vi "UNITEST MAIN v2.0.vi"() -> ()   [LabVIEW 2025]
uses:
  Traction Loop/Traction Receipe Enum.ctl
  v06/controls/LAB-IQ UI Data.ctl
  controls/REF Enum Unitest.ctl
  Acquostics Loops/Write Main Enum.ctl
  Acquostics Loops/Read Main Enum.ctl
  Temperature/Temperature enum.ctl
  Traction Loop/Traction Write enum.ctl
  Traction Loop/Traction Read enum.ctl
  HEAVE vi's/Heave Write enum.ctl
  HEAVE vi's/Heave Right enum.ctl
  SWAY vi's/Sway Write enum.ctl
  SWAY vi's/Sway Right enum.ctl
  v05/LOAD CELL CODE/New Logic/Load cell Enum.ctl
  48f5795f-33f4-4366-aaa7-704d1097ecc1.vi
  0f9b3d6c-7caf-4790-9f98-5fac89a3677b.vi
  d081153b-36ca-4bc4-8478-749476f82ba4.vi
  1202965f-721d-4349-8d61-5de826f379ef.vi
  02c5850b-52e8-4ed5-91f8-6f0ad62f4994.vi
  1223eb78-e4c4-4b69-bf80-185c82055158.vi
  e5651a45-6a49-4a3f-b503-ff1eaf449b4a.vi
  <vilib>/Utility/error.llb/Trim Whitespace One-Sided.vi
  support/Message Queue/Enqueue Message (Single).vi
  <vilib>/Utility/error.llb/Error Cluster From Error Code.vi
  <vilib>/Utility/file.llb/Read Delimited Spreadsheet (string).vi
  <vilib>/Utility/file.llb/Write Delimited Spreadsheet (string).vi
  <vilib>/ErrorRing/Error Ring.xnode
  support/Message Queue/LAB-IQ Message Queue.lvlib
  support/User Event - Stop/LAB-IQ User Event - Stop.lvlib
panel:
  in  "Disable Axis Jog Soft Limits":bool
  out "error out 6":errorcluster
  out "error out 5":errorcluster
  in  "Temperature 2":dbl caption="°C"
  out "error out 4":errorcluster
  out "Traction Recipe Start Recording":bool
  out "error out 3":errorcluster
  out "Depth (µm)":dbl min=-200.0 max=200.0 step=0.1 format="%.1f"
  out "tdms file out":refnum<k34>
  in  "Depthz":bool
  out "Acoustic Graphs":cluster{"number: 0 to 1":dbl, dbl, dbl}(graph)
  out "SET entrainment Velocity":dbl
  out "Test Array Size":i32
  in  "SRR INDEX [ STRIBECK]":i32
  out "Stribeck Size":i32
  out "SET SRR":dbl
  out "Enum - READ":T1
  out "ELAPSED TIMER":dbl
  out "BALL SET RPM":dbl
  out "DISC SET RPM":dbl
  out "SET LOAD":dbl
  in  "TEMPERATURE READ":dbl=40.0
  out "SET TEMPERATURE":dbl
  out "Traction Size":i32
  out "DISC SPEED (rpm)":dbl=100.0 min=0.1 max=3000.0 step=0.1 format="%.1f"
  out "BALL SPEED (rpm)":dbl=100.0 min=0.1 max=3000.0 step=0.1 format="%.1f"
  in  "BALL WEAR TRACK":dbl=7.9
  in  "DISC WEARTRACK":dbl=24.0
  in  "SRR INDEX [ TRACTION]":i32
  in  "Start Index Type":i32
  in  "Enum - Menu":T1
  out "Ball (mm/sec)":dbl
  out "Disc (mm/sec)":dbl
  in  "Traction Receipe Update Details":bool
  in  "HomeTraction":bool
  in  "Demo Mode Display":enum32{"Page 1", "Page 2"}(tab)
  in  "Traction Message":string="Recommended motion directions \nfor traction module.\n\nBall:  Counterclockwise\nDisc: Clockwise"
  in  "Traction Step Update Details":bool
  in  "Main Tab sequence for selection":T2(tab)
  out "ExceedDiscSpeed  Cinstant Speed":string
  out "ExceedBallSpeed Constant":string
  in  "TEST SELECTION (MTM) 2":enum32{"Ball Speed", "Disc Speed"}(radio)
  in  "SPEED SELECTION : MTM 2":enum32{"Speed in Rpm", "Speed in m/sec"}(radio)=enum."Speed in m/sec"
  in  "MTM Test Selection 2":enum32{"Time", "Cycle"}(radio)
  in  "Enter the Speed (m/sec):":dbl=0.5 min=3e-06 max=2500.0 step=0.001 format="%.6f"
  in  "Enter the Speed (m/sec):":dbl=0.5 min=3e-06 max=3000.0 step=0.001 format="%.6f"
  in  "Enter the Speed (RPM):":dbl=100.0 min=0.1 max=3000.0 step=0.1 format="%.1f"
  out "Lower Spped":string
  out "Upper":string
  in  "Enter the Speed (RPM):":dbl=1.0 min=0.1 max=2500.0 step=0.1 format="%.1f"
  out "ExceedBallSpeed step":string
  out "ExceedDiscSpeed":string
  out "Disc Speed Indicator":bool
  out "ExceedBallSpeed":string
  out "BallSpeed Exceed Indication":bool
  in  "Apply":bool
  in  "SPEED SELECTION : MTM":enum32{"Speed in Rpm", "Speed in m/sec"}(radio)=enum."Speed in m/sec"
  in  "TEST SELECTION (MTM)":enum32{"Ball Speed", "Disc Speed"}(radio)
  in  "MTM Test Selection":enum32{"Time", "Cycle"}(radio)
  in  "File Path Tab":enum32{"Page 1", "Page 2"}(tab)
  in  "File Path String":string="File Path Location : C:-->LAB-IQ 150 --> User Defined\n                                       Protocol-->File.txt"
  in  "Save":bool
  in  "Import":bool
  in  "File Path :":path
  in  "Step Sequence Indication Tab":enum32{"Page 1", "Page 2"}(tab)
  in  "Step Sequence Indication":string="Minimum 2 Steps required to perform the Speed Sequence"
  in  "Calculate Step":bool
  in  "StepTable":string[][](table)
  in  "Ramp Tab":enum32{"Page 1"}(tab)
  out "e.v/ssr":enum32{"E.V", "SSR"}(tab)
  in  "Enter Fixed SRR":dbl=1.0 min=-1.0 max=1.0 step=0.001 format="%.3f"
  in  "Enter the Final E.Velocity (m/s)":dbl=1.0 min=0.001 max=10.0 step=0.001 format="%.3f"
  in  "Enter initial E.Velocity (m/s)":dbl=2.0 min=0.001 max=10.0 step=0.001 format="%.3f"
  in  "Enter Fixed E.Velocity":dbl=1.0 min=0.001 max=2.0 step=0.001 format="%.3f"
  in  "Enter Final SRR":dbl=1.0 min=-1.0 max=1.0 step=0.001 format="%.2f"
  in  "Enter initial SRR":dbl=1.0 min=-1.0 max=1.0 step=0.001 format="%.2f"
  in  "Ball WTD":dbl=17.32 min=17.32 max=17.32 step=0.001 format="%.2f"
  in  "E.Velocity":bool caption="SRR"
  in  "Enter the Final Velocity (m/s)":dbl=1.0 min=0.001 max=2.0 step=0.001 format="%.3f"
  in  "Enter initial Velocity (m/s)":dbl=2.0 min=0.001 max=2.0 step=0.001 format="%.3f"
  out "Ramp Up   Disc":bool caption="Ramp Down"
  out "Initial DiscSpeed (RPM)":dbl=100.0 min=0.1 max=3000.0 step=0.1 format="%.1f"
  out "Final Speed (RPM)":dbl=1.0 min=0.1 max=3000.0 step=0.1 format="%.1f"
  out "Final Speed (RPM)":dbl=1.0 min=0.1 max=3000.0 step=0.1 format="%.1f"
  out "Initial Speed (RPM)":dbl=100.0 min=0.1 max=3000.0 step=0.1 format="%.1f"
  in  "Enter the Final Velocity (m/s)":dbl=1.0 min=0.001 max=2.0 step=0.001 format="%.3f"
  in  "Enter initial Velocity (m/s)":dbl=2.0 min=0.001 max=2.0 step=0.001 format="%.3f"
  out "Ramp Up":bool caption="Ramp Down"
  in  "Disc Motion Direction:":u16(ring) items=["Clockwise", "Counter Clockwise"]
  in  "Ball Motion Direction :":u16(ring) items=["Clockwise", "Counter Clockwise"]
  in  "Motion Mode:":u16(ring) items=["Uniform Rotation", "Speed Step", "Speed Ramp", "Speed Recipe"]
  in  "Wear Track Diameter (mm) 3":dbl=16.0 caption="Wear Track Diameter (mm):" min=1.0 max=20.0 step=0.01 format="%.2f"
  in  "Set WTD 2":bool
  in  "SRR Sweep Range (%)":string caption="Speed (mm/s)"
  out "Traction Receipe":i32(listbox)=-1
  in  "Total Execution Time":dbl
  in  "Total Steps":dbl
  in  "Duration / Step (s)":dbl=6.0
  in  "STRIBECK Fixed SRR List (%)":string="5,10,20,40,60,80,100"
  in  "Duration / Step (s)":dbl=6.0
  in  "SRR Sweep Range (%)":string
  in  "Speed (mm/s)":dbl=1000.0
  in  "Temperature Stages (°C)":string="40,100,140"
  in  "Load (N)":string="25"
  in  "Lubricant Name":string
  in  "Profile File Name":string
  out "error out":errorcluster
  in  "Checkbox 2":bool
  in  "Checkbox":bool=TRUE
  out "Scratch Start Recording":bool
  in  "SwaySpeed Set":bool
  in  "Analysis Home":bool
  out "Test Trip":bool
  out "Hymidity":bool
  in  "Humidity Disable trip":bool=TRUE
  in  "CoF Trip  2":dbl=540.0 min=100.0 max=540.0 step=1.0
  in  "File Path :  2":path
  out "Wear Track Diameter":dbl
  in  "Stribeck table":bool
  in  "seq":bool=TRUE
  out "Drive Error":string
  out "Scratch Start Test":bool
  in  "HomeScratch":bool
  in  "TEST SELECTION":enum32{"Time", "Cycle"}(radio)
  out "Spare 15":u8
  out "Spare 14":u8
  out "Spare 13":u8
  out "Spare 12":u8
  out "Spare 11":u8
  out "Spare 10":u8
  out "Spare 9":u8
  out "Spare 8":u8
  out "Start Test Temp":bool
  in  "PID Delay (sec)":dbl=1.0 format="%#_6p"
  out "Spare 15":u8
  out "Spare 14":u8
  out "Spare 13":u8
  out "Spare 12":u8
  out "Spare 11":u8
  out "Spare 10":u8
  out "Spare 9":u8
  out "Spare 8":u8
  out "Load Cell Temp":bool
  in  "Enter Fixed SRR 2":dbl min=0.0 max=0.0 format="%.3f"
  in  "E.Velocity 2":bool=TRUE caption="SRR"
  in  "Tab Control 3":T3(tab)
  in  "PID":T4={"min_deadband_floor"=50000000.0, "min_finetune_floor"=10.0, "dynamic_spindle_noise_scalar"=100.0, "filter_alpha"=0.05, "Vertical load (N)"=0.0, "Pulse delta"=0.0, "Fine Tune Zone"=10.0, "Max_pos_limit"=50000000.0, "Min_pos_limit"=0.0, "i_limit"=10.0, "Max Step Linit"=10.0, "Init Step"=10.0, "pct_scale"=100.0, "Deadband"=0.1, "Kd"=0.0, "Ki"=0.0, "Kp"=1.0, "Current Position"=0.0, "Set Load"=0.0, "Current Load"=0.0, "gFF Rot 7"={0.0, 0.0, 0.0}, "Bypass Load"=FALSE, "Enter ByPass Load"=0.0, "apply load"=FALSE} {"Vertical load (N)" format="%#.3f"}
  in  "Ramp":bool
  in  "Load Cell Link":T5={"model"="", "SN"=0, "Sensor IP"="192.168.1.100", "Port"=8080, "Acq Delay (ms)"=10.0, "Burst Delay (ms)"=10.0, "Save Dwell"=0.015, "FORCE (N)"=[], "TORQUE (N-m)"=[], "ft_data"=[1.0, 1.0, 1.0, 1.0, 1.0, 1.0], "running_flag"=FALSE, "ClearAll"=FALSE, "ZeroAll"=FALSE} {"Save Dwell" min=0.0 max=5.0 step=0.001 format="%.3f"}
  out "error out Temperature":errorcluster
  in  "READ TEMPERATURE":dbl
  out "Downlink traction":T6 {"TRACTION POSE 1" format="%#.6f"; "TRACTION POSE 2" format="%#.6f"; "Missed Packets" format="%#.6f"}
  in  "Uplink Traction":T7={"Sequence ID"=0, "Mode Command"=2, "Distance"=10000.0, "SPEED"=10000.0, "Reserved "=0.0, "SPARE 1"=0, "SPARE 2"=0, "SPARE  3"=0, "SPARE  4"=0, "SPARE  5"=0, "SPARE 6"=0, "SPARE 7"=0, "SPARE 8"=0, "SPARE 9"=0, "SPARE 10"=0, "SPARE 11"=0, "SPARE 12"=0, "SPARE 13"=0, "SPARE 14"=0, "SPARE 15"=0, "SPARE 16"=0, "SPARE 17"=0}
  out "DOWNLINK SWAY":T8 {"SWAY POSE" format="%#.6f"; "Rotary POSE" format="%#.6f"; "Missed Packets" format="%#.6f"}
  in  "UPLINK SWAY":T9={"Sequence ID"=0, "Mode Command"=2, "Distance"=10000.0, "SPEED"=10000.0, "Reserved"=0.0, "SPARE1"=0, "SPARE 2"=0, "SPARE  3"=0, "SPARE  4"=0, "SPARE  5"=0, "SPARE 6"=0, "SPARE 7"=0, "SPARE 8"=0, "SPARE 9"=0, "SPARE 10"=0, "SPARE 11"=0, "SPARE 12"=0, "SPARE 13"=0, "SPARE 14"=0, "SPARE 15"=0, "SPARE 16"=0, "SPARE 17"=0}
  out "DOWNLINK HEAVE":T10 {"HEAVE POSE" format="%#.6f"; "SURGE POSE" format="%#.6f"; "Missed Packets" format="%#.6f"}
  in  "UPLINK HEAVE":T11={"Sequence ID"=0, "Mode Command"=2, "Distance"=10000.0, "SPEED"=10000.0, "Reserved"=0.0, "SPARE 1"=0, "SPARE 2"=0, "SPARE 3"=0, "SPARE 4"=0, "SPARE 5"=0, "SPARE 6"=0, "SPARE 7"=0, "SPARE 8"=0, "SPARE 9"=0, "SPARE 10"=0, "SPARE 11"=0, "SPARE 12"=0, "SPARE 13"=0, "SPARE 14"=0, "SPARE 15"=0, "SPARE 16"=0, "SPARE 17"=0}
  out "error out 2":errorcluster
  in  "error in (no error)":errorcluster
  out "Downlink Packet":T12
  in  "Uplink Packet":T13
  in  "Manual Write TRACTION":bool
  out "TRACTION WRITE":string
  out "Read TRACTION Temp":bool
  out "error out Read TRACTION":errorcluster
  out "error out Write  TRACTION":errorcluster
  out "TRACTION READ":string
  in  "Manual Write SWAY":bool
  out "SWAY WRITE":string
  out "Read SWAY Temp":bool
  out "error out Read SWAY":errorcluster
  out "error out Write  SWAY":errorcluster
  out "SWAY READ":string
  out "HEAVE ENABLE":bool
  in  "Manual Write Heave & Surge":bool
  out "Heave and Surge Write":string
  out "Read Heave Temp":bool
  out "error out Read":errorcluster
  out "error out Write":errorcluster
  out "Heave and Surge Read":string
  out "DAQ Status":u32
  out "Isolated Gain":u32
  out "Current Filter Id":u32
  out "rx command count":u32
  out "Last Config Rejected":u32
  out "data out":string
  in  "Manual Write Acquostic":bool
  in  "Sway Loop Delay":dbl
  in  "Sway PID Speed":dbl=1.0 format="%.4f"
  in  "Sway Jog Speed":dbl=1.0 format="%.4f"
  in  "Heave Loop Delay":dbl
  in  "Heave PID Speed":dbl=15.0
  in  "Surge Jog Speed":dbl=1.0 format="%.4f"
  in  "Heave Jog Speed":dbl=15.0
  in  "Sway PPR":dbl=6400.0
  in  "Surge PPR":dbl=6400.0
  in  "Heave PPR":dbl=6400.0
  in  "Sway Pitch":dbl=2.0
  in  "Surge Pitch":dbl=3.0
  in  "Heave Pitch":dbl=4.0
  out "Sway Pulses/mm":dbl=320.0
  out "Surge Pulses/mm":dbl=1600.0
  out "Heave Pulses/mm":dbl=1600.0
  out "Zmm":dbl=1600.0
  in  "Heave distance":dbl=340.0
  in  "RotHomeSurgeOffsetCounts":dbl=311465.0
  in  "RotHomeSwayOffsetCounts":dbl=14656.0
  in  "TracHomeSwayOffsetCounts 20MM":dbl=1432.0
  in  "TracHomeSurgeOffsetCounts 20MM":dbl=505100.0
  in  "LRMHomeSwayOffsetCounts":dbl=26880.0
  in  "LRMHomeSurgeOffsetCounts":dbl=307197.0
  in  "Heave Counts:":dbl=100.0 min=0.0 max=100000000.0 step=1.0
  in  "Distance (mm):":dbl=100.0 min=0.0 max=1500.0 step=0.001 format="%.5f"
  in  "Distance (mm): 2":dbl=100.0 caption="Distance (mm):" min=0.0 max=1500.0 step=0.0001 format="%.3f"
  in  "Surge Counts:":dbl=100.0 min=0.0 max=100000000.0 step=1.0 format="%.1f"
  in  "Distance (mm): 3":dbl=100.0 caption="Distance (mm):" min=0.0 max=1500.0 step=0.001 format="%.5f"
  in  "Sway Counts:":dbl=100.0 min=0.0 max=100000000.0 step=1.0 format="%.2f"
  in  "Enter Distance":bool caption="Enter Counts"
  in  "SAVE  2":bool
  in  "DataSavingLoopDelay(ms)":dbl=15.0
  in  "Surge distance (mm)":dbl=370.0
  in  "Sway distance (mm)":dbl=245.0
  in  "Filter%":dbl=80.0 min=50.0 max=100.0 step=0.1 format="%.1f"
  in  "Apply Filter (Load)":bool=TRUE
  in  "Filter% 2":dbl=50.0 min=50.0 max=100.0 step=0.1 format="%.1f"
  in  "Apply Filter (FF)":bool
  in  "Acoustic Emission:":dbl=1.0 min=0.0001 max=200.0 step=0.0001 format="%.4f"
  in  "TracHomeSwayOffsetCounts 10MM":dbl=1432.0
  in  "TracHomeSurgeOffsetCounts 10MM":dbl=505100.0
  in  "Filter ON/OFF":bool=TRUE
  in  "Re-initilaize":bool
  in  "SAMPLES":dbl=100.0
  in  "JOG TRIP LOAD VALUE (N)":dbl
  in  "Start Button":bool
  in  "SURGE FORWARD COUNT":dbl
  in  "SURGE BACKWARD COUNT":dbl
  in  "SURGE SPEED":dbl
  in  "Firmware Version":string="BCLV 3.6"
  in  "Instrument Serial":string="770073"
  in  "Runtime":string="LabVIEW 2025 (64-bit)"
  in  "Workorder":string="2479"
  in  "Version":string="1.AU.26"
  in  "Operating System":string="Windows 11 Pro"
  in  "version":string="v1.AU.26"
  in  "COF TRIP VALUE":dbl
  in  "FF TRIP VALUE":dbl
  in  "CYCLIC FF TRIP VALUE":dbl
  in  "CYCLIC CoF TRIP VALUE":dbl
  in  "COF TRIP  ENABLE":bool
  in  "FF TRIP  ENABLE":bool
  in  "CYCLIC FF TRIP  ENABLE":bool
  in  "CYCLIC COF TRIP  ENABLE":bool
  in  "LOAD TRIP VALUE":dbl
  in  "LOAD TRIP  ENABLE":bool
  in  "DEPTH TRIP VALUE":dbl
  in  "DEPTH TRIP   ENABLE":bool
  in  "Rotary Vertical":bool
  in  "Rotary Horizontal":bool
  in  "Sway LRM":bool
  in  "LRM CAM":bool
  in  "Scratch 2":bool
  in  "Traction 2":bool
  in  "GUI":T14(tab)
  in  "Platform Settings":bool caption="Password"
  in  "Configure":bool caption="Password"
  in  "Home":bool caption="Password"
  in  "EXIT":bool
  in  "Analysis":bool caption="Password"
  in  "service 2":bool caption="Password"
  in  "MainPage":T15(tab)=enum."HOME"
  in  "Select Load Head":bool
  in  "Notes :":string
  in  "FILE":string
  in  "Sample ID :":string
  in  "Operator ID :":string
  in  "Operator Name :":string
  in  "Auto":bool caption="Power Status"
  in  "Disable Axis Jog Soft Limits m":bool
  out "Sway and Surge COM Status":bool=TRUE caption="Load COM Status"
  out "Heave COM Status":bool=TRUE caption="Load COM Status"
  in  "Enable Platform":bool
  in  "Surge Forward Main":bool
  in  "Surge Backward Main":bool
  in  "Sway Right Main":bool
  in  "Sway Left Main":bool
  in  "Heave Down Main":bool
  in  "Heave Up main":bool
  in  "mm":dbl=0.001 caption="Jog" min=0.001 max=100.0 step=0.01 format="%#.3f"
  in  "Surface Analysis":bool
  in  "Imaging":bool
  in  "Image Analysis":bool
  in  "Post Analysis":bool
  in  "SSP 0.75":bool
  in  "SSP 0.5":bool
  in  "SSP 0.3":bool
  in  "Warning":enum32{"Page 2"}(tab)
  in  "gui GIF":enum32{"Check", "Deca", "kilo", "Micro"}(tab)
  out "Communication is established":bool=TRUE caption="Load COM Status"
  in  "Reference Sample":u16(ring) items=["None", "Brass", "Aluminium", "Mild Steel"]
  in  "com 3":bool
  out "com":bool
  out "DecaForce COM Status":bool caption="Load COM Status"
  in  "Loading Mode":u16(ring) items=["Constant", "Ramp", "Steps", "Indentation"]
  in  "Enter the CoF Trip":dbl=1.0
  in  "Enter the Friction Force Trip":dbl=520.0 min=500.0 max=500.0 step=1.0 format="%#.1f"
  in  "Enter the Normal load Trip":dbl=520.0 min=500.0 max=500.0 step=0.001 format="%.3f"
  in  "KiloForce":bool
  in  "DecaForce":bool
  in  "MicroForce":bool
  in  "LHBack":bool
  in  "LHNext":bool
  in  "Load Selection":T16(tab)
  in  "Enter the Load  (N)":dbl=2.0 caption="Enter the Load (N)" min=2.0 max=50.0 step=0.1 format="%#.4f"
  in  "Enter the Final Load (N)":dbl=1.0 min=2.0 max=200.0 step=1.0 format="%#.0f"
  in  "Enter the Loading Rate (N/min)":dbl=60.0 min=1.0 max=200.0 step=0.1 format="%.2f"
  out "Warning 2":bool
  in  "Stribeck Table  For loading":string[][](table)
  in  "Clear 3":bool
  out "Message":string="Load Entered is out of range!!!"
  in  "Save 3":bool
  in  "Import 3":bool
  in  "Indentation":string[][](table)=[["Detection", "5", "2"], ["Unload", "0", "5"], ["Load", "10", "2"], ["Unload", "0", "5"], ["Detection", "5", "2"], ["Unload", "0", "5"]]
  in  "Multipoint":bool caption="Singlepoint"
  in  "AppLoad 4":bool
  in  "zNL":bool
  out "NL disp":dbl caption="Normal Load ( N )" min=-2000.0 max=2000.0 step=0.0001 format="%.1f"
  in  "Traction":bool
  in  "Surge Forward MM":bool
  in  "Surge Backward MM":bool
  in  "M3 Image":enum32{"Page 1", "Page 2"}(tab)
  in  "String 39":string="Jog heave to bring the upper sample closer to the lower sample within 1mm."
  in  "Sway Left MM":bool
  in  "Sway Right MM":bool
  in  "mm":dbl=0.001 caption="Jog" min=0.001 max=5.0 step=0.0001 format="%#.3f"
  in  "Heave Down MM":bool
  in  "Heave Up MM":bool
  in  "Wear Track Diameter (mm)":dbl=30.0 caption="Wear Track Diameter (mm):" min=1.0 max=30.0 step=1.0 format="%.2f"
  in  "Set WTD":bool
  in  "HomeScratch":bool
  in  "HomeRot":bool
  in  "PlaceModule":bool
  in  "Motion Mode:":u16(ring) items=["Uniform Rotation", "Angular Oscillation", "Stribeck ", "Steps"]
  in  "LR Sway":bool
  in  "Rot Hor":bool
  in  "Rot Ver":bool
  in  "Scratch":bool
  in  "LR Cam":bool
  in  "MMBack":bool
  in  "MMNext":bool
  in  "Rotary Module Selection":T17(tab)
  in  "SPEED SELECTION :":enum32{"Speed in RPM", "Speed in m/sec"}(radio)=enum."Speed in m/sec"
  in  "Enter the Speed(mm/sec)":dbl=0.1 min=0.0001 max=1000.0 step=0.1 format="%#.4f"
  in  "Enter the Speed (RPM)":dbl=45.0 min=1.0 max=3000.0 step=1.0
  in  "Enter the Frequency (Hz)":dbl=1.0 min=0.1 max=10.0 step=0.1 format="%.1f"
  in  "Enter the Angle (Deg)":dbl=45.0 min=5.0 max=300.0 step=1.0
  in  "Angular Oscillation Set":bool
  in  "Rotary Tab":enum32{"Page 1", "Page 2"}(tab)
  out "e.v/ssr 2":enum32{"E.V", "SSR"}(tab)
  in  "Enter the Final E.Velocity (m/s) 2":dbl=1.0 min=0.001 max=4.0 step=0.001 format="%.3f"
  in  "Enter initial E.Velocity (m/s) 2":dbl=2.0 min=0.001 max=4.0 step=0.001 format="%.3f"
  in  "Enter Fixed E.Velocity 2":dbl=1.0 min=0.001 max=2.0 step=0.001 format="%.3f"
  in  "Enter Final SRR 2":dbl=1.0 min=0.001 max=1.0 step=0.001 format="%.2f"
  in  "Enter initial SRR 2":dbl=1.0 min=0.001 max=1.0 step=0.001 format="%.2f"
  out "Final Speed (RPM) 3":dbl=1.0 min=0.1 max=3000.0 step=0.1 format="%.1f"
  out "Initial Speed (RPM) 2":dbl=100.0 min=0.1 max=3000.0 step=0.1 format="%.1f"
  in  "Enter the Final Velocity (m/s) 3":dbl=1.0 min=0.001 max=2.0 step=0.001 format="%.3f"
  in  "Enter initial Velocity (m/s)  3":dbl=2.0 min=0.001 max=2.0 step=0.001 format="%.3f"
  out "Ramp Up 2":bool caption="Ramp Down"
  in  "Import 2":bool
  in  "Save 2":bool
  in  "SPEED SELECTION : rotary":enum32{"Speed in Rpm", "Speed in m/sec"}(radio)=enum."Speed in m/sec"
  in  "calculate rotary":bool
  in  "String 45":string="File Path Location : C:-->LAB-IQ 150 --> User Defined\n                                       Protocol-->File.txt"
  in  "Step Speed":enum32{"Step Speed", "Step (load-Speed)"}(tab)
  in  "StepTable For Speed":string[][](table)
  in  "StepTable For Load-Speed":string[][](table)=[["", "", ""], ["", "", ""], ["", "", ""], ["", "", ""]]
  in  "StepTable For Speed 3":string[][](table)=[["", "", ""], ["", "", ""], ["", "", ""], ["", "", ""]]
  in  "Clear rot":bool
  in  "Motion Direction:  3":u16(ring)=1 items=["Clockwise", "Counter Clockwise"]
  in  "Enter Scratch length (mm):":dbl=1.0 min=1.0 max=50.0 step=0.0001 format="%.4f"
  in  "Enter Scratch Speed (mm/s):":dbl=1.0 min=0.003 max=10.0 step=0.0031 format="%.5f"
  in  "Scartch Offset":dbl=1.0 caption="Scratch Offset: (mm)" min=0.1 max=5.0 step=0.1 format="%.1f"
  in  "Motion type:":u16(ring) items=["Unidirection", "Bidirection"]
  in  "Scratch Mode":u16(ring) items=["Scratch", "Pre-Post Scan", "Multi Scratch"]
  in  "Rotary Speed Exced":string="Motor Speed Out of Range"
  in  "No of Scratch":dbl=1.0 min=1.0 max=50.0 step=0.0001
  out "Humidity  Status  3":bool caption="Communication Status"
  out "Low Temp  Status  2":bool=TRUE caption="Communication Status"
  out "TK4 status 2":bool=TRUE caption="Communication Status"
  in  "Acuostic M":string="Before selecting Acoustic make sure the sensor output pin is connected to A4."
  in  "Stage Temperature":dbl[](array[numeric])=[150.0, 230.0, 300.0, 350.0, 400.0, 450.0, 500.0]
  in  "Sample Temperature":dbl[](array[numeric])=[100.0, 150.0, 200.0, 250.0, 300.0, 350.0, 400.0]
  in  "Humidity (Amb)":bool
  in  "Clear List":bool
  out "Sensors Picked":string
  in  "Add to list":bool
  in  "Wear":bool
  in  "Vibration":bool
  in  "Humidity (Chamber)":bool
  in  "Temperature (Chamber)":bool
  in  "ECR":bool
  in  "Temperature (Amb)":bool
  in  "Microphone":bool
  in  "Acoustic Emission 3":bool
  in  "SNext":bool
  in  "APBack":bool
  in  "Enter the Temperature (°C):":dbl
  in  "Enter the Stage \nTemperature (°C):":dbl=20.0 min=20.0 max=150.0 step=1.0 format="%#.0f"
  in  "Enter the Humidity (%Rh):":dbl=30.0 min=30.0 max=85.0 step=1.0
  in  "Low Temp":bool
  in  "High Temp":bool
  in  "Humidity":bool
  in  "Gains":enum32{"20dB", "40dB", "60dB"}(radio)=enum."60dB"
  in  "Main Screen Tab":T18(tab)
  out "NL Trip 2":dbl=600.0
  in  "Load Disable Trip":bool=TRUE
  in  "Depth Trip 2":bool=TRUE
  out "Depth Trip":dbl=600.0
  in  "ClrLog":bool
  out "Trip Log":string
  in  "Start Test":bool
  out "Test status":bool caption="Test Status"
  out "AR Led":bool caption="AR"
  out "Data":bool=TRUE
  out "Health":bool=TRUE
  out "Sway COM Status":bool=TRUE caption="Load COM Status"
  out "Heave COM Status":bool=TRUE caption="Load COM Status"
  in  "BACK":bool
  out "Ambient \nTemperature":dbl min=0.0 max=5000.0 step=0.1 format="%.1f"
  out "Ambient\n Humidity":dbl min=0.0 max=5000.0 step=0.1 format="%.2f"
  out "NL disp 2":dbl caption="Normal Load ( N )" min=-2000.0 max=2000.0 step=0.0001 format="%.1f"
  out "Set Humidity":dbl caption="Set Humidity  (% Rh)" min=-2000.0 max=2000.0 step=1.0 format="%.1f"
  out "humidity disp":dbl caption="Humidity (% Rh)" min=-2000.0 max=2000.0 step=1.0 format="%.1f"
  in  "Humidity On":bool
  in  "zNL 2":bool
  in  "Load En":bool
  out "Freq (Hz)":dbl min=0.0 max=5000.0 step=0.1 format="%.4f"
  out "HumCOMStatus":bool caption="Communication Status"
  out "Load Communication":bool
  in  "Temp Tabs":enum32{"Low Temp", "High Temp"}(tab)=enum."High Temp"
  out "Controller  Status":bool
  out "ChamberTemp":dbl format="%#.1f"
  in  "SetTmp":dbl=-190.0 caption="Set Temperature (Deg C)" min=-190.0 max=100.0 step=1.0 format="%.1f"
  in  "Cooling":bool
  in  "Heater":bool
  out "TK4 status":bool caption="Controller  Status"
  out "ChamberTemp":dbl format="%#.1f"
  in  "SetTmp":dbl caption="Set Temperature (Deg C)" min=0.0 max=1000.0 step=1.0 format="%.1f"
  in  "Set Load (N)":dbl=100.0 min=0.01 max=1500.0 step=0.01 format="%.1f"
  in  "Time Tab":enum32{"cycles", "duration"}(tab)=enum."duration"
  out "Test Duration 4":dbl=600.0 caption="Test Duration\n(HH:MM:SS)" min=0.0083 max=180000.0 step=0.0001 format="%<%H:%M:%S>t"
  out "TEST CYCLE":dbl min=0.0 max=5000.0 step=0.01 format="%.2f"
  in  "TOTAL CYCLES":dbl min=0.0 max=5000.0 step=0.1 format="%.4f"
  out "Time ( HH:MM:SS ) 2":dbl min=0.0 max=144000.0 step=1.0 format="%<%H:%M:%S>t"
  in  "Test Duration":dbl=600.0 caption="Test Duration\n(HH:MM:SS)" min=0.0083 max=180000.0 step=0.0001 format="%<%H:%M:%S>t"
  in  "Main Speed Tab":enum32{"ROTARY", "TRACTION"}(tab)
  in  "SPEED TAB":enum32{"RPM", "m/sec"}(tab)
  out "Speed (RPM)":dbl min=0.0 max=5000.0 step=0.1 format="%.1f"
  out "Set Speed":dbl caption="Set Speed (RPM)" min=0.0 max=1500.0 step=0.1 format="%.1f"
  out "Speed (m/sec)":dbl min=0.0 max=5000.0 step=0.001 format="%.4f"
  out "Set Speed (m/sec)":dbl min=0.0 max=1500.0 step=0.001 format="%.4f"
  in  "MTM MOTOR DISPLAY":enum32{"MTM RPM", "MTM m/sec"}(tab)
  out "Disc Speed (RPM)":dbl min=0.0 max=1500.0 step=0.1 format="%.1f"
  out "Ball Speed (RPM)":dbl min=0.0 max=1500.0 step=0.1 format="%.1f"
  out "Disc Speed (m/sec)":dbl min=0.0 max=1500.0 step=0.1 format="%.1f"
  out "Ball Speed (m/sec)":dbl min=0.0 max=1500.0 step=0.1 format="%.1f"
  in  "Angle and Frequency":enum32{"angular", "lrm"}(tab)
  out "Angle (Deg)":dbl min=0.0 max=5000.0 step=0.01 format="%.2f"
  out "Stroke (mm)":dbl min=0.0 max=5000.0 step=0.01 format="%.2f"
  in  "STOP":bool
  out "Multi Scratch Pass":dbl min=0.0 max=5000.0 step=0.1
  in  "FF Tab":T19(tab)
  in  "COF Disable Trip":bool=TRUE
  out "COF TRIP":dbl=600.0
  out "Coefficient of Friction":dbl[](graph) caption="Waveform Chart - Dark"
  in  "zFF":bool
  in  "FF Disable Trip":bool=TRUE
  out "FF TRIP":dbl=600.0
  out "Friction Force (N)":dbl min=-2000.0 max=2000.0 step=0.0001 format="%.3f"
  out "Friction Force (N)":dbl[](graph) caption="Waveform Chart - Dark"
  in  "CZ FF":bool
  out "Cyclic Friction Force (N)":dbl min=-2000.0 max=2000.0 step=0.0001 format="%.3f"
  out "Cyclic FF TRIP":dbl=600.0
  in  "Cyclic FF Disable Trip":bool=TRUE
  out "cyclic COF TRIP":dbl=600.0
  in  "cyclic COF Disable Trip":bool=TRUE
  out "Acoustic Emission (mV)":dbl min=0.0 max=5000.0 step=0.1
  out "Normal Load ( N )":dbl[](graph) caption="Waveform Chart - Dark"
  out "Acoustic Emission":dbl[](graph) caption="Waveform Chart - Dark"
  out "Depth (Microns)":dbl[](graph) caption="Waveform Chart - Dark"
  in  "X-AXIS":u16(ring) items=["None", "Time ( Sec )", "Normal Load ( N )", "Frictional Force ( N )", "Coefficient of Friction", "Depth ( Microns )", "Speed ( RPM )", "Frequency ( Hz )", "Angle ( Degree )", "Cyclic Friction Force ( N )", "Cyclic Co efficient Friction ", "Stage temperature ( Degree celcius )", "Sample temperature ( Degree celcius )", "Stroke Length ( mm )", "Scratch Speed ( mm/sec )", "Amb Humidity ( % Rh ) ", "Amb Temperature (Deg C)", "Acoustic (mV)", "Mx (Nm)", "My (Nm)", "Mz (Nm)", "Humidity ( % Rh )", "Sliding Distance (mm)", "Wear Track Diameter (mm)", "Fx(N)", "Fy(N)", "MTM BallSpeed (RPM)", "MTM DiscSpeed (RPM)", "Entrainment Speed", "Slide Role", "Slip(%)", "Rotary Speed (m/sec)", "MTM Ball Speed (m/sec)", "MTM Disc Speed (m/sec)", "ECR (ohms)", "Cycles (N)"]
  in  "Y-AXIS":u16(ring) items=["None", "Time ( Sec )", "Normal Load ( N )", "Frictional Force ( N )", "Coefficient of Friction", "Depth ( Microns )", "Speed ( RPM )", "Frequency ( Hz )", "Angle ( Degree )", "Cyclic Friction Force ( N )", "Cyclic Co efficient Friction ", "Stage temperature ( Degree celcius )", "Sample temperature ( Degree celcius )", "Stroke Length ( mm )", "Scratch Speed ( mm/sec )", "Amb Humidity ( % Rh ) ", "Amb Temperature (Deg C)", "Acoustic (mV)", "Mx (Nm)", "My (Nm)", "Mz (Nm)", "Humidity ( % Rh )", "Sliding Distance (mm)", "Wear Track Diameter (mm)", "Fx(N)", "Fy(N)", "MTM BallSpeed (RPM)", "MTM DiscSpeed (RPM)", "Entrainment Speed", "Slide Role", "Slip(%)", "Rotary Speed (m/sec)", "MTM Ball Speed (m/sec)", "MTM Disc Speed (m/sec)", "ECR (ohms)", "Cycles (N)"]
  out "XY Graph":cluster{"Array 2":dbl[], "Array 2":dbl[]}[](graph) caption="XY Graph 20"
  out "VARIANCE":dbl=-0.0 format="%0.2f"
  out "SD":dbl=-0.0 format="%.3f"
  out "MEAN":dbl format="%.3f"
  out "VARIANCE":dbl=-0.0 format="%0.2f"
  out "SD":dbl=-0.0 format="%.3f"
  out "MEAN":dbl format="%.3f"
  out "VARIANCE":dbl=-0.0 format="%0.2f"
  out "SD":dbl=-0.0 format="%.3f"
  out "MEAN":dbl format="%.3f"
  out "VARIANCE":dbl=-0.0 format="%0.2f"
  out "SD":dbl=-0.0 format="%.3f"
  out "MEAN":dbl format="%.3f"
  in  "Analysis Home new":bool
  out "File 2 Discription":string="\r"
  out "File 1 Discription":string="\r"
  in  "OPEN 1":bool
  in  "OPEN 2":bool
  out "File Name 1":string
  out "File Name 2":string
  in  "Refresh 2":bool
  in  "OPEN 3":bool
  out "File Name 3":string
  out "File Name 4":string
  in  "OPEN 4":bool
  out "File 4 Discription":string="\r"
  out "File 3 Discription":string="\r"
  in  "File Format":u16(ring) items=["csv", "txt", "duf"]
  in  "Export":bool
  in  "Report":bool
  in  "Password":string
  in  "Home Service":bool
  in  "Advanced Setting":bool
  in  "Edit Gain Constants":bool
  in  "Save Gain Constants":bool
  in  "Humidity Port:":refnum<visa-resource-name>="COM10"
  in  "Temperature":refnum<visa-resource-name>="COM14"
  in  "ECR Port:":refnum<visa-resource-name>="COM10"
  in  "Info":bool
  in  "Service About":bool
  # "1. Test Identification & Global Setup"
  # "2. Step Configurations & Timing"
  # "Step 1 Configuration: TRACTION Step"
  # "%"
  # "NOTE: This operation needs to be done only when the machine is ON."
  # "Steps 2+ Configuration: STRIBECK Steps"
  # "Acoustic Emission (mV)"
  # "Upper Drive (Ball)"
  # "Lower Drive (Disc)"
  # "Variable"
  # "Configuration"
  # "ABOUT SCREEN PARAMETERS"
  # "Limits for Heave Surge and Sway"
  # "© 2023"
  # "Modules Offset Parameters"
  # "Counts-Distance Calculator"
  # "SURGE MOVEMENT"
  # "STAGE SELECTION"
  # "LOAD TRIP PARAMETERS"
  # "File Name :"
  # "Ensure the traction module is aligned\n horizontally with the stage before ENABLE."
  # "JOG MODE"
  # "Module Selection"
  # "Positioning Control"
  # "Connect the controller\ncable to M2"
  # "Environment"
  # "Sensors"
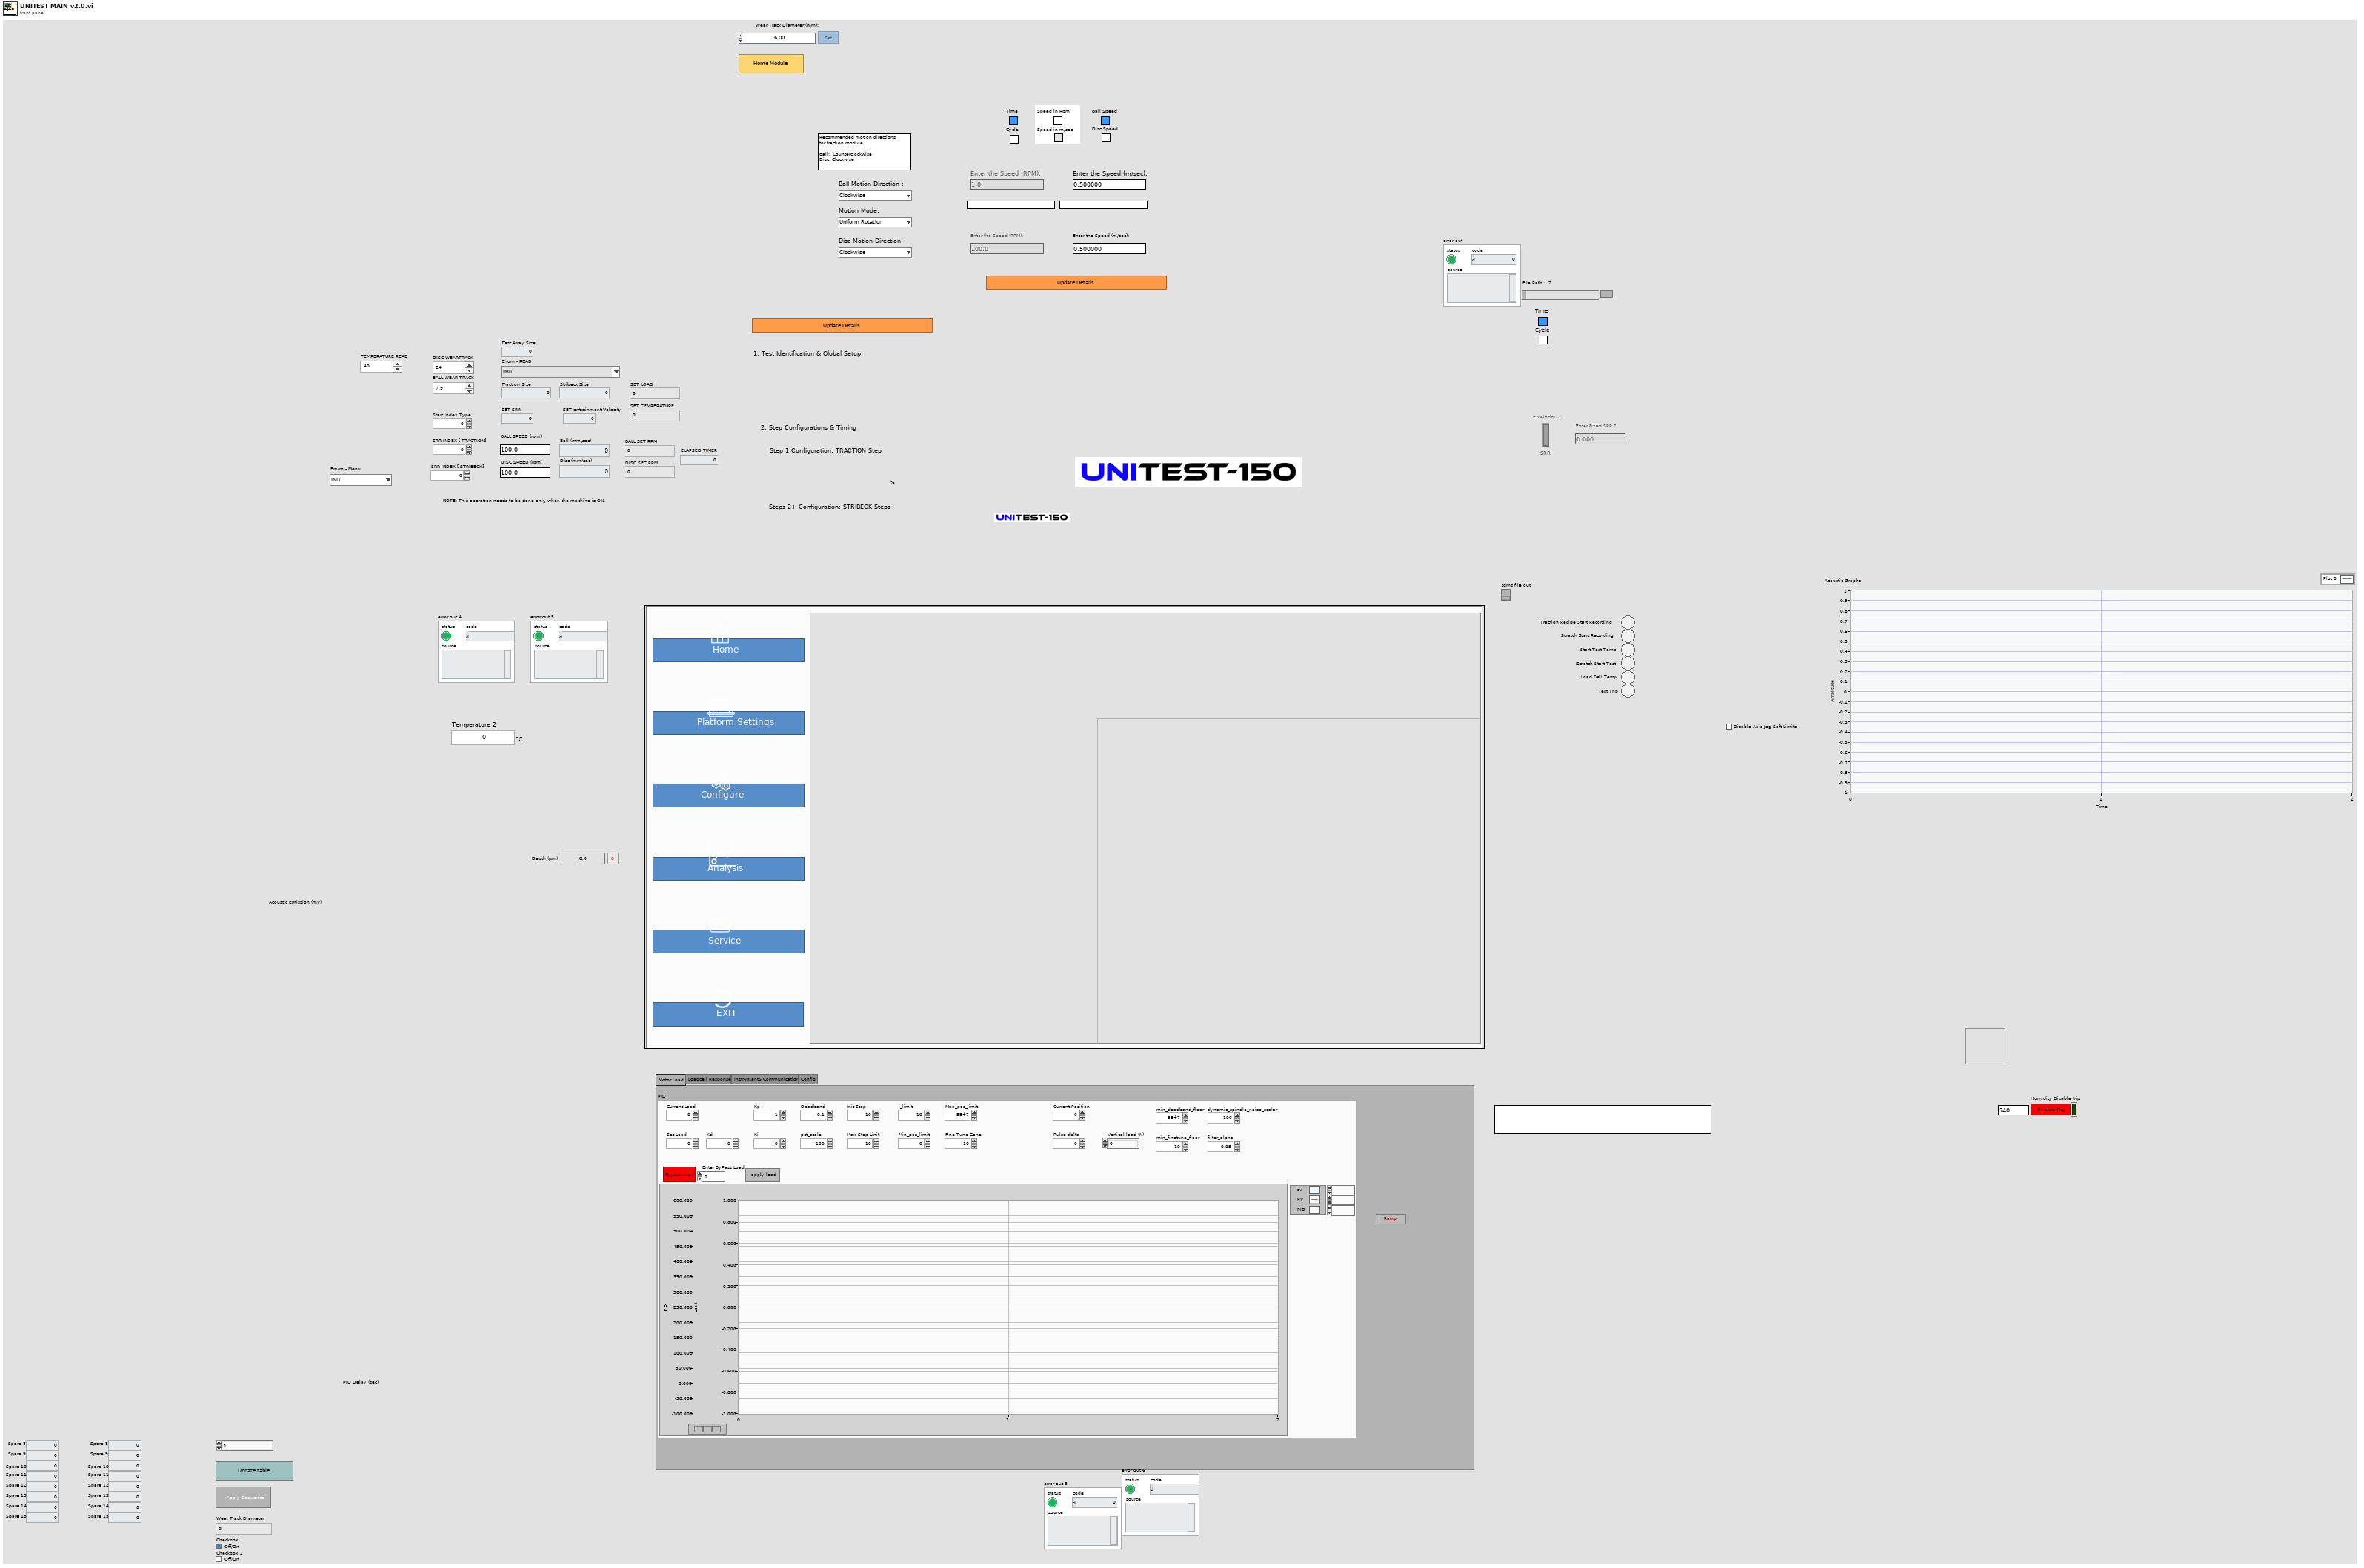
[diagram p1: front panel]
types:
  T1 = typedef "Traction Receipe Enum.ctl" = enum16{"INIT", "START", "TRACTION", "STRIBECK", "MAIN INDEX INCREMENT", "TEMPERATURE SET", "TEMPERATURE REACH", "CHURNING START", "CHURNING STOP", "LOAD", "LOAD REACHED", "SRR SET", "SRR WAIT", "SRR INCREMENT", "SPEED SET", "SPEED WAIT", "SPEED INCREMENT", "UNLOAD", "CLOSE"}
  T2 = enum32{"Uniform Rotary", "Speed Sequence", "SpeedRamp"}
  T3 = enum32{"Motor Load", "Loadcell Response", "Motor", "Depth_graph", "UIO Communicator", "Add to list parametrs", "InstrumentS Communication", "Config"}
  T4 = cluster{"min_deadband_floor":dbl, "min_finetune_floor":dbl, "dynamic_spindle_noise_scalar":dbl, "filter_alpha":dbl, "Vertical load (N)":dbl, "Pulse delta":dbl, "Fine Tune Zone":dbl, "Max_pos_limit":dbl, "Min_pos_limit":dbl, "i_limit":dbl, "Max Step Linit":dbl, "Init Step":dbl, "pct_scale":dbl, "Deadband":dbl, "Kd":dbl, "Ki":dbl, "Kp":dbl, "Current Position":dbl, "Set Load":dbl, "Current Load":dbl, "gFF Rot 7":cluster{dbl, dbl, dbl}, "Bypass Load":bool, "Enter ByPass Load":dbl, "apply load":bool}
  T5 = cluster{"model":string, "SN":i32, "Sensor IP":string, "Port":i32, "Acq Delay (ms)":dbl, "Burst Delay (ms)":dbl, "Save Dwell":dbl, "FORCE (N)":dbl[][], "TORQUE (N-m)":dbl[][], "ft_data":dbl[], "running_flag":bool, "ClearAll":bool, "ZeroAll":bool}
  T6 = cluster{"Ack ID":u16, "State":u8, "Homed":u8, "TRACTION POSE 1":sgl, "TRACTION POSE 2":sgl, "faultCode ":u16, "fwMajor ":u8, "fwMinor":u8, "Node Id":u8, "Spare 1":u8, "Spare 2":u8, "Spare 3":u8, "Spare 4":u8, "Spare 5":u8, "Spare 6":u8, "Spare 7":u8, "System UPTIME":sgl, "Missed Packets":sgl, "faultCode Traction 1":u16, "faultCode Traction 2":u16}
  T7 = cluster{"Sequence ID":u16, "Mode Command":u8, "Distance":sgl, "SPEED":sgl, "Reserved ":sgl, "SPARE 1":u8, "SPARE 2":u8, "SPARE  3":u8, "SPARE  4":u8, "SPARE  5":u8, "SPARE 6":u8, "SPARE 7":u8, "SPARE 8":u8, "SPARE 9":u8, "SPARE 10":u8, "SPARE 11":u8, "SPARE 12":u8, "SPARE 13":u8, "SPARE 14":u8, "SPARE 15":u8, "SPARE 16":u8, "SPARE 17":u8}
  T8 = cluster{"Ack ID ":u16, "State":u8, "Homed":u8, "SWAY POSE ":sgl, "Rotary POSE ":sgl, "faultCode":u16, "fwMajor":u8, "fwMinor":u8, "Node Id":u8, "Spare 1":u8, "Spare 2":u8, "Spare 3":u8, "Spare 4":u8, "Spare 5":u8, "Spare 6":u8, "Spare 7":u8, "System UPTIME ":sgl, "Missed Packets ":sgl, "faultCode Sway":u16, "faultCode Rotary":u16}
  T9 = cluster{"Sequence ID":u16, "Mode Command":u8, "Distance":sgl, "SPEED":sgl, "Reserved":sgl, "SPARE1":u8, "SPARE 2":u8, "SPARE  3":u8, "SPARE  4":u8, "SPARE  5":u8, "SPARE 6":u8, "SPARE 7":u8, "SPARE 8":u8, "SPARE 9":u8, "SPARE 10":u8, "SPARE 11":u8, "SPARE 12":u8, "SPARE 13":u8, "SPARE 14":u8, "SPARE 15":u8, "SPARE 16":u8, "SPARE 17":u8}
  T10 = cluster{"Ack ID":u16, "State":u8, "Homed":u8, "HEAVE POSE":sgl, "SURGE POSE":sgl, "faultCode":u16, "fwMajor":u8, "fwMinor":u8, "Node Id":u8, "Temp":u8, "Humidity":u8, "Spare 1":u8, "Spare 2":u8, "Spare 3":u8, "Spare 4":u8, "Spare 5":u8, "System UPTIME":sgl, "Missed Packets":sgl, "faultCode Heave":u16, "faultCode Surge Left":u16, "faultCode Surge Right":u16}
  T11 = cluster{"Sequence ID":u16, "Mode Command":u8, "Distance":sgl, "SPEED":sgl, "Reserved":sgl, "SPARE 1":u8, "SPARE 2":u8, "SPARE 3":u8, "SPARE 4":u8, "SPARE 5":u8, "SPARE 6":u8, "SPARE 7":u8, "SPARE 8":u8, "SPARE 9":u8, "SPARE 10":u8, "SPARE 11":u8, "SPARE 12":u8, "SPARE 13":u8, "SPARE 14":u8, "SPARE 15":u8, "SPARE 16":u8, "SPARE 17":u8}
  T12 = cluster{"Sequence ID":u32, "Timestamp":u32, "System Status":u32, "Peak Amplitude":sgl, "Amplitude dB_AE":sgl, "AE Ring-Down Counts":u32, "Signal Energy":sgl, "Spare 1":u32}
  T13 = cluster{"Sequence ID":u32, "Target Gain":u32, "Target Filter":u32, "Spare 1":u32, "Spare 2":u32, "Spare 3":u32, "Spare 4":u32, "Spare 5":u32}
  T14 = enum32{"Setup", "Load Head", "Motion Module", "Environment", "Begin"}
  T15 = enum32{"Details", "PlatformSetting", "Analysis", "HOME"}
  T16 = enum32{"Constant", "Ramp", "Step", "Indentation"}
  T17 = enum32{"Uniform Rotation", "Angular Oscillation", "Speed Ramp", "Speed Step"}
  T18 = enum32{"  Acquire  ", "Compare Files Rot", "About", "Service"}
  T19 = enum32{"Coefficient of Friction ", "Friction Force (N)", "Cyclic Friction Force (N)", "Cyclic Coefficient of Friction "}
  T20 = typedef "REF Enum Unitest.ctl" = enum16{"Init", "UI Loop", "LOAD COM LOOP", "HEAVE MOTOR COM LOOP", "SWAY MOTOR COM LOOP", "RAMP MOTOR COM LOOP", "TEMPERATURE COM LOOP", "HUMIDITY COM PORT", "ECR PORT", "MONITOR LOOP", "PROGRAM LOOP", "LOAD PID", "REPORT", "ACOUSTIC"}
  T21 = typedef "LAB-IQ UI Data.ctl" = cluster{"Main Home Screen":cluster{"GUI":refnum<vi>, "Platform Settings":refnum<vi>, "Configure":refnum<vi>, "Home":refnum<vi>, "EXIT":refnum<vi>, "service 2":refnum<vi>, "MainPage":refnum<vi>, "Analysis":refnum<vi>}, "Platform Settings":cluster{"mm/s  Surge":refnum<vi>, "Drive Error":refnum<vi>, "Disable Axis Jog Soft Limits":refnum<vi>, "mm/s  Sway":refnum<vi>, "Sway and Surge COM Status":refnum<vi>, "Heave COM Status":refnum<vi>, "Enable Platform":refnum<vi>, "Surge Forward Main":refnum<vi>, "Sway Right Main":refnum<vi>, "Sway Left Main":refnum<vi>, "Heave Down Main":refnum<vi>, "Heave Up main":refnum<vi>, "mm/s Heave":refnum<vi>, "mm/sec":refnum<vi>, "mm":refnum<vi>, "Surge Backward Main":refnum<vi>}, "Analysis Screen":cluster{"Analysis Home":refnum<vi>, "Surface Analysis":refnum<vi>, "Imaging":refnum<vi>, "Image Analysis":refnum<vi>, "Post Analysis":refnum<vi>}, "Config Screen":cluster{"Select Load Head":refnum<vi>, "Notes :":refnum<vi>, "FILE":refnum<vi>, "Sample ID :":refnum<vi>, "Operator ID :":refnum<vi>, "Operator Name :":refnum<vi>, "Auto":refnum<vi>}, "Motion Module":cluster{"zNL":refnum<vi>, "NL disp":refnum<vi>, "Rotary Tab":refnum<vi>, "Motion Direction:  3":refnum<vi>, "E.Velocity 2":refnum<vi>, "e.v/ssr 2":refnum<vi>, "Enter Fixed E.Velocity 2":refnum<vi>, "Enter Final SRR 2":refnum<vi>, "Enter initial SRR 2":refnum<vi>, "Enter Fixed SRR 2":refnum<vi>, "Enter the Final E.Velocity (m/s) 2":refnum<vi>, "Enter initial E.Velocity (m/s) 2":refnum<vi>, "Final Speed (RPM) 3":refnum<vi>, "Initial Speed (RPM) 2":refnum<vi>, "Enter the Final Velocity (m/s) 3":refnum<vi>, "Enter initial Velocity (m/s)  3":refnum<vi>, "Ramp Up 2":refnum<vi>, "TEST SELECTION":refnum<vi>, "SPEED SELECTION : ":refnum<vi>, "Angular Oscillation Set":refnum<vi>, "Traction":refnum<vi>, "Step Speed":refnum<vi>, "StepTable For Load-Speed":refnum<vi>, "StepTable For Speed":refnum<vi>, "Surge Forward MM":refnum<vi>, "Surge Backward MM":refnum<vi>, "M3 Image":refnum<vi>, "String 39":refnum<vi>, "Sway Left MM":refnum<vi>, "Sway Right MM":refnum<vi>, "Disable Axis Jog Soft Limits":refnum<vi>, "mm":refnum<vi>, "Heave Down MM":refnum<vi>, "Heave Up MM":refnum<vi>, "Wear Track Diameter (mm)":refnum<vi>, "Set WTD":refnum<vi>, "HomeScratch":refnum<vi>, "HomeRot":refnum<vi>, "PlaceModule":refnum<vi>, "Enter the Angle (Deg)":refnum<vi>, "Enter the Frequency (Hz)":refnum<vi>, "Motion Mode:":refnum<vi>, "LR Sway":refnum<vi>, "Rot Hor":refnum<vi>, "Scratch":refnum<vi>, "LR Cam":refnum<vi>, "MMBack":refnum<vi>, "MMNext":refnum<vi>, "Rot Ver":refnum<vi>, "Rotary Module Selection":refnum<vi>, "calculate rotary":refnum<vi>, "SPEED SELECTION : rotary":refnum<vi>, "Import 2":refnum<vi>, "Save 2":refnum<vi>, "File Path :  2":refnum<vi>, "String 45":refnum<vi>, "StepTable For Speed 3":refnum<vi>, "Enter the Speed(mm/sec)":refnum<vi>, "Enter the Speed(RPM)":refnum<vi>, "Enter Scratch Speed (mm/s):":refnum<vi>, "SwaySpeed Set":refnum<vi>, "Scartch Offset":refnum<vi>, "Motion type:":refnum<vi>, "HomeScratch 2":refnum<vi>, "Enter Scratch length (mm):":refnum<vi>, "Wear Track Diameter":refnum<vi>, "Rotary Speed Exced":refnum<vi>, "Scratch Mode":refnum<vi>, "No of Scratch":refnum<vi>}, "Environmental control":cluster{"Humidity  Status  3":refnum<vi>, "Low Temp  Status  2":refnum<vi>, "TK4 status 2":refnum<vi>, "Stage Temperature":refnum<vi>, "Sample Temperature":refnum<vi>, "Humidity (Amb)":refnum<vi>, "Clear List":refnum<vi>, "Add to list":refnum<vi>, "Wear":refnum<vi>, "Vibration":refnum<vi>, "Humidity (Chamber)":refnum<vi>, "Temperature (Chamber)":refnum<vi>, "ECR ":refnum<vi>, "Temperature (Amb)":refnum<vi>, "Microphone":refnum<vi>, "Acoustic Emission 3":refnum<vi>, "SNext":refnum<vi>, "APBack":refnum<vi>, "Enter the Temperature (°C):":refnum<vi>, "Enter the Stage \nTemperature (°C):":refnum<vi>, "Enter the Humidity (%Rh):":refnum<vi>, "Low Temp":refnum<vi>, "High Temp":refnum<vi>, "Humidity":refnum<vi>, "Sensors Picked":refnum<vi>}, "About Screen":cluster{"Password":refnum<vi>, "Home Service":refnum<vi>, "Advanced Setting":refnum<vi>, "About Tab":refnum<vi>, "ECR Port:":refnum<vi>, "Ramp Port:":refnum<vi>, "Installation/Replacement completed":refnum<vi>, "Loahead":refnum<vi>, "Heave and Surge COM Port:":refnum<vi>, "Sway COM Port:":refnum<vi>, "Temp Modbus:":refnum<vi>, "Humidity Port:":refnum<vi>, "Edit Gain Constants":refnum<vi>, "Save Gain Constants":refnum<vi>}, "Main Screen":cluster{"Main Screen Tab":refnum<vi>, "Angle and Frequency":refnum<vi>, "Stroke (mm)":refnum<vi>, "Angle (Deg)":refnum<vi>, "Main Speed Tab":refnum<vi>, "MTM MOTOR DISPLAY":refnum<vi>, "Disc Speed (m/sec)":refnum<vi>, "Ball Speed (m/sec)":refnum<vi>, "Disc Speed (RPM)":refnum<vi>, "Ball Speed (RPM)":refnum<vi>, "SPEED TAB":refnum<vi>, "Speed (m/sec)":refnum<vi>, "Set Speed (m/sec)":refnum<vi>, "Speed (RPM)":refnum<vi>, "Set Speed":refnum<vi>, "Time Tab":refnum<vi>, "Time ( HH:MM:SS ) 2":refnum<vi>, "Test Duration":refnum<vi>, "Test Duration 4":refnum<vi>, "TEST CYCLE":refnum<vi>, "TOTAL CYCLES":refnum<vi>, "Set Load (N)":refnum<vi>, "Temp Tabs":refnum<vi>, "Heater":refnum<vi>, "TK4 status":refnum<vi>, "ChamberTemp":refnum<vi>, "SetTmp":refnum<vi>, "Controller  Status":refnum<vi>, "ChamberTemp 2":refnum<vi>, "SetTmp 2":refnum<vi>, "Controller  Status 2":refnum<vi>, "ChamberTemp 3":refnum<vi>, "SetTmp 3":refnum<vi>, "Cooling":refnum<vi>, "Load Communication":refnum<vi>, "Ambient \nTemperature":refnum<vi>, "HumCOMStatus":refnum<vi>, "Ambient\n Humidity":refnum<vi>, "Freq (Hz)":refnum<vi>, "Load En":refnum<vi>, "NLt":refnum<vi>, "zNL 2":refnum<vi>, "Humidity On":refnum<vi>, "humidity disp":refnum<vi>, "Set Humidity":refnum<vi>, "NL disp 2":refnum<vi>, "Humidity On 2":refnum<vi>, "humidity disp 2":refnum<vi>, "Set Humidity 2":refnum<vi>, "NL disp 3":refnum<vi>, "AppLoadSeq scratch":refnum<vi>, "Stop Scratch":refnum<vi>, "ClrLog":refnum<vi>, "Trip Log":refnum<vi>, "STOP":refnum<vi>, "Start Test":refnum<vi>, "Test status":refnum<vi>, "AR Led":refnum<vi>, "Data":refnum<vi>, "Health":refnum<vi>, "Sway COM Status":refnum<vi>, "Heave COM Status":refnum<vi>, "Grp Tab":refnum<vi>, "Sub Graph":refnum<vi>, "SD (mm)":refnum<vi>, "Siliding distance Reset Graph":refnum<vi>, "SDGp":refnum<vi>, "Humidity Reset Graph":refnum<vi>, "HumrGp":refnum<vi>, "Acoustic Emission (mV)":refnum<vi>, "Aqucostic Reset Graph":refnum<vi>, "gACQUOS":refnum<vi>, "ECR RESET":refnum<vi>, "ECR":refnum<vi>, "Temperature Reset":refnum<vi>, "Acoustic Emission (mV) 2":refnum<vi>, "Aqucostic Reset Graph 2":refnum<vi>, "gACQUOS 2":refnum<vi>, "ECR RESET 2":refnum<vi>, "ECR 2":refnum<vi>, "Temperature Reset 2":refnum<vi>, "Temperature (deg c)":refnum<vi>, "Speed Reset Graph":refnum<vi>, "Speed Tab":refnum<vi>, "MTM DISC  SPEED":refnum<vi>, "MTM BALL SPEED":refnum<vi>, "speed mm/sec":refnum<vi>, "Hymidity":refnum<vi>, "Humidity Disable trip":refnum<vi>, "CoF Trip  2":refnum<vi>, "Depth Trip":refnum<vi>, "Weart Deapth":refnum<vi>, "Depth Reset Graph":refnum<vi>, "Weart":refnum<vi>, "Depthz":refnum<vi>, "Depth (µm)":refnum<vi>, "WearGp":refnum<vi>, "NL Trip 2":refnum<vi>, "Load pid":refnum<vi>, "Load Disable Trip":refnum<vi>, "Load Reset Graph":refnum<vi>, "NL Display 4":refnum<vi>, "Main Chart 3":refnum<vi>, "BACK":refnum<vi>, "Depth Trip 2":refnum<vi>, "COF TRIP ":refnum<vi>, "Friction Force (N)":refnum<vi>, "FF Reset Graph":refnum<vi>, "FF Disable Trip":refnum<vi>, "FF TRIP":refnum<vi>, "COF Disable Trip":refnum<vi>, "COF Reset Graph":refnum<vi>, "Start Test Temp":refnum<vi>, "zFF":refnum<vi>, "Friction Force (N) Graph":refnum<vi>, "Coefficient of Friction":refnum<vi>, "Scratch Start Test":refnum<vi>, "FF Tab":refnum<vi>, "Cyclic Friction Force (N)":refnum<vi>, "CZ FF":refnum<vi>, "Cyclic Friction Force (N) Graph":refnum<vi>, "Cyclic Coefficient of Friction":refnum<vi>, "Cyclic FF TRIP":refnum<vi>, "Cyclic FF Disable Trip":refnum<vi>, "cyclic COF Disable Trip":refnum<vi>, "cyclic COF TRIP":refnum<vi>, "cyclic COF Reset Graph":refnum<vi>, "Cyclic FF Reset Graph":refnum<vi>, "Test Trip":refnum<vi>, "Multi Scratch Pass":refnum<vi>, "Scratch Start Recording":refnum<vi>, "Coefficient of Friction 2":refnum<vi>, "Acoustic Emission":refnum<vi>, "Friction Force (N) 2":refnum<vi>, "Depth (Microns)":refnum<vi>, "Normal Load ( N )":refnum<vi>}, "Loading":cluster{"Indentation":refnum<vi>, "Reference Sample":refnum<vi>, "Load Cell Communication Slide":refnum<vi>, "com 3":refnum<vi>, "com":refnum<vi>, "DecaForce COM Status":refnum<vi>, "Update":refnum<vi>, "Clear 3":refnum<vi>, "seq":refnum<vi>, "Stribeck table":refnum<vi>, "Stribeck Table  For loading":refnum<vi>, "Loading Mode":refnum<vi>, "Enter the Final Load (N)":refnum<vi>, "Enter the CoF Trip":refnum<vi>, "Enter the Friction Force Trip":refnum<vi>, "Enter the Normal load Trip":refnum<vi>, "Enter the Load  (N)":refnum<vi>, "KiloForce":refnum<vi>, "DecaForce ":refnum<vi>, "MicroForce":refnum<vi>, "LHBack":refnum<vi>, "LHNext":refnum<vi>, "Enter the Loading Rate (N/min)":refnum<vi>, "Message":refnum<vi>, "Warning 2":refnum<vi>, "SSP 0.75":refnum<vi>, "SSP 0.5":refnum<vi>, "SSP 0.3":refnum<vi>, "Warning":refnum<vi>, "gui GIF":refnum<vi>, "Communication is established":refnum<vi>, "AppLoad 4":refnum<vi>, "Multipoint":refnum<vi>, "Load Selection":refnum<vi>}, "PID":cluster{"Ramp":refnum<vi>, "Vertical load (N)":refnum<vi>, "apply load":refnum<vi>, "apply load 2":refnum<vi>, "Enter ByPass Load":refnum<vi>, "Bypass Load":refnum<vi>, "gFF Rot":refnum<vi>}, "Config Parameters":cluster{"Tab Control 3":refnum<vi>, "Tab Control 19":refnum<vi>, "SAMPLES":refnum<vi>, "Re-initilaize":refnum<vi>, "Filter ON/OFF":refnum<vi>, "TracHomeSurgeOffsetCounts 10MM":refnum<vi>, "TracHomeSwayOffsetCounts 10MM":refnum<vi>, "Acoustic Emission:":refnum<vi>, "Apply Filter (FF)":refnum<vi>, "Filter% 2":refnum<vi>, "Apply Filter (Load)":refnum<vi>, "Filter% ":refnum<vi>, "Sway distance (mm)":refnum<vi>, "Surge distance (mm)":refnum<vi>, "DataSavingLoopDelay(ms)":refnum<vi>, "SAVE 2":refnum<vi>, "Enter Distance":refnum<vi>, "Sway Counts:":refnum<vi>, "Distance (mm): 3":refnum<vi>, "Surge Counts:":refnum<vi>, "Distance (mm): 2":refnum<vi>, "Distance (mm):":refnum<vi>, "Heave Counts:":refnum<vi>, "LRMHomeSurgeOffsetCounts":refnum<vi>, "LRMHomeSwayOffsetCounts":refnum<vi>, "TracHomeSurgeOffsetCounts 20MM":refnum<vi>, "TracHomeSwayOffsetCounts 20MM":refnum<vi>, "RotHomeSwayOffsetCounts":refnum<vi>, "RotHomeSurgeOffsetCounts":refnum<vi>, "Heave distance":refnum<vi>, "Zmm":refnum<vi>, "Heave Pulses/mm":refnum<vi>, "Surge Pulses/mm":refnum<vi>, "Sway Pulses/mm":refnum<vi>, "Heave Pitch":refnum<vi>, "Surge Pitch":refnum<vi>, "Sway Pitch":refnum<vi>, "Heave PPR":refnum<vi>, "Surge PPR":refnum<vi>, "Sway PPR":refnum<vi>, "Tab Control 5":refnum<vi>, "Tab Control 14":refnum<vi>, "Tab Control 26":refnum<vi>, "AE":refnum<vi>, "Heave Loop Delay":refnum<vi>, "Heave PID Speed":refnum<vi>, "Surge Jog Speed":refnum<vi>, "Heave Jog Speed":refnum<vi>, "Sway Loop Delay":refnum<vi>, "Sway PID Speed":refnum<vi>, "Sway Jog Speed":refnum<vi>, "DEPTH TRIP VALUE":refnum<vi>, "LOAD TRIP VALUE":refnum<vi>, "DEPTH TRIP   ENABLE":refnum<vi>, "LOAD TRIP  ENABLE":refnum<vi>, "CYCLIC FF TRIP VALUE":refnum<vi>, "FF TRIP VALUE":refnum<vi>, "CYCLIC CoF TRIP VALUE":refnum<vi>, "COF TRIP VALUE":refnum<vi>, "CYCLIC COF TRIP  ENABLE":refnum<vi>, "CYCLIC FF TRIP  ENABLE":refnum<vi>, "FF TRIP  ENABLE":refnum<vi>, "COF TRIP  ENABLE":refnum<vi>, "JOG TRIP LOAD VALUE (N)":refnum<vi>, "Rotary Vertical":refnum<vi>, "Traction":refnum<vi>, "Scratch":refnum<vi>, "LRM CAM":refnum<vi>, "Sway LRM":refnum<vi>, "Rotary Horizontal":refnum<vi>, "SURGE SPEED":refnum<vi>, "SURGE BACKWARD COUNT":refnum<vi>, "SURGE FORWARD COUNT":refnum<vi>, "Start Button":refnum<vi>}, "Loading Com Port":cluster{"ClearAll":refnum<vi>, "Mz(Nm)":refnum<vi>, "My(Nm)":refnum<vi>, "Mx(Nm)":refnum<vi>, "Save Dwell":refnum<vi>, "Acq Delay (ms)":refnum<vi>, "Burst Delay (ms)":refnum<vi>, "model":refnum<vi>, "SN":refnum<vi>, "FFx(N)":refnum<vi>, "Sensor IP":refnum<vi>, "Port":refnum<vi>, "FFy(N)":refnum<vi>, "Load(N)":refnum<vi>, "delete Handle":refnum<vi>, "Create Handle":refnum<vi>, "ft_data":refnum<vi>, "ft_range":refnum<vi>, "ft_data 2":refnum<vi>, "stop 6":refnum<vi>, "running_flag":refnum<vi>, "ft_udp_handle":refnum<vi>, "get-data-return":refnum<vi>, "get-range-return":refnum<vi>, "zero-return":refnum<vi>, "filter-return":refnum<vi>, "initial-return":refnum<vi>, "deleteHandle-result":refnum<vi>, "Load Cell Temp":refnum<vi>, "Load Cell":refnum<vi>, "ZeroAll":refnum<vi>, "FORCE (N)":refnum<vi>, "TORQUE (N-m)":refnum<vi>, "Load Cell Link":refnum<vi>}, "Heave AND Surge":cluster{"SURGE POSE":refnum<vi>, "error out Read":refnum<vi>, "HEAVE POSE":refnum<vi>, "State":refnum<vi>, "Homed":refnum<vi>, "Sequence ID":refnum<vi>, "error out Write":refnum<vi>, "faultCode":refnum<vi>, "Ack ID":refnum<vi>, "SPEED":refnum<vi>, "Distance":refnum<vi>, "Mode Command":refnum<vi>, "Heave and Surge Read":refnum<vi>, "Read Heave Temp":refnum<vi>, "Spare 15":refnum<vi>, "Spare 14":refnum<vi>, "Spare 13":refnum<vi>, "Spare 12":refnum<vi>, "Spare 11":refnum<vi>, "Spare 10":refnum<vi>, "Spare 9":refnum<vi>, "Spare 8":refnum<vi>, "Spare 7":refnum<vi>, "Spare 4":refnum<vi>, "Spare 3":refnum<vi>, "Spare 2":refnum<vi>, "Humidity":refnum<vi>, "Temp":refnum<vi>, "Node Id":refnum<vi>, "Spare 1":refnum<vi>, "SPARE 4":refnum<vi>, "SPARE 3":refnum<vi>, "SPARE 2":refnum<vi>, "SPARE 1":refnum<vi>, "fwMajor":refnum<vi>, "fwMinor":refnum<vi>, "Manual Write":refnum<vi>, "Heave and Surge Write":refnum<vi>, "SPARE 5":refnum<vi>, "Reserved ":refnum<vi>, "SPARE 8":refnum<vi>, "SPARE 6":refnum<vi>, "SPARE 7":refnum<vi>, "SPARE 17":refnum<vi>, "SPARE 16":refnum<vi>, "SPARE 15":refnum<vi>, "SPARE 14":refnum<vi>, "SPARE 13":refnum<vi>, "SPARE 12":refnum<vi>, "SPARE 11":refnum<vi>, "SPARE 10":refnum<vi>, "SPARE 9":refnum<vi>, "System UPTIME":refnum<vi>, "Missed Packets":refnum<vi>, "faultCode Surge Right":refnum<vi>, "faultCode Surge Left":refnum<vi>, "faultCode Heave":refnum<vi>, "UPLINK HEAVE":refnum<vi>, "DOWNLINK HEAVE":refnum<vi>}, "New PID LOGIC":cluster{"Fine Tune Zone":refnum<vi>, "PID SDelay":refnum<vi>, "Max_pos_limit":refnum<vi>, "Min_pos_limit":refnum<vi>, "i_limit":refnum<vi>, "pct_scale":refnum<vi>, "Deadband":refnum<vi>, "Kd":refnum<vi>, "Ki":refnum<vi>, "Kp":refnum<vi>, "Current Position":refnum<vi>, "Set Load":refnum<vi>, "Current Load":refnum<vi>, "Pulse delta":refnum<vi>, "Init Step":refnum<vi>, "Max Step Linit":refnum<vi>, "min_deadband_floor":refnum<vi>, "dynamic_spindle_noise_scalar":refnum<vi>, "min_finetune_floor":refnum<vi>, "filter_alpha":refnum<vi>, "PID":refnum<vi>}, "SWAY ":cluster{"fwMajor":refnum<vi>, "Homed":refnum<vi>, "Rotary POSE":refnum<vi>, "State":refnum<vi>, "SWAY POSE":refnum<vi>, "Ack ID":refnum<vi>, "faultCode":refnum<vi>, "Node Id":refnum<vi>, "fwMinor":refnum<vi>, "Spare 6":refnum<vi>, "Spare 5":refnum<vi>, "Spare 4":refnum<vi>, "Spare 3":refnum<vi>, "Spare 2":refnum<vi>, "Spare 1":refnum<vi>, "Spare 7":refnum<vi>, "SPARE  5":refnum<vi>, "error out Write  SWAY ":refnum<vi>, "error out Read SWAY ":refnum<vi>, "Manual Write SWAY ":refnum<vi>, "SWAY WRITE":refnum<vi>, "SPARE  4":refnum<vi>, "SPARE  3":refnum<vi>, "SPARE 2":refnum<vi>, "SPARE 1":refnum<vi>, "Spare 15":refnum<vi>, "Spare 14":refnum<vi>, "Spare 13":refnum<vi>, "Spare 12":refnum<vi>, "Spare 11":refnum<vi>, "Spare 9":refnum<vi>, "Spare 8":refnum<vi>, "SPEED":refnum<vi>, "Distance":refnum<vi>, "Mode Command":refnum<vi>, "Sequence ID":refnum<vi>, "SWAY READ":refnum<vi>, "Spare 10":refnum<vi>, "Read SWAY Temp":refnum<vi>, "faultCode Sway ":refnum<vi>, "Missed Packets":refnum<vi>, "System UPTIME sway":refnum<vi>, "SPARE 6":refnum<vi>, "SPARE 7":refnum<vi>, "SPARE 9":refnum<vi>, "SPARE 11":refnum<vi>, "SPARE 10":refnum<vi>, "SPARE 8":refnum<vi>, "SPARE 13":refnum<vi>, "SPARE 12":refnum<vi>, "SPARE 17":refnum<vi>, "SPARE 16":refnum<vi>, "SPARE 15":refnum<vi>, "SPARE 14":refnum<vi>, "Reserved":refnum<vi>, "faultCode Rotary":refnum<vi>, "UPLINK SWAY":refnum<vi>, "DOWNLINK SWAY":refnum<vi>}, "Analysis Screen":cluster{"Analysis Home":refnum<vi>, "Refresh 2":refnum<vi>, "MEAN 4":refnum<vi>, "SD 4":refnum<vi>, "VARIANCE 4":refnum<vi>, "MEAN  3":refnum<vi>, "SD  3":refnum<vi>, "VARIANCE  3":refnum<vi>, "MEAN 2":refnum<vi>, "SD  2":refnum<vi>, "VARIANCE 2":refnum<vi>, "MEAN":refnum<vi>, "SD":refnum<vi>, "VARIANCE":refnum<vi>, "File 4 Discription":refnum<vi>, "OPEN 4":refnum<vi>, "File Name 4":refnum<vi>, "OPEN 3":refnum<vi>, "File 3 Discription":refnum<vi>, "File Name 3":refnum<vi>, "Y-AXIS":refnum<vi>, "X-AXIS":refnum<vi>, "XY Graph":refnum<vi>, "File Name 2":refnum<vi>, "File Name 1":refnum<vi>, "OPEN 2":refnum<vi>, "OPEN 1":refnum<vi>, "File 1 Discription ":refnum<vi>, "File 2 Discription":refnum<vi>, "Export":refnum<vi>, "File Format":refnum<vi>}, "Traction":cluster{"faultCode Traction 2":refnum<vi>, "faultCode Traction 1":refnum<vi>, "Missed Packets":refnum<vi>, "System UPTIME Traction":refnum<vi>, "SPARE 17":refnum<vi>, "SPARE 16":refnum<vi>, "SPARE 15":refnum<vi>, "SPARE 14":refnum<vi>, "SPARE 13":refnum<vi>, "SPARE 12":refnum<vi>, "SPARE 11":refnum<vi>, "SPARE 10":refnum<vi>, "SPARE 9":refnum<vi>, "SPARE 8":refnum<vi>, "SPARE 7":refnum<vi>, "SPARE 6":refnum<vi>, "Reserved":refnum<vi>, "SPARE  5":refnum<vi>, "Manual Write TRACTION":refnum<vi>, "TRACTION WRITE":refnum<vi>, "SPARE  4":refnum<vi>, "SPARE  3":refnum<vi>, "SPARE 2":refnum<vi>, "SPARE 1":refnum<vi>, "Spare 7":refnum<vi>, "Spare 6":refnum<vi>, "Spare 5":refnum<vi>, "Spare 4":refnum<vi>, "Spare 2":refnum<vi>, "Spare 1":refnum<vi>, "Node Id":refnum<vi>, "Read TRACTION Temp":refnum<vi>, "fwMinor":refnum<vi>, "fwMajor":refnum<vi>, "faultCode":refnum<vi>, "TRACTION POSE":refnum<vi>, "TRACTION POSE 2":refnum<vi>, "Homed":refnum<vi>, "State":refnum<vi>, "Ack ID":refnum<vi>, "SPEED":refnum<vi>, "Distance":refnum<vi>, "Mode Command":refnum<vi>, "Sequence ID":refnum<vi>, "error out Read TRACTION":refnum<vi>, "error out Write  TRACTION":refnum<vi>, "TRACTION READ":refnum<vi>, "Spare 3":refnum<vi>, "Downlink traction":refnum<vi>, "Uplink Traction":refnum<vi>}, "Traction reciepe":cluster{"SRR Sweep Range (%) Stribeck":refnum<vi>, "Traction Receipe":refnum<vi>, "Total Execution Time":refnum<vi>, "Total Steps":refnum<vi>, "Duration / Step (s)  Stribeck":refnum<vi>, "STRIBECK Fixed SRR List (%)":refnum<vi>, "Duration / Step (s) Traction":refnum<vi>, "SRR Sweep Range (%) traction":refnum<vi>, "Rolling Speed (mm/s)":refnum<vi>, "Temperature Stages (°C)":refnum<vi>, "Ball Load (N)":refnum<vi>, "Lubricant Name":refnum<vi>, "Profile File Name":refnum<vi>, "SET entrainment Velocity":refnum<vi>, "Test Array Size":refnum<vi>, "SRR INDEX [ STRIBECK]":refnum<vi>, "Stribeck Size":refnum<vi>, "SET SRR":refnum<vi>, "ELAPSED TIMER ":refnum<vi>, "BALL SET RPM":refnum<vi>, "DISC SET RPM":refnum<vi>, "SET LOAD":refnum<vi>, "TEMPERATURE READ":refnum<vi>, "SET TEMPERATURE":refnum<vi>, "Traction Size":refnum<vi>, "DISC SPEED (rpm)":refnum<vi>, "BALL SPEED (rpm)":refnum<vi>, "BALL WEAR TRACK":refnum<vi>, "DISC WEARTRACK":refnum<vi>, "SRR INDEX [ TRACTION]":refnum<vi>, "Start Index Type":refnum<vi>, "Enum - Menu":refnum<vi>, "Ball (mm/sec)":refnum<vi>, "Disc (mm/sec)":refnum<vi>, "Traction Receipe Update Details":refnum<vi>}, "Traction Control":cluster{"HomeTraction":refnum<vi>, "Demo Mode Display":refnum<vi>, "Traction Message":refnum<vi>, "Traction Step Update Details":refnum<vi>, "Main Tab sequence for selection":refnum<vi>, "Ramp Tab":refnum<vi>, "e.v/ssr":refnum<vi>, "Enter Fixed E.Velocity":refnum<vi>, "Enter Final SRR":refnum<vi>, "Enter initial SRR":refnum<vi>, "Enter Fixed SRR":refnum<vi>, "Enter the Final E.Velocity (m/s)":refnum<vi>, "Enter initial E.Velocity (m/s)":refnum<vi>, "Ball WTD":refnum<vi>, "E.Velocity":refnum<vi>, "Enter the Final Velocity (m/s)":refnum<vi>, "Enter initial Velocity (m/s)":refnum<vi>, "Ramp Up   Disc":refnum<vi>, "Initial DiscSpeed (RPM)":refnum<vi>, "Final Speed (RPM) Ball":refnum<vi>, "Final Speed (RPM)":refnum<vi>, "Initial Speed (RPM) Ball":refnum<vi>, "Enter the Final Velocity (m/s) Ball":refnum<vi>, "Enter initial Velocity (m/s) Ball":refnum<vi>, "Ramp Up":refnum<vi>, "ExceedBallSpeed step":refnum<vi>, "ExceedDiscSpeed":refnum<vi>, "BallSpeed Exceed Indication":refnum<vi>, "Apply":refnum<vi>, "SPEED SELECTION : MTM":refnum<vi>, "SPEED SELECTION : MTM 2":refnum<vi>, "TEST SELECTION (MTM)":refnum<vi>, "MTM Test Selection":refnum<vi>, "File Path Tab":refnum<vi>, "File Path String":refnum<vi>, "Save":refnum<vi>, "Save  2":refnum<vi>, "Import ":refnum<vi>, "File Path :":refnum<vi>, "Step Sequence Indication Tab":refnum<vi>, "Step Sequence Indication":refnum<vi>, "Calculate Step":refnum<vi>, "StepTable":refnum<vi>, "ExceedDiscSpeed  Cinstant Speed":refnum<vi>, "ExceedBallSpeed Constant":refnum<vi>, "TEST SELECTION (MTM) 2":refnum<vi>, "SPEED SELECTION : MTM 3":refnum<vi>, "MTM Test Selection 2":refnum<vi>, "Enter the Speed (m/sec): ":refnum<vi>, "Enter the Speed (m/sec):  2":refnum<vi>, "Enter the Speed (RPM):":refnum<vi>, "Lower Spped ":refnum<vi>, "Upper":refnum<vi>, "Enter the Speed (RPM):Ball":refnum<vi>, "Disc Motion Direction: ":refnum<vi>, "Ball Motion Direction :":refnum<vi>, "Motion Mode: ":refnum<vi>, "Wear Track Diameter (mm) ":refnum<vi>, "Disc Speed Indicator":refnum<vi>, "ExceedBallSpeed":refnum<vi>}, "Acquostic":cluster{"Last Config Rejected ":refnum<vi>, "rx command count":refnum<vi>, "Current Filter Id":refnum<vi>, "Isolated Gain":refnum<vi>, "DAQ Status":refnum<vi>, "error out":refnum<vi>, "error in (no error)":refnum<vi>, "Uplink Packet":refnum<vi>, "data out":refnum<vi>, "Downlink Packet":refnum<vi>, "Gains":refnum<vi>, "Manual Write Acquostic":refnum<vi>, "Acoustic Graphs":refnum<vi>}, "ABOUT":cluster{"version":refnum<vi>, "Operating System":refnum<vi>, "Version":refnum<vi>, "Workorder":refnum<vi>, "Runtime":refnum<vi>, "Instrument Serial":refnum<vi>, "Firmware Version":refnum<vi>, "Info":refnum<vi>}, "Temperature Port":cluster{"Temperature":refnum<vi>, "error out Temperature":refnum<vi>, "READ TEMPERATURE":refnum<vi>}}
  T22 = typedef "Traction Read enum.ctl" = enum16{"INIT", "READ", "CLOSE", "REINIT", ""}
  T23 = typedef "Traction Write enum.ctl" = enum16{"INIT", "WRITE", "CLOSE", "REINIT"}
  T24 = typedef "Heave Right enum.ctl" = enum16{"INIT", "READ", "CLOSE", "REINIT", ""}
  T25 = typedef "Heave Write enum.ctl" = enum16{"INIT", "WRITE", "CLOSE", "REINIT"}
  T26 = enum8{"Enabled", "Disabled", "Disabled and Grayed Out"}
  T27 = enum16{"open", "open or create", "create or replace", "create", "open (read-only)"}
  T28 = typedef "Load cell Enum.ctl" = enum16{"Init", "set UDP", "Read Info", "set Low Pass Filter", "Set Zero", "get data", "close", "REInit"}
  T29 = typedef "Sway Write enum.ctl" = enum16{"INIT", "WRITE", "CLOSE", "REINIT"}
  T30 = typedef "Write Main Enum.ctl" = enum16{"INIT", "WRITE", "RE-INIT", "CLOSE"}
  T31 = typedef "Temperature enum.ctl" = enum16{"Init", "read", "write", "close", "error_init"}
  T32 = typedef "Sway Right enum.ctl" = enum16{"INIT", "READ", "CLOSE", "REINIT", ""}
  T33 = typedef "Read Main Enum.ctl" = enum16{"INIT", "READ", "RE-INIT", "CLOSE"}
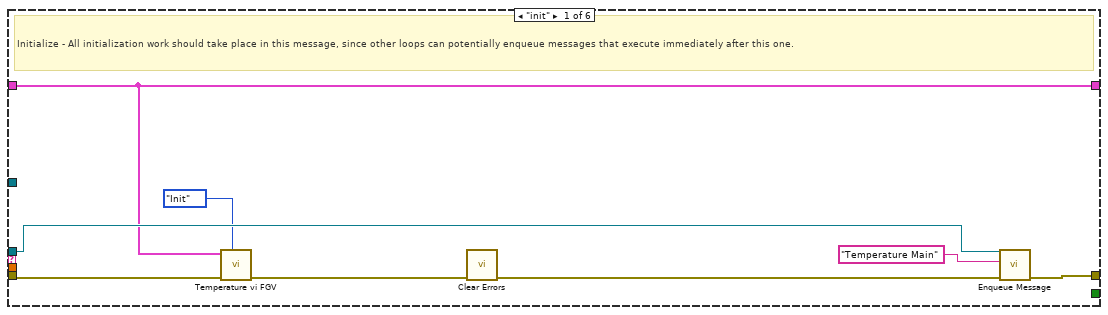
[diagram p2: hidden frame]
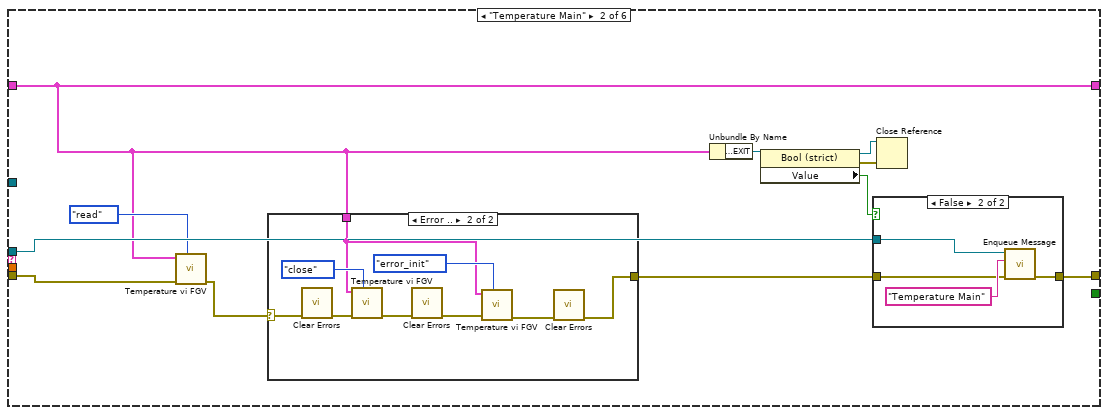
[diagram p3: hidden frame]
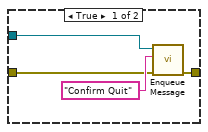
[diagram p5: hidden frame]
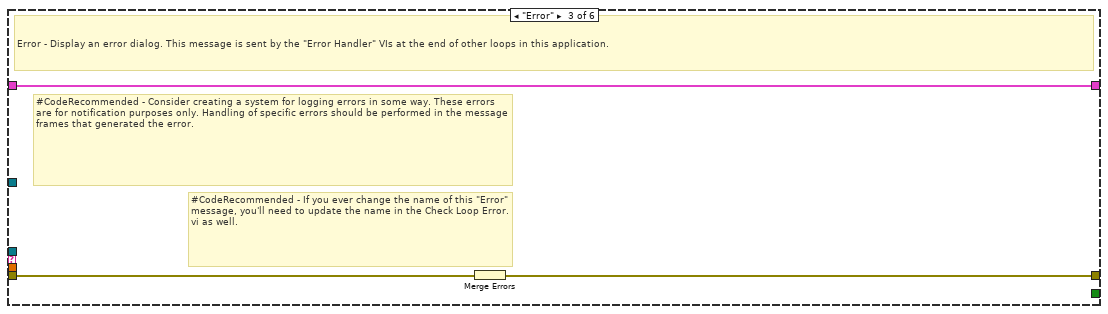
[diagram p6: hidden frame]
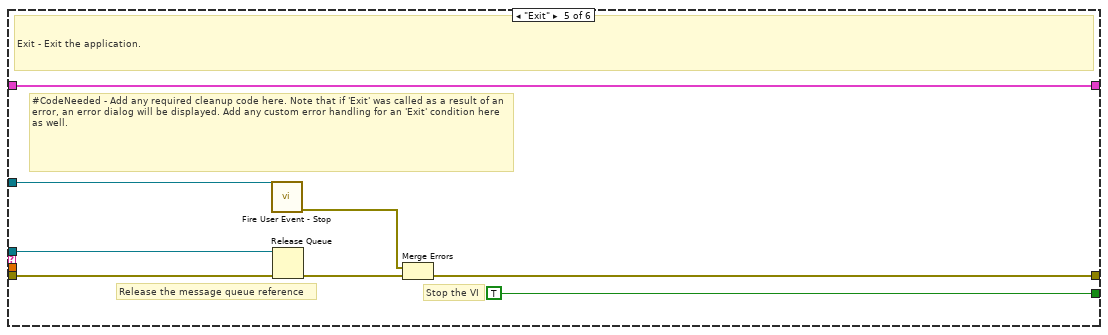
[diagram p7: hidden frame]
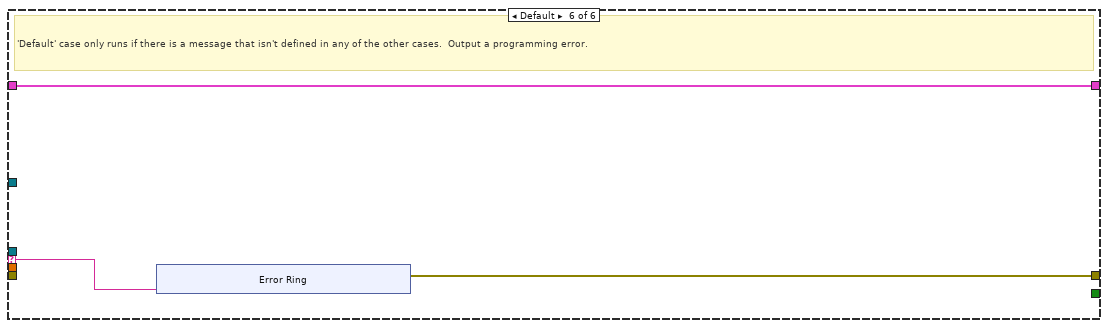
[diagram p8: hidden frame]
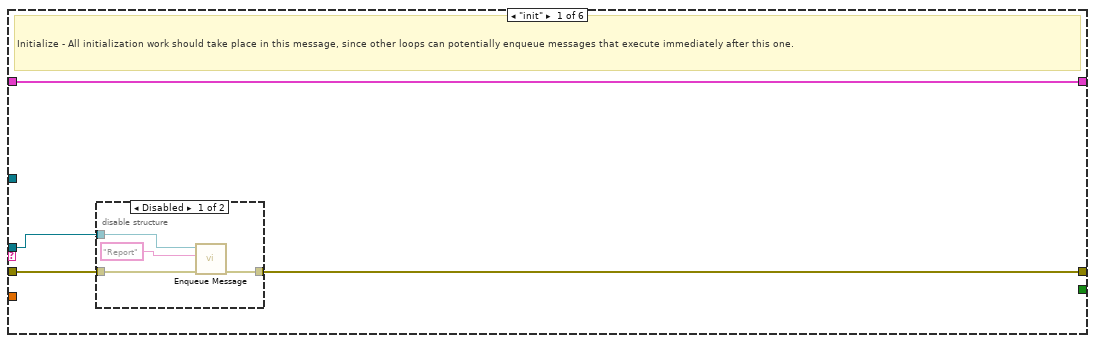
[diagram p9: hidden frame]
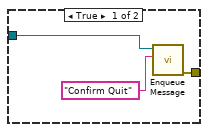
[diagram p11: hidden frame]
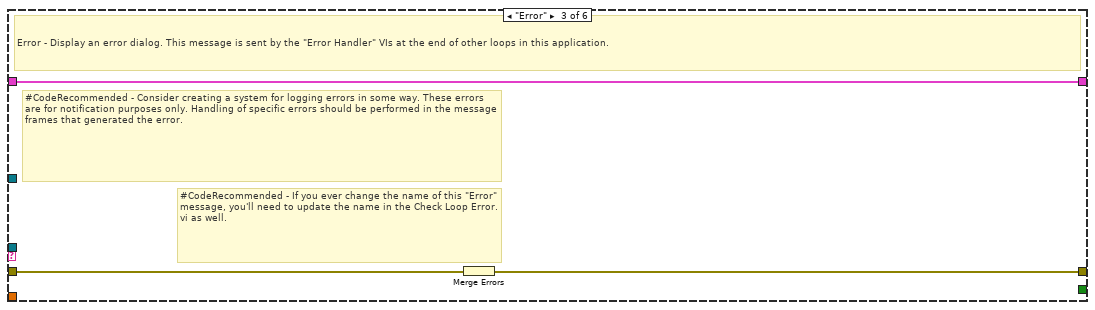
[diagram p12: hidden frame]
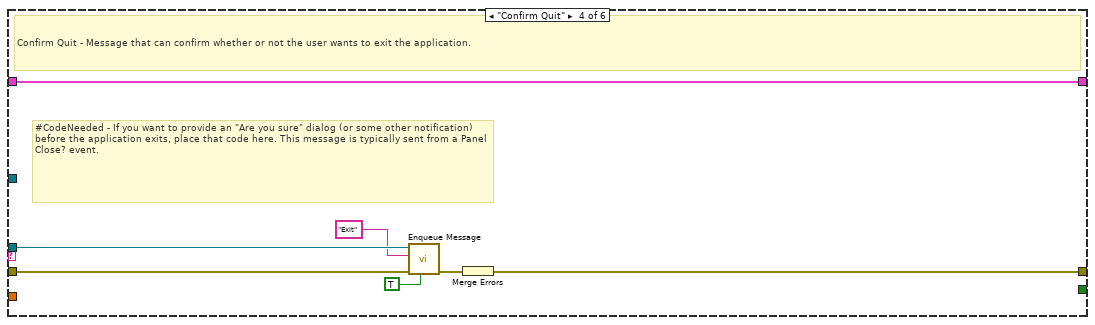
[diagram p13: hidden frame]
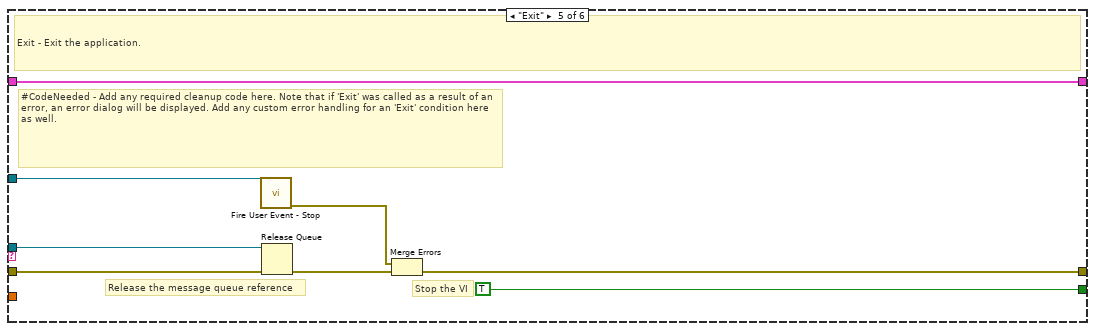
[diagram p14: hidden frame]
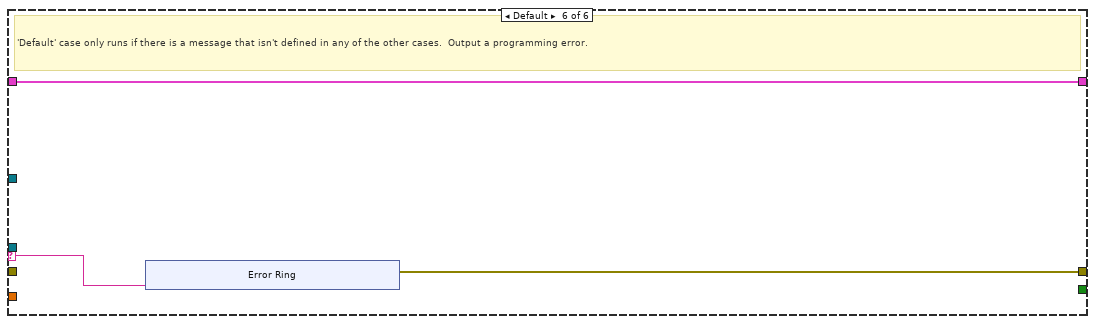
[diagram p15: hidden frame]
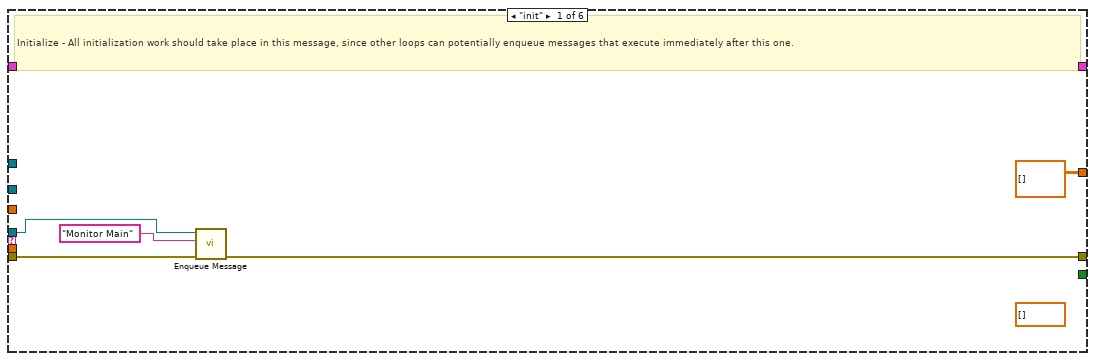
[diagram p16: hidden frame]
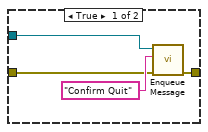
[diagram p17: hidden frame]
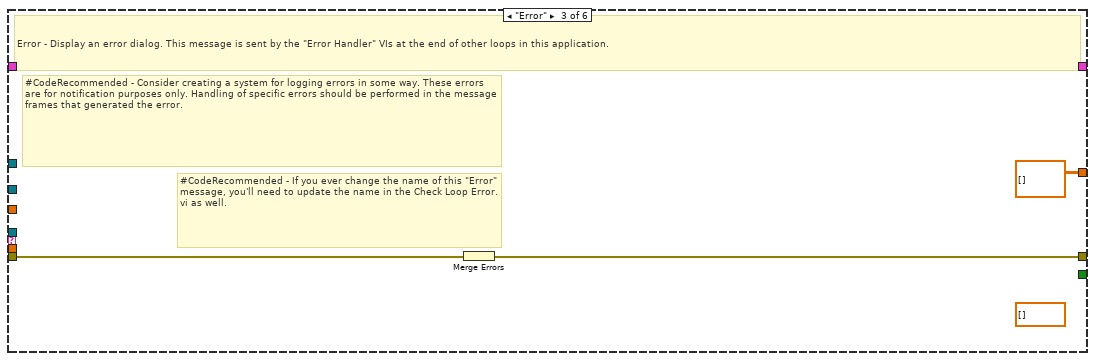
[diagram p18: hidden frame]
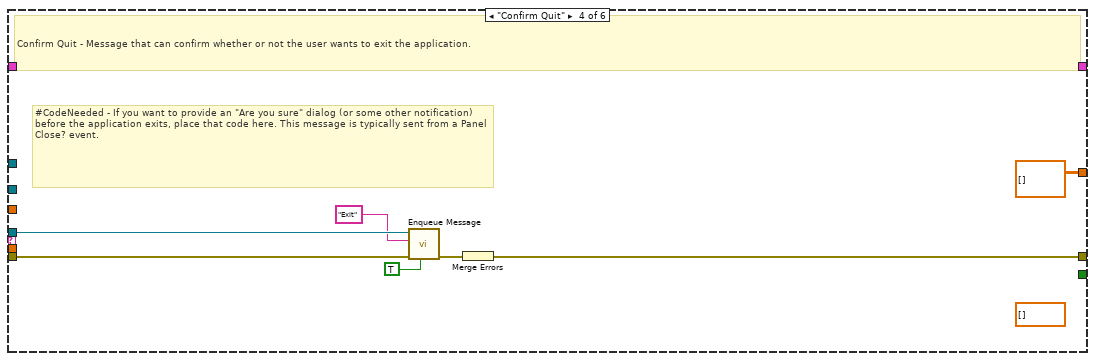
[diagram p19: hidden frame]
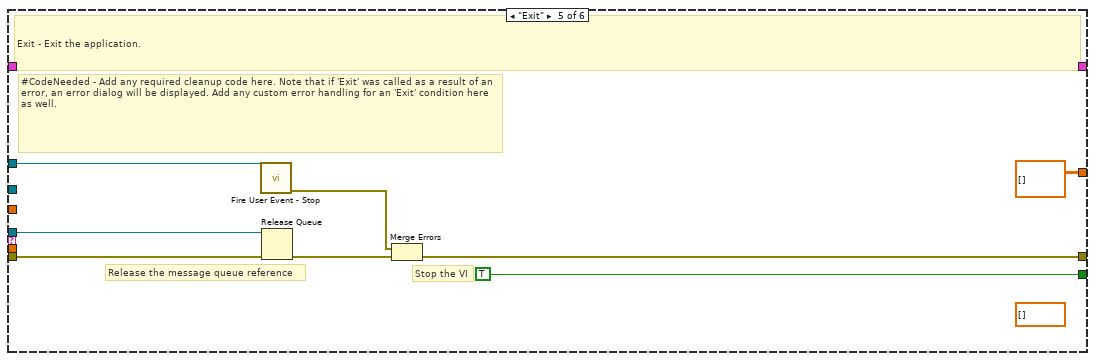
[diagram p20: hidden frame]
diagram:
  w59 = 0.0 ("prev_error_out")
  n1 = flat-sequence {
    tunnel: [w98] -> w87
    tunnel: T21 {"Main Home Screen"={"GUI"=refnum, "Platform Settings"=refnum, "Configure"=refnum, "Home"=refnum, "EXIT"=refnum, "service 2"=refnum, "MainPage"=refnum, "Analysis"=refnum}, "Platform Settings"={"mm/s  Surge"=refnum, "Drive Error"=refnum, "Disable Axis Jog Soft Limits"=refnum, "mm/s  Sway"=refnum, "Sway and Surge COM Status"=refnum, "Heave COM Status"=refnum, "Enable Platform"=refnum, "Surge Forward Main"=refnum, "Sway Right Main"=refnum, "Sway Left Main"=refnum, "Heave Down Main"=refnum, "Heave Up main"=refnum, "mm/s Heave"=refnum, "mm/sec"=refnum, "mm"=refnum, "Surge Backward Main"=refnum}, "Analysis Screen"={"Analysis Home"=refnum, "Surface Analysis"=refnum, "Imaging"=refnum, "Image Analysis"=refnum, "Post Analysis"=refnum}, "Config Screen"={"Select Load Head"=refnum, "Notes :"=refnum, "FILE"=refnum, "Sample ID :"=refnum, "Operator ID :"=refnum, "Operator Name :"=refnum, "Auto"=refnum}, "Motion Module"={"zNL"=refnum, "NL disp"=refnum, "Rotary Tab"=refnum, "Motion Direction:  3"=refnum, "E.Velocity 2"=refnum, "e.v/ssr 2"=refnum, "Enter Fixed E.Velocity 2"=refnum, "Enter Final SRR 2"=refnum, "Enter initial SRR 2"=refnum, "Enter Fixed SRR 2"=refnum, "Enter the Final E.Velocity (m/s) 2"=refnum, "Enter initial E.Velocity (m/s) 2"=refnum, "Final Speed (RPM) 3"=refnum, "Initial Speed (RPM) 2"=refnum, "Enter the Final Velocity (m/s) 3"=refnum, "Enter initial Velocity (m/s)  3"=refnum, "Ramp Up 2"=refnum, "TEST SELECTION"=refnum, "SPEED SELECTION : "=refnum, "Angular Oscillation Set"=refnum, "Traction"=refnum, "Step Speed"=refnum, "StepTable For Load-Speed"=refnum, "StepTable For Speed"=refnum, "Surge Forward MM"=refnum, "Surge Backward MM"=refnum, "M3 Image"=refnum, "String 39"=refnum, "Sway Left MM"=refnum, "Sway Right MM"=refnum, "Disable Axis Jog Soft Limits"=refnum, "mm"=refnum, "Heave Down MM"=refnum, "Heave Up MM"=refnum, "Wear Track Diameter (mm)"=refnum, "Set WTD"=refnum, "HomeScratch"=refnum, "HomeRot"=refnum, "PlaceModule"=refnum, "Enter the Angle (Deg)"=refnum, "Enter the Frequency (Hz)"=refnum, "Motion Mode:"=refnum, "LR Sway"=refnum, "Rot Hor"=refnum, "Scratch"=refnum, "LR Cam"=refnum, "MMBack"=refnum, "MMNext"=refnum, "Rot Ver"=refnum, "Rotary Module Selection"=refnum, "calculate rotary"=refnum, "SPEED SELECTION : rotary"=refnum, "Import 2"=refnum, "Save 2"=refnum, "File Path :  2"=refnum, "String 45"=refnum, "StepTable For Speed 3"=refnum, "Enter the Speed(mm/sec)"=refnum, "Enter the Speed(RPM)"=refnum, "Enter Scratch Speed (mm/s):"=refnum, "SwaySpeed Set"=refnum, "Scartch Offset"=refnum, "Motion type:"=refnum, "HomeScratch 2"=refnum, "Enter Scratch length (mm):"=refnum, "Wear Track Diameter"=refnum, "Rotary Speed Exced"=refnum, "Scratch Mode"=refnum, "No of Scratch"=refnum}, "Environmental control"={"Humidity  Status  3"=refnum, "Low Temp  Status  2"=refnum, "TK4 status 2"=refnum, "Stage Temperature"=refnum, "Sample Temperature"=refnum, "Humidity (Amb)"=refnum, "Clear List"=refnum, "Add to list"=refnum, "Wear"=refnum, "Vibration"=refnum, "Humidity (Chamber)"=refnum, "Temperature (Chamber)"=refnum, "ECR "=refnum, "Temperature (Amb)"=refnum, "Microphone"=refnum, "Acoustic Emission 3"=refnum, "SNext"=refnum, "APBack"=refnum, "Enter the Temperature (°C):"=refnum, "Enter the Stage \nTemperature (°C):"=refnum, "Enter the Humidity (%Rh):"=refnum, "Low Temp"=refnum, "High Temp"=refnum, "Humidity"=refnum, "Sensors Picked"=refnum}, "About Screen"={"Password"=refnum, "Home Service"=refnum, "Advanced Setting"=refnum, "About Tab"=refnum, "ECR Port:"=refnum, "Ramp Port:"=refnum, "Installation/Replacement completed"=refnum, "Loahead"=refnum, "Heave and Surge COM Port:"=refnum, "Sway COM Port:"=refnum, "Temp Modbus:"=refnum, "Humidity Port:"=refnum, "Edit Gain Constants"=refnum, "Save Gain Constants"=refnum}, "Main Screen"={"Main Screen Tab"=refnum, "Angle and Frequency"=refnum, "Stroke (mm)"=refnum, "Angle (Deg)"=refnum, "Main Speed Tab"=refnum, "MTM MOTOR DISPLAY"=refnum, "Disc Speed (m/sec)"=refnum, "Ball Speed (m/sec)"=refnum, "Disc Speed (RPM)"=refnum, "Ball Speed (RPM)"=refnum, "SPEED TAB"=refnum, "Speed (m/sec)"=refnum, "Set Speed (m/sec)"=refnum, "Speed (RPM)"=refnum, "Set Speed"=refnum, "Time Tab"=refnum, "Time ( HH:MM:SS ) 2"=refnum, "Test Duration"=refnum, "Test Duration 4"=refnum, "TEST CYCLE"=refnum, "TOTAL CYCLES"=refnum, "Set Load (N)"=refnum, "Temp Tabs"=refnum, "Heater"=refnum, "TK4 status"=refnum, "ChamberTemp"=refnum, "SetTmp"=refnum, "Controller  Status"=refnum, "ChamberTemp 2"=refnum, "SetTmp 2"=refnum, "Controller  Status 2"=refnum, "ChamberTemp 3"=refnum, "SetTmp 3"=refnum, "Cooling"=refnum, "Load Communication"=refnum, "Ambient \nTemperature"=refnum, "HumCOMStatus"=refnum, "Ambient\n Humidity"=refnum, "Freq (Hz)"=refnum, "Load En"=refnum, "NLt"=refnum, "zNL 2"=refnum, "Humidity On"=refnum, "humidity disp"=refnum, "Set Humidity"=refnum, "NL disp 2"=refnum, "Humidity On 2"=refnum, "humidity disp 2"=refnum, "Set Humidity 2"=refnum, "NL disp 3"=refnum, "AppLoadSeq scratch"=refnum, "Stop Scratch"=refnum, "ClrLog"=refnum, "Trip Log"=refnum, "STOP"=refnum, "Start Test"=refnum, "Test status"=refnum, "AR Led"=refnum, "Data"=refnum, "Health"=refnum, "Sway COM Status"=refnum, "Heave COM Status"=refnum, "Grp Tab"=refnum, "Sub Graph"=refnum, "SD (mm)"=refnum, "Siliding distance Reset Graph"=refnum, "SDGp"=refnum, "Humidity Reset Graph"=refnum, "HumrGp"=refnum, "Acoustic Emission (mV)"=refnum, "Aqucostic Reset Graph"=refnum, "gACQUOS"=refnum, "ECR RESET"=refnum, "ECR"=refnum, "Temperature Reset"=refnum, "Acoustic Emission (mV) 2"=refnum, "Aqucostic Reset Graph 2"=refnum, "gACQUOS 2"=refnum, "ECR RESET 2"=refnum, "ECR 2"=refnum, "Temperature Reset 2"=refnum, "Temperature (deg c)"=refnum, "Speed Reset Graph"=refnum, "Speed Tab"=refnum, "MTM DISC  SPEED"=refnum, "MTM BALL SPEED"=refnum, "speed mm/sec"=refnum, "Hymidity"=refnum, "Humidity Disable trip"=refnum, "CoF Trip  2"=refnum, "Depth Trip"=refnum, "Weart Deapth"=refnum, "Depth Reset Graph"=refnum, "Weart"=refnum, "Depthz"=refnum, "Depth (µm)"=refnum, "WearGp"=refnum, "NL Trip 2"=refnum, "Load pid"=refnum, "Load Disable Trip"=refnum, "Load Reset Graph"=refnum, "NL Display 4"=refnum, "Main Chart 3"=refnum, "BACK"=refnum, "Depth Trip 2"=refnum, "COF TRIP "=refnum, "Friction Force (N)"=refnum, "FF Reset Graph"=refnum, "FF Disable Trip"=refnum, "FF TRIP"=refnum, "COF Disable Trip"=refnum, "COF Reset Graph"=refnum, "Start Test Temp"=refnum, "zFF"=refnum, "Friction Force (N) Graph"=refnum, "Coefficient of Friction"=refnum, "Scratch Start Test"=refnum, "FF Tab"=refnum, "Cyclic Friction Force (N)"=refnum, "CZ FF"=refnum, "Cyclic Friction Force (N) Graph"=refnum, "Cyclic Coefficient of Friction"=refnum, "Cyclic FF TRIP"=refnum, "Cyclic FF Disable Trip"=refnum, "cyclic COF Disable Trip"=refnum, "cyclic COF TRIP"=refnum, "cyclic COF Reset Graph"=refnum, "Cyclic FF Reset Graph"=refnum, "Test Trip"=refnum, "Multi Scratch Pass"=refnum, "Scratch Start Recording"=refnum, "Coefficient of Friction 2"=refnum, "Acoustic Emission"=refnum, "Friction Force (N) 2"=refnum, "Depth (Microns)"=refnum, "Normal Load ( N )"=refnum}, "Loading"={"Indentation"=refnum, "Reference Sample"=refnum, "Load Cell Communication Slide"=refnum, "com 3"=refnum, "com"=refnum, "DecaForce COM Status"=refnum, "Update"=refnum, "Clear 3"=refnum, "seq"=refnum, "Stribeck table"=refnum, "Stribeck Table  For loading"=refnum, "Loading Mode"=refnum, "Enter the Final Load (N)"=refnum, "Enter the CoF Trip"=refnum, "Enter the Friction Force Trip"=refnum, "Enter the Normal load Trip"=refnum, "Enter the Load  (N)"=refnum, "KiloForce"=refnum, "DecaForce "=refnum, "MicroForce"=refnum, "LHBack"=refnum, "LHNext"=refnum, "Enter the Loading Rate (N/min)"=refnum, "Message"=refnum, "Warning 2"=refnum, "SSP 0.75"=refnum, "SSP 0.5"=refnum, "SSP 0.3"=refnum, "Warning"=refnum, "gui GIF"=refnum, "Communication is established"=refnum, "AppLoad 4"=refnum, "Multipoint"=refnum, "Load Selection"=refnum}, "PID"={"Ramp"=refnum, "Vertical load (N)"=refnum, "apply load"=refnum, "apply load 2"=refnum, "Enter ByPass Load"=refnum, "Bypass Load"=refnum, "gFF Rot"=refnum}, "Config Parameters"={"Tab Control 3"=refnum, "Tab Control 19"=refnum, "SAMPLES"=refnum, "Re-initilaize"=refnum, "Filter ON/OFF"=refnum, "TracHomeSurgeOffsetCounts 10MM"=refnum, "TracHomeSwayOffsetCounts 10MM"=refnum, "Acoustic Emission:"=refnum, "Apply Filter (FF)"=refnum, "Filter% 2"=refnum, "Apply Filter (Load)"=refnum, "Filter% "=refnum, "Sway distance (mm)"=refnum, "Surge distance (mm)"=refnum, "DataSavingLoopDelay(ms)"=refnum, "SAVE 2"=refnum, "Enter Distance"=refnum, "Sway Counts:"=refnum, "Distance (mm): 3"=refnum, "Surge Counts:"=refnum, "Distance (mm): 2"=refnum, "Distance (mm):"=refnum, "Heave Counts:"=refnum, "LRMHomeSurgeOffsetCounts"=refnum, "LRMHomeSwayOffsetCounts"=refnum, "TracHomeSurgeOffsetCounts 20MM"=refnum, "TracHomeSwayOffsetCounts 20MM"=refnum, "RotHomeSwayOffsetCounts"=refnum, "RotHomeSurgeOffsetCounts"=refnum, "Heave distance"=refnum, "Zmm"=refnum, "Heave Pulses/mm"=refnum, "Surge Pulses/mm"=refnum, "Sway Pulses/mm"=refnum, "Heave Pitch"=refnum, "Surge Pitch"=refnum, "Sway Pitch"=refnum, "Heave PPR"=refnum, "Surge PPR"=refnum, "Sway PPR"=refnum, "Tab Control 5"=refnum, "Tab Control 14"=refnum, "Tab Control 26"=refnum, "AE"=refnum, "Heave Loop Delay"=refnum, "Heave PID Speed"=refnum, "Surge Jog Speed"=refnum, "Heave Jog Speed"=refnum, "Sway Loop Delay"=refnum, "Sway PID Speed"=refnum, "Sway Jog Speed"=refnum, "DEPTH TRIP VALUE"=refnum, "LOAD TRIP VALUE"=refnum, "DEPTH TRIP   ENABLE"=refnum, "LOAD TRIP  ENABLE"=refnum, "CYCLIC FF TRIP VALUE"=refnum, "FF TRIP VALUE"=refnum, "CYCLIC CoF TRIP VALUE"=refnum, "COF TRIP VALUE"=refnum, "CYCLIC COF TRIP  ENABLE"=refnum, "CYCLIC FF TRIP  ENABLE"=refnum, "FF TRIP  ENABLE"=refnum, "COF TRIP  ENABLE"=refnum, "JOG TRIP LOAD VALUE (N)"=refnum, "Rotary Vertical"=refnum, "Traction"=refnum, "Scratch"=refnum, "LRM CAM"=refnum, "Sway LRM"=refnum, "Rotary Horizontal"=refnum, "SURGE SPEED"=refnum, "SURGE BACKWARD COUNT"=refnum, "SURGE FORWARD COUNT"=refnum, "Start Button"=refnum}, "Loading Com Port"={"ClearAll"=refnum, "Mz(Nm)"=refnum, "My(Nm)"=refnum, "Mx(Nm)"=refnum, "Save Dwell"=refnum, "Acq Delay (ms)"=refnum, "Burst Delay (ms)"=refnum, "model"=refnum, "SN"=refnum, "FFx(N)"=refnum, "Sensor IP"=refnum, "Port"=refnum, "FFy(N)"=refnum, "Load(N)"=refnum, "delete Handle"=refnum, "Create Handle"=refnum, "ft_data"=refnum, "ft_range"=refnum, "ft_data 2"=refnum, "stop 6"=refnum, "running_flag"=refnum, "ft_udp_handle"=refnum, "get-data-return"=refnum, "get-range-return"=refnum, "zero-return"=refnum, "filter-return"=refnum, "initial-return"=refnum, "deleteHandle-result"=refnum, "Load Cell Temp"=refnum, "Load Cell"=refnum, "ZeroAll"=refnum, "FORCE (N)"=refnum, "TORQUE (N-m)"=refnum, "Load Cell Link"=refnum}, "Heave AND Surge"={"SURGE POSE"=refnum, "error out Read"=refnum, "HEAVE POSE"=refnum, "State"=refnum, "Homed"=refnum, "Sequence ID"=refnum, "error out Write"=refnum, "faultCode"=refnum, "Ack ID"=refnum, "SPEED"=refnum, "Distance"=refnum, "Mode Command"=refnum, "Heave and Surge Read"=refnum, "Read Heave Temp"=refnum, "Spare 15"=refnum, "Spare 14"=refnum, "Spare 13"=refnum, "Spare 12"=refnum, "Spare 11"=refnum, "Spare 10"=refnum, "Spare 9"=refnum, "Spare 8"=refnum, "Spare 7"=refnum, "Spare 4"=refnum, "Spare 3"=refnum, "Spare 2"=refnum, "Humidity"=refnum, "Temp"=refnum, "Node Id"=refnum, "Spare 1"=refnum, "SPARE 4"=refnum, "SPARE 3"=refnum, "SPARE 2"=refnum, "SPARE 1"=refnum, "fwMajor"=refnum, "fwMinor"=refnum, "Manual Write"=refnum, "Heave and Surge Write"=refnum, "SPARE 5"=refnum, "Reserved "=refnum, "SPARE 8"=refnum, "SPARE 6"=refnum, "SPARE 7"=refnum, "SPARE 17"=refnum, "SPARE 16"=refnum, "SPARE 15"=refnum, "SPARE 14"=refnum, "SPARE 13"=refnum, "SPARE 12"=refnum, "SPARE 11"=refnum, "SPARE 10"=refnum, "SPARE 9"=refnum, "System UPTIME"=refnum, "Missed Packets"=refnum, "faultCode Surge Right"=refnum, "faultCode Surge Left"=refnum, "faultCode Heave"=refnum, "UPLINK HEAVE"=refnum, "DOWNLINK HEAVE"=refnum}, "New PID LOGIC"={"Fine Tune Zone"=refnum, "PID SDelay"=refnum, "Max_pos_limit"=refnum, "Min_pos_limit"=refnum, "i_limit"=refnum, "pct_scale"=refnum, "Deadband"=refnum, "Kd"=refnum, "Ki"=refnum, "Kp"=refnum, "Current Position"=refnum, "Set Load"=refnum, "Current Load"=refnum, "Pulse delta"=refnum, "Init Step"=refnum, "Max Step Linit"=refnum, "min_deadband_floor"=refnum, "dynamic_spindle_noise_scalar"=refnum, "min_finetune_floor"=refnum, "filter_alpha"=refnum, "PID"=refnum}, "SWAY "={"fwMajor"=refnum, "Homed"=refnum, "Rotary POSE"=refnum, "State"=refnum, "SWAY POSE"=refnum, "Ack ID"=refnum, "faultCode"=refnum, "Node Id"=refnum, "fwMinor"=refnum, "Spare 6"=refnum, "Spare 5"=refnum, "Spare 4"=refnum, "Spare 3"=refnum, "Spare 2"=refnum, "Spare 1"=refnum, "Spare 7"=refnum, "SPARE  5"=refnum, "error out Write  SWAY "=refnum, "error out Read SWAY "=refnum, "Manual Write SWAY "=refnum, "SWAY WRITE"=refnum, "SPARE  4"=refnum, "SPARE  3"=refnum, "SPARE 2"=refnum, "SPARE 1"=refnum, "Spare 15"=refnum, "Spare 14"=refnum, "Spare 13"=refnum, "Spare 12"=refnum, "Spare 11"=refnum, "Spare 9"=refnum, "Spare 8"=refnum, "SPEED"=refnum, "Distance"=refnum, "Mode Command"=refnum, "Sequence ID"=refnum, "SWAY READ"=refnum, "Spare 10"=refnum, "Read SWAY Temp"=refnum, "faultCode Sway "=refnum, "Missed Packets"=refnum, "System UPTIME sway"=refnum, "SPARE 6"=refnum, "SPARE 7"=refnum, "SPARE 9"=refnum, "SPARE 11"=refnum, "SPARE 10"=refnum, "SPARE 8"=refnum, "SPARE 13"=refnum, "SPARE 12"=refnum, "SPARE 17"=refnum, "SPARE 16"=refnum, "SPARE 15"=refnum, "SPARE 14"=refnum, "Reserved"=refnum, "faultCode Rotary"=refnum, "UPLINK SWAY"=refnum, "DOWNLINK SWAY"=refnum}, "Analysis Screen"={"Analysis Home"=refnum, "Refresh 2"=refnum, "MEAN 4"=refnum, "SD 4"=refnum, "VARIANCE 4"=refnum, "MEAN  3"=refnum, "SD  3"=refnum, "VARIANCE  3"=refnum, "MEAN 2"=refnum, "SD  2"=refnum, "VARIANCE 2"=refnum, "MEAN"=refnum, "SD"=refnum, "VARIANCE"=refnum, "File 4 Discription"=refnum, "OPEN 4"=refnum, "File Name 4"=refnum, "OPEN 3"=refnum, "File 3 Discription"=refnum, "File Name 3"=refnum, "Y-AXIS"=refnum, "X-AXIS"=refnum, "XY Graph"=refnum, "File Name 2"=refnum, "File Name 1"=refnum, "OPEN 2"=refnum, "OPEN 1"=refnum, "File 1 Discription "=refnum, "File 2 Discription"=refnum, "Export"=refnum, "File Format"=refnum}, "Traction"={"faultCode Traction 2"=refnum, "faultCode Traction 1"=refnum, "Missed Packets"=refnum, "System UPTIME Traction"=refnum, "SPARE 17"=refnum, "SPARE 16"=refnum, "SPARE 15"=refnum, "SPARE 14"=refnum, "SPARE 13"=refnum, "SPARE 12"=refnum, "SPARE 11"=refnum, "SPARE 10"=refnum, "SPARE 9"=refnum, "SPARE 8"=refnum, "SPARE 7"=refnum, "SPARE 6"=refnum, "Reserved"=refnum, "SPARE  5"=refnum, "Manual Write TRACTION"=refnum, "TRACTION WRITE"=refnum, "SPARE  4"=refnum, "SPARE  3"=refnum, "SPARE 2"=refnum, "SPARE 1"=refnum, "Spare 7"=refnum, "Spare 6"=refnum, "Spare 5"=refnum, "Spare 4"=refnum, "Spare 2"=refnum, "Spare 1"=refnum, "Node Id"=refnum, "Read TRACTION Temp"=refnum, "fwMinor"=refnum, "fwMajor"=refnum, "faultCode"=refnum, "TRACTION POSE"=refnum, "TRACTION POSE 2"=refnum, "Homed"=refnum, "State"=refnum, "Ack ID"=refnum, "SPEED"=refnum, "Distance"=refnum, "Mode Command"=refnum, "Sequence ID"=refnum, "error out Read TRACTION"=refnum, "error out Write  TRACTION"=refnum, "TRACTION READ"=refnum, "Spare 3"=refnum, "Downlink traction"=refnum, "Uplink Traction"=refnum}, "Traction reciepe"={"SRR Sweep Range (%) Stribeck"=refnum, "Traction Receipe"=refnum, "Total Execution Time"=refnum, "Total Steps"=refnum, "Duration / Step (s)  Stribeck"=refnum, "STRIBECK Fixed SRR List (%)"=refnum, "Duration / Step (s) Traction"=refnum, "SRR Sweep Range (%) traction"=refnum, "Rolling Speed (mm/s)"=refnum, "Temperature Stages (°C)"=refnum, "Ball Load (N)"=refnum, "Lubricant Name"=refnum, "Profile File Name"=refnum, "SET entrainment Velocity"=refnum, "Test Array Size"=refnum, "SRR INDEX [ STRIBECK]"=refnum, "Stribeck Size"=refnum, "SET SRR"=refnum, "ELAPSED TIMER "=refnum, "BALL SET RPM"=refnum, "DISC SET RPM"=refnum, "SET LOAD"=refnum, "TEMPERATURE READ"=refnum, "SET TEMPERATURE"=refnum, "Traction Size"=refnum, "DISC SPEED (rpm)"=refnum, "BALL SPEED (rpm)"=refnum, "BALL WEAR TRACK"=refnum, "DISC WEARTRACK"=refnum, "SRR INDEX [ TRACTION]"=refnum, "Start Index Type"=refnum, "Enum - Menu"=refnum, "Ball (mm/sec)"=refnum, "Disc (mm/sec)"=refnum, "Traction Receipe Update Details"=refnum}, "Traction Control"={"HomeTraction"=refnum, "Demo Mode Display"=refnum, "Traction Message"=refnum, "Traction Step Update Details"=refnum, "Main Tab sequence for selection"=refnum, "Ramp Tab"=refnum, "e.v/ssr"=refnum, "Enter Fixed E.Velocity"=refnum, "Enter Final SRR"=refnum, "Enter initial SRR"=refnum, "Enter Fixed SRR"=refnum, "Enter the Final E.Velocity (m/s)"=refnum, "Enter initial E.Velocity (m/s)"=refnum, "Ball WTD"=refnum, "E.Velocity"=refnum, "Enter the Final Velocity (m/s)"=refnum, "Enter initial Velocity (m/s)"=refnum, "Ramp Up   Disc"=refnum, "Initial DiscSpeed (RPM)"=refnum, "Final Speed (RPM) Ball"=refnum, "Final Speed (RPM)"=refnum, "Initial Speed (RPM) Ball"=refnum, "Enter the Final Velocity (m/s) Ball"=refnum, "Enter initial Velocity (m/s) Ball"=refnum, "Ramp Up"=refnum, "ExceedBallSpeed step"=refnum, "ExceedDiscSpeed"=refnum, "BallSpeed Exceed Indication"=refnum, "Apply"=refnum, "SPEED SELECTION : MTM"=refnum, "SPEED SELECTION : MTM 2"=refnum, "TEST SELECTION (MTM)"=refnum, "MTM Test Selection"=refnum, "File Path Tab"=refnum, "File Path String"=refnum, "Save"=refnum, "Save  2"=refnum, "Import "=refnum, "File Path :"=refnum, "Step Sequence Indication Tab"=refnum, "Step Sequence Indication"=refnum, "Calculate Step"=refnum, "StepTable"=refnum, "ExceedDiscSpeed  Cinstant Speed"=refnum, "ExceedBallSpeed Constant"=refnum, "TEST SELECTION (MTM) 2"=refnum, "SPEED SELECTION : MTM 3"=refnum, "MTM Test Selection 2"=refnum, "Enter the Speed (m/sec): "=refnum, "Enter the Speed (m/sec):  2"=refnum, "Enter the Speed (RPM):"=refnum, "Lower Spped "=refnum, "Upper"=refnum, "Enter the Speed (RPM):Ball"=refnum, "Disc Motion Direction: "=refnum, "Ball Motion Direction :"=refnum, "Motion Mode: "=refnum, "Wear Track Diameter (mm) "=refnum, "Disc Speed Indicator"=refnum, "ExceedBallSpeed"=refnum}, "Acquostic"={"Last Config Rejected "=refnum, "rx command count"=refnum, "Current Filter Id"=refnum, "Isolated Gain"=refnum, "DAQ Status"=refnum, "error out"=refnum, "error in (no error)"=refnum, "Uplink Packet"=refnum, "data out"=refnum, "Downlink Packet"=refnum, "Gains"=refnum, "Manual Write Acquostic"=refnum, "Acoustic Graphs"=refnum}, "ABOUT"={"version"=refnum, "Operating System"=refnum, "Version"=refnum, "Workorder"=refnum, "Runtime"=refnum, "Instrument Serial"=refnum, "Firmware Version"=refnum, "Info"=refnum}, "Temperature Port"={"Temperature"=refnum, "error out Temperature"=refnum, "READ TEMPERATURE"=refnum}} ("Data Cluster") -> [w97]
    tunnel: w87 -> [w120]
    tunnel: [w107] -> w86
    tunnel: w86 -> [w127]
    tunnel: [w121] -> w85
    tunnel: w85 -> [w136]
    tunnel: [w135] -> w84
    tunnel: w84 -> [w170]
    tunnel: [w169] -> w82
    tunnel: w82 -> [w241]
    tunnel: [w240] -> w81
    tunnel: w81 -> [w268]
    tunnel: [w267] -> w80
    tunnel: w80 -> [w278]
    tunnel: [w277] -> w79
    tunnel: w79 -> [w366]
    tunnel: [w365] -> w67
    tunnel: w67 -> [w374]
    tunnel: [w373] -> w66
    tunnel: w66 -> [w444]
    tunnel: [w443] -> w65
    tunnel: w65 -> [w461]
    tunnel: [w460] -> w64
    tunnel: w64 -> [w522]
    tunnel: [w521] -> w63
    tunnel: w63 -> [w545]
    tunnel: [w544] -> w62
    tunnel: w62 -> [w605]
    tunnel: [w604] -> w60
    tunnel: w60 -> [w638]
    tunnel: [w637] -> w57
    tunnel: w57 -> [w690]
    tunnel: [w689] -> w56
    tunnel: w56 -> [w727]
    tunnel: [w726] -> w55
    tunnel: w55 -> [w787]
    tunnel: [w786] -> w49
    tunnel: w49 -> [w802]
    tunnel: [w801] -> w2
    tunnel: w2 -> [w812]
    tunnel: [w811] -> w1
    tunnel: [w816] -> w47
    tunnel: w1 -> [w817]
    frame #0 {
      # "MAIN HOME SCREEN"
      n2 = control-ref of="GUI"() -> (w106:refnum<vi>)
      n3 = control-ref of="MainPage"() -> (w100:refnum<vi>)
      n4 = control-ref of="Platform Settings"() -> (w105:refnum<vi>)
      n5 = control-ref of="Configure"() -> (w104:refnum<vi>)
      n6 = control-ref of="Home"() -> (w103:refnum<vi>)
      n7 = control-ref of="EXIT"() -> (w102:refnum<vi>)
      n8 = control-ref of="service 2"() -> (w101:refnum<vi>)
      n9 = control-ref of="Analysis"() -> (w99:refnum<vi>)
      n10 = Bundle By Name(cluster=w97, "Main Home Screen.GUI"=w106, "Main Home Screen.Platform Settings"=w105, "Main Home Screen.Configure"=w104, "Main Home Screen.Home"=w103, "Main Home Screen.EXIT"=w102, "Main Home Screen.service 2"=w101, "Main Home Screen.MainPage"=w100, "Main Home Screen.Analysis"=w99) -> (w98:T21)
    }
    frame #1 {
      # "PLATFORM SETTINGS"
      n11 = control-ref of="Disable Axis Jog Soft Limits m"() -> (w118:refnum<vi>)
      n12 = control-ref of="Sway and Surge COM Status"() -> (w117:refnum<vi>)
      n13 = control-ref of="Heave COM Status"() -> (w116:refnum<vi>)
      n14 = control-ref of="Enable Platform"() -> (w115:refnum<vi>)
      n15 = control-ref of="Surge Forward Main"() -> (w114:refnum<vi>)
      n16 = control-ref of="Sway Right Main"() -> (w113:refnum<vi>)
      n17 = control-ref of="Sway Left Main"() -> (w112:refnum<vi>)
      n18 = control-ref of="Heave Down Main"() -> (w111:refnum<vi>)
      n19 = control-ref of="Heave Up main"() -> (w110:refnum<vi>)
      n20 = control-ref of="Surge Backward Main"() -> (w108:refnum<vi>)
      n21 = control-ref of="mm"() -> (w109:refnum<vi>)
      n22 = control-ref of="Drive Error"() -> (w119:refnum<vi>)
      n23 = Bundle By Name(cluster=w120, "Platform Settings.Drive Error"=w119, "Platform Settings.Disable Axis Jog Soft Limits"=w118, "Platform Settings.Sway and Surge COM Status"=w117, "Platform Settings.Heave COM Status"=w116, "Platform Settings.Enable Platform"=w115, "Platform Settings.Surge Forward Main"=w114, "Platform Settings.Sway Right Main"=w113, "Platform Settings.Sway Left Main"=w112, "Platform Settings.Heave Down Main"=w111, "Platform Settings.Heave Up main"=w110, "Platform Settings.mm"=w109, "Platform Settings.Surge Backward Main"=w108) -> (w107:T21)
    }
    frame #2 {
      # "ANALYSIS SCREEN"
      n24 = control-ref of="Analysis Home"() -> (w126:refnum<vi>)
      n25 = control-ref of="Surface Analysis"() -> (w125:refnum<vi>)
      n26 = control-ref of="Imaging"() -> (w124:refnum<vi>)
      n27 = control-ref of="Image Analysis"() -> (w123:refnum<vi>)
      n28 = control-ref of="Post Analysis"() -> (w122:refnum<vi>)
      n29 = Bundle By Name(cluster=w127, "Analysis Screen.Analysis Home"=w126, "Analysis Screen.Surface Analysis"=w125, "Analysis Screen.Imaging"=w124, "Analysis Screen.Image Analysis"=w123, "Analysis Screen.Post Analysis"=w122) -> (w121:T21)
    }
    frame #3 {
      # "CONFIG SCREEN"
      n30 = control-ref of="Select Load Head"() -> (w134:refnum<vi>)
      n31 = control-ref of="Auto"() -> (w128:refnum<vi>)
      n32 = control-ref of="Notes :"() -> (w133:refnum<vi>)
      n33 = control-ref of="FILE"() -> (w132:refnum<vi>)
      n34 = control-ref of="Sample ID :"() -> (w131:refnum<vi>)
      n35 = control-ref of="Operator ID :"() -> (w130:refnum<vi>)
      n36 = control-ref of="Operator Name :"() -> (w129:refnum<vi>)
      n37 = Bundle By Name(cluster=w136, "Config Screen.Select Load Head"=w134, "Config Screen.Notes :"=w133, "Config Screen.FILE"=w132, "Config Screen.Sample ID :"=w131, "Config Screen.Operator ID :"=w130, "Config Screen.Operator Name :"=w129, "Config Screen.Auto"=w128) -> (w135:T21)
    }
    frame #4 {
      # "°C"
      # "LOADING SCREEN"
      n38 = control-ref of="Warning"() -> (w162:refnum<vi>)
      n39 = control-ref of="gui GIF"() -> (w161:refnum<vi>)
      n40 = control-ref of="Load Selection"() -> (w137:refnum<vi>)
      n41 = control-ref of="Warning 2"() -> (w166:refnum<vi>)
      n42 = control-ref of="SSP 0.75"() -> (w165:refnum<vi>)
      n43 = control-ref of="SSP 0.5"() -> (w164:refnum<vi>)
      n44 = control-ref of="SSP 0.3"() -> (w163:refnum<vi>)
      n45 = control-ref of="Communication is established"() -> (w160:refnum<vi>)
      n46 = control-ref of="AppLoad 4"() -> (w159:refnum<vi>)
      n47 = control-ref of="Multipoint"() -> (w158:refnum<vi>)
      n48 = control-ref of="com 3"() -> (w155:refnum<vi>)
      n49 = control-ref of="com"() -> (w154:refnum<vi>)
      n50 = control-ref of="DecaForce COM Status"() -> (w153:refnum<vi>)
      n51 = control-ref of="Clear 3"() -> (w152:refnum<vi>)
      n52 = control-ref of="seq"() -> (w151:refnum<vi>)
      n53 = control-ref of="Stribeck table"() -> (w150:refnum<vi>)
      n54 = control-ref of="KiloForce"() -> (w142:refnum<vi>)
      n55 = control-ref of="DecaForce"() -> (w141:refnum<vi>)
      n56 = control-ref of="MicroForce"() -> (w140:refnum<vi>)
      n57 = control-ref of="LHBack"() -> (w139:refnum<vi>)
      n58 = control-ref of="LHNext"() -> (w138:refnum<vi>)
      n59 = control-ref of="Enter the Loading Rate (N/min)"() -> (w168:refnum<vi>)
      n60 = control-ref of="Enter the Final Load (N)"() -> (w147:refnum<vi>)
      n61 = control-ref of="Enter the CoF Trip"() -> (w146:refnum<vi>)
      n62 = control-ref of="Enter the Friction Force Trip"() -> (w145:refnum<vi>)
      n63 = control-ref of="Enter the Normal load Trip"() -> (w144:refnum<vi>)
      n64 = control-ref of="Enter the Load  (N)"() -> (w143:refnum<vi>)
      n65 = control-ref of="Message"() -> (w167:refnum<vi>)
      n66 = control-ref of="Indentation"() -> (w157:refnum<vi>)
      n67 = control-ref of="Stribeck Table  For loading"() -> (w149:refnum<vi>)
      n68 = control-ref of="Reference Sample"() -> (w156:refnum<vi>)
      n69 = control-ref of="Loading Mode"() -> (w148:refnum<vi>)
      n70 = Bundle By Name(cluster=w170, "Loading.Enter the Loading Rate (N/min)"=w168, "Loading.Message"=w167, "Loading.Warning 2"=w166, "Loading.SSP 0.75"=w165, "Loading.SSP 0.5"=w164, "Loading.SSP 0.3"=w163, "Loading.Warning"=w162, "Loading.gui GIF"=w161, "Loading.Communication is established"=w160, "Loading.AppLoad 4"=w159, "Loading.Multipoint"=w158, "Loading.Indentation"=w157, "Loading.Reference Sample"=w156, "Loading.com 3"=w155, "Loading.com"=w154, "Loading.DecaForce COM Status"=w153, "Loading.Clear 3"=w152, "Loading.seq"=w151, "Loading.Stribeck table"=w150, "Loading.Stribeck Table  For loading"=w149, "Loading.Loading Mode"=w148, "Loading.Enter the Final Load (N)"=w147, "Loading.Enter the CoF Trip"=w146, "Loading.Enter the Friction Force Trip"=w145, "Loading.Enter the Normal load Trip"=w144, "Loading.Enter the Load  (N)"=w143, "Loading.KiloForce"=w142, "Loading.DecaForce"=w141, "Loading.MicroForce"=w140, "Loading.LHBack"=w139, "Loading.LHNext"=w138, "Loading.Load Selection"=w137) -> (w169:T21)
    }
    frame #5 {
      # "MOTION MODULE SCREEN"
      n71 = control-ref of="TEST SELECTION"() -> (w222:refnum<vi>)
      n72 = control-ref of="SPEED SELECTION :"() -> (w221:refnum<vi>)
      n73 = control-ref of="SPEED SELECTION : rotary"() -> (w188:refnum<vi>)
      n74 = control-ref of="Rotary Tab"() -> (w237:refnum<vi>)
      n75 = control-ref of="e.v/ssr 2"() -> (w234:refnum<vi>)
      n76 = control-ref of="Step Speed"() -> (w218:refnum<vi>)
      n77 = control-ref of="M3 Image"() -> (w213:refnum<vi>)
      n78 = control-ref of="Rotary Module Selection"() -> (w190:refnum<vi>)
      n79 = control-ref of="zNL"() -> (w239:refnum<vi>)
      n80 = control-ref of="E.Velocity 2"() -> (w235:refnum<vi>)
      n81 = control-ref of="Ramp Up 2"() -> (w223:refnum<vi>)
      n82 = control-ref of="Angular Oscillation Set"() -> (w220:refnum<vi>)
      n83 = control-ref of="Traction"() -> (w219:refnum<vi>)
      n84 = control-ref of="Surge Forward MM"() -> (w215:refnum<vi>)
      n85 = control-ref of="Surge Backward MM"() -> (w214:refnum<vi>)
      n86 = control-ref of="Sway Left MM"() -> (w211:refnum<vi>)
      n87 = control-ref of="Sway Right MM"() -> (w210:refnum<vi>)
      n88 = control-ref of="Disable Axis Jog Soft Limits"() -> (w209:refnum<vi>)
      n89 = control-ref of="Heave Down MM"() -> (w207:refnum<vi>)
      n90 = control-ref of="Heave Up MM"() -> (w206:refnum<vi>)
      n91 = control-ref of="Set WTD"() -> (w204:refnum<vi>)
      n92 = control-ref of="HomeScratch"() -> (w203:refnum<vi>)
      n93 = control-ref of="HomeRot"() -> (w202:refnum<vi>)
      n94 = control-ref of="PlaceModule"() -> (w201:refnum<vi>)
      n95 = control-ref of="LR Sway"() -> (w197:refnum<vi>)
      n96 = control-ref of="Rot Hor"() -> (w196:refnum<vi>)
      n97 = control-ref of="Scratch"() -> (w195:refnum<vi>)
      n98 = control-ref of="LR Cam"() -> (w194:refnum<vi>)
      n99 = control-ref of="MMBack"() -> (w193:refnum<vi>)
      n100 = control-ref of="MMNext"() -> (w192:refnum<vi>)
      n101 = control-ref of="Rot Ver"() -> (w191:refnum<vi>)
      n102 = control-ref of="calculate rotary"() -> (w189:refnum<vi>)
      n103 = control-ref of="Import 2"() -> (w187:refnum<vi>)
      n104 = control-ref of="Save 2"() -> (w186:refnum<vi>)
      n105 = control-ref of="SwaySpeed Set"() -> (w179:refnum<vi>)
      n106 = control-ref of="HomeScratch"() -> (w175:refnum<vi>)
      n107 = control-ref of="NL disp"() -> (w238:refnum<vi>)
      n108 = control-ref of="Enter Fixed E.Velocity 2"() -> (w233:refnum<vi>)
      n109 = control-ref of="Enter Final SRR 2"() -> (w232:refnum<vi>)
      n110 = control-ref of="Enter initial SRR 2"() -> (w231:refnum<vi>)
      n111 = control-ref of="Enter Fixed SRR 2"() -> (w230:refnum<vi>)
      n112 = control-ref of="Enter the Final E.Velocity (m/s) 2"() -> (w229:refnum<vi>)
      n113 = control-ref of="Enter initial E.Velocity (m/s) 2"() -> (w228:refnum<vi>)
      n114 = control-ref of="Final Speed (RPM) 3"() -> (w227:refnum<vi>)
      n115 = control-ref of="Initial Speed (RPM) 2"() -> (w226:refnum<vi>)
      n116 = control-ref of="Enter the Final Velocity (m/s) 3"() -> (w225:refnum<vi>)
      n117 = control-ref of="Enter initial Velocity (m/s)  3"() -> (w224:refnum<vi>)
      n118 = control-ref of="mm"() -> (w208:refnum<vi>)
      n119 = control-ref of="Wear Track Diameter (mm)"() -> (w205:refnum<vi>)
      n120 = control-ref of="Enter the Angle (Deg)"() -> (w200:refnum<vi>)
      n121 = control-ref of="Enter the Frequency (Hz)"() -> (w199:refnum<vi>)
      n122 = control-ref of="Enter the Speed(mm/sec)"() -> (w182:refnum<vi>)
      n123 = control-ref of="Enter the Speed (RPM)"() -> (w181:refnum<vi>)
      n124 = control-ref of="Enter Scratch Speed (mm/s):"() -> (w180:refnum<vi>)
      n125 = control-ref of="Scartch Offset"() -> (w178:refnum<vi>)
      n126 = control-ref of="Enter Scratch length (mm):"() -> (w174:refnum<vi>)
      n127 = control-ref of="Wear Track Diameter"() -> (w173:refnum<vi>)
      n128 = control-ref of="No of Scratch"() -> (w171:refnum<vi>)
      n129 = control-ref of="String 39"() -> (w212:refnum<vi>)
      n130 = control-ref of="String 45"() -> (w184:refnum<vi>)
      n131 = control-ref of="Rotary Speed Exced"() -> (w172:refnum<vi>)
      n132 = control-ref of="StepTable For Load-Speed"() -> (w217:refnum<vi>)
      n133 = control-ref of="StepTable For Speed"() -> (w216:refnum<vi>)
      n134 = control-ref of="StepTable For Speed 3"() -> (w183:refnum<vi>)
      n135 = control-ref of="Motion Direction:  3"() -> (w236:refnum<vi>)
      n136 = control-ref of="Motion Mode:"() -> (w198:refnum<vi>)
      n137 = control-ref of="Scratch Mode"() -> (w177:refnum<vi>)
      n138 = control-ref of="Motion type:"() -> (w176:refnum<vi>)
      n139 = control-ref of="File Path :  2"() -> (w185:refnum<vi>)
      n140 = Bundle By Name(cluster=w241, "Motion Module.zNL"=w239, "Motion Module.NL disp"=w238, "Motion Module.Rotary Tab"=w237, "Motion Module.Motion Direction:  3"=w236, "Motion Module.E.Velocity 2"=w235, "Motion Module.e.v/ssr 2"=w234, "Motion Module.Enter Fixed E.Velocity 2"=w233, "Motion Module.Enter Final SRR 2"=w232, "Motion Module.Enter initial SRR 2"=w231, "Motion Module.Enter Fixed SRR 2"=w230, "Motion Module.Enter the Final E.Velocity (m/s) 2"=w229, "Motion Module.Enter initial E.Velocity (m/s) 2"=w228, "Motion Module.Final Speed (RPM) 3"=w227, "Motion Module.Initial Speed (RPM) 2"=w226, "Motion Module.Enter the Final Velocity (m/s) 3"=w225, "Motion Module.Enter initial Velocity (m/s)  3"=w224, "Motion Module.Ramp Up 2"=w223, "Motion Module.TEST SELECTION"=w222, "Motion Module.SPEED SELECTION :"=w221, "Motion Module.Angular Oscillation Set"=w220, "Motion Module.Traction"=w219, "Motion Module.Step Speed"=w218, "Motion Module.StepTable For Load-Speed"=w217, "Motion Module.StepTable For Speed"=w216, "Motion Module.Surge Forward MM"=w215, "Motion Module.Surge Backward MM"=w214, "Motion Module.M3 Image"=w213, "Motion Module.String 39"=w212, "Motion Module.Sway Left MM"=w211, "Motion Module.Sway Right MM"=w210, "Motion Module.Disable Axis Jog Soft Limits"=w209, "Motion Module.mm"=w208, "Motion Module.Heave Down MM"=w207, "Motion Module.Heave Up MM"=w206, "Motion Module.Wear Track Diameter (mm)"=w205, "Motion Module.Set WTD"=w204, "Motion Module.HomeScratch"=w203, "Motion Module.HomeRot"=w202, "Motion Module.PlaceModule"=w201, "Motion Module.Enter the Angle (Deg)"=w200, "Motion Module.Enter the Frequency (Hz)"=w199, "Motion Module.Motion Mode:"=w198, "Motion Module.LR Sway"=w197, "Motion Module.Rot Hor"=w196, "Motion Module.Scratch"=w195, "Motion Module.LR Cam"=w194, "Motion Module.MMBack"=w193, "Motion Module.MMNext"=w192, "Motion Module.Rot Ver"=w191, "Motion Module.Rotary Module Selection"=w190, "Motion Module.calculate rotary"=w189, "Motion Module.SPEED SELECTION : rotary"=w188, "Motion Module.Import 2"=w187, "Motion Module.Save 2"=w186, "Motion Module.File Path :  2"=w185, "Motion Module.String 45"=w184, "Motion Module.StepTable For Speed 3"=w183, "Motion Module.Enter the Speed(mm/sec)"=w182, "Motion Module.Enter the Speed(RPM)"=w181, "Motion Module.Enter Scratch Speed (mm/s):"=w180, "Motion Module.SwaySpeed Set"=w179, "Motion Module.Scartch Offset"=w178, "Motion Module.Scratch Mode"=w177, "Motion Module.Motion type:"=w176, "Motion Module.HomeScratch 2"=w175, "Motion Module.Enter Scratch length (mm):"=w174, "Motion Module.Wear Track Diameter"=w173, "Motion Module.Rotary Speed Exced"=w172, "Motion Module.No of Scratch"=w171) -> (w240:T21)
    }
    frame #6 {
      # "ENVIRONMENTAL CONTROL"
      n141 = control-ref of="Add to list"() -> (w259:refnum<vi>)
      n142 = control-ref of="Wear"() -> (w258:refnum<vi>)
      n143 = control-ref of="Vibration"() -> (w257:refnum<vi>)
      n144 = control-ref of="Humidity (Chamber)"() -> (w256:refnum<vi>)
      n145 = control-ref of="Temperature (Chamber)"() -> (w255:refnum<vi>)
      n146 = control-ref of="ECR"() -> (w254:refnum<vi>)
      n147 = control-ref of="Temperature (Amb)"() -> (w253:refnum<vi>)
      n148 = control-ref of="Microphone"() -> (w252:refnum<vi>)
      n149 = control-ref of="Acoustic Emission 3"() -> (w251:refnum<vi>)
      n150 = control-ref of="SNext"() -> (w250:refnum<vi>)
      n151 = control-ref of="APBack"() -> (w249:refnum<vi>)
      n152 = control-ref of="Low Temp"() -> (w245:refnum<vi>)
      n153 = control-ref of="High Temp"() -> (w244:refnum<vi>)
      n154 = control-ref of="Humidity"() -> (w243:refnum<vi>)
      n155 = control-ref of="Humidity  Status  3"() -> (w266:refnum<vi>)
      n156 = control-ref of="Low Temp  Status  2"() -> (w265:refnum<vi>)
      n157 = control-ref of="TK4 status 2"() -> (w264:refnum<vi>)
      n158 = control-ref of="Humidity (Amb)"() -> (w261:refnum<vi>)
      n159 = control-ref of="Clear List"() -> (w260:refnum<vi>)
      n160 = control-ref of="Enter the Temperature (°C):"() -> (w248:refnum<vi>)
      n161 = control-ref of="Enter the Stage \nTemperature (°C):"() -> (w247:refnum<vi>)
      n162 = control-ref of="Enter the Humidity (%Rh):"() -> (w246:refnum<vi>)
      n163 = control-ref of="Sensors Picked"() -> (w242:refnum<vi>)
      n164 = control-ref of="Stage Temperature"() -> (w263:refnum<vi>)
      n165 = control-ref of="Sample Temperature"() -> (w262:refnum<vi>)
      n166 = Bundle By Name(cluster=w268, "Environmental control.Humidity  Status  3"=w266, "Environmental control.Low Temp  Status  2"=w265, "Environmental control.TK4 status 2"=w264, "Environmental control.Stage Temperature"=w263, "Environmental control.Sample Temperature"=w262, "Environmental control.Humidity (Amb)"=w261, "Environmental control.Clear List"=w260, "Environmental control.Add to list"=w259, "Environmental control.Wear"=w258, "Environmental control.Vibration"=w257, "Environmental control.Humidity (Chamber)"=w256, "Environmental control.Temperature (Chamber)"=w255, "Environmental control.ECR"=w254, "Environmental control.Temperature (Amb)"=w253, "Environmental control.Microphone"=w252, "Environmental control.Acoustic Emission 3"=w251, "Environmental control.SNext"=w250, "Environmental control.APBack"=w249, "Environmental control.Enter the Temperature (°C):"=w248, "Environmental control.Enter the Stage \nTemperature (°C):"=w247, "Environmental control.Enter the Humidity (%Rh):"=w246, "Environmental control.Low Temp"=w245, "Environmental control.High Temp"=w244, "Environmental control.Humidity"=w243, "Environmental control.Sensors Picked"=w242) -> (w267:T21)
    }
    frame #7 {
      # "ABOUT SCREEN"
      n167 = control-ref of="ECR Port:"() -> (w273:refnum<vi>)
      n168 = control-ref of="Temperature"() -> (w272:refnum<vi>)
      n169 = control-ref of="Humidity Port:"() -> (w271:refnum<vi>)
      n170 = control-ref of="Home Service"() -> (w275:refnum<vi>)
      n171 = control-ref of="Advanced Setting"() -> (w274:refnum<vi>)
      n172 = control-ref of="Edit Gain Constants"() -> (w270:refnum<vi>)
      n173 = control-ref of="Save Gain Constants"() -> (w269:refnum<vi>)
      n174 = control-ref of="Password"() -> (w276:refnum<vi>)
      n175 = Bundle By Name(cluster=w278, "About Screen.Password"=w276, "About Screen.Home Service"=w275, "About Screen.Advanced Setting"=w274, "About Screen.ECR Port:"=w273, "About Screen.Temp Modbus:"=w272, "About Screen.Humidity Port:"=w271, "About Screen.Edit Gain Constants"=w270, "About Screen.Save Gain Constants"=w269) -> (w277:T21)
    }
    frame #8 {
      # "TEST SCREEN"
      n176 = control-ref of="Coefficient of Friction"() -> (w283:refnum<vi>)
      n177 = control-ref of="Acoustic Emission"() -> (w282:refnum<vi>)
      n178 = control-ref of="Friction Force (N)"() -> (w281:refnum<vi>)
      n179 = control-ref of="Depth (Microns)"() -> (w280:refnum<vi>)
      n180 = control-ref of="Normal Load ( N )"() -> (w279:refnum<vi>)
      n181 = control-ref of="Main Screen Tab"() -> (w364:refnum<vi>)
      n182 = control-ref of="Angle and Frequency"() -> (w363:refnum<vi>)
      n183 = control-ref of="Main Speed Tab"() -> (w360:refnum<vi>)
      n184 = control-ref of="MTM MOTOR DISPLAY"() -> (w359:refnum<vi>)
      n185 = control-ref of="SPEED TAB"() -> (w354:refnum<vi>)
      n186 = control-ref of="Time Tab"() -> (w349:refnum<vi>)
      n187 = control-ref of="Temp Tabs"() -> (w342:refnum<vi>)
      n188 = control-ref of="FF Tab"() -> (w293:refnum<vi>)
      n189 = control-ref of="Test Trip"() -> (w286:refnum<vi>)
      n190 = control-ref of="Heater"() -> (w341:refnum<vi>)
      n191 = control-ref of="TK4 status"() -> (w340:refnum<vi>)
      n192 = control-ref of="Controller  Status"() -> (w337:refnum<vi>)
      n193 = control-ref of="Cooling"() -> (w334:refnum<vi>)
      n194 = control-ref of="Load Communication"() -> (w333:refnum<vi>)
      n195 = control-ref of="HumCOMStatus"() -> (w331:refnum<vi>)
      n196 = control-ref of="Load En"() -> (w328:refnum<vi>)
      n197 = control-ref of="zNL 2"() -> (w327:refnum<vi>)
      n198 = control-ref of="Humidity On"() -> (w326:refnum<vi>)
      n199 = control-ref of="ClrLog"() -> (w322:refnum<vi>)
      n200 = control-ref of="STOP"() -> (w320:refnum<vi>)
      n201 = control-ref of="Start Test"() -> (w319:refnum<vi>)
      n202 = control-ref of="Test status"() -> (w318:refnum<vi>)
      n203 = control-ref of="AR Led"() -> (w317:refnum<vi>)
      n204 = control-ref of="Data"() -> (w316:refnum<vi>)
      n205 = control-ref of="Health"() -> (w315:refnum<vi>)
      n206 = control-ref of="Sway COM Status"() -> (w314:refnum<vi>)
      n207 = control-ref of="Heave COM Status"() -> (w313:refnum<vi>)
      n208 = control-ref of="Hymidity"() -> (w311:refnum<vi>)
      n209 = control-ref of="Humidity Disable trip"() -> (w310:refnum<vi>)
      n210 = control-ref of="Depthz"() -> (w307:refnum<vi>)
      n211 = control-ref of="Load Disable Trip"() -> (w304:refnum<vi>)
      n212 = control-ref of="BACK"() -> (w303:refnum<vi>)
      n213 = control-ref of="Depth Trip 2"() -> (w302:refnum<vi>)
      n214 = control-ref of="FF Disable Trip"() -> (w299:refnum<vi>)
      n215 = control-ref of="COF Disable Trip"() -> (w297:refnum<vi>)
      n216 = control-ref of="Start Test Temp"() -> (w296:refnum<vi>)
      n217 = control-ref of="zFF"() -> (w295:refnum<vi>)
      n218 = control-ref of="Scratch Start Test"() -> (w294:refnum<vi>)
      n219 = control-ref of="CZ FF"() -> (w291:refnum<vi>)
      n220 = control-ref of="Cyclic FF Disable Trip"() -> (w289:refnum<vi>)
      n221 = control-ref of="cyclic COF Disable Trip"() -> (w288:refnum<vi>)
      n222 = control-ref of="Scratch Start Recording"() -> (w284:refnum<vi>)
      n223 = control-ref of="Stroke (mm)"() -> (w362:refnum<vi>)
      n224 = control-ref of="Angle (Deg)"() -> (w361:refnum<vi>)
      n225 = control-ref of="Disc Speed (m/sec)"() -> (w358:refnum<vi>)
      n226 = control-ref of="Ball Speed (m/sec)"() -> (w357:refnum<vi>)
      n227 = control-ref of="Disc Speed (RPM)"() -> (w356:refnum<vi>)
      n228 = control-ref of="Ball Speed (RPM)"() -> (w355:refnum<vi>)
      n229 = control-ref of="Speed (m/sec)"() -> (w353:refnum<vi>)
      n230 = control-ref of="Set Speed (m/sec)"() -> (w352:refnum<vi>)
      n231 = control-ref of="Speed (RPM)"() -> (w351:refnum<vi>)
      n232 = control-ref of="Set Speed"() -> (w350:refnum<vi>)
      n233 = control-ref of="Time ( HH:MM:SS ) 2"() -> (w348:refnum<vi>)
      n234 = control-ref of="Test Duration"() -> (w347:refnum<vi>)
      n235 = control-ref of="Test Duration 4"() -> (w346:refnum<vi>)
      n236 = control-ref of="TEST CYCLE"() -> (w345:refnum<vi>)
      n237 = control-ref of="TOTAL CYCLES"() -> (w344:refnum<vi>)
      n238 = control-ref of="Set Load (N)"() -> (w343:refnum<vi>)
      n239 = control-ref of="ChamberTemp"() -> (w339:refnum<vi>)
      n240 = control-ref of="SetTmp"() -> (w338:refnum<vi>)
      n241 = control-ref of="ChamberTemp"() -> (w336:refnum<vi>)
      n242 = control-ref of="SetTmp"() -> (w335:refnum<vi>)
      n243 = control-ref of="Ambient \nTemperature"() -> (w332:refnum<vi>)
      n244 = control-ref of="Ambient\n Humidity"() -> (w330:refnum<vi>)
      n245 = control-ref of="Freq (Hz)"() -> (w329:refnum<vi>)
      n246 = control-ref of="humidity disp"() -> (w325:refnum<vi>)
      n247 = control-ref of="Set Humidity"() -> (w324:refnum<vi>)
      n248 = control-ref of="NL disp 2"() -> (w323:refnum<vi>)
      n249 = control-ref of="Acoustic Emission (mV)"() -> (w312:refnum<vi>)
      n250 = control-ref of="CoF Trip  2"() -> (w309:refnum<vi>)
      n251 = control-ref of="Depth Trip"() -> (w308:refnum<vi>)
      n252 = control-ref of="Depth (µm)"() -> (w306:refnum<vi>)
      n253 = control-ref of="NL Trip 2"() -> (w305:refnum<vi>)
      n254 = control-ref of="COF TRIP"() -> (w301:refnum<vi>)
      n255 = control-ref of="Friction Force (N)"() -> (w300:refnum<vi>)
      n256 = control-ref of="FF TRIP"() -> (w298:refnum<vi>)
      n257 = control-ref of="Cyclic Friction Force (N)"() -> (w292:refnum<vi>)
      n258 = control-ref of="Cyclic FF TRIP"() -> (w290:refnum<vi>)
      n259 = control-ref of="cyclic COF TRIP"() -> (w287:refnum<vi>)
      n260 = control-ref of="Multi Scratch Pass"() -> (w285:refnum<vi>)
      n261 = control-ref of="Trip Log"() -> (w321:refnum<vi>)
      n262 = Bundle By Name(cluster=w366, "Main Screen.Test Trip"=w286, "Main Screen.Main Screen Tab"=w364, "Main Screen.Angle and Frequency"=w363, "Main Screen.Stroke (mm)"=w362, "Main Screen.Angle (Deg)"=w361, "Main Screen.Main Speed Tab"=w360, "Main Screen.MTM MOTOR DISPLAY"=w359, "Main Screen.Disc Speed (m/sec)"=w358, "Main Screen.Ball Speed (m/sec)"=w357, "Main Screen.Disc Speed (RPM)"=w356, "Main Screen.Ball Speed (RPM)"=w355, "Main Screen.SPEED TAB"=w354, "Main Screen.Speed (m/sec)"=w353, "Main Screen.Set Speed (m/sec)"=w352, "Main Screen.Speed (RPM)"=w351, "Main Screen.Set Speed"=w350, "Main Screen.Time Tab"=w349, "Main Screen.Time ( HH:MM:SS ) 2"=w348, "Main Screen.Test Duration"=w347, "Main Screen.Test Duration 4"=w346, "Main Screen.TEST CYCLE"=w345, "Main Screen.TOTAL CYCLES"=w344, "Main Screen.Set Load (N)"=w343, "Main Screen.Temp Tabs"=w342, "Main Screen.Heater"=w341, "Main Screen.TK4 status"=w340, "Main Screen.ChamberTemp"=w339, "Main Screen.SetTmp"=w338, "Main Screen.Controller  Status"=w337, "Main Screen.ChamberTemp 2"=w336, "Main Screen.SetTmp 2"=w335, "Main Screen.Cooling"=w334, "Main Screen.Load Communication"=w333, "Main Screen.Ambient \nTemperature"=w332, "Main Screen.HumCOMStatus"=w331, "Main Screen.Ambient\n Humidity"=w330, "Main Screen.Freq (Hz)"=w329, "Main Screen.Load En"=w328, "Main Screen.zNL 2"=w327, "Main Screen.Humidity On"=w326, "Main Screen.humidity disp"=w325, "Main Screen.Set Humidity"=w324, "Main Screen.NL disp 2"=w323, "Main Screen.ClrLog"=w322, "Main Screen.Trip Log"=w321, "Main Screen.STOP"=w320, "Main Screen.Start Test"=w319, "Main Screen.Test status"=w318, "Main Screen.AR Led"=w317, "Main Screen.Data"=w316, "Main Screen.Health"=w315, "Main Screen.Sway COM Status"=w314, "Main Screen.Heave COM Status"=w313, "Main Screen.Acoustic Emission (mV)"=w312, "Main Screen.Hymidity"=w311, "Main Screen.Humidity Disable trip"=w310, "Main Screen.CoF Trip  2"=w309, "Main Screen.Depth Trip"=w308, "Main Screen.Depthz"=w307, "Main Screen.Depth (µm)"=w306, "Main Screen.NL Trip 2"=w305, "Main Screen.Load Disable Trip"=w304, "Main Screen.BACK"=w303, "Main Screen.Depth Trip 2"=w302, "Main Screen.COF TRIP"=w301, "Main Screen.Friction Force (N)"=w300, "Main Screen.FF Disable Trip"=w299, "Main Screen.FF TRIP"=w298, "Main Screen.COF Disable Trip"=w297, "Main Screen.FF Tab"=w293, "Main Screen.Start Test Temp"=w296, "Main Screen.zFF"=w295, "Main Screen.Scratch Start Test"=w294, "Main Screen.Cyclic Friction Force (N)"=w292, "Main Screen.CZ FF"=w291, "Main Screen.Cyclic FF TRIP"=w290, "Main Screen.Cyclic FF Disable Trip"=w289, "Main Screen.cyclic COF Disable Trip"=w288, "Main Screen.cyclic COF TRIP"=w287, "Main Screen.Multi Scratch Pass"=w285, "Main Screen.Scratch Start Recording"=w284, "Main Screen.Coefficient of Friction 2"=w283, "Main Screen.Acoustic Emission"=w282, "Main Screen.Friction Force (N) 2"=w281, "Main Screen.Depth (Microns)"=w280, "Main Screen.Normal Load ( N )"=w279) -> (w365:T21)
    }
    frame #9 {
      # "PID"
      n263 = control-ref of="gFF Rot 7"() -> (w367:refnum<vi>)
      n264 = control-ref of="Ramp"() -> (w372:refnum<vi>)
      n265 = control-ref of="apply load"() -> (w370:refnum<vi>)
      n266 = control-ref of="Bypass Load"() -> (w368:refnum<vi>)
      n267 = control-ref of="Vertical load (N)"() -> (w371:refnum<vi>)
      n268 = control-ref of="Enter ByPass Load"() -> (w369:refnum<vi>)
      n269 = Bundle By Name(cluster=w374, "PID.Ramp"=w372, "PID.Vertical load (N)"=w371, "PID.apply load"=w370, "PID.Enter ByPass Load"=w369, "PID.Bypass Load"=w368, "PID.gFF Rot"=w367) -> (w373:T21)
    }
    frame #10 {
      # "CONFIG PARAMETERS"
      n270 = control-ref of="DEPTH TRIP   ENABLE"() -> (w395:refnum<vi>)
      n271 = control-ref of="LOAD TRIP  ENABLE"() -> (w394:refnum<vi>)
      n272 = control-ref of="CYCLIC COF TRIP  ENABLE"() -> (w389:refnum<vi>)
      n273 = control-ref of="CYCLIC FF TRIP  ENABLE"() -> (w388:refnum<vi>)
      n274 = control-ref of="FF TRIP  ENABLE"() -> (w387:refnum<vi>)
      n275 = control-ref of="COF TRIP  ENABLE"() -> (w386:refnum<vi>)
      n276 = control-ref of="Rotary Vertical"() -> (w384:refnum<vi>)
      n277 = control-ref of="Traction 2"() -> (w383:refnum<vi>)
      n278 = control-ref of="Scratch 2"() -> (w382:refnum<vi>)
      n279 = control-ref of="LRM CAM"() -> (w381:refnum<vi>)
      n280 = control-ref of="Sway LRM"() -> (w380:refnum<vi>)
      n281 = control-ref of="Rotary Horizontal"() -> (w379:refnum<vi>)
      n282 = control-ref of="Start Button"() -> (w375:refnum<vi>)
      n283 = control-ref of="Re-initilaize"() -> (w441:refnum<vi>)
      n284 = control-ref of="Filter ON/OFF"() -> (w440:refnum<vi>)
      n285 = control-ref of="Apply Filter (FF)"() -> (w436:refnum<vi>)
      n286 = control-ref of="Apply Filter (Load)"() -> (w434:refnum<vi>)
      n287 = control-ref of="SAVE  2"() -> (w429:refnum<vi>)
      n288 = control-ref of="Enter Distance"() -> (w428:refnum<vi>)
      n289 = control-ref of="Heave Loop Delay"() -> (w404:refnum<vi>)
      n290 = control-ref of="Heave PID Speed"() -> (w403:refnum<vi>)
      n291 = control-ref of="Surge Jog Speed"() -> (w402:refnum<vi>)
      n292 = control-ref of="Heave Jog Speed"() -> (w401:refnum<vi>)
      n293 = control-ref of="Sway Loop Delay"() -> (w400:refnum<vi>)
      n294 = control-ref of="Sway PID Speed"() -> (w399:refnum<vi>)
      n295 = control-ref of="Sway Jog Speed"() -> (w398:refnum<vi>)
      n296 = control-ref of="DEPTH TRIP VALUE"() -> (w397:refnum<vi>)
      n297 = control-ref of="LOAD TRIP VALUE"() -> (w396:refnum<vi>)
      n298 = control-ref of="CYCLIC FF TRIP VALUE"() -> (w393:refnum<vi>)
      n299 = control-ref of="FF TRIP VALUE"() -> (w392:refnum<vi>)
      n300 = control-ref of="CYCLIC CoF TRIP VALUE"() -> (w391:refnum<vi>)
      n301 = control-ref of="COF TRIP VALUE"() -> (w390:refnum<vi>)
      n302 = control-ref of="JOG TRIP LOAD VALUE (N)"() -> (w385:refnum<vi>)
      n303 = control-ref of="SURGE SPEED"() -> (w378:refnum<vi>)
      n304 = control-ref of="SURGE BACKWARD COUNT"() -> (w377:refnum<vi>)
      n305 = control-ref of="SURGE FORWARD COUNT"() -> (w376:refnum<vi>)
      n306 = control-ref of="SAMPLES"() -> (w442:refnum<vi>)
      n307 = control-ref of="TracHomeSurgeOffsetCounts 10MM"() -> (w439:refnum<vi>)
      n308 = control-ref of="TracHomeSwayOffsetCounts 10MM"() -> (w438:refnum<vi>)
      n309 = control-ref of="Acoustic Emission:"() -> (w437:refnum<vi>)
      n310 = control-ref of="Filter% 2"() -> (w435:refnum<vi>)
      n311 = control-ref of="Filter%"() -> (w433:refnum<vi>)
      n312 = control-ref of="Sway distance (mm)"() -> (w432:refnum<vi>)
      n313 = control-ref of="Surge distance (mm)"() -> (w431:refnum<vi>)
      n314 = control-ref of="DataSavingLoopDelay(ms)"() -> (w430:refnum<vi>)
      n315 = control-ref of="Sway Counts:"() -> (w427:refnum<vi>)
      n316 = control-ref of="Distance (mm): 3"() -> (w426:refnum<vi>)
      n317 = control-ref of="Surge Counts:"() -> (w425:refnum<vi>)
      n318 = control-ref of="Distance (mm): 2"() -> (w424:refnum<vi>)
      n319 = control-ref of="Distance (mm):"() -> (w423:refnum<vi>)
      n320 = control-ref of="Heave Counts:"() -> (w422:refnum<vi>)
      n321 = control-ref of="LRMHomeSurgeOffsetCounts"() -> (w421:refnum<vi>)
      n322 = control-ref of="LRMHomeSwayOffsetCounts"() -> (w420:refnum<vi>)
      n323 = control-ref of="TracHomeSurgeOffsetCounts 20MM"() -> (w419:refnum<vi>)
      n324 = control-ref of="TracHomeSwayOffsetCounts 20MM"() -> (w418:refnum<vi>)
      n325 = control-ref of="RotHomeSwayOffsetCounts"() -> (w417:refnum<vi>)
      n326 = control-ref of="RotHomeSurgeOffsetCounts"() -> (w416:refnum<vi>)
      n327 = control-ref of="Heave distance"() -> (w415:refnum<vi>)
      n328 = control-ref of="Zmm"() -> (w414:refnum<vi>)
      n329 = control-ref of="Heave Pulses/mm"() -> (w413:refnum<vi>)
      n330 = control-ref of="Surge Pulses/mm"() -> (w412:refnum<vi>)
      n331 = control-ref of="Sway Pulses/mm"() -> (w411:refnum<vi>)
      n332 = control-ref of="Heave Pitch"() -> (w410:refnum<vi>)
      n333 = control-ref of="Surge Pitch"() -> (w409:refnum<vi>)
      n334 = control-ref of="Sway Pitch"() -> (w408:refnum<vi>)
      n335 = control-ref of="Heave PPR"() -> (w407:refnum<vi>)
      n336 = control-ref of="Surge PPR"() -> (w406:refnum<vi>)
      n337 = control-ref of="Sway PPR"() -> (w405:refnum<vi>)
      n338 = Bundle By Name(cluster=w444, "Config Parameters.SAMPLES"=w442, "Config Parameters.Re-initilaize"=w441, "Config Parameters.Filter ON/OFF"=w440, "Config Parameters.TracHomeSurgeOffsetCounts 10MM"=w439, "Config Parameters.TracHomeSwayOffsetCounts 10MM"=w438, "Config Parameters.Acoustic Emission:"=w437, "Config Parameters.Apply Filter (FF)"=w436, "Config Parameters.Filter% 2"=w435, "Config Parameters.Apply Filter (Load)"=w434, "Config Parameters.Filter%"=w433, "Config Parameters.Sway distance (mm)"=w432, "Config Parameters.Surge distance (mm)"=w431, "Config Parameters.DataSavingLoopDelay(ms)"=w430, "Config Parameters.SAVE 2"=w429, "Config Parameters.Enter Distance"=w428, "Config Parameters.Sway Counts:"=w427, "Config Parameters.Distance (mm): 3"=w426, "Config Parameters.Surge Counts:"=w425, "Config Parameters.Distance (mm): 2"=w424, "Config Parameters.Distance (mm):"=w423, "Config Parameters.Heave Counts:"=w422, "Config Parameters.LRMHomeSurgeOffsetCounts"=w421, "Config Parameters.LRMHomeSwayOffsetCounts"=w420, "Config Parameters.TracHomeSurgeOffsetCounts 20MM"=w419, "Config Parameters.TracHomeSwayOffsetCounts 20MM"=w418, "Config Parameters.RotHomeSwayOffsetCounts"=w417, "Config Parameters.RotHomeSurgeOffsetCounts"=w416, "Config Parameters.Heave distance"=w415, "Config Parameters.Zmm"=w414, "Config Parameters.Heave Pulses/mm"=w413, "Config Parameters.Surge Pulses/mm"=w412, "Config Parameters.Sway Pulses/mm"=w411, "Config Parameters.Heave Pitch"=w410, "Config Parameters.Surge Pitch"=w409, "Config Parameters.Sway Pitch"=w408, "Config Parameters.Heave PPR"=w407, "Config Parameters.Surge PPR"=w406, "Config Parameters.Sway PPR"=w405, "Config Parameters.Heave Loop Delay"=w404, "Config Parameters.Heave PID Speed"=w403, "Config Parameters.Surge Jog Speed"=w402, "Config Parameters.Heave Jog Speed"=w401, "Config Parameters.Sway Loop Delay"=w400, "Config Parameters.Sway PID Speed"=w399, "Config Parameters.Sway Jog Speed"=w398, "Config Parameters.DEPTH TRIP VALUE"=w397, "Config Parameters.LOAD TRIP VALUE"=w396, "Config Parameters.DEPTH TRIP   ENABLE"=w395, "Config Parameters.LOAD TRIP  ENABLE"=w394, "Config Parameters.CYCLIC FF TRIP VALUE"=w393, "Config Parameters.FF TRIP VALUE"=w392, "Config Parameters.CYCLIC CoF TRIP VALUE"=w391, "Config Parameters.COF TRIP VALUE"=w390, "Config Parameters.CYCLIC COF TRIP  ENABLE"=w389, "Config Parameters.CYCLIC FF TRIP  ENABLE"=w388, "Config Parameters.FF TRIP  ENABLE"=w387, "Config Parameters.COF TRIP  ENABLE"=w386, "Config Parameters.JOG TRIP LOAD VALUE (N)"=w385, "Config Parameters.Rotary Vertical"=w384, "Config Parameters.Traction"=w383, "Config Parameters.Scratch"=w382, "Config Parameters.LRM CAM"=w381, "Config Parameters.Sway LRM"=w380, "Config Parameters.Rotary Horizontal"=w379, "Config Parameters.SURGE SPEED"=w378, "Config Parameters.SURGE BACKWARD COUNT"=w377, "Config Parameters.SURGE FORWARD COUNT"=w376, "Config Parameters.Start Button"=w375) -> (w443:T21)
    }
    frame #11 {
      # "LOADING COM PORT"
      n339 = control-ref of="FORCE (N)"() -> (w447:refnum<vi>)
      n340 = control-ref of="TORQUE (N-m)"() -> (w446:refnum<vi>)
      n341 = control-ref of="ClearAll"() -> (w459:refnum<vi>)
      n342 = control-ref of="ZeroAll"() -> (w457:refnum<vi>)
      n343 = control-ref of="running_flag"() -> (w449:refnum<vi>)
      n344 = control-ref of="Load Cell Temp"() -> (w448:refnum<vi>)
      n345 = control-ref of="Save Dwell"() -> (w458:refnum<vi>)
      n346 = control-ref of="Acq Delay (ms)"() -> (w456:refnum<vi>)
      n347 = control-ref of="Burst Delay (ms)"() -> (w455:refnum<vi>)
      n348 = control-ref of="SN"() -> (w453:refnum<vi>)
      n349 = control-ref of="Port"() -> (w451:refnum<vi>)
      n350 = control-ref of="Load Cell Link"() -> (w445:refnum<vi>)
      n351 = control-ref of="model"() -> (w454:refnum<vi>)
      n352 = control-ref of="Sensor IP"() -> (w452:refnum<vi>)
      n353 = control-ref of="ft_data"() -> (w450:refnum<vi>)
      n354 = Bundle By Name(cluster=w461, "Loading Com Port.ClearAll"=w459, "Loading Com Port.Save Dwell"=w458, "Loading Com Port.ZeroAll"=w457, "Loading Com Port.Acq Delay (ms)"=w456, "Loading Com Port.Burst Delay (ms)"=w455, "Loading Com Port.model"=w454, "Loading Com Port.SN"=w453, "Loading Com Port.Sensor IP"=w452, "Loading Com Port.Port"=w451, "Loading Com Port.ft_data"=w450, "Loading Com Port.running_flag"=w449, "Loading Com Port.Load Cell Temp"=w448, "Loading Com Port.FORCE (N)"=w447, "Loading Com Port.TORQUE (N-m)"=w446, "Loading Com Port.Load Cell Link"=w445) -> (w460:T21)
    }
    frame #12 {
      # "HEAVE AND SURGE"
      n355 = control-ref of="Read Heave Temp"() -> (w507:refnum<vi>)
      n356 = control-ref of="Manual Write Heave & Surge"() -> (w484:refnum<vi>)
      n357 = control-ref of="error out Read"() -> (w519:refnum<vi>)
      n358 = control-ref of="error out Write"() -> (w514:refnum<vi>)
      n359 = control-ref of="UPLINK HEAVE"() -> (w463:refnum<vi>)
      n360 = control-ref of="DOWNLINK HEAVE"() -> (w462:refnum<vi>)
      n361 = control-ref of="SURGE POSE"() -> (w520:refnum<vi>)
      n362 = control-ref of="HEAVE POSE"() -> (w518:refnum<vi>)
      n363 = control-ref of="State"() -> (w517:refnum<vi>)
      n364 = control-ref of="Homed"() -> (w516:refnum<vi>)
      n365 = control-ref of="Sequence ID"() -> (w515:refnum<vi>)
      n366 = control-ref of="faultCode"() -> (w513:refnum<vi>)
      n367 = control-ref of="Ack ID"() -> (w512:refnum<vi>)
      n368 = control-ref of="SPEED"() -> (w511:refnum<vi>)
      n369 = control-ref of="Distance"() -> (w510:refnum<vi>)
      n370 = control-ref of="Mode Command"() -> (w509:refnum<vi>)
      n371 = control-ref of="SPARE 2"() -> (w506:refnum<vi>)
      n372 = control-ref of="SPARE 1"() -> (w505:refnum<vi>)
      n373 = control-ref of="Spare 15"() -> (w504:refnum<vi>)
      n374 = control-ref of="Spare 14"() -> (w503:refnum<vi>)
      n375 = control-ref of="Spare 13"() -> (w502:refnum<vi>)
      n376 = control-ref of="Spare 12"() -> (w501:refnum<vi>)
      n377 = control-ref of="Spare 11"() -> (w500:refnum<vi>)
      n378 = control-ref of="Spare 10"() -> (w499:refnum<vi>)
      n379 = control-ref of="Spare 9"() -> (w498:refnum<vi>)
      n380 = control-ref of="Spare 8"() -> (w497:refnum<vi>)
      n381 = control-ref of="Spare 5"() -> (w496:refnum<vi>)
      n382 = control-ref of="Spare 4"() -> (w495:refnum<vi>)
      n383 = control-ref of="Spare 3"() -> (w494:refnum<vi>)
      n384 = control-ref of="Spare 2"() -> (w493:refnum<vi>)
      n385 = control-ref of="Spare 1"() -> (w492:refnum<vi>)
      n386 = control-ref of="Humidity"() -> (w491:refnum<vi>)
      n387 = control-ref of="Temp"() -> (w490:refnum<vi>)
      n388 = control-ref of="Node Id"() -> (w489:refnum<vi>)
      n389 = control-ref of="SPARE 3"() -> (w488:refnum<vi>)
      n390 = control-ref of="SPARE 4"() -> (w487:refnum<vi>)
      n391 = control-ref of="fwMajor"() -> (w486:refnum<vi>)
      n392 = control-ref of="fwMinor"() -> (w485:refnum<vi>)
      n393 = control-ref of="SPARE 5"() -> (w482:refnum<vi>)
      n394 = control-ref of="Reserved"() -> (w481:refnum<vi>)
      n395 = control-ref of="SPARE 8"() -> (w480:refnum<vi>)
      n396 = control-ref of="SPARE 6"() -> (w479:refnum<vi>)
      n397 = control-ref of="SPARE 7"() -> (w478:refnum<vi>)
      n398 = control-ref of="SPARE 17"() -> (w477:refnum<vi>)
      n399 = control-ref of="SPARE 16"() -> (w476:refnum<vi>)
      n400 = control-ref of="SPARE 15"() -> (w475:refnum<vi>)
      n401 = control-ref of="SPARE 14"() -> (w474:refnum<vi>)
      n402 = control-ref of="SPARE 13"() -> (w473:refnum<vi>)
      n403 = control-ref of="SPARE 12"() -> (w472:refnum<vi>)
      n404 = control-ref of="SPARE 11"() -> (w471:refnum<vi>)
      n405 = control-ref of="SPARE 10"() -> (w470:refnum<vi>)
      n406 = control-ref of="SPARE 9"() -> (w469:refnum<vi>)
      n407 = control-ref of="System UPTIME"() -> (w468:refnum<vi>)
      n408 = control-ref of="Missed Packets"() -> (w467:refnum<vi>)
      n409 = control-ref of="faultCode Surge Right"() -> (w466:refnum<vi>)
      n410 = control-ref of="faultCode Surge Left"() -> (w465:refnum<vi>)
      n411 = control-ref of="faultCode Heave"() -> (w464:refnum<vi>)
      n412 = control-ref of="Heave and Surge Read"() -> (w508:refnum<vi>)
      n413 = control-ref of="Heave and Surge Write"() -> (w483:refnum<vi>)
      n414 = Bundle By Name(cluster=w522, "Heave AND Surge.SURGE POSE"=w520, "Heave AND Surge.error out Read"=w519, "Heave AND Surge.HEAVE POSE"=w518, "Heave AND Surge.State"=w517, "Heave AND Surge.Homed"=w516, "Heave AND Surge.Sequence ID"=w515, "Heave AND Surge.error out Write"=w514, "Heave AND Surge.faultCode"=w513, "Heave AND Surge.Ack ID"=w512, "Heave AND Surge.SPEED"=w511, "Heave AND Surge.Distance"=w510, "Heave AND Surge.Mode Command"=w509, "Heave AND Surge.Heave and Surge Read"=w508, "Heave AND Surge.Read Heave Temp"=w507, "Heave AND Surge.SPARE 2"=w506, "Heave AND Surge.SPARE 1"=w505, "Heave AND Surge.Spare 15"=w504, "Heave AND Surge.Spare 14"=w503, "Heave AND Surge.Spare 13"=w502, "Heave AND Surge.Spare 12"=w501, "Heave AND Surge.Spare 11"=w500, "Heave AND Surge.Spare 10"=w499, "Heave AND Surge.Spare 9"=w498, "Heave AND Surge.Spare 8"=w497, "Heave AND Surge.Spare 7"=w496, "Heave AND Surge.Spare 4"=w495, "Heave AND Surge.Spare 3"=w494, "Heave AND Surge.Spare 4"=w493, "Heave AND Surge.Spare 3"=w492, "Heave AND Surge.Spare 2"=w491, "Heave AND Surge.Spare 1"=w490, "Heave AND Surge.Node Id"=w489, "Heave AND Surge.SPARE 3"=w488, "Heave AND Surge.SPARE 4"=w487, "Heave AND Surge.fwMajor"=w486, "Heave AND Surge.fwMinor"=w485, "Heave AND Surge.Manual Write"=w484, "Heave AND Surge.Heave and Surge Write"=w483, "Heave AND Surge.SPARE 5"=w482, "Heave AND Surge.Reserved"=w481, "Heave AND Surge.SPARE 8"=w480, "Heave AND Surge.SPARE 6"=w479, "Heave AND Surge.SPARE 7"=w478, "Heave AND Surge.SPARE 17"=w477, "Heave AND Surge.SPARE 16"=w476, "Heave AND Surge.SPARE 15"=w475, "Heave AND Surge.SPARE 14"=w474, "Heave AND Surge.SPARE 13"=w473, "Heave AND Surge.SPARE 12"=w472, "Heave AND Surge.SPARE 11"=w471, "Heave AND Surge.SPARE 10"=w470, "Heave AND Surge.SPARE 9"=w469, "Heave AND Surge.System UPTIME"=w468, "Heave AND Surge.Missed Packets"=w467, "Heave AND Surge.faultCode Surge Right"=w466, "Heave AND Surge.faultCode Surge Left"=w465, "Heave AND Surge.faultCode Heave"=w464, "Heave AND Surge.UPLINK HEAVE"=w463, "Heave AND Surge.DOWNLINK HEAVE"=w462) -> (w521:T21)
    }
    frame #13 {
      # "NEW PID LOGIC"
      n415 = control-ref of="PID"() -> (w523:refnum<vi>)
      n416 = control-ref of="Fine Tune Zone"() -> (w543:refnum<vi>)
      n417 = control-ref of="PID Delay (sec)"() -> (w542:refnum<vi>)
      n418 = control-ref of="Max_pos_limit"() -> (w541:refnum<vi>)
      n419 = control-ref of="Min_pos_limit"() -> (w540:refnum<vi>)
      n420 = control-ref of="i_limit"() -> (w539:refnum<vi>)
      n421 = control-ref of="pct_scale"() -> (w530:refnum<vi>)
      n422 = control-ref of="Deadband"() -> (w538:refnum<vi>)
      n423 = control-ref of="Kd"() -> (w537:refnum<vi>)
      n424 = control-ref of="Ki"() -> (w536:refnum<vi>)
      n425 = control-ref of="Kp"() -> (w535:refnum<vi>)
      n426 = control-ref of="Current Position"() -> (w534:refnum<vi>)
      n427 = control-ref of="Set Load"() -> (w533:refnum<vi>)
      n428 = control-ref of="Current Load"() -> (w532:refnum<vi>)
      n429 = control-ref of="Pulse delta"() -> (w531:refnum<vi>)
      n430 = control-ref of="Init Step"() -> (w529:refnum<vi>)
      n431 = control-ref of="Max Step Linit"() -> (w528:refnum<vi>)
      n432 = control-ref of="min_deadband_floor"() -> (w527:refnum<vi>)
      n433 = control-ref of="dynamic_spindle_noise_scalar"() -> (w526:refnum<vi>)
      n434 = control-ref of="min_finetune_floor"() -> (w525:refnum<vi>)
      n435 = control-ref of="filter_alpha"() -> (w524:refnum<vi>)
      n436 = Bundle By Name(cluster=w545, "New PID LOGIC.Fine Tune Zone"=w543, "New PID LOGIC.PID SDelay"=w542, "New PID LOGIC.Max_pos_limit"=w541, "New PID LOGIC.Min_pos_limit"=w540, "New PID LOGIC.i_limit"=w539, "New PID LOGIC.pct_scale"=w530, "New PID LOGIC.Deadband"=w538, "New PID LOGIC.Kd"=w537, "New PID LOGIC.Ki"=w536, "New PID LOGIC.Kp"=w535, "New PID LOGIC.Current Position"=w534, "New PID LOGIC.Set Load"=w533, "New PID LOGIC.Current Load"=w532, "New PID LOGIC.Pulse delta"=w531, "New PID LOGIC.Init Step"=w529, "New PID LOGIC.Max Step Linit"=w528, "New PID LOGIC.min_deadband_floor"=w527, "New PID LOGIC.dynamic_spindle_noise_scalar"=w526, "New PID LOGIC.min_finetune_floor"=w525, "New PID LOGIC.filter_alpha"=w524, "New PID LOGIC.PID"=w523) -> (w544:T21)
    }
    frame #14 {
      # "SWAY"
      n437 = control-ref of="Manual Write SWAY"() -> (w584:refnum<vi>)
      n438 = control-ref of="Read SWAY Temp"() -> (w565:refnum<vi>)
      n439 = control-ref of="error out Write  SWAY"() -> (w586:refnum<vi>)
      n440 = control-ref of="error out Read SWAY"() -> (w585:refnum<vi>)
      n441 = control-ref of="faultCode Rotary"() -> (w548:refnum<vi>)
      n442 = control-ref of="UPLINK SWAY"() -> (w547:refnum<vi>)
      n443 = control-ref of="DOWNLINK SWAY"() -> (w546:refnum<vi>)
      n444 = control-ref of="fwMajor"() -> (w603:refnum<vi>)
      n445 = control-ref of="Homed"() -> (w602:refnum<vi>)
      n446 = control-ref of="Rotary POSE"() -> (w601:refnum<vi>)
      n447 = control-ref of="State"() -> (w600:refnum<vi>)
      n448 = control-ref of="SWAY POSE"() -> (w599:refnum<vi>)
      n449 = control-ref of="Ack ID"() -> (w598:refnum<vi>)
      n450 = control-ref of="faultCode"() -> (w597:refnum<vi>)
      n451 = control-ref of="Node Id"() -> (w596:refnum<vi>)
      n452 = control-ref of="fwMinor"() -> (w595:refnum<vi>)
      n453 = control-ref of="Spare 6"() -> (w594:refnum<vi>)
      n454 = control-ref of="Spare 5"() -> (w593:refnum<vi>)
      n455 = control-ref of="Spare 4"() -> (w592:refnum<vi>)
      n456 = control-ref of="Spare 3"() -> (w591:refnum<vi>)
      n457 = control-ref of="Spare 2"() -> (w590:refnum<vi>)
      n458 = control-ref of="Spare 1"() -> (w589:refnum<vi>)
      n459 = control-ref of="Spare 7"() -> (w588:refnum<vi>)
      n460 = control-ref of="SPARE  5"() -> (w587:refnum<vi>)
      n461 = control-ref of="SPARE  4"() -> (w582:refnum<vi>)
      n462 = control-ref of="SPARE  3"() -> (w581:refnum<vi>)
      n463 = control-ref of="SPARE 2"() -> (w580:refnum<vi>)
      n464 = control-ref of="SPARE1"() -> (w579:refnum<vi>)
      n465 = control-ref of="Spare 15"() -> (w578:refnum<vi>)
      n466 = control-ref of="Spare 14"() -> (w577:refnum<vi>)
      n467 = control-ref of="Spare 13"() -> (w576:refnum<vi>)
      n468 = control-ref of="Spare 12"() -> (w575:refnum<vi>)
      n469 = control-ref of="Spare 11"() -> (w574:refnum<vi>)
      n470 = control-ref of="Spare 9"() -> (w573:refnum<vi>)
      n471 = control-ref of="Spare 8"() -> (w572:refnum<vi>)
      n472 = control-ref of="SPEED"() -> (w571:refnum<vi>)
      n473 = control-ref of="Distance"() -> (w570:refnum<vi>)
      n474 = control-ref of="Mode Command"() -> (w569:refnum<vi>)
      n475 = control-ref of="Sequence ID"() -> (w568:refnum<vi>)
      n476 = control-ref of="Spare 10"() -> (w566:refnum<vi>)
      n477 = control-ref of="faultCode Sway"() -> (w564:refnum<vi>)
      n478 = control-ref of="Missed Packets"() -> (w563:refnum<vi>)
      n479 = control-ref of="System UPTIME"() -> (w562:refnum<vi>)
      n480 = control-ref of="SPARE 6"() -> (w561:refnum<vi>)
      n481 = control-ref of="SPARE 7"() -> (w560:refnum<vi>)
      n482 = control-ref of="SPARE 9"() -> (w559:refnum<vi>)
      n483 = control-ref of="SPARE 11"() -> (w558:refnum<vi>)
      n484 = control-ref of="SPARE 10"() -> (w557:refnum<vi>)
      n485 = control-ref of="SPARE 8"() -> (w556:refnum<vi>)
      n486 = control-ref of="SPARE 13"() -> (w555:refnum<vi>)
      n487 = control-ref of="SPARE 12"() -> (w554:refnum<vi>)
      n488 = control-ref of="SPARE 17"() -> (w553:refnum<vi>)
      n489 = control-ref of="SPARE 16"() -> (w552:refnum<vi>)
      n490 = control-ref of="SPARE 15"() -> (w551:refnum<vi>)
      n491 = control-ref of="SPARE 14"() -> (w550:refnum<vi>)
      n492 = control-ref of="Reserved"() -> (w549:refnum<vi>)
      n493 = control-ref of="SWAY WRITE"() -> (w583:refnum<vi>)
      n494 = control-ref of="SWAY READ"() -> (w567:refnum<vi>)
      n495 = Bundle By Name(cluster=w605, "SWAY.fwMajor"=w603, "SWAY.Homed"=w602, "SWAY.Rotary POSE"=w601, "SWAY.State"=w600, "SWAY.SWAY POSE"=w599, "SWAY.Ack ID"=w598, "SWAY.faultCode"=w597, "SWAY.Node Id"=w596, "SWAY.fwMinor"=w595, "SWAY.Spare 6"=w594, "SWAY.Spare 5"=w593, "SWAY.Spare 4"=w592, "SWAY.Spare 3"=w591, "SWAY.Spare 2"=w590, "SWAY.Spare 1"=w589, "SWAY.Spare 7"=w588, "SWAY.SPARE  5"=w587, "SWAY.error out Write  SWAY"=w586, "SWAY.error out Read SWAY"=w585, "SWAY.Manual Write SWAY"=w584, "SWAY.SWAY WRITE"=w583, "SWAY.SPARE  4"=w582, "SWAY.SPARE  3"=w581, "SWAY.SPARE 2"=w580, "SWAY.SPARE 1"=w579, "SWAY.Spare 15"=w578, "SWAY.Spare 14"=w577, "SWAY.Spare 13"=w576, "SWAY.Spare 12"=w575, "SWAY.Spare 11"=w574, "SWAY.Spare 9"=w573, "SWAY.Spare 8"=w572, "SWAY.SPEED"=w571, "SWAY.Distance"=w570, "SWAY.Mode Command"=w569, "SWAY.Sequence ID"=w568, "SWAY.SWAY READ"=w567, "SWAY.Spare 10"=w566, "SWAY.Read SWAY Temp"=w565, "SWAY.faultCode Sway"=w564, "SWAY.Missed Packets"=w563, "SWAY.System UPTIME sway"=w562, "SWAY.SPARE 6"=w561, "SWAY.SPARE 7"=w560, "SWAY.SPARE 9"=w559, "SWAY.SPARE 11"=w558, "SWAY.SPARE 10"=w557, "SWAY.SPARE 8"=w556, "SWAY.SPARE 13"=w555, "SWAY.SPARE 12"=w554, "SWAY.SPARE 17"=w553, "SWAY.SPARE 16"=w552, "SWAY.SPARE 15"=w551, "SWAY.SPARE 14"=w550, "SWAY.Reserved"=w549, "SWAY.faultCode Rotary"=w548, "SWAY.UPLINK SWAY"=w547, "SWAY.DOWNLINK SWAY"=w546) -> (w604:T21)
    }
    frame #15 {
      # "ANALYSIS SCREEN GRAPH PLOT"
      n496 = control-ref of="Analysis Home new"() -> (w636:refnum<vi>)
      n497 = control-ref of="Refresh 2"() -> (w635:refnum<vi>)
      n498 = control-ref of="OPEN 4"() -> (w621:refnum<vi>)
      n499 = control-ref of="OPEN 3"() -> (w619:refnum<vi>)
      n500 = control-ref of="XY Graph"() -> (w614:refnum<vi>)
      n501 = control-ref of="OPEN 2"() -> (w611:refnum<vi>)
      n502 = control-ref of="OPEN 1"() -> (w610:refnum<vi>)
      n503 = control-ref of="Export"() -> (w607:refnum<vi>)
      n504 = control-ref of="MEAN"() -> (w634:refnum<vi>)
      n505 = control-ref of="SD"() -> (w633:refnum<vi>)
      n506 = control-ref of="VARIANCE"() -> (w632:refnum<vi>)
      n507 = control-ref of="MEAN"() -> (w631:refnum<vi>)
      n508 = control-ref of="SD"() -> (w630:refnum<vi>)
      n509 = control-ref of="VARIANCE"() -> (w629:refnum<vi>)
      n510 = control-ref of="MEAN"() -> (w628:refnum<vi>)
      n511 = control-ref of="SD"() -> (w627:refnum<vi>)
      n512 = control-ref of="VARIANCE"() -> (w626:refnum<vi>)
      n513 = control-ref of="MEAN"() -> (w625:refnum<vi>)
      n514 = control-ref of="SD"() -> (w624:refnum<vi>)
      n515 = control-ref of="VARIANCE"() -> (w623:refnum<vi>)
      n516 = control-ref of="File 4 Discription"() -> (w622:refnum<vi>)
      n517 = control-ref of="File Name 4"() -> (w620:refnum<vi>)
      n518 = control-ref of="File 3 Discription"() -> (w618:refnum<vi>)
      n519 = control-ref of="File Name 3"() -> (w617:refnum<vi>)
      n520 = control-ref of="File Name 2"() -> (w613:refnum<vi>)
      n521 = control-ref of="File Name 1"() -> (w612:refnum<vi>)
      n522 = control-ref of="File 1 Discription"() -> (w609:refnum<vi>)
      n523 = control-ref of="File 2 Discription"() -> (w608:refnum<vi>)
      n524 = control-ref of="Y-AXIS"() -> (w616:refnum<vi>)
      n525 = control-ref of="X-AXIS"() -> (w615:refnum<vi>)
      n526 = control-ref of="File Format"() -> (w606:refnum<vi>)
      n527 = Bundle By Name(cluster=w638, "Analysis Screen.Analysis Home"=w636, "Analysis Screen.Refresh 2"=w635, "Analysis Screen.MEAN 4"=w634, "Analysis Screen.SD 4"=w633, "Analysis Screen.VARIANCE 4"=w632, "Analysis Screen.MEAN  3"=w631, "Analysis Screen.SD  3"=w630, "Analysis Screen.VARIANCE  3"=w629, "Analysis Screen.MEAN 2"=w628, "Analysis Screen.SD  2"=w627, "Analysis Screen.VARIANCE 2"=w626, "Analysis Screen.MEAN"=w625, "Analysis Screen.SD"=w624, "Analysis Screen.VARIANCE"=w623, "Analysis Screen.File 4 Discription"=w622, "Analysis Screen.OPEN 4"=w621, "Analysis Screen.File Name 4"=w620, "Analysis Screen.OPEN 3"=w619, "Analysis Screen.File 3 Discription"=w618, "Analysis Screen.File Name 3"=w617, "Analysis Screen.Y-AXIS"=w616, "Analysis Screen.X-AXIS"=w615, "Analysis Screen.XY Graph"=w614, "Analysis Screen.File Name 2"=w613, "Analysis Screen.File Name 1"=w612, "Analysis Screen.OPEN 2"=w611, "Analysis Screen.OPEN 1"=w610, "Analysis Screen.File 1 Discription"=w609, "Analysis Screen.File 2 Discription"=w608, "Analysis Screen.Export"=w607, "Analysis Screen.File Format"=w606) -> (w637:T21)
    }
    frame #16 {
      # "TRACTION"
      n528 = control-ref of="Manual Write TRACTION"() -> (w670:refnum<vi>)
      n529 = control-ref of="Read TRACTION Temp"() -> (w657:refnum<vi>)
      n530 = control-ref of="error out Read TRACTION"() -> (w644:refnum<vi>)
      n531 = control-ref of="error out Write  TRACTION"() -> (w643:refnum<vi>)
      n532 = control-ref of="Downlink traction"() -> (w640:refnum<vi>)
      n533 = control-ref of="Uplink Traction"() -> (w639:refnum<vi>)
      n534 = control-ref of="Spare 3"() -> (w641:refnum<vi>)
      n535 = control-ref of="faultCode Traction 2"() -> (w688:refnum<vi>)
      n536 = control-ref of="faultCode Traction 1"() -> (w687:refnum<vi>)
      n537 = control-ref of="Missed Packets"() -> (w686:refnum<vi>)
      n538 = control-ref of="System UPTIME"() -> (w685:refnum<vi>)
      n539 = control-ref of="SPARE 17"() -> (w684:refnum<vi>)
      n540 = control-ref of="SPARE 16"() -> (w683:refnum<vi>)
      n541 = control-ref of="SPARE 15"() -> (w682:refnum<vi>)
      n542 = control-ref of="SPARE 14"() -> (w681:refnum<vi>)
      n543 = control-ref of="SPARE 13"() -> (w680:refnum<vi>)
      n544 = control-ref of="SPARE 12"() -> (w679:refnum<vi>)
      n545 = control-ref of="SPARE 11"() -> (w678:refnum<vi>)
      n546 = control-ref of="SPARE 10"() -> (w677:refnum<vi>)
      n547 = control-ref of="SPARE 9"() -> (w676:refnum<vi>)
      n548 = control-ref of="SPARE 8"() -> (w675:refnum<vi>)
      n549 = control-ref of="SPARE 7"() -> (w674:refnum<vi>)
      n550 = control-ref of="SPARE 6"() -> (w673:refnum<vi>)
      n551 = control-ref of="Reserved"() -> (w672:refnum<vi>)
      n552 = control-ref of="SPARE  5"() -> (w671:refnum<vi>)
      n553 = control-ref of="SPARE  4"() -> (w668:refnum<vi>)
      n554 = control-ref of="SPARE  3"() -> (w667:refnum<vi>)
      n555 = control-ref of="SPARE 2"() -> (w666:refnum<vi>)
      n556 = control-ref of="SPARE 1"() -> (w665:refnum<vi>)
      n557 = control-ref of="Spare 7"() -> (w664:refnum<vi>)
      n558 = control-ref of="Spare 6"() -> (w663:refnum<vi>)
      n559 = control-ref of="Spare 5"() -> (w662:refnum<vi>)
      n560 = control-ref of="Spare 4"() -> (w661:refnum<vi>)
      n561 = control-ref of="Spare 2"() -> (w660:refnum<vi>)
      n562 = control-ref of="Spare 1"() -> (w659:refnum<vi>)
      n563 = control-ref of="Node Id"() -> (w658:refnum<vi>)
      n564 = control-ref of="fwMinor"() -> (w656:refnum<vi>)
      n565 = control-ref of="fwMajor"() -> (w655:refnum<vi>)
      n566 = control-ref of="faultCode"() -> (w654:refnum<vi>)
      n567 = control-ref of="TRACTION POSE 2"() -> (w653:refnum<vi>)
      n568 = control-ref of="TRACTION POSE 1"() -> (w652:refnum<vi>)
      n569 = control-ref of="Homed"() -> (w651:refnum<vi>)
      n570 = control-ref of="State"() -> (w650:refnum<vi>)
      n571 = control-ref of="Ack ID"() -> (w649:refnum<vi>)
      n572 = control-ref of="SPEED"() -> (w648:refnum<vi>)
      n573 = control-ref of="Distance"() -> (w647:refnum<vi>)
      n574 = control-ref of="Mode Command"() -> (w646:refnum<vi>)
      n575 = control-ref of="Sequence ID"() -> (w645:refnum<vi>)
      n576 = control-ref of="TRACTION WRITE"() -> (w669:refnum<vi>)
      n577 = control-ref of="TRACTION READ"() -> (w642:refnum<vi>)
      n578 = Bundle By Name(cluster=w690, "Traction.faultCode Traction 2"=w688, "Traction.faultCode Traction 1"=w687, "Traction.Missed Packets"=w686, "Traction.System UPTIME Traction"=w685, "Traction.SPARE 17"=w684, "Traction.SPARE 16"=w683, "Traction.SPARE 15"=w682, "Traction.SPARE 14"=w681, "Traction.SPARE 13"=w680, "Traction.SPARE 12"=w679, "Traction.SPARE 11"=w678, "Traction.SPARE 10"=w677, "Traction.SPARE 9"=w676, "Traction.SPARE 8"=w675, "Traction.SPARE 7"=w674, "Traction.SPARE 6"=w673, "Traction.Reserved"=w672, "Traction.SPARE  5"=w671, "Traction.Manual Write TRACTION"=w670, "Traction.TRACTION WRITE"=w669, "Traction.SPARE  4"=w668, "Traction.SPARE  3"=w667, "Traction.SPARE 2"=w666, "Traction.SPARE 1"=w665, "Traction.Spare 7"=w664, "Traction.Spare 6"=w663, "Traction.Spare 5"=w662, "Traction.Spare 4"=w661, "Traction.Spare 2"=w660, "Traction.Spare 1"=w659, "Traction.Node Id"=w658, "Traction.Read TRACTION Temp"=w657, "Traction.fwMinor"=w656, "Traction.fwMajor"=w655, "Traction.faultCode"=w654, "Traction.TRACTION POSE"=w653, "Traction.TRACTION POSE 2"=w652, "Traction.Homed"=w651, "Traction.State"=w650, "Traction.Ack ID"=w649, "Traction.SPEED"=w648, "Traction.Distance"=w647, "Traction.Mode Command"=w646, "Traction.Sequence ID"=w645, "Traction.error out Read TRACTION"=w644, "Traction.error out Write  TRACTION"=w643, "Traction.TRACTION READ"=w642, "Traction.Spare 3"=w641, "Traction.Downlink traction"=w640, "Traction.Uplink Traction"=w639) -> (w689:T21)
    }
    frame #17 {
      # "TRACTIOJN RECEIPE"
      n579 = control-ref of="Traction Receipe"() -> (w713:refnum<vi>)
      n580 = control-ref of="Traction Receipe Update Details"() -> (w691:refnum<vi>)
      n581 = control-ref of="Total Execution Time"() -> (w724:refnum<vi>)
      n582 = control-ref of="Total Steps"() -> (w723:refnum<vi>)
      n583 = control-ref of="Duration / Step (s)"() -> (w722:refnum<vi>)
      n584 = control-ref of="Duration / Step (s)"() -> (w720:refnum<vi>)
      n585 = control-ref of="Speed (mm/s)"() -> (w718:refnum<vi>)
      n586 = control-ref of="SET entrainment Velocity"() -> (w712:refnum<vi>)
      n587 = control-ref of="Test Array Size"() -> (w711:refnum<vi>)
      n588 = control-ref of="SRR INDEX [ STRIBECK]"() -> (w710:refnum<vi>)
      n589 = control-ref of="Stribeck Size"() -> (w709:refnum<vi>)
      n590 = control-ref of="SET SRR"() -> (w708:refnum<vi>)
      n591 = control-ref of="ELAPSED TIMER"() -> (w707:refnum<vi>)
      n592 = control-ref of="BALL SET RPM"() -> (w706:refnum<vi>)
      n593 = control-ref of="DISC SET RPM"() -> (w705:refnum<vi>)
      n594 = control-ref of="SET LOAD"() -> (w704:refnum<vi>)
      n595 = control-ref of="TEMPERATURE READ"() -> (w703:refnum<vi>)
      n596 = control-ref of="SET TEMPERATURE"() -> (w702:refnum<vi>)
      n597 = control-ref of="Traction Size"() -> (w701:refnum<vi>)
      n598 = control-ref of="DISC SPEED (rpm)"() -> (w700:refnum<vi>)
      n599 = control-ref of="BALL SPEED (rpm)"() -> (w699:refnum<vi>)
      n600 = control-ref of="BALL WEAR TRACK"() -> (w698:refnum<vi>)
      n601 = control-ref of="DISC WEARTRACK"() -> (w697:refnum<vi>)
      n602 = control-ref of="SRR INDEX [ TRACTION]"() -> (w696:refnum<vi>)
      n603 = control-ref of="Start Index Type"() -> (w695:refnum<vi>)
      n604 = control-ref of="Ball (mm/sec)"() -> (w693:refnum<vi>)
      n605 = control-ref of="Disc (mm/sec)"() -> (w692:refnum<vi>)
      n606 = control-ref of="SRR Sweep Range (%)"() -> (w725:refnum<vi>)
      n607 = control-ref of="STRIBECK Fixed SRR List (%)"() -> (w721:refnum<vi>)
      n608 = control-ref of="SRR Sweep Range (%)"() -> (w719:refnum<vi>)
      n609 = control-ref of="Temperature Stages (°C)"() -> (w717:refnum<vi>)
      n610 = control-ref of="Load (N)"() -> (w716:refnum<vi>)
      n611 = control-ref of="Lubricant Name"() -> (w715:refnum<vi>)
      n612 = control-ref of="Profile File Name"() -> (w714:refnum<vi>)
      n613 = control-ref of="Enum - Menu"() -> (w694:refnum<vi>)
      n614 = Bundle By Name(cluster=w727, "Traction reciepe.SRR Sweep Range (%) Stribeck"=w725, "Traction reciepe.Traction Receipe"=w713, "Traction reciepe.Total Execution Time"=w724, "Traction reciepe.Total Steps"=w723, "Traction reciepe.Duration / Step (s)  Stribeck"=w722, "Traction reciepe.STRIBECK Fixed SRR List (%)"=w721, "Traction reciepe.Duration / Step (s) Traction"=w720, "Traction reciepe.SRR Sweep Range (%) traction"=w719, "Traction reciepe.Rolling Speed (mm/s)"=w718, "Traction reciepe.Temperature Stages (°C)"=w717, "Traction reciepe.Ball Load (N)"=w716, "Traction reciepe.Lubricant Name"=w715, "Traction reciepe.Profile File Name"=w714, "Traction reciepe.SET entrainment Velocity"=w712, "Traction reciepe.Test Array Size"=w711, "Traction reciepe.SRR INDEX [ STRIBECK]"=w710, "Traction reciepe.Stribeck Size"=w709, "Traction reciepe.SET SRR"=w708, "Traction reciepe.ELAPSED TIMER"=w707, "Traction reciepe.BALL SET RPM"=w706, "Traction reciepe.DISC SET RPM"=w705, "Traction reciepe.SET LOAD"=w704, "Traction reciepe.TEMPERATURE READ"=w703, "Traction reciepe.SET TEMPERATURE"=w702, "Traction reciepe.Traction Size"=w701, "Traction reciepe.DISC SPEED (rpm)"=w700, "Traction reciepe.BALL SPEED (rpm)"=w699, "Traction reciepe.BALL WEAR TRACK"=w698, "Traction reciepe.DISC WEARTRACK"=w697, "Traction reciepe.SRR INDEX [ TRACTION]"=w696, "Traction reciepe.Start Index Type"=w695, "Traction reciepe.Enum - Menu"=w694, "Traction reciepe.Ball (mm/sec)"=w693, "Traction reciepe.Disc (mm/sec)"=w692, "Traction reciepe.Traction Receipe Update Details"=w691) -> (w726:T21)
    }
    frame #18 {
      # "TRACTION CONTROL"
      n615 = control-ref of="SPEED SELECTION : MTM"() -> (w756:refnum<vi>)
      n616 = control-ref of="TEST SELECTION (MTM)"() -> (w755:refnum<vi>)
      n617 = control-ref of="MTM Test Selection"() -> (w754:refnum<vi>)
      n618 = control-ref of="TEST SELECTION (MTM) 2"() -> (w742:refnum<vi>)
      n619 = control-ref of="SPEED SELECTION : MTM 2"() -> (w741:refnum<vi>)
      n620 = control-ref of="MTM Test Selection 2"() -> (w740:refnum<vi>)
      n621 = control-ref of="Demo Mode Display"() -> (w784:refnum<vi>)
      n622 = control-ref of="Main Tab sequence for selection"() -> (w781:refnum<vi>)
      n623 = control-ref of="Ramp Tab"() -> (w780:refnum<vi>)
      n624 = control-ref of="e.v/ssr"() -> (w779:refnum<vi>)
      n625 = control-ref of="File Path Tab"() -> (w753:refnum<vi>)
      n626 = control-ref of="Step Sequence Indication Tab"() -> (w748:refnum<vi>)
      n627 = control-ref of="HomeTraction"() -> (w785:refnum<vi>)
      n628 = control-ref of="Traction Step Update Details"() -> (w782:refnum<vi>)
      n629 = control-ref of="E.Velocity"() -> (w771:refnum<vi>)
      n630 = control-ref of="Ramp Up   Disc"() -> (w768:refnum<vi>)
      n631 = control-ref of="Ramp Up"() -> (w761:refnum<vi>)
      n632 = control-ref of="BallSpeed Exceed Indication"() -> (w758:refnum<vi>)
      n633 = control-ref of="Apply"() -> (w757:refnum<vi>)
      n634 = control-ref of="Save"() -> (w751:refnum<vi>)
      n635 = control-ref of="Import"() -> (w750:refnum<vi>)
      n636 = control-ref of="Calculate Step"() -> (w746:refnum<vi>)
      n637 = control-ref of="Disc Speed Indicator"() -> (w729:refnum<vi>)
      n638 = control-ref of="Enter Fixed E.Velocity"() -> (w778:refnum<vi>)
      n639 = control-ref of="Enter Final SRR"() -> (w777:refnum<vi>)
      n640 = control-ref of="Enter initial SRR"() -> (w776:refnum<vi>)
      n641 = control-ref of="Enter Fixed SRR"() -> (w775:refnum<vi>)
      n642 = control-ref of="Enter the Final E.Velocity (m/s)"() -> (w774:refnum<vi>)
      n643 = control-ref of="Enter initial E.Velocity (m/s)"() -> (w773:refnum<vi>)
      n644 = control-ref of="Ball WTD"() -> (w772:refnum<vi>)
      n645 = control-ref of="Enter the Final Velocity (m/s)"() -> (w770:refnum<vi>)
      n646 = control-ref of="Enter initial Velocity (m/s)"() -> (w769:refnum<vi>)
      n647 = control-ref of="Initial DiscSpeed (RPM)"() -> (w767:refnum<vi>)
      n648 = control-ref of="Final Speed (RPM)"() -> (w766:refnum<vi>)
      n649 = control-ref of="Final Speed (RPM) Ball"() -> (w765:refnum<vi>)
      n650 = control-ref of="Initial Speed (RPM) Ball"() -> (w764:refnum<vi>)
      n651 = control-ref of="Enter the Final Velocity (m/s) Ball"() -> (w763:refnum<vi>)
      n652 = control-ref of="Enter initial Velocity (m/s) Ball"() -> (w762:refnum<vi>)
      n653 = control-ref of="Enter the Speed (m/sec):"() -> (w739:refnum<vi>)
      n654 = control-ref of="Enter the Speed (m/sec):"() -> (w738:refnum<vi>)
      n655 = control-ref of="Enter the Speed (RPM):"() -> (w737:refnum<vi>)
      n656 = control-ref of="Enter the Speed (RPM):Ball"() -> (w734:refnum<vi>)
      n657 = control-ref of="Wear Track Diameter (mm)"() -> (w730:refnum<vi>)
      n658 = control-ref of="Traction Message"() -> (w783:refnum<vi>)
      n659 = control-ref of="ExceedBallSpeed step"() -> (w760:refnum<vi>)
      n660 = control-ref of="ExceedDiscSpeed"() -> (w759:refnum<vi>)
      n661 = control-ref of="File Path String"() -> (w752:refnum<vi>)
      n662 = control-ref of="Step Sequence Indication"() -> (w747:refnum<vi>)
      n663 = control-ref of="ExceedDiscSpeed  Cinstant Speed"() -> (w744:refnum<vi>)
      n664 = control-ref of="ExceedBallSpeed Constant"() -> (w743:refnum<vi>)
      n665 = control-ref of="Lower Spped"() -> (w736:refnum<vi>)
      n666 = control-ref of="Upper"() -> (w735:refnum<vi>)
      n667 = control-ref of="ExceedBallSpeed"() -> (w728:refnum<vi>)
      n668 = control-ref of="StepTable"() -> (w745:refnum<vi>)
      n669 = control-ref of="Disc Motion Direction:"() -> (w733:refnum<vi>)
      n670 = control-ref of="Ball Motion Direction :"() -> (w732:refnum<vi>)
      n671 = control-ref of="Motion Mode:"() -> (w731:refnum<vi>)
      n672 = control-ref of="File Path :"() -> (w749:refnum<vi>)
      n673 = Bundle By Name(cluster=w787, "Traction Control.HomeTraction"=w785, "Traction Control.Demo Mode Display"=w784, "Traction Control.Traction Message"=w783, "Traction Control.Traction Step Update Details"=w782, "Traction Control.Main Tab sequence for selection"=w781, "Traction Control.Ramp Tab"=w780, "Traction Control.e.v/ssr"=w779, "Traction Control.Enter Fixed E.Velocity"=w778, "Traction Control.Enter Final SRR"=w777, "Traction Control.Enter initial SRR"=w776, "Traction Control.Enter Fixed SRR"=w775, "Traction Control.Enter the Final E.Velocity (m/s)"=w774, "Traction Control.Enter initial E.Velocity (m/s)"=w773, "Traction Control.Ball WTD"=w772, "Traction Control.E.Velocity"=w771, "Traction Control.Enter the Final Velocity (m/s)"=w770, "Traction Control.Enter initial Velocity (m/s)"=w769, "Traction Control.Ramp Up   Disc"=w768, "Traction Control.Initial DiscSpeed (RPM)"=w767, "Traction Control.Final Speed (RPM) Ball"=w766, "Traction Control.Final Speed (RPM)"=w765, "Traction Control.Initial Speed (RPM) Ball"=w764, "Traction Control.Enter the Final Velocity (m/s) Ball"=w763, "Traction Control.Enter initial Velocity (m/s) Ball"=w762, "Traction Control.Ramp Up"=w761, "Traction Control.ExceedBallSpeed step"=w760, "Traction Control.ExceedDiscSpeed"=w759, "Traction Control.BallSpeed Exceed Indication"=w758, "Traction Control.Apply"=w757, "Traction Control.SPEED SELECTION : MTM"=w756, "Traction Control.TEST SELECTION (MTM)"=w755, "Traction Control.MTM Test Selection"=w754, "Traction Control.File Path Tab"=w753, "Traction Control.File Path String"=w752, "Traction Control.Save"=w751, "Traction Control.Import"=w750, "Traction Control.File Path :"=w749, "Traction Control.Step Sequence Indication Tab"=w748, "Traction Control.Step Sequence Indication"=w747, "Traction Control.Calculate Step"=w746, "Traction Control.StepTable"=w745, "Traction Control.ExceedDiscSpeed  Cinstant Speed"=w744, "Traction Control.ExceedBallSpeed Constant"=w743, "Traction Control.TEST SELECTION (MTM) 2"=w742, "Traction Control.SPEED SELECTION : MTM 3"=w741, "Traction Control.MTM Test Selection 2"=w740, "Traction Control.Enter the Speed (m/sec):"=w739, "Traction Control.Enter the Speed (m/sec):  2"=w738, "Traction Control.Enter the Speed (RPM):"=w737, "Traction Control.Lower Spped"=w736, "Traction Control.Upper"=w735, "Traction Control.Enter the Speed (RPM):Ball"=w734, "Traction Control.Disc Motion Direction:"=w733, "Traction Control.Ball Motion Direction :"=w732, "Traction Control.Motion Mode:"=w731, "Traction Control.Wear Track Diameter (mm)"=w730, "Traction Control.Disc Speed Indicator"=w729, "Traction Control.ExceedBallSpeed"=w728) -> (w786:T21)
    }
    frame #19 {
      # "ACOUSTICS"
      n674 = control-ref of="Gains"() -> (w790:refnum<vi>)
      n675 = control-ref of="Acoustic Graphs"() -> (w788:refnum<vi>)
      n676 = control-ref of="Manual Write Acquostic"() -> (w789:refnum<vi>)
      n677 = control-ref of="error out 2"() -> (w795:refnum<vi>)
      n678 = control-ref of="error in (no error)"() -> (w794:refnum<vi>)
      n679 = control-ref of="Downlink Packet"() -> (w793:refnum<vi>)
      n680 = control-ref of="Uplink Packet"() -> (w792:refnum<vi>)
      n681 = control-ref of="Last Config Rejected"() -> (w800:refnum<vi>)
      n682 = control-ref of="rx command count"() -> (w799:refnum<vi>)
      n683 = control-ref of="Current Filter Id"() -> (w798:refnum<vi>)
      n684 = control-ref of="Isolated Gain"() -> (w797:refnum<vi>)
      n685 = control-ref of="DAQ Status"() -> (w796:refnum<vi>)
      n686 = control-ref of="data out"() -> (w791:refnum<vi>)
      n687 = Bundle By Name(cluster=w802, "Acquostic.Last Config Rejected"=w800, "Acquostic.rx command count"=w799, "Acquostic.Current Filter Id"=w798, "Acquostic.Isolated Gain"=w797, "Acquostic.DAQ Status"=w796, "Acquostic.error out"=w795, "Acquostic.error in (no error)"=w794, "Acquostic.Downlink Packet"=w793, "Acquostic.Uplink Packet"=w792, "Acquostic.data out"=w791, "Acquostic.Acoustic Graphs"=w788, "Acquostic.Gains"=w790, "Acquostic.Manual Write Acquostic"=w789) -> (w801:T21)
    }
    frame #20 {
      # "ABOUT SCREEN"
      n688 = control-ref of="Info"() -> (w803:refnum<vi>)
      n689 = control-ref of="version"() -> (w810:refnum<vi>)
      n690 = control-ref of="Operating System"() -> (w809:refnum<vi>)
      n691 = control-ref of="Version"() -> (w808:refnum<vi>)
      n692 = control-ref of="Workorder"() -> (w807:refnum<vi>)
      n693 = control-ref of="Runtime"() -> (w806:refnum<vi>)
      n694 = control-ref of="Instrument Serial"() -> (w805:refnum<vi>)
      n695 = control-ref of="Firmware Version"() -> (w804:refnum<vi>)
      n696 = Bundle By Name(cluster=w812, "ABOUT.version"=w810, "ABOUT.Operating System"=w809, "ABOUT.Version"=w808, "ABOUT.Workorder"=w807, "ABOUT.Runtime"=w806, "ABOUT.Instrument Serial"=w805, "ABOUT.Firmware Version"=w804, "ABOUT.Info"=w803) -> (w811:T21)
    }
    frame #21 {
      # "TEMPERATURE PORT"
      n697 = control-ref of="error out Temperature"() -> (w814:refnum<vi>)
      n698 = control-ref of="Temperature 2"() -> (w815:refnum<vi>)
      n699 = control-ref of="READ TEMPERATURE"() -> (w813:refnum<vi>)
      n700 = Bundle By Name(cluster=w817, "Temperature Port.Temperature"=w815, "Temperature Port.error out Temperature"=w814, "Temperature Port.READ TEMPERATURE"=w813) -> (w816:T21)
    }
  }
  n701 = call <userlib>:"Fit VI window to Largest Dec.vi"() -> ("error out"=w75:errorcluster, "dup VI Ref"=w72:refnum<vi>)  [unwired: 6 in]
  n702 = invoke on="Invoke Node" class="VI" method="FP.Run-Time Position.Maximized"(reference=w72, error in=w75) -> (error out=w74:errorcluster)  [unwired: 2 in, 3 out]
  n703 = call <vilib>:"Clear Errors.vi"("error in (no error)"=w74) -> ("error out"=w73:errorcluster)  [unwired: 5 in, 1 out]
  n704 = control-ref of="This VI"() -> (w78:refnum<vi>)
  n705 = invoke on="Invoke Node" class="VI" method="Default Vals.Reinit All"(reference=w78, error in=w73) -> (reference out=w76:refnum<vi>, error out=w77:errorcluster)  [unwired: 1 in, 1 out]
  n706 = Close Reference(reference=w76, error in (no error)=w77) -> (error out=w71:errorcluster)
  n707 = call "Create User Event - Stop.vi"("error in (no error)"=w71) -> ("error out"=w18:errorcluster, "User Event - Stop"=w48:refnum<user-event>)  [unwired: 9 in]
  n708 = call "Queue Out Unitest.vi"("error in"=w18, 11:REF_Enum_Unitest."Init") -> ("error out"=w43:errorcluster)  [unwired: 8 in, 1 out]
  n709 = call "Queue Out Unitest.vi"("error in"=w43, 11:REF_Enum_Unitest."UI Loop") -> ("error out"=w42:errorcluster, "Quee Out"=w16:refnum<queue>)  [unwired: 8 in]
  n710 = call "Queue Out Unitest.vi"("error in"=w42, 11:REF_Enum_Unitest."LOAD COM LOOP") -> ("error out"=w41:errorcluster, "Quee Out"=w15:refnum<queue>)  [unwired: 8 in]
  n711 = call "Queue Out Unitest.vi"("error in"=w41, 11:REF_Enum_Unitest."HEAVE MOTOR COM LOOP") -> ("error out"=w40:errorcluster, "Quee Out"=w14:refnum<queue>)  [unwired: 8 in]
  n712 = call "Queue Out Unitest.vi"("error in"=w40, 11:REF_Enum_Unitest."SWAY MOTOR COM LOOP") -> ("error out"=w39:errorcluster, "Quee Out"=w13:refnum<queue>)  [unwired: 8 in]
  n713 = call "Queue Out Unitest.vi"("error in"=w39, 11:REF_Enum_Unitest."RAMP MOTOR COM LOOP") -> ("error out"=w38:errorcluster, "Quee Out"=w12:refnum<queue>)  [unwired: 8 in]
  n714 = call "Queue Out Unitest.vi"("error in"=w38, 11:REF_Enum_Unitest."TEMPERATURE COM LOOP") -> ("error out"=w37:errorcluster, "Quee Out"=w11:refnum<queue>)  [unwired: 8 in]
  n715 = call "Queue Out Unitest.vi"("error in"=w37, 11:REF_Enum_Unitest."HUMIDITY COM PORT") -> ("error out"=w36:errorcluster, "Quee Out"=w10:refnum<queue>)  [unwired: 8 in]
  n716 = call "Queue Out Unitest.vi"("error in"=w36, 11:REF_Enum_Unitest."ECR PORT") -> ("error out"=w35:errorcluster, "Quee Out"=w9:refnum<queue>)  [unwired: 8 in]
  n717 = call "Queue Out Unitest.vi"("error in"=w35, 11:REF_Enum_Unitest."MONITOR LOOP") -> ("error out"=w34:errorcluster, "Quee Out"=w8:refnum<queue>)  [unwired: 8 in]
  n718 = call "Queue Out Unitest.vi"("error in"=w34, 11:REF_Enum_Unitest."PROGRAM LOOP") -> ("error out"=w33:errorcluster, "Quee Out"=w7:refnum<queue>)  [unwired: 8 in]
  n719 = call "Queue Out Unitest.vi"("error in"=w33, 11:REF_Enum_Unitest."LOAD PID") -> ("error out"=w32:errorcluster, "Quee Out"=w6:refnum<queue>)  [unwired: 8 in]
  n720 = call "Queue Out Unitest.vi"("error in"=w32, 11:REF_Enum_Unitest."REPORT") -> ("error out"=w20:errorcluster, "Quee Out"=w5:refnum<queue>)  [unwired: 8 in]
  n721 = call "Queue Out Unitest.vi"("error in"=w20, 11:REF_Enum_Unitest."ACOUSTIC") -> ("error out"=w17:errorcluster, "Quee Out"=w4:refnum<queue>)  [unwired: 8 in]
  n722 = register-events(w48) -> (reference out=w90:refnum<event-registration>, error out=w88:errorcluster)  [unwired: 2 in]
  n723 = Merge Errors(w88, w17) -> (w89:errorcluster)
  n724 = disable-structure shown="Enabled" {
    disable-tunnel: w12 -> [w822 _]
    disable-tunnel: [w821 w917] -> w58
    disable-tunnel: w48 -> [w820 _]
    disable-tunnel: w47 -> [w819 _]
    disable-tunnel: w18 -> [w818 w917]
    frame Enabled {
      n725 = while {
        shift-right: [w824] -> _
        shift-left: w819 -> [w843]
        tunnel: [w837] -> w821
        tunnel: w822 -> [w835]
        tunnel: w818 -> [w834]
        tunnel: w820 -> [w833]
        stop <- w842 stop-if-true
        # "Ramp Motor  Handling Loop"
        n726 = call "Dequeue Message.vi"("error in (no error)"=w834, "Message Queue"=w835) -> ("error out"=w841:errorcluster, "output data"=w839:dbl[][], "Message"=w840:string, "dup Message Queue"=w838:refnum<queue>)  [unwired: 6 in]
        n727 = case "Message Cases" shown="\"Ramp Main\"" w840 {
          selector: w840 -> [_ _ _ _ _ w907]
          tunnel: w838 -> [w855 w871 _ w894 w906 _]
          tunnel: w841 -> [w857 w869 w889 w898 w900 _]
          tunnel: [w858 w872 w890 w896 w902 w908] -> w836
          tunnel: w843 -> [w846 w860 w891 w897 w905 w909]
          tunnel: [w846 w860 w891 w897 w905 w909] -> w824
          tunnel: [_ _ _ _ TRUE _] -> w842
          tunnel: w839 -> [_ _ _ _ _ _]
          tunnel: w833 -> [_ _ _ _ w899 _]
          frame "init" {
            # "Initialize - All initialization work should take place in this message, since other loops can potentially enqueue messages that execute immediately after this one."
            n728 = call "TRACTION WRITE FGV.vi"("Enum - Menu"=Traction_Write_enum."INIT", "error in (no error)"=w857, "main ref"=w846) -> ("error out"=w854:errorcluster)  [unwired: 8 in]
            n729 = call <vilib>:"Clear Errors.vi"("error in (no error)"=w854) -> ("error out"=w852:errorcluster)  [unwired: 5 in, 1 out]
            n730 = call "Stall Data Flow.vim"("value in"=w852, "milliseconds to wait"=u32 1000) -> ("value out"=w851:errorcluster)  [unwired: 1 out]
            n731 = call "Traction  Init.vi"("error in (no error)"=w851, "main ref"=w846) -> ("error out"=w849:errorcluster)  [unwired: 9 in]
            n732 = call <vilib>:"Clear Errors.vi"("error in (no error)"=w849) -> ("error out"=w848:errorcluster)  [unwired: 5 in, 1 out]
            n733 = call "TRACTION READ FGV.vi"("Enum - Menu"=Traction_Read_enum."INIT", "error in (no error)"=w848, "main ref"=w846) -> ("error out"=w847:errorcluster)  [unwired: 7 in, 1 out]
            n734 = call <vilib>:"Clear Errors.vi"("error in (no error)"=w847) -> ("error out"=w845:errorcluster)  [unwired: 5 in, 1 out]
            n735 = call-poly "Enqueue Message.vi"("error in (no error)"=w845, "Message"="Ramp Main", "Message Queue"=w855) -> ("error out"=w858:errorcluster)  [unwired: 7 in, 1 out]
          }
          frame "Ramp Main" {
            n736 = Unbundle By Name(w860) -> ("Traction.Read TRACTION Temp"=w865:refnum<vi>)
            n737 = property on="Property Node" class="Bool (strict)"(reference=w865) -> (reference out=w863:refnum<vi>, error out=w864:errorcluster, "Value"=w861:bool)  [unwired: 1 in]
            n738 = Close Reference(reference=w863, error in (no error)=w864) -> ()  [unwired: 1 out]
            n739 = case shown="True" w861 {
              tunnel: w869 -> [w873 w880]
              tunnel: [w873 w877] -> w862
              tunnel: w860 -> [_ w878]
              tunnel: w860 -> [_ w876]
              frame False {
              }
              frame True {
                n740 = call "TRACTION READ FGV.vi"("Enum - Menu"=Traction_Read_enum."READ", "error in (no error)"=w880, "main ref"=w878) -> ("error out"=w879:errorcluster, "ERROR TEMP"=w875:bool)  [unwired: 7 in]
                n741 = call "Traction Reinitize.vi"("error in (no error)"=w879, "Checkbox"=w875, "Data Cluster"=w876) -> ("error out"=w877:errorcluster)  [unwired: 8 in]
              }
            }
            n742 = Unbundle By Name(w860) -> ("Main Home Screen.EXIT"=w870:refnum<vi>)
            n743 = call <vilib>:"Clear Errors.vi"("error in (no error)"=w862) -> ("error out"=w859:errorcluster)  [unwired: 5 in, 1 out]
            n744 = property on="Property Node" class="Bool (strict)"(reference=w870) -> (reference out=w867:refnum<vi>, error out=w868:errorcluster, "Value"=w866:bool)  [unwired: 1 in]
            n745 = case shown="False" w866 {
              tunnel: [w883 w887] -> w872
              tunnel: w871 -> [w882 w886]
              tunnel: w859 -> [w881 w885]
              frame True {
                n746 = call-poly "Enqueue Message.vi"("error in (no error)"=w881, "Message"="Confirm Quit", "Message Queue"=w882) -> ("error out"=w883:errorcluster)  [unwired: 7 in, 1 out]
              }
              frame False {
                n747 = call-poly "Enqueue Message.vi"("error in (no error)"=w885, "Message"="Ramp Main", "Message Queue"=w886) -> ("error out"=w887:errorcluster)  [unwired: 7 in, 1 out]
              }
            }
            n748 = Close Reference(reference=w867, error in (no error)=w868) -> ()  [unwired: 1 out]
          }
          frame "Error" {
            # "#CodeRecommended - If you ever change the name of this \"Error\" message, you'll need to update the name in the Check Loop Error.vi as well."
            # "#CodeRecommended - Consider creating a system for logging errors in some way. These errors are for notification purposes only. Handling of specific errors should be performed in the message frames that generated the error."
            # "Error - Display an error dialog. This message is sent by the \"Error Handler\" VIs at the end of other loops in this application."
            n749 = Merge Errors(w889) -> (w890:errorcluster)
          }
          frame "Confirm Quit" {
            # "#CodeNeeded - If you want to provide an \"Are you sure\" dialog (or some other notification) before the application exits, place that code here. This message is typically sent from a Panel Close? event."
            # "Confirm Quit - Message that can confirm whether or not the user wants to exit the application."
            n750 = call-poly "Enqueue Message.vi"("Priority Message? (F)"=TRUE, "error in (no error)"=w898, "Message"="Exit", "Message Queue"=w894) -> ("error out"=w895:errorcluster)  [unwired: 6 in, 1 out]
            n751 = Merge Errors(w895) -> (w896:errorcluster)
          }
          frame "Exit" {
            # "Stop the VI"
            # "Release the message queue reference"
            # "#CodeNeeded - Add any required cleanup code here. Note that if 'Exit' was called as a result of an error, an error dialog will be displayed. Add any custom error handling for an 'Exit' condition here as well."
            # "Exit - Exit the application."
            n752 = call "Fire User Event - Stop.vi"("User Event - Stop"=w899) -> ("error out"=w901:errorcluster)  [unwired: 10 in]
            n753 = Release Queue(queue=w906, error in (no error)=w900) -> (error out=w903:errorcluster)  [unwired: 1 in, 2 out]
            n754 = Merge Errors(w901, w903) -> (w902:errorcluster)
          }
          frame Default {
            # "'Default' case only runs if there is a message that isn't defined in any of the other cases.  Output a programming error."
            n755 = xnode ("Error Ring")("parameter 0"=w907) -> ("error out"=w908:errorcluster)
          }
        }
        n756 = call "LAB-IQ Error Handler - Message Handling Loop.vi"("error in (no error)"=w836, "Message Queue"=w838) -> ("dup error in"=w837:errorcluster)  [unwired: 8 in, 1 out]
        n757 = Unbundle By Name(w824) -> ("Motion Module.Traction"=w832:refnum<vi>)
        n758 = property on="Property Node" class="Bool (strict)"(reference=w832) -> (reference out=w830:refnum<vi>, error out=w831:errorcluster, "Value"=w829:bool)  [unwired: 1 in]
        n759 = Close Reference(reference=w830, error in (no error)=w831) -> ()  [unwired: 1 out]
        n760 = Equal?(x=w829, y=TRUE) -> (x = y?=w827:bool)
        n761 = Select(t=i64 5 ("Period"), s=w827, f=i64 1000) -> (s? t:f=w823:i64)
        n762 = Wait (ms)(milliseconds to wait=w823) -> ()  [unwired: 1 out]
      }
    }
    frame Disabled {
      # "E"
      # "ENABLE WHEN RUNNING IN TRACTION TEST CONDITION"
    }
  }
  n763 = disable-structure "Diagram Disable Structure" shown="Enabled" {
    disable-tunnel: w10 -> [w922 _]
    disable-tunnel: w47 -> [w921 _]
    disable-tunnel: w48 -> [w920 _]
    disable-tunnel: w18 -> [w919 w988]
    disable-tunnel: [w918 w988] -> w53
    frame Disabled {
      n764 = while {
        shift-right: [w933] -> _
        shift-left: w921 -> [w934]
        tunnel: [w927] -> w918
        tunnel: w922 -> [w925]
        tunnel: w919 -> [w924]
        tunnel: w920 -> [w923]
        stop <- w932 stop-if-true
        # "Humidity  Handling Loop"
        n765 = call "Dequeue Message.vi"("error in (no error)"=w924, "Message Queue"=w925) -> ("error out"=w931:errorcluster, "output data"=w929:dbl[][], "Message"=w930:string, "dup Message Queue"=w928:refnum<queue>)  [unwired: 6 in]
        n766 = case "Message Cases" shown="\"Humidity Main\"" w930 {
          selector: w930 -> [_ _ _ _ _ w978]
          tunnel: w928 -> [w935 w946 _ w965 w977 _]
          tunnel: w931 -> [w938 w943 w962 w969 w971 _]
          tunnel: [w939 w947 w956 w967 w973 w979] -> w926
          tunnel: w934 -> [w937 w945 w961 w968 w976 w980]
          tunnel: [w937 w945 w961 w968 w976 w980] -> w933
          tunnel: [_ _ _ _ TRUE _] -> w932
          tunnel: w929 -> [_ _ w960 _ _ _]
          tunnel: w923 -> [_ _ _ _ w970 _]
          frame "init" {
            # "Initialize - All initialization work should take place in this message, since other loops can potentially enqueue messages that execute immediately after this one."
            n767 = call-poly "Enqueue Message.vi"("error in (no error)"=w938, "Message"="Humidity Main", "Message Queue"=w935) -> ("error out"=w939:errorcluster)  [unwired: 7 in, 1 out]
          }
          frame "Humidity Main" {
            n768 = Unbundle By Name(w945) -> ("Main Home Screen.EXIT"=w944:refnum<vi>)
            n769 = property on="Property Node" class="Bool (strict)"(reference=w944) -> (reference out=w941:refnum<vi>, error out=w942:errorcluster, "Value"=w940:bool)  [unwired: 1 in]
            n770 = case shown="False" w940 {
              tunnel: [w950 w954] -> w947
              tunnel: w946 -> [w949 w953]
              tunnel: w943 -> [w948 w952]
              frame True {
                n771 = call-poly "Enqueue Message.vi"("error in (no error)"=w948, "Message"="Confirm Quit", "Message Queue"=w949) -> ("error out"=w950:errorcluster)  [unwired: 7 in, 1 out]
              }
              frame False {
                n772 = call-poly "Enqueue Message.vi"("error in (no error)"=w952, "Message"="Humidity Main", "Message Queue"=w953) -> ("error out"=w954:errorcluster)  [unwired: 7 in, 1 out]
              }
            }
            n773 = Close Reference(reference=w941, error in (no error)=w942) -> ()  [unwired: 1 out]
          }
          frame "Error" {
            # "#CodeRecommended - If you ever change the name of this \"Error\" message, you'll need to update the name in the Check Loop Error.vi as well."
            # "#CodeRecommended - Consider creating a system for logging errors in some way. These errors are for notification purposes only. Handling of specific errors should be performed in the message frames that generated the error."
            # "Error - Display an error dialog. This message is sent by the \"Error Handler\" VIs at the end of other loops in this application."
            n774 = Variant To Data(error in=w962, type=errorcluster {"status"=FALSE, "code"=0, "source"=""} ("error constant"), Variant=w960) -> (data=w958:errorcluster, error out=w957:errorcluster)
            n775 = call <vilib>:"Simple Error Handler.vi"("error in (no error)"=w958) -> ()  [unwired: 4 in, 5 out]
            n776 = Merge Errors(w957) -> (w956:errorcluster)
          }
          frame "Confirm Quit" {
            # "#CodeNeeded - If you want to provide an \"Are you sure\" dialog (or some other notification) before the application exits, place that code here. This message is typically sent from a Panel Close? event."
            # "Confirm Quit - Message that can confirm whether or not the user wants to exit the application."
            n777 = call-poly "Enqueue Message.vi"("Priority Message? (F)"=TRUE, "error in (no error)"=w969, "Message"="Exit", "Message Queue"=w965) -> ("error out"=w966:errorcluster)  [unwired: 6 in, 1 out]
            n778 = Merge Errors(w966) -> (w967:errorcluster)
          }
          frame "Exit" {
            # "Stop the VI"
            # "Release the message queue reference"
            # "#CodeNeeded - Add any required cleanup code here. Note that if 'Exit' was called as a result of an error, an error dialog will be displayed. Add any custom error handling for an 'Exit' condition here as well."
            # "Exit - Exit the application."
            n779 = call "Fire User Event - Stop.vi"("User Event - Stop"=w970) -> ("error out"=w972:errorcluster)  [unwired: 10 in]
            n780 = Release Queue(queue=w977, error in (no error)=w971) -> (error out=w974:errorcluster)  [unwired: 1 in, 2 out]
            n781 = Merge Errors(w972, w974) -> (w973:errorcluster)
          }
          frame Default {
            # "'Default' case only runs if there is a message that isn't defined in any of the other cases.  Output a programming error."
            n782 = xnode ("Error Ring")("parameter 0"=w978) -> ("error out"=w979:errorcluster)
          }
        }
        n783 = call "LAB-IQ Error Handler - Message Handling Loop.vi"("error in (no error)"=w926, "Message Queue"=w928) -> ("dup error in"=w927:errorcluster)  [unwired: 8 in, 1 out]
      }
    }
    frame Enabled {
    }
  }
  n784 = disable-structure "Diagram Disable Structure" shown="Enabled" {
    disable-tunnel: w9 -> [w993 _]
    disable-tunnel: w47 -> [w992 _]
    disable-tunnel: w48 -> [w991 _]
    disable-tunnel: w18 -> [w990 w1059]
    disable-tunnel: [w989 w1059] -> w54
    frame Disabled {
      n785 = while {
        shift-right: [w1004] -> _
        shift-left: w992 -> [w1005]
        tunnel: [w998] -> w989
        tunnel: w993 -> [w996]
        tunnel: w990 -> [w995]
        tunnel: w991 -> [w994]
        stop <- w1003 stop-if-true
        # "ECR  Handling Loop"
        n786 = call "Dequeue Message.vi"("error in (no error)"=w995, "Message Queue"=w996) -> ("error out"=w1002:errorcluster, "output data"=w1000:dbl[][], "Message"=w1001:string, "dup Message Queue"=w999:refnum<queue>)  [unwired: 6 in]
        n787 = case "Message Cases" shown="\"ECR Main\"" w1001 {
          selector: w1001 -> [_ _ _ _ _ w1049]
          tunnel: w999 -> [w1006 w1017 _ w1036 w1048 _]
          tunnel: w1002 -> [w1009 w1014 w1033 w1040 w1042 _]
          tunnel: [w1010 w1018 w1027 w1038 w1044 w1050] -> w997
          tunnel: w1005 -> [w1008 w1016 w1032 w1039 w1047 w1051]
          tunnel: [w1008 w1016 w1032 w1039 w1047 w1051] -> w1004
          tunnel: [_ _ _ _ TRUE _] -> w1003
          tunnel: w1000 -> [_ _ w1031 _ _ _]
          tunnel: w994 -> [_ _ _ _ w1041 _]
          frame "init" {
            # "Initialize - All initialization work should take place in this message, since other loops can potentially enqueue messages that execute immediately after this one."
            n788 = call-poly "Enqueue Message.vi"("error in (no error)"=w1009, "Message"="ECR Main", "Message Queue"=w1006) -> ("error out"=w1010:errorcluster)  [unwired: 7 in, 1 out]
          }
          frame "ECR Main" {
            n789 = Unbundle By Name(w1016) -> ("Main Home Screen.EXIT"=w1015:refnum<vi>)
            n790 = property on="Property Node" class="Bool (strict)"(reference=w1015) -> (reference out=w1012:refnum<vi>, error out=w1013:errorcluster, "Value"=w1011:bool)  [unwired: 1 in]
            n791 = case shown="False" w1011 {
              tunnel: [w1021 w1025] -> w1018
              tunnel: w1017 -> [w1020 w1024]
              tunnel: w1014 -> [w1019 w1023]
              frame True {
                n792 = call-poly "Enqueue Message.vi"("error in (no error)"=w1019, "Message"="Confirm Quit", "Message Queue"=w1020) -> ("error out"=w1021:errorcluster)  [unwired: 7 in, 1 out]
              }
              frame False {
                n793 = call-poly "Enqueue Message.vi"("error in (no error)"=w1023, "Message"="ECR Main", "Message Queue"=w1024) -> ("error out"=w1025:errorcluster)  [unwired: 7 in, 1 out]
              }
            }
            n794 = Close Reference(reference=w1012, error in (no error)=w1013) -> ()  [unwired: 1 out]
          }
          frame "Error" {
            # "#CodeRecommended - If you ever change the name of this \"Error\" message, you'll need to update the name in the Check Loop Error.vi as well."
            # "#CodeRecommended - Consider creating a system for logging errors in some way. These errors are for notification purposes only. Handling of specific errors should be performed in the message frames that generated the error."
            # "Error - Display an error dialog. This message is sent by the \"Error Handler\" VIs at the end of other loops in this application."
            n795 = Variant To Data(error in=w1033, type=errorcluster {"status"=FALSE, "code"=0, "source"=""} ("error constant"), Variant=w1031) -> (data=w1029:errorcluster, error out=w1028:errorcluster)
            n796 = call <vilib>:"Simple Error Handler.vi"("error in (no error)"=w1029) -> ()  [unwired: 4 in, 5 out]
            n797 = Merge Errors(w1028) -> (w1027:errorcluster)
          }
          frame "Confirm Quit" {
            # "#CodeNeeded - If you want to provide an \"Are you sure\" dialog (or some other notification) before the application exits, place that code here. This message is typically sent from a Panel Close? event."
            # "Confirm Quit - Message that can confirm whether or not the user wants to exit the application."
            n798 = call-poly "Enqueue Message.vi"("Priority Message? (F)"=TRUE, "error in (no error)"=w1040, "Message"="Exit", "Message Queue"=w1036) -> ("error out"=w1037:errorcluster)  [unwired: 6 in, 1 out]
            n799 = Merge Errors(w1037) -> (w1038:errorcluster)
          }
          frame "Exit" {
            # "Stop the VI"
            # "Release the message queue reference"
            # "#CodeNeeded - Add any required cleanup code here. Note that if 'Exit' was called as a result of an error, an error dialog will be displayed. Add any custom error handling for an 'Exit' condition here as well."
            # "Exit - Exit the application."
            n800 = call "Fire User Event - Stop.vi"("User Event - Stop"=w1041) -> ("error out"=w1043:errorcluster)  [unwired: 10 in]
            n801 = Release Queue(queue=w1048, error in (no error)=w1042) -> (error out=w1045:errorcluster)  [unwired: 1 in, 2 out]
            n802 = Merge Errors(w1043, w1045) -> (w1044:errorcluster)
          }
          frame Default {
            # "'Default' case only runs if there is a message that isn't defined in any of the other cases.  Output a programming error."
            n803 = xnode ("Error Ring")("parameter 0"=w1049) -> ("error out"=w1050:errorcluster)
          }
        }
        n804 = call "LAB-IQ Error Handler - Message Handling Loop.vi"("error in (no error)"=w997, "Message Queue"=w999) -> ("dup error in"=w998:errorcluster)  [unwired: 8 in, 1 out]
      }
    }
    frame Enabled {
    }
  }
  n805 = while {
    tunnel: w16 -> [w1067]
    shift-right: [w1065] -> w93
    shift-left: w90 -> [w1066]
    tunnel: [w1061] -> w91
    stop <- w1063 stop-if-true
    # "Event Handling Loop"
    n806 = event shown="[85] \"Heater\": Value Change" {
      selector: w1066 -> [_ _ _ _ _ _ _ _ _ _ _ _ _ _ _ _ _ _ _ _ _ _ _ _ _ _ _ _ _ _ _ _ _ _ _ _ _ _ _ _ _ _ _ _ _ _ _ _ _ _ _ _ _ _ _ _ _ _ _ _ _ _ _ _ _ _ _ _ _ _ _ _ _ _ _ _ _ _ _ _ _ _ _ _ _ _ _ _ _]
      dyn-events: [_ _ _ _ _ _ _ _ _ _ _ _ _ _ _ _ _ _ _ _ _ _ _ _ _ _ _ _ _ _ _ _ _ _ _ _ _ _ _ _ _ _ _ _ _ _ _ _ _ _ _ _ _ _ _ _ _ _ _ _ _ _ _ _ _ _ _ _ _ _ _ _ _ _ _ _ _ _ _ _ _ _ _ _ _ _ _ _ _] -> w1065
      timeout: 100 -> [_ _ _ _ _ _ _ _ _ _ _ _ _ _ _ _ _ _ _ _ _ _ _ _ _ _ _ _ _ _ _ _ _ _ _ _ _ _ _ _ _ _ _ _ _ _ _ _ _ _ _ _ _ _ _ _ _ _ _ _ _ _ _ _ _ _ _ _ _ _ _ _ _ _ _ _ _ _ _ _ _ _ _ _ _ _ _ _ _]
      tunnel: [_ _ _ _ _ _ _ _ _ _ _ _ _ _ _ _ _ _ _ _ _ _ _ _ _ _ _ _ _ _ _ _ _ _ _ _ _ _ _ _ _ _ _ _ _ _ _ _ _ _ _ _ _ _ _ _ _ _ _ _ _ _ _ _ _ _ _ _ _ _ _ _ _ _ _ _ _ _ _ _ _ _ _ _ _ _ _ _ TRUE ("Discard?")] -> w1063
      tunnel: w1067 -> [w1068 w1074 w1079 w1084 w1089 w1094 w1099 w1104 w1109 w1114 w1119 w1124 w1129 w1134 w1139 w1144 w1149 w1154 w1159 w1164 w1169 w1174 w1179 w1184 w1189 w1194 w1199 w1204 w1209 w1214 w1219 w1224 w1229 w1234 w1239 w1244 w1249 w1254 w1259 w1264 w1269 w1274 w1279 w1284 w1289 w1294 w1299 w1304 w1309 w1314 w1319 w1324 w1329 w1334 w1339 w1344 w1349 w1354 w1359 w1364 w1369 w1374 w1379 w1384 w1389 w1394 w1399 w1404 w1409 w1414 w1419 w1424 w1429 w1434 w1439 w1444 w1449 w1454 w1459 w1464 w1469 w1474 w1479 w1484 w1489 w1494 w1499 w1500 w1505]
      tunnel: [w1072 w1078 w1080 w1085 w1090 w1095 w1100 w1105 w1110 w1115 w1120 w1125 w1130 w1135 w1140 w1145 w1150 w1155 w1160 w1165 w1170 w1175 w1180 w1185 w1190 w1195 w1200 w1205 w1210 w1215 w1220 w1225 w1230 w1235 w1240 w1245 w1250 w1255 w1260 w1265 w1270 w1275 w1280 w1285 w1290 w1295 w1300 w1305 w1310 w1315 w1320 w1325 w1330 w1335 w1340 w1345 w1350 w1355 w1360 w1365 w1370 w1375 w1380 w1385 w1390 w1395 w1400 w1405 w1410 w1415 w1420 w1425 w1430 w1435 w1440 w1445 w1450 w1455 w1460 w1465 w1470 w1475 w1480 w1485 w1490 w1495 _ w1504 _] -> w1064
      tunnel: [w1071 w1077 w1081 w1086 w1091 w1096 w1101 w1106 w1111 w1116 w1121 w1126 w1131 w1136 w1141 w1146 w1151 w1156 w1161 w1166 w1171 w1176 w1181 w1186 w1191 w1196 w1201 w1206 w1211 w1216 w1221 w1226 w1231 w1236 w1241 w1246 w1251 w1256 w1261 w1266 w1271 w1276 w1281 w1286 w1291 w1296 w1301 w1306 w1311 w1316 w1321 w1326 w1331 w1336 w1341 w1346 w1351 w1356 w1361 w1366 w1371 w1376 w1381 w1386 w1391 w1396 w1401 w1406 w1411 w1416 w1421 w1426 w1431 w1436 w1441 w1446 w1451 w1456 w1461 w1466 w1471 w1476 w1481 w1486 w1491 w1496 w1499 w1503 w1505] -> w1062
      event Panel Close? {
        n807 = event-data() -> ()  [unwired: 1 in, 1 out]
        n808 = call-poly "Enqueue Message.vi"("Priority Message? (F)"=TRUE, "Message"="Confirm Quit", "Message Queue"=w1068) -> ("error out"=w1072:errorcluster, "dup Message Queue"=w1071:refnum<queue>)  [unwired: 7 in]
        n809 = event-data ("Event Filter Node")("Discard?"=TRUE) -> ()  [unwired: 1 in, 1 out]
      }
      event Timeout {
        n810 = event-data() -> ()  [unwired: 1 in, 1 out]
        n811 = call-poly "Enqueue Message.vi"("Priority Message? (F)"=TRUE, "Message"="Timeout", "Message Queue"=w1074) -> ("error out"=w1078:errorcluster, "dup Message Queue"=w1077:refnum<queue>)  [unwired: 7 in]
      }
      event "SAVE  2": Value Change {
        n812 = event-data() -> ()  [unwired: 1 in, 1 out]
        n813 = call-poly "Enqueue Message.vi"("Priority Message? (F)"=TRUE, "Message"="Service Save", "Message Queue"=w1079) -> ("error out"=w1080:errorcluster, "dup Message Queue"=w1081:refnum<queue>)  [unwired: 7 in]
      }
      event "Home": Value Change {
        n814 = event-data() -> ()  [unwired: 1 in, 1 out]
        n815 = call-poly "Enqueue Message.vi"("Priority Message? (F)"=TRUE, "Message"="HOME", "Message Queue"=w1084) -> ("error out"=w1085:errorcluster, "dup Message Queue"=w1086:refnum<queue>)  [unwired: 7 in]
      }
      event "Platform Settings": Value Change {
        n816 = event-data() -> ()  [unwired: 1 in, 1 out]
        n817 = call-poly "Enqueue Message.vi"("Priority Message? (F)"=TRUE, "Message"="Platform Setting", "Message Queue"=w1089) -> ("error out"=w1090:errorcluster, "dup Message Queue"=w1091:refnum<queue>)  [unwired: 7 in]
      }
      event "Configure": Value Change {
        n818 = event-data() -> ()  [unwired: 1 in, 1 out]
        n819 = call-poly "Enqueue Message.vi"("Priority Message? (F)"=TRUE, "Message"="Configure", "Message Queue"=w1094) -> ("error out"=w1095:errorcluster, "dup Message Queue"=w1096:refnum<queue>)  [unwired: 7 in]
      }
      event "Analysis": Value Change {
        n820 = event-data() -> ()  [unwired: 1 in, 1 out]
        n821 = call-poly "Enqueue Message.vi"("Priority Message? (F)"=TRUE, "Message"="Analysis", "Message Queue"=w1099) -> ("error out"=w1100:errorcluster, "dup Message Queue"=w1101:refnum<queue>)  [unwired: 7 in]
      }
      event "service 2": Value Change {
        n822 = event-data() -> ()  [unwired: 1 in, 1 out]
        n823 = call-poly "Enqueue Message.vi"("Priority Message? (F)"=TRUE, "Message"="service 2", "Message Queue"=w1104) -> ("error out"=w1105:errorcluster, "dup Message Queue"=w1106:refnum<queue>)  [unwired: 7 in]
      }
      event "Auto": Value Change {
        n824 = event-data() -> ()  [unwired: 1 in, 1 out]
        n825 = call-poly "Enqueue Message.vi"("Priority Message? (F)"=TRUE, "Message"="Auto", "Message Queue"=w1109) -> ("error out"=w1110:errorcluster, "dup Message Queue"=w1111:refnum<queue>)  [unwired: 7 in]
      }
      event "Select Load Head": Value Change {
        n826 = event-data() -> ()  [unwired: 1 in, 1 out]
        n827 = call-poly "Enqueue Message.vi"("Priority Message? (F)"=TRUE, "Message"="Select Load Head", "Message Queue"=w1114) -> ("error out"=w1115:errorcluster, "dup Message Queue"=w1116:refnum<queue>)  [unwired: 7 in]
      }
      event "com 3": Value Change {
        n828 = event-data() -> ()  [unwired: 1 in, 1 out]
        n829 = call-poly "Enqueue Message.vi"("Priority Message? (F)"=TRUE, "Message"="com 3", "Message Queue"=w1119) -> ("error out"=w1120:errorcluster, "dup Message Queue"=w1121:refnum<queue>)  [unwired: 7 in]
      }
      event "Loading Mode": Value Change {
        n830 = event-data() -> ()  [unwired: 1 in, 1 out]
        n831 = call-poly "Enqueue Message.vi"("Priority Message? (F)"=TRUE, "Message"="Loading Mode", "Message Queue"=w1124) -> ("error out"=w1125:errorcluster, "dup Message Queue"=w1126:refnum<queue>)  [unwired: 7 in]
      }
      event "SSP 0.3": Value Change {
        n832 = event-data() -> ()  [unwired: 1 in, 1 out]
        n833 = call-poly "Enqueue Message.vi"("Priority Message? (F)"=TRUE, "Message"="SSP 0.3", "Message Queue"=w1129) -> ("error out"=w1130:errorcluster, "dup Message Queue"=w1131:refnum<queue>)  [unwired: 7 in]
      }
      event "SSP 0.5": Value Change {
        n834 = event-data() -> ()  [unwired: 1 in, 1 out]
        n835 = call-poly "Enqueue Message.vi"("Priority Message? (F)"=TRUE, "Message"="SSP 0.5", "Message Queue"=w1134) -> ("error out"=w1135:errorcluster, "dup Message Queue"=w1136:refnum<queue>)  [unwired: 7 in]
      }
      event "SSP 0.75": Value Change {
        n836 = event-data() -> ()  [unwired: 1 in, 1 out]
        n837 = call-poly "Enqueue Message.vi"("Priority Message? (F)"=TRUE, "Message"="SSP 0.75", "Message Queue"=w1139) -> ("error out"=w1140:errorcluster, "dup Message Queue"=w1141:refnum<queue>)  [unwired: 7 in]
      }
      event "LHBack": Value Change {
        n838 = event-data() -> ()  [unwired: 1 in, 1 out]
        n839 = call-poly "Enqueue Message.vi"("Priority Message? (F)"=TRUE, "Message"="LHBack", "Message Queue"=w1144) -> ("error out"=w1145:errorcluster, "dup Message Queue"=w1146:refnum<queue>)  [unwired: 7 in]
      }
      event "LHNext": Value Change {
        n840 = event-data() -> ()  [unwired: 1 in, 1 out]
        n841 = call-poly "Enqueue Message.vi"("Priority Message? (F)"=TRUE, "Message"="LHNext", "Message Queue"=w1149) -> ("error out"=w1150:errorcluster, "dup Message Queue"=w1151:refnum<queue>)  [unwired: 7 in]
      }
      event "Rot Ver": Value Change {
        n842 = event-data() -> ()  [unwired: 1 in, 1 out]
        n843 = call-poly "Enqueue Message.vi"("Priority Message? (F)"=TRUE, "Message"="Rot Ver", "Message Queue"=w1154) -> ("error out"=w1155:errorcluster, "dup Message Queue"=w1156:refnum<queue>)  [unwired: 7 in]
      }
      event "Traction": Value Change {
        n844 = event-data() -> ()  [unwired: 1 in, 1 out]
        n845 = call-poly "Enqueue Message.vi"("Priority Message? (F)"=TRUE, "Message"="Traction", "Message Queue"=w1159) -> ("error out"=w1160:errorcluster, "dup Message Queue"=w1161:refnum<queue>)  [unwired: 7 in]
      }
      event "Scratch": Value Change {
        n846 = event-data() -> ()  [unwired: 1 in, 1 out]
        n847 = call-poly "Enqueue Message.vi"("Priority Message? (F)"=TRUE, "Message"="Scratch", "Message Queue"=w1164) -> ("error out"=w1165:errorcluster, "dup Message Queue"=w1166:refnum<queue>)  [unwired: 7 in]
      }
      event "Motion Mode:": Value Change {
        n848 = event-data() -> ()  [unwired: 1 in, 1 out]
        n849 = call-poly "Enqueue Message.vi"("Priority Message? (F)"=TRUE, "Message"="Motion Mode:", "Message Queue"=w1169) -> ("error out"=w1170:errorcluster, "dup Message Queue"=w1171:refnum<queue>)  [unwired: 7 in]
      }
      event "MMBack": Value Change {
        n850 = event-data() -> ()  [unwired: 1 in, 1 out]
        n851 = call-poly "Enqueue Message.vi"("Priority Message? (F)"=TRUE, "Message"="MMBack", "Message Queue"=w1174) -> ("error out"=w1175:errorcluster, "dup Message Queue"=w1176:refnum<queue>)  [unwired: 7 in]
      }
      event "MMNext": Value Change {
        n852 = event-data() -> ()  [unwired: 1 in, 1 out]
        n853 = call-poly "Enqueue Message.vi"("Priority Message? (F)"=TRUE, "Message"="MMNext", "Message Queue"=w1179) -> ("error out"=w1180:errorcluster, "dup Message Queue"=w1181:refnum<queue>)  [unwired: 7 in]
      }
      event "APBack": Value Change {
        n854 = event-data() -> ()  [unwired: 1 in, 1 out]
        n855 = call-poly "Enqueue Message.vi"("Priority Message? (F)"=TRUE, "Message"="APBack", "Message Queue"=w1184) -> ("error out"=w1185:errorcluster, "dup Message Queue"=w1186:refnum<queue>)  [unwired: 7 in]
      }
      event "SNext": Value Change {
        n856 = event-data() -> ()  [unwired: 1 in, 1 out]
        n857 = call-poly "Enqueue Message.vi"("Priority Message? (F)"=TRUE, "Message"="SNext", "Message Queue"=w1189) -> ("error out"=w1190:errorcluster, "dup Message Queue"=w1191:refnum<queue>)  [unwired: 7 in]
      }
      event "Load Cell Link.ZeroAll": Value Change {
        n858 = event-data() -> ()  [unwired: 1 in, 1 out]
        n859 = call-poly "Enqueue Message.vi"("Priority Message? (F)"=TRUE, "Message"="ZeroAll", "Message Queue"=w1194) -> ("error out"=w1195:errorcluster, "dup Message Queue"=w1196:refnum<queue>)  [unwired: 7 in]
      }
      event "Enable Platform": Value Change {
        n860 = event-data() -> ()  [unwired: 1 in, 1 out]
        n861 = call-poly "Enqueue Message.vi"("Priority Message? (F)"=TRUE, "Message"="Enable Platform", "Message Queue"=w1199) -> ("error out"=w1200:errorcluster, "dup Message Queue"=w1201:refnum<queue>)  [unwired: 7 in]
      }
      event "Heave Up main": Value Change {
        n862 = event-data() -> ()  [unwired: 1 in, 1 out]
        n863 = call-poly "Enqueue Message.vi"("Priority Message? (F)"=TRUE, "Message"="Heave Up main", "Message Queue"=w1204) -> ("error out"=w1205:errorcluster, "dup Message Queue"=w1206:refnum<queue>)  [unwired: 7 in]
      }
      event "Heave Up MM": Value Change {
        n864 = event-data() -> ()  [unwired: 1 in, 1 out]
        n865 = call-poly "Enqueue Message.vi"("Priority Message? (F)"=TRUE, "Message"="Heave Up MM", "Message Queue"=w1209) -> ("error out"=w1210:errorcluster, "dup Message Queue"=w1211:refnum<queue>)  [unwired: 7 in]
      }
      event "Heave Down Main": Value Change {
        n866 = event-data() -> ()  [unwired: 1 in, 1 out]
        n867 = call-poly "Enqueue Message.vi"("Priority Message? (F)"=TRUE, "Message"="Heave Down Main", "Message Queue"=w1214) -> ("error out"=w1215:errorcluster, "dup Message Queue"=w1216:refnum<queue>)  [unwired: 7 in]
      }
      event "Heave Down MM": Value Change {
        n868 = event-data() -> ()  [unwired: 1 in, 1 out]
        n869 = call-poly "Enqueue Message.vi"("Priority Message? (F)"=TRUE, "Message"="Heave Down MM", "Message Queue"=w1219) -> ("error out"=w1220:errorcluster, "dup Message Queue"=w1221:refnum<queue>)  [unwired: 7 in]
      }
      event "Manual Write Heave & Surge": Value Change {
        n870 = event-data() -> ()  [unwired: 1 in, 1 out]
        n871 = call-poly "Enqueue Message.vi"("Priority Message? (F)"=TRUE, "Message"="Manual Write Heave & Surge", "Message Queue"=w1224) -> ("error out"=w1225:errorcluster, "dup Message Queue"=w1226:refnum<queue>)  [unwired: 7 in]
      }
      event "Manual Write SWAY": Value Change {
        n872 = event-data() -> ()  [unwired: 1 in, 1 out]
        n873 = call-poly "Enqueue Message.vi"("Priority Message? (F)"=TRUE, "Message"="Manual Write SWAY", "Message Queue"=w1229) -> ("error out"=w1230:errorcluster, "dup Message Queue"=w1231:refnum<queue>)  [unwired: 7 in]
      }
      event "Surge Backward Main": Value Change {
        n874 = event-data() -> ()  [unwired: 1 in, 1 out]
        n875 = call-poly "Enqueue Message.vi"("Priority Message? (F)"=TRUE, "Message"="Surge Backward Main", "Message Queue"=w1234) -> ("error out"=w1235:errorcluster, "dup Message Queue"=w1236:refnum<queue>)  [unwired: 7 in]
      }
      event "Surge Backward MM": Value Change {
        n876 = event-data() -> ()  [unwired: 1 in, 1 out]
        n877 = call-poly "Enqueue Message.vi"("Priority Message? (F)"=TRUE, "Message"="Surge Backward MM", "Message Queue"=w1239) -> ("error out"=w1240:errorcluster, "dup Message Queue"=w1241:refnum<queue>)  [unwired: 7 in]
      }
      event "Surge Forward Main": Value Change {
        n878 = event-data() -> ()  [unwired: 1 in, 1 out]
        n879 = call-poly "Enqueue Message.vi"("Priority Message? (F)"=TRUE, "Message"="Surge Forward Main", "Message Queue"=w1244) -> ("error out"=w1245:errorcluster, "dup Message Queue"=w1246:refnum<queue>)  [unwired: 7 in]
      }
      event "Surge Forward MM": Value Change {
        n880 = event-data() -> ()  [unwired: 1 in, 1 out]
        n881 = call-poly "Enqueue Message.vi"("Priority Message? (F)"=TRUE, "Message"="Surge Forward MM", "Message Queue"=w1249) -> ("error out"=w1250:errorcluster, "dup Message Queue"=w1251:refnum<queue>)  [unwired: 7 in]
      }
      event "Sway Left Main": Value Change {
        n882 = event-data() -> ()  [unwired: 1 in, 1 out]
        n883 = call-poly "Enqueue Message.vi"("Priority Message? (F)"=TRUE, "Message"="Sway Left Main", "Message Queue"=w1254) -> ("error out"=w1255:errorcluster, "dup Message Queue"=w1256:refnum<queue>)  [unwired: 7 in]
      }
      event "Sway Left MM": Value Change {
        n884 = event-data() -> ()  [unwired: 1 in, 1 out]
        n885 = call-poly "Enqueue Message.vi"("Priority Message? (F)"=TRUE, "Message"="Sway Left MM", "Message Queue"=w1259) -> ("error out"=w1260:errorcluster, "dup Message Queue"=w1261:refnum<queue>)  [unwired: 7 in]
      }
      event "Sway Right MM": Value Change {
        n886 = event-data() -> ()  [unwired: 1 in, 1 out]
        n887 = call-poly "Enqueue Message.vi"("Priority Message? (F)"=TRUE, "Message"="Sway Right MM", "Message Queue"=w1264) -> ("error out"=w1265:errorcluster, "dup Message Queue"=w1266:refnum<queue>)  [unwired: 7 in]
      }
      event "Sway Right Main": Value Change {
        n888 = event-data() -> ()  [unwired: 1 in, 1 out]
        n889 = call-poly "Enqueue Message.vi"("Priority Message? (F)"=TRUE, "Message"="Sway Right Main", "Message Queue"=w1269) -> ("error out"=w1270:errorcluster, "dup Message Queue"=w1271:refnum<queue>)  [unwired: 7 in]
      }
      event "Load En": Value Change {
        n890 = event-data() -> ()  [unwired: 1 in, 1 out]
        n891 = call-poly "Enqueue Message.vi"("Priority Message? (F)"=TRUE, "Message"="Load En", "Message Queue"=w1274) -> ("error out"=w1275:errorcluster, "dup Message Queue"=w1276:refnum<queue>)  [unwired: 7 in]
      }
      event "PID.apply load": Value Change {
        n892 = event-data() -> ()  [unwired: 1 in, 1 out]
        n893 = call-poly "Enqueue Message.vi"("Priority Message? (F)"=TRUE, "Message"="apply load", "Message Queue"=w1279) -> ("error out"=w1280:errorcluster, "dup Message Queue"=w1281:refnum<queue>)  [unwired: 7 in]
      }
      event "BACK": Value Change {
        n894 = event-data() -> ()  [unwired: 1 in, 1 out]
        n895 = call-poly "Enqueue Message.vi"("Priority Message? (F)"=TRUE, "Message"="BACK", "Message Queue"=w1284) -> ("error out"=w1285:errorcluster, "dup Message Queue"=w1286:refnum<queue>)  [unwired: 7 in]
      }
      event "Start Test": Value Change {
        n896 = event-data() -> ()  [unwired: 1 in, 1 out]
        n897 = call-poly "Enqueue Message.vi"("Priority Message? (F)"=TRUE, "Message"="Start Test", "Message Queue"=w1289) -> ("error out"=w1290:errorcluster, "dup Message Queue"=w1291:refnum<queue>)  [unwired: 7 in]
      }
      event "STOP": Value Change {
        n898 = event-data() -> ()  [unwired: 1 in, 1 out]
        n899 = call-poly "Enqueue Message.vi"("Priority Message? (F)"=TRUE, "Message"="STOP", "Message Queue"=w1294) -> ("error out"=w1295:errorcluster, "dup Message Queue"=w1296:refnum<queue>)  [unwired: 7 in]
      }
      event "PlaceModule": Value Change {
        n900 = event-data() -> ()  [unwired: 1 in, 1 out]
        n901 = call-poly "Enqueue Message.vi"("Priority Message? (F)"=TRUE, "Message"="PlaceModule", "Message Queue"=w1299) -> ("error out"=w1300:errorcluster, "dup Message Queue"=w1301:refnum<queue>)  [unwired: 7 in]
      }
      event "HomeRot", "HomeScratch", "HomeScratch": Value Change {
        n902 = event-data() -> ()  [unwired: 1 in, 1 out]
        n903 = call-poly "Enqueue Message.vi"("Priority Message? (F)"=TRUE, "Message"="Stage Homing", "Message Queue"=w1304) -> ("error out"=w1305:errorcluster, "dup Message Queue"=w1306:refnum<queue>)  [unwired: 7 in]
      }
      event "Clear 3": Value Change {
        n904 = event-data() -> ()  [unwired: 1 in, 1 out]
        n905 = call-poly "Enqueue Message.vi"("Priority Message? (F)"=TRUE, "Message"="Clear 3", "Message Queue"=w1309) -> ("error out"=w1310:errorcluster, "dup Message Queue"=w1311:refnum<queue>)  [unwired: 7 in]
      }
      event "Set WTD": Value Change {
        n906 = event-data() -> ()  [unwired: 1 in, 1 out]
        n907 = call-poly "Enqueue Message.vi"("Priority Message? (F)"=TRUE, "Message"="Set WTD", "Message Queue"=w1314) -> ("error out"=w1315:errorcluster, "dup Message Queue"=w1316:refnum<queue>)  [unwired: 7 in]
      }
      event "Import 2": Value Change {
        n908 = event-data() -> ()  [unwired: 1 in, 1 out]
        n909 = call-poly "Enqueue Message.vi"("Priority Message? (F)"=TRUE, "Message"="Import 2", "Message Queue"=w1319) -> ("error out"=w1320:errorcluster, "dup Message Queue"=w1321:refnum<queue>)  [unwired: 7 in]
      }
      event "Import 3": Value Change {
        n910 = event-data() -> ()  [unwired: 1 in, 1 out]
        n911 = call-poly "Enqueue Message.vi"("Priority Message? (F)"=TRUE, "Message"="Import 3", "Message Queue"=w1324) -> ("error out"=w1325:errorcluster, "dup Message Queue"=w1326:refnum<queue>)  [unwired: 7 in]
      }
      event "Save 2": Value Change {
        n912 = event-data() -> ()  [unwired: 1 in, 1 out]
        n913 = call-poly "Enqueue Message.vi"("Priority Message? (F)"=TRUE, "Message"="Save 2", "Message Queue"=w1329) -> ("error out"=w1330:errorcluster, "dup Message Queue"=w1331:refnum<queue>)  [unwired: 7 in]
      }
      event "Save 3": Value Change {
        n914 = event-data() -> ()  [unwired: 1 in, 1 out]
        n915 = call-poly "Enqueue Message.vi"("Priority Message? (F)"=TRUE, "Message"="Save 3", "Message Queue"=w1334) -> ("error out"=w1335:errorcluster, "dup Message Queue"=w1336:refnum<queue>)  [unwired: 7 in]
      }
      event "calculate rotary": Value Change {
        n916 = event-data() -> ()  [unwired: 1 in, 1 out]
        n917 = call-poly "Enqueue Message.vi"("Priority Message? (F)"=TRUE, "Message"="Calculate Rotary", "Message Queue"=w1339) -> ("error out"=w1340:errorcluster, "dup Message Queue"=w1341:refnum<queue>)  [unwired: 7 in]
      }
      event "Clear List": Value Change {
        n918 = event-data() -> ()  [unwired: 1 in, 1 out]
        n919 = call-poly "Enqueue Message.vi"("Priority Message? (F)"=TRUE, "Message"="Clear List", "Message Queue"=w1344) -> ("error out"=w1345:errorcluster, "dup Message Queue"=w1346:refnum<queue>)  [unwired: 7 in]
      }
      event "Add to list": Value Change {
        n920 = event-data() -> ()  [unwired: 1 in, 1 out]
        n921 = call-poly "Enqueue Message.vi"("Priority Message? (F)"=TRUE, "Message"="Add to list", "Message Queue"=w1349) -> ("error out"=w1350:errorcluster, "dup Message Queue"=w1351:refnum<queue>)  [unwired: 7 in]
      }
      event "ClrLog": Value Change {
        n922 = event-data() -> ()  [unwired: 1 in, 1 out]
        n923 = call-poly "Enqueue Message.vi"("Priority Message? (F)"=TRUE, "Message"="ClrLog", "Message Queue"=w1354) -> ("error out"=w1355:errorcluster, "dup Message Queue"=w1356:refnum<queue>)  [unwired: 7 in]
      }
      event "Disable Axis Jog Soft Limits m": Value Change {
        n924 = event-data() -> ()  [unwired: 1 in, 1 out]
        n925 = call-poly "Enqueue Message.vi"("Priority Message? (F)"=TRUE, "Message"="Disable Axis Jog Soft Limits", "Message Queue"=w1359) -> ("error out"=w1360:errorcluster, "dup Message Queue"=w1361:refnum<queue>)  [unwired: 7 in]
      }
      event "Home Service": Value Change {
        n926 = event-data() -> ()  [unwired: 1 in, 1 out]
        n927 = call-poly "Enqueue Message.vi"("Priority Message? (F)"=TRUE, "Message"="Home Service", "Message Queue"=w1364) -> ("error out"=w1365:errorcluster, "dup Message Queue"=w1366:refnum<queue>)  [unwired: 7 in]
      }
      event "Edit Gain Constants": Value Change {
        n928 = event-data() -> ()  [unwired: 1 in, 1 out]
        n929 = call-poly "Enqueue Message.vi"("Priority Message? (F)"=TRUE, "Message"="Edit Gain Constants", "Message Queue"=w1369) -> ("error out"=w1370:errorcluster, "dup Message Queue"=w1371:refnum<queue>)  [unwired: 7 in]
      }
      event "Advanced Setting": Value Change {
        n930 = event-data() -> ()  [unwired: 1 in, 1 out]
        n931 = call-poly "Enqueue Message.vi"("Priority Message? (F)"=TRUE, "Message"="Advanced Setting", "Message Queue"=w1374) -> ("error out"=w1375:errorcluster, "dup Message Queue"=w1376:refnum<queue>)  [unwired: 7 in]
      }
      event "Password": Value Change {
        n932 = event-data() -> ()  [unwired: 1 in, 1 out]
        n933 = call-poly "Enqueue Message.vi"("Priority Message? (F)"=TRUE, "Message"="Password", "Message Queue"=w1379) -> ("error out"=w1380:errorcluster, "dup Message Queue"=w1381:refnum<queue>)  [unwired: 7 in]
      }
      event "Service About": Value Change {
        n934 = event-data() -> ()  [unwired: 1 in, 1 out]
        n935 = call-poly "Enqueue Message.vi"("Priority Message? (F)"=TRUE, "Message"="Service About", "Message Queue"=w1384) -> ("error out"=w1385:errorcluster, "dup Message Queue"=w1386:refnum<queue>)  [unwired: 7 in]
      }
      event "OPEN 1": Value Change {
        n936 = event-data() -> ()  [unwired: 1 in, 1 out]
        n937 = call-poly "Enqueue Message.vi"("Priority Message? (F)"=TRUE, "Message"="OPEN 1", "Message Queue"=w1389) -> ("error out"=w1390:errorcluster, "dup Message Queue"=w1391:refnum<queue>)  [unwired: 7 in]
      }
      event "OPEN 2": Value Change {
        n938 = event-data() -> ()  [unwired: 1 in, 1 out]
        n939 = call-poly "Enqueue Message.vi"("Priority Message? (F)"=TRUE, "Message"="OPEN 2", "Message Queue"=w1394) -> ("error out"=w1395:errorcluster, "dup Message Queue"=w1396:refnum<queue>)  [unwired: 7 in]
      }
      event "OPEN 3": Value Change {
        n940 = event-data() -> ()  [unwired: 1 in, 1 out]
        n941 = call-poly "Enqueue Message.vi"("Priority Message? (F)"=TRUE, "Message"="OPEN 3", "Message Queue"=w1399) -> ("error out"=w1400:errorcluster, "dup Message Queue"=w1401:refnum<queue>)  [unwired: 7 in]
      }
      event "OPEN 4": Value Change {
        n942 = event-data() -> ()  [unwired: 1 in, 1 out]
        n943 = call-poly "Enqueue Message.vi"("Priority Message? (F)"=TRUE, "Message"="OPEN 4", "Message Queue"=w1404) -> ("error out"=w1405:errorcluster, "dup Message Queue"=w1406:refnum<queue>)  [unwired: 7 in]
      }
      event "Refresh 2": Value Change {
        n944 = event-data() -> ()  [unwired: 1 in, 1 out]
        n945 = call-poly "Enqueue Message.vi"("Priority Message? (F)"=TRUE, "Message"="Refresh 2", "Message Queue"=w1409) -> ("error out"=w1410:errorcluster, "dup Message Queue"=w1411:refnum<queue>)  [unwired: 7 in]
      }
      event "Analysis Home new": Value Change {
        n946 = event-data() -> ()  [unwired: 1 in, 1 out]
        n947 = call-poly "Enqueue Message.vi"("Priority Message? (F)"=TRUE, "Message"="Analysis Home", "Message Queue"=w1414) -> ("error out"=w1415:errorcluster, "dup Message Queue"=w1416:refnum<queue>)  [unwired: 7 in]
      }
      event "Post Analysis": Value Change {
        n948 = event-data() -> ()  [unwired: 1 in, 1 out]
        n949 = call-poly "Enqueue Message.vi"("Priority Message? (F)"=TRUE, "Message"="Post Analysis", "Message Queue"=w1419) -> ("error out"=w1420:errorcluster, "dup Message Queue"=w1421:refnum<queue>)  [unwired: 7 in]
      }
      event "Scratch Mode": Value Change {
        n950 = event-data() -> ()  [unwired: 1 in, 1 out]
        n951 = call-poly "Enqueue Message.vi"("Priority Message? (F)"=TRUE, "Message"="Scratch Mode", "Message Queue"=w1424) -> ("error out"=w1425:errorcluster, "dup Message Queue"=w1426:refnum<queue>)  [unwired: 7 in]
      }
      event "Export": Value Change {
        n952 = event-data() -> ()  [unwired: 1 in, 1 out]
        n953 = call-poly "Enqueue Message.vi"("Priority Message? (F)"=TRUE, "Message"="Export", "Message Queue"=w1429) -> ("error out"=w1430:errorcluster, "dup Message Queue"=w1431:refnum<queue>)  [unwired: 7 in]
      }
      event "Traction Receipe Update Details": Value Change {
        n954 = event-data() -> ()  [unwired: 1 in, 1 out]
        n955 = call-poly "Enqueue Message.vi"("Priority Message? (F)"=TRUE, "Message"="Traction Receipe Update Details", "Message Queue"=w1434) -> ("error out"=w1435:errorcluster, "dup Message Queue"=w1436:refnum<queue>)  [unwired: 7 in]
      }
      event "Manual Write TRACTION": Value Change {
        n956 = event-data() -> ()  [unwired: 1 in, 1 out]
        n957 = call-poly "Enqueue Message.vi"("Priority Message? (F)"=TRUE, "Message"="Manual Write TRACTION", "Message Queue"=w1439) -> ("error out"=w1440:errorcluster, "dup Message Queue"=w1441:refnum<queue>)  [unwired: 7 in]
      }
      event "Manual Write Acquostic": Value Change {
        n958 = event-data() -> ()  [unwired: 1 in, 1 out]
        n959 = call-poly "Enqueue Message.vi"("Priority Message? (F)"=TRUE, "Message"="Manual Write ACQUOSTIC", "Message Queue"=w1444) -> ("error out"=w1445:errorcluster, "dup Message Queue"=w1446:refnum<queue>)  [unwired: 7 in]
      }
      event "Report": Value Change {
        n960 = event-data() -> ()  [unwired: 1 in, 1 out]
        n961 = call-poly "Enqueue Message.vi"("Priority Message? (F)"=TRUE, "Message"="Report", "Message Queue"=w1449) -> ("error out"=w1450:errorcluster, "dup Message Queue"=w1451:refnum<queue>)  [unwired: 7 in]
      }
      event "Acoustic Emission 3": Value Change {
        n962 = event-data() -> ()  [unwired: 1 in, 1 out]
        n963 = call-poly "Enqueue Message.vi"("Priority Message? (F)"=TRUE, "Message"="Acoustic Emission 3", "Message Queue"=w1454) -> ("error out"=w1455:errorcluster, "dup Message Queue"=w1456:refnum<queue>)  [unwired: 7 in]
      }
      event "Info": Value Change {
        n964 = event-data() -> ()  [unwired: 1 in, 1 out]
        n965 = call-poly "Enqueue Message.vi"("Priority Message? (F)"=TRUE, "Message"="Info", "Message Queue"=w1459) -> ("error out"=w1460:errorcluster, "dup Message Queue"=w1461:refnum<queue>)  [unwired: 7 in]
      }
      event "Clear rot": Value Change {
        n966 = event-data() -> ()  [unwired: 1 in, 1 out]
        n967 = call-poly "Enqueue Message.vi"("Priority Message? (F)"=TRUE, "Message"="Clear rot", "Message Queue"=w1464) -> ("error out"=w1465:errorcluster, "dup Message Queue"=w1466:refnum<queue>)  [unwired: 7 in]
      }
      event "Load Disable Trip": Value Change {
        n968 = event-data() -> ()  [unwired: 1 in, 1 out]
        n969 = call-poly "Enqueue Message.vi"("Priority Message? (F)"=TRUE, "Message"="Load Disable Trip", "Message Queue"=w1469) -> ("error out"=w1470:errorcluster, "dup Message Queue"=w1471:refnum<queue>)  [unwired: 7 in]
      }
      event "COF Disable Trip": Value Change {
        n970 = event-data() -> ()  [unwired: 1 in, 1 out]
        n971 = call-poly "Enqueue Message.vi"("Priority Message? (F)"=TRUE, "Message"="COF Disable Trip", "Message Queue"=w1474) -> ("error out"=w1475:errorcluster, "dup Message Queue"=w1476:refnum<queue>)  [unwired: 7 in]
      }
      event "Depth Trip 2": Value Change {
        n972 = event-data() -> ()  [unwired: 1 in, 1 out]
        n973 = call-poly "Enqueue Message.vi"("Priority Message? (F)"=TRUE, "Message"="Depth Trip 2", "Message Queue"=w1479) -> ("error out"=w1480:errorcluster, "dup Message Queue"=w1481:refnum<queue>)  [unwired: 7 in]
      }
      event "zNL 2": Value Change {
        n974 = event-data() -> ()  [unwired: 1 in, 1 out]
        n975 = call-poly "Enqueue Message.vi"("Priority Message? (F)"=TRUE, "Message"="zNL 2", "Message Queue"=w1484) -> ("error out"=w1485:errorcluster, "dup Message Queue"=w1486:refnum<queue>)  [unwired: 7 in]
      }
      event "High Temp": Value Change {
        n976 = event-data() -> ()  [unwired: 1 in, 1 out]
        n977 = call-poly "Enqueue Message.vi"("Priority Message? (F)"=TRUE, "Message"="High Temp", "Message Queue"=w1489) -> ("error out"=w1490:errorcluster, "dup Message Queue"=w1491:refnum<queue>)  [unwired: 7 in]
      }
      event "Heater": Value Change {
        n978 = event-data() -> ()  [unwired: 1 in, 1 out]
        n979 = call-poly "Enqueue Message.vi"("Priority Message? (F)"=TRUE, "Message"="Heater", "Message Queue"=w1494) -> ("error out"=w1495:errorcluster, "dup Message Queue"=w1496:refnum<queue>)  [unwired: 7 in]
      }
      event Application Instance Close {
        # "#CodeRecommended - When a project closes, all VIs within that project are aborted and leave memory. However, any code placed in this event frame is guaranteed to run to completion, so add any cleanup code that absolutely must happen here."
        n980 = event-data() -> ()  [unwired: 1 in, 1 out]
      }
      event "EXIT": Value Change {
        n981 = event-data() -> ()  [unwired: 1 in, 1 out]
        n982 = call-poly "Enqueue Message.vi"("Priority Message? (F)"=TRUE, "Message"="Exit", "Message Queue"=w1500) -> ("error out"=w1504:errorcluster, "dup Message Queue"=w1503:refnum<queue>)  [unwired: 7 in]
      }
      event User Event {
        # "The Message Handling Loop processed an \"Exit\" message, which fired this event to stop the Event Handling Loop."
        n983 = event-data() -> ()  [unwired: 1 in, 1 out]
      }
    }
    n984 = call "LAB-IQ Error Handler - Event Handling Loop.vi"("error in (no error)"=w1064, "Message Queue"=w1062) -> ("dup error in"=w1061:errorcluster)  [unwired: 8 in, 1 out]
  }
  n985 = while "Timed Loop" {
    shift-right: [w1517] -> _
    shift-left: w47 -> [w1518]
    tunnel: [w1511] -> w68
    tunnel: w14 -> [w1507]
    tunnel: w18 -> [w1509]
    tunnel: w48 -> [w1508]
    stop <- w1516 stop-if-true
    # "Heave Motor  Handling Loop"
    n986 = call "Dequeue Message.vi"("error in (no error)"=w1509, "Message Queue"=w1507) -> ("error out"=w1515:errorcluster, "output data"=w1513:dbl[][], "Message"=w1514:string, "dup Message Queue"=w1512:refnum<queue>)  [unwired: 6 in]
    n987 = case "Message Cases" shown="\"Heave Main\"" w1514 {
      selector: w1514 -> [_ _ _ _ _ w1607]
      tunnel: w1512 -> [w1531 w1547 _ w1595 w1606 _]
      tunnel: w1515 -> [w1528 w1545 w1585 w1598 w1600 _]
      tunnel: [w1529 w1548 w1586 w1588 w1602 w1608] -> w1510
      tunnel: w1518 -> [w1520 w1533 w1587 w1591 w1605 w1609]
      tunnel: [w1520 w1533 w1587 w1591 w1605 w1609] -> w1517
      tunnel: [_ _ _ _ TRUE _] -> w1516
      tunnel: w1513 -> [_ _ _ _ _ _]
      tunnel: w1508 -> [_ _ _ _ w1599 _]
      frame "init" {
        # "Initialize - All initialization work should take place in this message, since other loops can potentially enqueue messages that execute immediately after this one."
        n988 = call "HEAVE WRITE FGV.vi"("Enum - Menu"=Heave_Write_enum."INIT", "error in (no error)"=w1528, "main ref"=w1520) -> ("error out"=w1527:errorcluster)  [unwired: 8 in]
        n989 = call <vilib>:"Clear Errors.vi"("error in (no error)"=w1527) -> ("error out"=w1522:errorcluster)  [unwired: 5 in, 1 out]
        n990 = call "Stall Data Flow.vim"("value in"=w1522, "milliseconds to wait"=u32 1000) -> ("value out"=w1525:errorcluster)  [unwired: 1 out]
        n991 = call "Heave Init.vi"("error in (no error)"=w1525, "main ref"=w1520) -> ("error out"=w1523:errorcluster)  [unwired: 9 in]
        n992 = call "HEAVE READ FGV.vi"("Enum - Menu"=Heave_Right_enum."INIT", "error in (no error)"=w1523, "main ref"=w1520) -> ("error out"=w1521:errorcluster)  [unwired: 6 in, 2 out]
        n993 = call <vilib>:"Clear Errors.vi"("error in (no error)"=w1521) -> ("error out"=w1530:errorcluster)  [unwired: 5 in, 1 out]
        n994 = call-poly "Enqueue Message.vi"("error in (no error)"=w1530, "Message"="Heave Main", "Message Queue"=w1531) -> ("error out"=w1529:errorcluster)  [unwired: 7 in, 1 out]
      }
      frame "Heave Main" {
        n995 = Unbundle By Name(w1533) -> ("Heave AND Surge.Read Heave Temp"=w1541:refnum<vi>)
        n996 = property on="Property Node" class="Bool (strict)"(reference=w1541) -> (reference out=w1539:refnum<vi>, error out=w1540:errorcluster, "Value"=w1538:bool)  [unwired: 1 in]
        n997 = Close Reference(reference=w1539, error in (no error)=w1540) -> ()  [unwired: 1 out]
        n998 = case shown="True" w1538 {
          tunnel: w1545 -> [w1571 w1576]
          tunnel: [w1571 w1575] -> w1536
          tunnel: w1533 -> [_ w1574]
          tunnel: [FALSE ("x < y?") w1573] -> w1534
          frame False {
          }
          frame True {
            n999 = call "HEAVE READ FGV.vi"("Enum - Menu"=Heave_Right_enum."READ", "error in (no error)"=w1576, "main ref"=w1574) -> ("error out"=w1575:errorcluster, "x < y?"=w1573:bool)  [unwired: 6 in, 1 out]
          }
        }
        n1000 = case shown="True" w1534 {
          tunnel: w1533 -> [w1551 w1558]
          frame False {
            w1549 = TRUE ("PAUSE")
            w1550 = FALSE ("Value")
            n1001 = Unbundle By Name(w1551) -> ("Platform Settings.Heave COM Status"=w1557:refnum<vi>)
            n1002 = Unbundle By Name(w1551) -> ("Main Screen.Heave COM Status"=w1552:refnum<vi>)
            n1003 = property on="Property Node" class="Bool (strict)"(reference=w1557, "Value"=w1550) -> (reference out=w1555:refnum<vi>, error out=w1556:errorcluster)  [unwired: 1 in]
            n1004 = property on="Property Node" class="Bool (strict)"(reference=w1552, "Value"=w1550) -> (reference out=w1554:refnum<vi>, error out=w1553:errorcluster)  [unwired: 1 in]
            n1005 = Close Reference(reference=w1555, error in (no error)=w1556) -> ()  [unwired: 1 out]
            n1006 = Close Reference(reference=w1554, error in (no error)=w1553) -> ()  [unwired: 1 out]
            n1007 = call "ELAPSED TIMER VI FOR Sway Loop Connection.vi"("RESET"=w1549, "PAUSE"=w1549) -> ()  [unwired: 7 in, 3 out]
          }
          frame True {
            w1561 = FALSE ("PAUSE")
            n1008 = call "ELAPSED TIMER VI FOR Sway Loop Connection.vi"("TARGET"=2.0, "RESET"=w1561, "PAUSE"=w1561) -> ("ELAPSED INDICATION"=w1559:bool)  [unwired: 6 in, 2 out]
            n1009 = case shown="True" w1559 {
              tunnel: w1558 -> [_ w1562]
              frame False {
              }
              frame True {
                w1563 = TRUE ("Value")
                n1010 = Unbundle By Name(w1562) -> ("Main Screen.Heave COM Status"=w1564:refnum<vi>)
                n1011 = Unbundle By Name(w1562) -> ("Platform Settings.Heave COM Status"=w1569:refnum<vi>)
                n1012 = property on="Property Node" class="Bool (strict)"(reference=w1564, "Value"=w1563) -> (reference out=w1566:refnum<vi>, error out=w1565:errorcluster)  [unwired: 1 in]
                n1013 = property on="Property Node" class="Bool (strict)"(reference=w1569, "Value"=w1563) -> (reference out=w1567:refnum<vi>, error out=w1568:errorcluster)  [unwired: 1 in]
                n1014 = Close Reference(reference=w1566, error in (no error)=w1565) -> ()  [unwired: 1 out]
                n1015 = Close Reference(reference=w1567, error in (no error)=w1568) -> ()  [unwired: 1 out]
              }
            }
          }
        }
        n1016 = call "Heave Reinitial.vi"("error in (no error)"=w1536, "Data Cluster"=w1533) -> ("error out"=w1535:errorcluster)  [unwired: 9 in]
        n1017 = Unbundle By Name(w1533) -> ("Main Home Screen.EXIT"=w1546:refnum<vi>)
        n1018 = property on="Property Node" class="Bool (strict)"(reference=w1546) -> (reference out=w1543:refnum<vi>, error out=w1544:errorcluster, "Value"=w1542:bool)  [unwired: 1 in]
        n1019 = call <vilib>:"Clear Errors.vi"("error in (no error)"=w1535) -> ("error out"=w1537:errorcluster)  [unwired: 5 in, 1 out]
        n1020 = Close Reference(reference=w1543, error in (no error)=w1544) -> ()  [unwired: 1 out]
        n1021 = case shown="False" w1542 {
          tunnel: [w1579 w1583] -> w1548
          tunnel: w1547 -> [w1578 w1582]
          tunnel: w1537 -> [w1577 w1581]
          frame True {
            n1022 = call-poly "Enqueue Message.vi"("error in (no error)"=w1577, "Message"="Confirm Quit", "Message Queue"=w1578) -> ("error out"=w1579:errorcluster)  [unwired: 7 in, 1 out]
          }
          frame False {
            n1023 = call-poly "Enqueue Message.vi"("error in (no error)"=w1581, "Message"="Heave Main", "Message Queue"=w1582) -> ("error out"=w1583:errorcluster)  [unwired: 7 in, 1 out]
          }
        }
      }
      frame "Error" {
        # "#CodeRecommended - If you ever change the name of this \"Error\" message, you'll need to update the name in the Check Loop Error.vi as well."
        # "#CodeRecommended - Consider creating a system for logging errors in some way. These errors are for notification purposes only. Handling of specific errors should be performed in the message frames that generated the error."
        # "Error - Display an error dialog. This message is sent by the \"Error Handler\" VIs at the end of other loops in this application."
        n1024 = Merge Errors(w1585) -> (w1586:errorcluster)
      }
      frame "Confirm Quit" {
        # "#CodeNeeded - If you want to provide an \"Are you sure\" dialog (or some other notification) before the application exits, place that code here. This message is typically sent from a Panel Close? event."
        # "Confirm Quit - Message that can confirm whether or not the user wants to exit the application."
        n1025 = call-poly "Enqueue Message.vi"("Priority Message? (F)"=TRUE, "error in (no error)"=w1598, "Message"="Exit", "Message Queue"=w1595) -> ("error out"=w1596:errorcluster)  [unwired: 6 in, 1 out]
        n1026 = Merge Errors(w1596) -> (w1597:errorcluster)
        n1027 = call <vilib>:"Clear Errors.vi"("error in (no error)"=w1597) -> ("error out"=w1589:errorcluster)  [unwired: 5 in, 1 out]
        n1028 = call "HEAVE WRITE FGV.vi"("Enum - Menu"=Heave_Write_enum."CLOSE", "error in (no error)"=w1589, "main ref"=w1591) -> ("error out"=w1592:errorcluster)  [unwired: 8 in]
        n1029 = call <vilib>:"Clear Errors.vi"("error in (no error)"=w1592) -> ("error out"=w1588:errorcluster)  [unwired: 5 in, 1 out]
      }
      frame "Exit" {
        # "Stop the VI"
        # "Release the message queue reference"
        # "#CodeNeeded - Add any required cleanup code here. Note that if 'Exit' was called as a result of an error, an error dialog will be displayed. Add any custom error handling for an 'Exit' condition here as well."
        # "Exit - Exit the application."
        n1030 = call "Fire User Event - Stop.vi"("User Event - Stop"=w1599) -> ("error out"=w1601:errorcluster)  [unwired: 10 in]
        n1031 = Release Queue(queue=w1606, error in (no error)=w1600) -> (error out=w1603:errorcluster)  [unwired: 1 in, 2 out]
        n1032 = Merge Errors(w1601, w1603) -> (w1602:errorcluster)
      }
      frame Default {
        # "'Default' case only runs if there is a message that isn't defined in any of the other cases.  Output a programming error."
        n1033 = xnode ("Error Ring")("parameter 0"=w1607) -> ("error out"=w1608:errorcluster)
      }
    }
    n1034 = call "LAB-IQ Error Handler - Message Handling Loop.vi"("error in (no error)"=w1510, "Message Queue"=w1512) -> ("dup error in"=w1511:errorcluster)  [unwired: 8 in, 1 out]
  }
  n1035 = while {
    tunnel: w16 -> [w1617]
    shift-right: [w1627] -> _
    shift-left: w47 -> [w1628]
    tunnel: w48 -> [w1625]
    tunnel: w89 -> [w1624]
    tunnel: [w1619] -> w96
    stop <- w1626 stop-if-true
    # "Message Handling Loop"
    n1036 = call "Dequeue Message.vi"("error in (no error)"=w1624, "Message Queue"=w1617) -> ("error out"=w1623:errorcluster, "output data"=w1621:dbl[][], "Message"=w1622:string, "dup Message Queue"=w1620:refnum<queue>)  [unwired: 6 in]
    n1037 = case "Message Cases" shown="\"Timeout\"" w1622 {
      selector: w1622 -> [_ _ _ _ _ _ _ _ _ _ _ _ _ _ _ _ _ _ _ _ _ _ _ _ _ _ _ _ _ _ _ _ _ _ _ _ _ _ _ _ _ _ _ _ _ _ _ _ _ _ _ _ _ _ _ _ _ _ _ _ _ _ _ _ _ _ _ _ _ _ _ _ _ _ _ _ _ _ _ _ _ _ _ _ _ _ _ _ _ _ w3133]
      tunnel: w1620 -> [_ w1673 _ _ _ _ _ _ _ _ _ _ _ _ _ _ _ _ _ _ _ _ _ _ _ _ _ _ _ _ _ _ _ _ _ _ _ _ _ _ _ _ _ _ _ _ _ _ _ _ _ _ _ _ _ _ _ _ _ _ _ _ _ _ _ _ _ _ _ _ _ _ _ _ _ _ _ _ _ _ _ _ _ _ _ _ _ _ w3121 w3132 _]
      tunnel: w1623 -> [w1629 w1675 w1677 w1687 w1708 w1725 w1742 w1759 w1780 w1793 w1813 w1818 w1830 w1835 w1900 w1926 w1952 w1987 w2003 w2055 w2059 w2062 w2065 w2072 w2148 w2160 w2181 w2193 w2219 w2230 w2241 w2252 w2263 w2274 w2285 w2296 w2308 w2319 w2330 w2341 w2350 w2361 w2371 w2382 w2389 w2419 w2443 w2479 w2515 w2523 w2526 w2534 w2546 w2555 w2575 w2595 w2610 w2624 w2634 w2644 w2646 w2661 w2674 w2691 w2708 w2732 w2740 w2799 w2823 w2833 w2874 w2917 w2960 w2996 w3003 w3022 w3028 w3036 w3048 w3059 w3068 w3072 w3076 w3080 w3084 w3098 w3107 w3115 w3124 w3125 _]
      tunnel: [w1631 w1646 w1679 w1688 w1703 w1720 w1737 w1754 w1775 w1785 w1801 w1816 w1828 w1839 w1896 w1922 w1948 w1988 w2004 w2019 w2058 w2061 w2064 w2071 w2142 w2159 w2182 w2205 w2221 w2232 w2243 w2254 w2265 w2276 w2287 w2298 w2309 w2320 w2331 w2342 w2352 w2362 w2372 w2383 w2388 w2418 w2448 w2484 w2496 w2522 w2525 w2533 w2540 w2550 w2570 w2588 w2607 w2623 w2634 w2644 w2652 w2660 w2673 w2690 w2707 w2731 w2739 w2799 w2823 w2830 w2871 w2914 w2957 w2997 w3003 w3016 w3026 w3035 w3055 w3062 w3066 w3071 w3075 w3079 w3083 w3097 w3106 w3116 w3123 w3128 w3134] -> w1618
      tunnel: w1628 -> [w1630 w1633 w1678 w1686 w1694 w1711 w1728 w1745 w1763 w1783 w1803 w1815 w1823 w1834 w1898 w1924 w1950 w1975 w1990 w2006 w2057 w2060 w2063 w2066 w2141 w2158 w2171 w2189 w2217 w2228 w2239 w2250 w2261 w2272 w2283 w2294 w2306 w2317 w2328 w2339 w2349 w2360 w2370 w2381 w2387 w2417 w2439 w2477 w2491 w2521 w2524 w2528 w2539 w2548 w2568 w2590 w2608 w2622 w2626 w2636 w2645 w2659 w2663 w2676 w2694 w2710 w2734 w2791 w2814 w2826 w2867 w2910 w2953 w2995 w2998 w3015 w3025 w3030 w3053 w3060 w3065 w3070 w3074 w3078 w3082 w3089 w3101 w3117 w3118 w3131 w3135]
      tunnel: [w1630 w1633 w1678 w1686 w1694 w1711 w1728 w1745 w1763 w1783 w1803 w1815 w1823 w1834 w1898 w1924 w1950 w1975 w1990 w2006 w2057 w2060 w2063 w2066 w2141 w2158 w2171 w2189 w2217 w2228 w2239 w2250 w2261 w2272 w2283 w2294 w2306 w2317 w2328 w2339 w2349 w2360 w2370 w2381 w2387 w2417 w2439 w2477 w2491 w2521 w2524 w2528 w2539 w2548 w2568 w2590 w2608 w2622 w2626 w2636 w2645 w2659 w2663 w2676 w2694 w2710 w2734 w2791 w2814 w2826 w2867 w2910 w2953 w2995 w2998 w3015 w3025 w3030 w3053 w3060 w3065 w3070 w3074 w3078 w3082 w3089 w3101 w3117 w3118 w3131 w3135] -> w1627
      tunnel: [_ _ _ _ _ _ _ _ _ _ _ _ _ _ _ _ _ _ _ _ _ _ _ _ _ _ _ _ _ _ _ _ _ _ _ _ _ _ _ _ _ _ _ _ _ _ _ _ _ _ _ _ _ _ _ _ _ _ _ _ _ _ _ _ _ _ _ _ _ _ _ _ _ _ _ _ _ _ _ _ _ _ _ _ _ _ _ _ _ TRUE _] -> w1626
      tunnel: w1621 -> [_ _ _ _ _ _ _ _ _ _ _ _ _ _ _ _ _ _ _ _ _ _ _ _ _ _ _ _ _ _ _ _ _ _ _ _ _ _ _ _ _ _ _ _ _ _ _ _ _ _ _ _ _ _ _ _ _ _ _ _ _ _ _ _ _ _ _ _ _ _ _ _ _ _ _ _ _ _ _ _ _ _ _ _ _ _ _ _ _ _ _]
      tunnel: w1625 -> [_ _ _ _ _ _ _ _ _ _ _ _ _ _ _ _ _ _ _ _ _ _ _ _ _ _ _ _ _ _ _ _ _ _ _ _ _ _ _ _ _ _ _ _ _ _ _ _ _ _ _ _ _ _ _ _ _ _ _ _ _ _ _ _ _ _ _ _ _ _ _ _ _ _ _ _ _ _ _ _ _ _ _ _ _ _ _ _ _ w3127 _]
      frame "Timeout" {
        n1038 = call "Time Out Loop.vi"("error in (no error)"=w1629, "Data Cluster"=w1630) -> ("error out"=w1631:errorcluster)  [unwired: 9 in]
        n1039 = call "Trip Log and Trip Monitor.vi"("error in (no error)"=w1629, "main ref"=w1630) -> ()  [unwired: 9 in, 1 out]
      }
      frame "init" {
        (unwired) FALSE ("Value")
        # "Initialize - All initialization work should take place in this message, since other loops can potentially enqueue messages that execute immediately after this one."
        n1040 = Unbundle By Name(w1633) -> ("Loading.Warning"=w1636:refnum<vi>)
        n1041 = property class="TabCtl (strict)"(reference=w1636, "Visible"=FALSE) -> (reference out=w1634:refnum<vi>, error out=w1635:errorcluster)  [unwired: 1 in]
        n1042 = call-poly "Enqueue Message.vi"("error in (no error)"=w1675, "Message"="Init Other Loop", "Message Queue"=w1673) -> ("error out"=w1676:errorcluster)  [unwired: 7 in, 1 out]
        n1043 = Close Reference(reference=w1634, error in (no error)=w1635) -> ()  [unwired: 1 out]
        n1044 = Unbundle By Name(w1633) -> ("Loading.SSP 0.3"=w1665:refnum<vi>)
        n1045 = Unbundle By Name(w1633) -> ("Loading.SSP 0.5"=w1662:refnum<vi>)
        n1046 = Unbundle By Name(w1633) -> ("Loading.SSP 0.75"=w1657:refnum<vi>)
        n1047 = Unbundle By Name(w1633) -> ("Loading.Communication is established"=w1652:refnum<vi>)
        n1048 = Unbundle By Name(w1633) -> ("Motion Module.Set WTD"=w1645:refnum<vi>)
        n1049 = call "Read Config Unitest.vi"("error in (no error)"=w1676, "main ref"=w1633) -> ("error out"=w1671:errorcluster)  [unwired: 9 in]
        n1050 = Unbundle By Name(w1633) -> ("Motion Module.Wear Track Diameter"=w1639:refnum<vi>)
        n1051 = Unbundle By Name(w1633) -> ("PID.Ramp"=w1649:refnum<vi>)
        n1052 = call "Encrypt file path creation.vi"("error in (no error)"=w1671) -> ("error out"=w1670:errorcluster, "File Path"=w1669:path)  [unwired: 9 in]
        n1053 = property on="Property Node" class="Bool (strict)"(reference=w1662, "Visible"=FALSE) -> (reference out=w1660:refnum<vi>, error out=w1661:errorcluster)  [unwired: 1 in]
        n1054 = property on="Property Node" class="Bool (strict)"(reference=w1665, "Visible"=FALSE) -> (reference out=w1667:refnum<vi>, error out=w1666:errorcluster)  [unwired: 1 in]
        n1055 = property on="Property Node" class="Bool (strict)"(reference=w1657, "Visible"=FALSE) -> (reference out=w1659:refnum<vi>, error out=w1658:errorcluster)  [unwired: 1 in]
        n1056 = property on="Property Node" class="Bool (strict)"(reference=w1649, "Value"=FALSE) -> (reference out=w1651:refnum<vi>, error out=w1650:errorcluster)  [unwired: 1 in]
        n1057 = property on="Property Node" class="DigNum (strict)"(reference=w1639, "Value"=0.0) -> (reference out=w1638:refnum<vi>, error out=w1640:errorcluster)  [unwired: 1 in]
        n1058 = property on="Property Node" class="Bool (strict)"(reference=w1645, "Visible"=FALSE, "DisabledEnum"=T26."Disabled and Grayed Out" ("Disabled")) -> (reference out=w1642:refnum<vi>, error out=w1644:errorcluster)  [unwired: 1 in]
        n1059 = property on="Property Node" class="Bool (strict)"(reference=w1652, "Visible"=FALSE ("Value")) -> (reference out=w1654:refnum<vi>, error out=w1653:errorcluster)  [unwired: 1 in]
        n1060 = call "DATA ENCRYPT STRING FILE WRITE.vi"("file path (dialog if empty)"=w1669, "error in (no error)"=w1670, "User Action"="System Booted", "main ref"=w1633) -> ("error out"=w1672:errorcluster)  [unwired: 5 in, 1 out]
        n1061 = Close Reference(reference=w1660, error in (no error)=w1661) -> ()  [unwired: 1 out]
        n1062 = Close Reference(reference=w1667, error in (no error)=w1666) -> ()  [unwired: 1 out]
        n1063 = Close Reference(reference=w1659, error in (no error)=w1658) -> ()  [unwired: 1 out]
        n1064 = Close Reference(reference=w1651, error in (no error)=w1650) -> ()  [unwired: 1 out]
        n1065 = Close Reference(reference=w1638, error in (no error)=w1640) -> ()  [unwired: 1 out]
        n1066 = Close Reference(reference=w1642, error in (no error)=w1644) -> ()  [unwired: 1 out]
        n1067 = Close Reference(reference=w1654, error in (no error)=w1653) -> ()  [unwired: 1 out]
        n1068 = call "Reinitial Parameter After Test.vi"("error in (no error)"=w1672, "main ref"=w1633) -> ("error out"=w1646:errorcluster)  [unwired: 9 in]
        n1069 = local write "HEAVE ENABLE"(FALSE ("HEAVE ENABLE")) -> ()
      }
      frame "Init Other Loop" {
        n1070 = disable-structure shown="Disabled" {
          disable-tunnel: [w1682 w1683] -> w1679
          disable-tunnel: w1678 -> [w1681 _]
          disable-tunnel: w1677 -> [w1680 w1683]
          frame Disabled {
            n1071 = call "SET LOAD PARAMETERS.vi"("error in (no error)"=w1680, "main ref"=w1681) -> ("error out"=w1682:errorcluster)  [unwired: 9 in]
          }
          frame Enabled {
          }
        }
      }
      frame "Service Save" {
        n1072 = call "Write Config Unitest.vi"("error in (no error)"=w1687, "main ref"=w1686) -> ("error out"=w1692:errorcluster)  [unwired: 9 in]
        n1073 = call "Stall Data Flow.vim"("value in"=w1692, "milliseconds to wait"=u32 2000) -> ("value out"=w1691:errorcluster)  [unwired: 1 out]
        n1074 = call "Read Config Unitest.vi"("error in (no error)"=w1691, "main ref"=w1686) -> ("error out"=w1689:errorcluster)  [unwired: 9 in]
        n1075 = local write "SAVE  2"(FALSE ("SAVE  2")) -> ()
        n1076 = call "DATA ENCRYPT STRING FILE WRITE.vi"("error in (no error)"=w1689, "User Action"="Service Parameter Saved", "main ref"=w1686) -> ("error out"=w1688:errorcluster)  [unwired: 6 in, 1 out]
      }
      frame "HOME" {
        n1077 = call "DATA ENCRYPT STRING FILE WRITE.vi"("error in (no error)"=w1708, "User Action"="User Pressed Home", "main ref"=w1694) -> ("error out"=w1704:errorcluster)  [unwired: 6 in, 1 out]
        n1078 = Unbundle By Name(w1694) -> ("Main Home Screen.MainPage"=w1699:refnum<vi>)
        n1079 = Unbundle By Name(w1694) -> ("Main Home Screen.Home"=w1707:refnum<vi>)
        n1080 = Unbundle By Name(w1694) -> ("Main Home Screen.GUI"=w1697:refnum<vi>)
        n1081 = property on="Property Node" class="Bool (strict)"(reference=w1707, error in=w1704, "Value"=FALSE) -> (reference out=w1705:refnum<vi>, error out=w1706:errorcluster)
        n1082 = property on="Property Node" class="TabCtl (strict)"(reference=w1699, "Value"=T15."HOME") -> (reference out=w1701:refnum<vi>, error out=w1700:errorcluster)  [unwired: 1 in]
        n1083 = property on="Property Node" class="TabCtl (strict)"(reference=w1697, "Value"=T14."Setup") -> (reference out=w1695:refnum<vi>, error out=w1696:errorcluster)  [unwired: 1 in]
        n1084 = Close Reference(reference=w1705, error in (no error)=w1706) -> (error out=w1703:errorcluster)
        n1085 = Close Reference(reference=w1701, error in (no error)=w1700) -> ()  [unwired: 1 out]
        n1086 = Close Reference(reference=w1695, error in (no error)=w1696) -> ()  [unwired: 1 out]
      }
      frame "Platform Setting" {
        n1087 = call "DATA ENCRYPT STRING FILE WRITE.vi"("error in (no error)"=w1725, "User Action"="User Pressed Platform Setting", "main ref"=w1711) -> ("error out"=w1721:errorcluster)  [unwired: 6 in, 1 out]
        n1088 = Unbundle By Name(w1711) -> ("Main Home Screen.Platform Settings"=w1724:refnum<vi>)
        n1089 = Unbundle By Name(w1711) -> ("Main Home Screen.MainPage"=w1716:refnum<vi>)
        n1090 = Unbundle By Name(w1711) -> ("Main Home Screen.GUI"=w1714:refnum<vi>)
        n1091 = property on="Property Node" class="TabCtl (strict)"(reference=w1716, "Value"=T15."PlatformSetting") -> (reference out=w1718:refnum<vi>, error out=w1717:errorcluster)  [unwired: 1 in]
        n1092 = property on="Property Node" class="TabCtl (strict)"(reference=w1714, "Value"=T14."Setup") -> (reference out=w1712:refnum<vi>, error out=w1713:errorcluster)  [unwired: 1 in]
        n1093 = property on="Property Node" class="Bool (strict)"(reference=w1724, error in=w1721, "Value"=FALSE) -> (reference out=w1722:refnum<vi>, error out=w1723:errorcluster)
        n1094 = Close Reference(reference=w1718, error in (no error)=w1717) -> ()  [unwired: 1 out]
        n1095 = Close Reference(reference=w1712, error in (no error)=w1713) -> ()  [unwired: 1 out]
        n1096 = Close Reference(reference=w1722, error in (no error)=w1723) -> (error out=w1720:errorcluster)
      }
      frame "Configure" {
        n1097 = call "DATA ENCRYPT STRING FILE WRITE.vi"("error in (no error)"=w1742, "User Action"="User Pressed Configure", "main ref"=w1728) -> ("error out"=w1738:errorcluster)  [unwired: 6 in, 1 out]
        n1098 = Unbundle By Name(w1728) -> ("Main Home Screen.Configure"=w1741:refnum<vi>)
        n1099 = Unbundle By Name(w1728) -> ("Main Home Screen.MainPage"=w1733:refnum<vi>)
        n1100 = Unbundle By Name(w1728) -> ("Main Home Screen.GUI"=w1731:refnum<vi>)
        n1101 = property on="Property Node" class="Bool (strict)"(reference=w1741, error in=w1738, "Value"=FALSE) -> (reference out=w1739:refnum<vi>, error out=w1740:errorcluster)
        n1102 = property on="Property Node" class="TabCtl (strict)"(reference=w1733, "Value"=T15."Details") -> (reference out=w1735:refnum<vi>, error out=w1734:errorcluster)  [unwired: 1 in]
        n1103 = property on="Property Node" class="TabCtl (strict)"(reference=w1731, "Value"=T14."Setup") -> (reference out=w1729:refnum<vi>, error out=w1730:errorcluster)  [unwired: 1 in]
        n1104 = Close Reference(reference=w1739, error in (no error)=w1740) -> (error out=w1737:errorcluster)
        n1105 = Close Reference(reference=w1735, error in (no error)=w1734) -> ()  [unwired: 1 out]
        n1106 = Close Reference(reference=w1729, error in (no error)=w1730) -> ()  [unwired: 1 out]
      }
      frame "Analysis" {
        n1107 = call "DATA ENCRYPT STRING FILE WRITE.vi"("error in (no error)"=w1759, "User Action"="User Pressed Analysis", "main ref"=w1745) -> ("error out"=w1755:errorcluster)  [unwired: 6 in, 1 out]
        n1108 = Unbundle By Name(w1745) -> ("Main Home Screen.MainPage"=w1750:refnum<vi>)
        n1109 = Unbundle By Name(w1745) -> ("Main Home Screen.Analysis"=w1758:refnum<vi>)
        n1110 = Unbundle By Name(w1745) -> ("Main Home Screen.GUI"=w1748:refnum<vi>)
        n1111 = property on="Property Node" class="Bool (strict)"(reference=w1758, error in=w1755, "Value"=FALSE) -> (reference out=w1756:refnum<vi>, error out=w1757:errorcluster)
        n1112 = property on="Property Node" class="TabCtl (strict)"(reference=w1750, "Value"=T15."Analysis") -> (reference out=w1752:refnum<vi>, error out=w1751:errorcluster)  [unwired: 1 in]
        n1113 = property on="Property Node" class="TabCtl (strict)"(reference=w1748, "Value"=T14."Setup") -> (reference out=w1746:refnum<vi>, error out=w1747:errorcluster)  [unwired: 1 in]
        n1114 = Close Reference(reference=w1756, error in (no error)=w1757) -> (error out=w1754:errorcluster)
        n1115 = Close Reference(reference=w1752, error in (no error)=w1751) -> ()  [unwired: 1 out]
        n1116 = Close Reference(reference=w1746, error in (no error)=w1747) -> ()  [unwired: 1 out]
      }
      frame "service 2" {
        n1117 = call "DATA ENCRYPT STRING FILE WRITE.vi"("error in (no error)"=w1780, "User Action"="User Pressed service", "main ref"=w1763) -> ("error out"=w1776:errorcluster)  [unwired: 6 in, 1 out]
        n1118 = Unbundle By Name(w1763) -> ("Main Screen.Main Screen Tab"=w1764:refnum<vi>)
        n1119 = Unbundle By Name(w1763) -> ("Main Home Screen.MainPage"=w1771:refnum<vi>)
        n1120 = Unbundle By Name(w1763) -> ("Main Home Screen.service 2"=w1779:refnum<vi>)
        n1121 = Unbundle By Name(w1763) -> ("Main Home Screen.GUI"=w1769:refnum<vi>)
        n1122 = property on="Property Node" class="Bool (strict)"(reference=w1779, error in=w1776, "Value"=FALSE) -> (reference out=w1777:refnum<vi>, error out=w1778:errorcluster)
        n1123 = property on="Property Node" class="TabCtl (strict)"(reference=w1771, "Value"=T15."HOME") -> (reference out=w1773:refnum<vi>, error out=w1772:errorcluster)  [unwired: 1 in]
        n1124 = property on="Property Node" class="TabCtl (strict)"(reference=w1769, "Value"=T14."Begin") -> (reference out=w1767:refnum<vi>, error out=w1768:errorcluster)  [unwired: 1 in]
        n1125 = property on="Property Node" class="TabCtl (strict)"(reference=w1764, "Value"=T18."About") -> (reference out=w1761:refnum<vi>, error out=w1765:errorcluster)  [unwired: 1 in]
        n1126 = Close Reference(reference=w1777, error in (no error)=w1778) -> (error out=w1775:errorcluster)
        n1127 = Close Reference(reference=w1773, error in (no error)=w1772) -> ()  [unwired: 1 out]
        n1128 = Close Reference(reference=w1767, error in (no error)=w1768) -> ()  [unwired: 1 out]
        n1129 = Close Reference(reference=w1761, error in (no error)=w1765) -> ()  [unwired: 1 out]
      }
      frame "Auto" {
        # "%I_%M_%S_%p_%B_%d_%Y"
        n1130 = call "DATA ENCRYPT STRING FILE WRITE.vi"("error in (no error)"=w1793, "User Action"="User Pressed Auto File Name", "main ref"=w1783) -> ("error out"=w1790:errorcluster)  [unwired: 6 in, 1 out]
        n1131 = Get Date/Time In Seconds() -> (seconds since 1Jan1904=w1791:timestamp)
        n1132 = Format Into String(format string="%<%I_%M_%S_%p_%B_%d_%Y>T", error in=w1790, w1791) -> (resulting string=w1784:string, error out=w1786:errorcluster)  [unwired: 1 in]
        n1133 = local write "Auto"(FALSE ("Auto")) -> ()
        n1134 = Unbundle By Name(w1783) -> ("Config Screen.FILE"=w1789:refnum<vi>)
        n1135 = property on="Property Node" class="Str"(reference=w1789, error in=w1786, "Value"=w1784) -> (reference out=w1787:refnum<vi>, error out=w1788:errorcluster)
        n1136 = Close Reference(reference=w1787, error in (no error)=w1788) -> (error out=w1785:errorcluster)
      }
      frame "Select Load Head" {
        n1137 = call "Reinitial Parameter.vi"("error in (no error)"=w1813, "Data Cluster"=w1803) -> ("error out"=w1812:errorcluster)  [unwired: 9 in]
        n1138 = call "FILE NAME RECHECK.vi"("error in (no error)"=w1812, "main ref"=w1803) -> ("error out"=w1802:errorcluster, "FILE OUT"=w1795:path)  [unwired: 8 in]
        n1139 = Strip Path(path=w1795) -> (name=w1809:string)  [unwired: 1 out]
        n1140 = Build Path(base path=w1795, name or relative path=w1809) -> (appended path=w1810:path)
        n1141 = Path To String(path=w1810) -> (string=w1807:string)
        n1142 = Concatenate Strings(w1807, ".tdms" ("string")) -> (w1808:string)
        n1143 = String To Path(string=w1808) -> (path=w1800:path)
        n1144 = call <vilib>:"Create File with Incrementing Suffix.vi"("file path"=w1800) -> ("error out"=w1797:errorcluster, "refnum out"=w1799:refnum<file>)  [unwired: 8 in, 1 out]
        n1145 = Close File(refnum=w1799, error in=w1797) -> (path=w1798:path, error out=→"error out 3":errorcluster)
        n1146 = TDMS Open(6:FALSE ("disable buffering (T)"), 8:w1802, 10:T27."create or replace" ("operation"), 11:w1798) -> (0:w1801:errorcluster, 3:→"tdms file out":refnum<k34>)  [unwired: 3 in]
      }
      frame "com 3" {
        n1147 = call "DATA ENCRYPT STRING FILE WRITE.vi"("error in (no error)"=w1818, "User Action"="User Pressed Check Load Communication", "main ref"=w1815) -> ("error out"=w1817:errorcluster)  [unwired: 6 in, 1 out]
        n1148 = call "SET LOAD PARAMETERS.vi"("error in (no error)"=w1817, "main ref"=w1815) -> ("error out"=w1816:errorcluster)  [unwired: 9 in]
        n1149 = local write "com 3"(FALSE ("com 3")) -> ()
      }
      frame "ZeroAll" {
        n1150 = call "DATA ENCRYPT STRING FILE WRITE.vi"("error in (no error)"=w1830, "User Action"="User Pressed Zero All", "main ref"=w1823) -> ("error out"=w1829:errorcluster)  [unwired: 6 in, 1 out]
        n1151 = call "NEW Load Cell FGV.vi"("Enum - Menu"=Load_cell_Enum."Set Zero", "error in (no error)"=w1829, "main ref"=w1823) -> ("error out"=w1828:errorcluster)  [unwired: 6 in, 2 out]
        n1152 = Unbundle By Name(w1823) -> ("Loading Com Port.Load Cell Link"=w1826:refnum<vi>)
        n1153 = Bundle By Name(cluster=T5 {"model"="", "SN"=0, "Sensor IP"="", "Port"=0, "Acq Delay (ms)"=0.0, "Burst Delay (ms)"=0.0, "Save Dwell"=0.0, "FORCE (N)"=[], "TORQUE (N-m)"=[], "ft_data"=[], "running_flag"=FALSE, "ClearAll"=FALSE, "ZeroAll"=FALSE} ("Value"), "ZeroAll"=FALSE) -> (w1821:T5)
        n1154 = property on="Property Node" class="Clust (strict)"(reference=w1826, "Value"=w1821) -> (reference out=w1824:refnum<vi>, error out=w1825:errorcluster)  [unwired: 1 in]
        n1155 = Close Reference(reference=w1824, error in (no error)=w1825) -> ()  [unwired: 1 out]
      }
      frame "Loading Mode" {
        n1156 = Unbundle By Name(w1834) -> ("Loading.Loading Mode"=w1836:refnum<vi>)
        n1157 = property on="Property Node" class="Ring (strict)"(reference=w1836, error in=w1835) -> (reference out=w1838:refnum<vi>, error out=w1837:errorcluster, "Value"=w1832:u16)
        n1158 = Close Reference(reference=w1838, error in (no error)=w1837) -> (error out=w1833:errorcluster)
        n1159 = case shown="1" w1832 {
          tunnel: [w1853 w1870 w1882 w1894] -> w1839
          tunnel: w1834 -> [w1840 w1856 w1874 w1886]
          tunnel: w1833 -> [w1854 w1869 w1881 w1893]
          frame 0, Default {
            n1160 = Unbundle By Name(w1840) -> ("Loading.Enter the Loading Rate (N/min)"=w1847:refnum<vi>)
            n1161 = Unbundle By Name(w1840) -> ("Loading.Load Selection"=w1850:refnum<vi>)
            n1162 = Unbundle By Name(w1840) -> ("Loading.Enter the Final Load (N)"=w1842:refnum<vi>)
            n1163 = property on="Property Node" class="TabCtl (strict)"(reference=w1850, "Value"=T16."Constant") -> (reference out=w1852:refnum<vi>, error out=w1851:errorcluster)  [unwired: 1 in]
            n1164 = property on="Property Node" class="DigNum (strict)"(reference=w1847, "DisabledEnum"=T26."Disabled and Grayed Out" ("Disabled")) -> (reference out=w1846:refnum<vi>, error out=w1848:errorcluster)  [unwired: 1 in]
            n1165 = property on="Property Node" class="DigNum (strict)"(reference=w1842, "DisabledEnum"=T26."Disabled and Grayed Out" ("Disabled")) -> (reference out=w1843:refnum<vi>, error out=w1841:errorcluster)  [unwired: 1 in]
            n1166 = call "DATA ENCRYPT STRING FILE WRITE.vi"("error in (no error)"=w1854, "User Action"="User selected Constant Mode", "main ref"=w1840) -> ("error out"=w1853:errorcluster)  [unwired: 6 in, 1 out]
            n1167 = Close Reference(reference=w1852, error in (no error)=w1851) -> ()  [unwired: 1 out]
            n1168 = Close Reference(reference=w1846, error in (no error)=w1848) -> ()  [unwired: 1 out]
            n1169 = Close Reference(reference=w1843, error in (no error)=w1841) -> ()  [unwired: 1 out]
          }
          frame 1 {
            n1170 = Unbundle By Name(w1856) -> ("Loading.Enter the Loading Rate (N/min)"=w1867:refnum<vi>)
            n1171 = Unbundle By Name(w1856) -> ("Loading.Enter the Final Load (N)"=w1862:refnum<vi>)
            n1172 = Unbundle By Name(w1856) -> ("Loading.Load Selection"=w1858:refnum<vi>)
            n1173 = property on="Property Node" class="TabCtl (strict)"(reference=w1858, "Value"=T16."Constant") -> (reference out=w1860:refnum<vi>, error out=w1859:errorcluster)  [unwired: 1 in]
            n1174 = property on="Property Node" class="DigNum (strict)"(reference=w1867, "DisabledEnum"=T26."Enabled" ("Disabled")) -> (reference out=w1866:refnum<vi>, error out=w1868:errorcluster)  [unwired: 1 in]
            n1175 = property on="Property Node" class="DigNum (strict)"(reference=w1862, "DisabledEnum"=T26."Enabled" ("Disabled")) -> (reference out=w1863:refnum<vi>, error out=w1861:errorcluster)  [unwired: 1 in]
            n1176 = call "DATA ENCRYPT STRING FILE WRITE.vi"("error in (no error)"=w1869, "User Action"="User selected Ramp Mode", "main ref"=w1856) -> ("error out"=w1870:errorcluster)  [unwired: 6 in, 1 out]
            n1177 = Close Reference(reference=w1860, error in (no error)=w1859) -> ()  [unwired: 1 out]
            n1178 = Close Reference(reference=w1866, error in (no error)=w1868) -> ()  [unwired: 1 out]
            n1179 = Close Reference(reference=w1863, error in (no error)=w1861) -> ()  [unwired: 1 out]
          }
          frame 2 {
            n1180 = Unbundle By Name(w1874) -> ("Loading.Load Selection"=w1878:refnum<vi>)
            n1181 = Unbundle By Name(w1874) -> ("Loading.Warning 2"=w1876:refnum<vi>)
            n1182 = property on="Property Node" class="TabCtl (strict)"(reference=w1878, "Value"=T16."Step") -> (reference out=w1880:refnum<vi>, error out=w1879:errorcluster)  [unwired: 1 in]
            n1183 = property on="Property Node" class="Bool (strict)"(reference=w1876, "Visible"=FALSE) -> (reference out=w1872:refnum<vi>, error out=w1875:errorcluster)  [unwired: 1 in]
            n1184 = call "DATA ENCRYPT STRING FILE WRITE.vi"("error in (no error)"=w1881, "User Action"="User selected Step Mode", "main ref"=w1874) -> ("error out"=w1882:errorcluster)  [unwired: 6 in, 1 out]
            n1185 = Close Reference(reference=w1880, error in (no error)=w1879) -> ()  [unwired: 1 out]
            n1186 = Close Reference(reference=w1872, error in (no error)=w1875) -> ()  [unwired: 1 out]
          }
          frame 3 {
            n1187 = Unbundle By Name(w1886) -> ("Loading.Load Selection"=w1890:refnum<vi>)
            n1188 = Unbundle By Name(w1886) -> ("Loading.Warning 2"=w1888:refnum<vi>)
            n1189 = property on="Property Node" class="TabCtl (strict)"(reference=w1890, "Value"=T16."Indentation") -> (reference out=w1892:refnum<vi>, error out=w1891:errorcluster)  [unwired: 1 in]
            n1190 = property on="Property Node" class="Bool (strict)"(reference=w1888, "Visible"=FALSE) -> (reference out=w1884:refnum<vi>, error out=w1887:errorcluster)  [unwired: 1 in]
            n1191 = call "DATA ENCRYPT STRING FILE WRITE.vi"("error in (no error)"=w1893, "User Action"="User selected Indentation Mode", "main ref"=w1886) -> ("error out"=w1894:errorcluster)  [unwired: 6 in, 1 out]
            n1192 = Close Reference(reference=w1892, error in (no error)=w1891) -> ()  [unwired: 1 out]
            n1193 = Close Reference(reference=w1884, error in (no error)=w1887) -> ()  [unwired: 1 out]
          }
        }
      }
      frame "SSP 0.3" {
        n1194 = Unbundle By Name(w1898) -> ("Loading.SSP 0.3"=w1901:refnum<vi>)
        n1195 = property on="Property Node" class="Bool (strict)"(reference=w1901, error in=w1900) -> (reference out=w1903:refnum<vi>, error out=w1902:errorcluster, "Value"=w1899:bool)
        n1196 = Close Reference(reference=w1903, error in (no error)=w1902) -> (error out=w1897:errorcluster)
        n1197 = case shown="True" w1899 {
          tunnel: w1898 -> [_ w1905]
          tunnel: w1897 -> [w1904 w1913]
          tunnel: [w1904 w1912] -> w1896
          frame False {
          }
          frame True {
            w1915 = FALSE ("Value")
            n1198 = Unbundle By Name(w1905) -> ("Loading.Enter the Load  (N)"=w1911:refnum<vi>)
            n1199 = Unbundle By Name(w1905) -> ("Loading.SSP 0.75"=w1916:refnum<vi>)
            n1200 = Unbundle By Name(w1905) -> ("Loading.SSP 0.5"=w1921:refnum<vi>)
            n1201 = property on="Property Node" class="Bool (strict)"(reference=w1916, "Value"=w1915) -> (reference out=w1918:refnum<vi>, error out=w1917:errorcluster)  [unwired: 1 in]
            n1202 = property on="Property Node" class="Bool (strict)"(reference=w1921, "Value"=w1915) -> (reference out=w1919:refnum<vi>, error out=w1920:errorcluster)  [unwired: 1 in]
            n1203 = property on="Property Node" class="DigNum (strict)"(reference=w1911, "Minimum"=2.0 ("Data Entry Limits:Minimum"), "Maximum"=50.0 ("Data Entry Limits:Maximum"), "Increment"=0.1 ("Data Entry Limits:Increment")) -> (reference out=w1909:refnum<vi>, error out=w1910:errorcluster)  [unwired: 1 in]
            n1204 = call "DATA ENCRYPT STRING FILE WRITE.vi"("error in (no error)"=w1913, "User Action"="User selected 0.3 SSP", "main ref"=w1905) -> ("error out"=w1912:errorcluster)  [unwired: 6 in, 1 out]
            n1205 = Close Reference(reference=w1918, error in (no error)=w1917) -> ()  [unwired: 1 out]
            n1206 = Close Reference(reference=w1919, error in (no error)=w1920) -> ()  [unwired: 1 out]
            n1207 = Close Reference(reference=w1909, error in (no error)=w1910) -> ()  [unwired: 1 out]
          }
        }
      }
      frame "SSP 0.5" {
        n1208 = Unbundle By Name(w1924) -> ("Loading.SSP 0.5"=w1927:refnum<vi>)
        n1209 = property on="Property Node" class="Bool (strict)"(reference=w1927, error in=w1926) -> (reference out=w1929:refnum<vi>, error out=w1928:errorcluster, "Value"=w1925:bool)
        n1210 = Close Reference(reference=w1929, error in (no error)=w1928) -> (error out=w1923:errorcluster)
        n1211 = case shown="True" w1925 {
          tunnel: w1924 -> [_ w1931]
          tunnel: w1923 -> [w1930 w1939]
          tunnel: [w1930 w1938] -> w1922
          frame False {
          }
          frame True {
            w1941 = FALSE ("Value")
            n1212 = Unbundle By Name(w1931) -> ("Loading.Enter the Load  (N)"=w1937:refnum<vi>)
            n1213 = Unbundle By Name(w1931) -> ("Loading.SSP 0.75"=w1947:refnum<vi>)
            n1214 = Unbundle By Name(w1931) -> ("Loading.SSP 0.3"=w1942:refnum<vi>)
            n1215 = property on="Property Node" class="Bool (strict)"(reference=w1942, "Value"=w1941) -> (reference out=w1944:refnum<vi>, error out=w1943:errorcluster)  [unwired: 1 in]
            n1216 = property on="Property Node" class="Bool (strict)"(reference=w1947, "Value"=w1941) -> (reference out=w1945:refnum<vi>, error out=w1946:errorcluster)  [unwired: 1 in]
            n1217 = property on="Property Node" class="DigNum (strict)"(reference=w1937, "Minimum"=2.0 ("Data Entry Limits:Minimum"), "Maximum"=200.0 ("Data Entry Limits:Maximum"), "Increment"=0.1 ("Data Entry Limits:Increment")) -> (reference out=w1935:refnum<vi>, error out=w1936:errorcluster)  [unwired: 1 in]
            n1218 = call "DATA ENCRYPT STRING FILE WRITE.vi"("error in (no error)"=w1939, "User Action"="User selected 0.5 SSP", "main ref"=w1931) -> ("error out"=w1938:errorcluster)  [unwired: 6 in, 1 out]
            n1219 = Close Reference(reference=w1944, error in (no error)=w1943) -> ()  [unwired: 1 out]
            n1220 = Close Reference(reference=w1945, error in (no error)=w1946) -> ()  [unwired: 1 out]
            n1221 = Close Reference(reference=w1935, error in (no error)=w1936) -> ()  [unwired: 1 out]
          }
        }
      }
      frame "SSP 0.75" {
        n1222 = Unbundle By Name(w1950) -> ("Loading.SSP 0.75"=w1953:refnum<vi>)
        n1223 = property on="Property Node" class="Bool (strict)"(reference=w1953, error in=w1952) -> (reference out=w1955:refnum<vi>, error out=w1954:errorcluster, "Value"=w1951:bool)
        n1224 = Close Reference(reference=w1955, error in (no error)=w1954) -> (error out=w1949:errorcluster)
        n1225 = case shown="True" w1951 {
          tunnel: w1950 -> [_ w1957]
          tunnel: w1949 -> [w1956 w1965]
          tunnel: [w1956 w1964] -> w1948
          frame False {
          }
          frame True {
            w1967 = FALSE ("Value")
            n1226 = Unbundle By Name(w1957) -> ("Loading.SSP 0.3"=w1968:refnum<vi>)
            n1227 = Unbundle By Name(w1957) -> ("Loading.SSP 0.5"=w1973:refnum<vi>)
            n1228 = Unbundle By Name(w1957) -> ("Loading.Enter the Load  (N)"=w1963:refnum<vi>)
            n1229 = property on="Property Node" class="Bool (strict)"(reference=w1968, "Value"=w1967) -> (reference out=w1970:refnum<vi>, error out=w1969:errorcluster)  [unwired: 1 in]
            n1230 = property on="Property Node" class="Bool (strict)"(reference=w1973, "Value"=w1967) -> (reference out=w1971:refnum<vi>, error out=w1972:errorcluster)  [unwired: 1 in]
            n1231 = property on="Property Node" class="DigNum (strict)"(reference=w1963, "Minimum"=200.0 ("Data Entry Limits:Minimum"), "Maximum"=500.0 ("Data Entry Limits:Maximum"), "Increment"=0.1 ("Data Entry Limits:Increment")) -> (reference out=w1961:refnum<vi>, error out=w1962:errorcluster)  [unwired: 1 in]
            n1232 = call "DATA ENCRYPT STRING FILE WRITE.vi"("error in (no error)"=w1965, "User Action"="User selected 0.75 SSP", "main ref"=w1957) -> ("error out"=w1964:errorcluster)  [unwired: 6 in, 1 out]
            n1233 = Close Reference(reference=w1970, error in (no error)=w1969) -> ()  [unwired: 1 out]
            n1234 = Close Reference(reference=w1971, error in (no error)=w1972) -> ()  [unwired: 1 out]
            n1235 = Close Reference(reference=w1961, error in (no error)=w1962) -> ()  [unwired: 1 out]
          }
        }
      }
      frame "LHBack" {
        # "Back to Configure"
        n1236 = Unbundle By Name(w1975) -> ("Main Home Screen.GUI"=w1984:refnum<vi>)
        n1237 = Unbundle By Name(w1975) -> ("Main Home Screen.MainPage"=w1980:refnum<vi>)
        n1238 = Unbundle By Name(w1975) -> ("Loading.LHBack"=w1978:refnum<vi>)
        n1239 = property on="Property Node" class="TabCtl (strict)"(reference=w1980, "Value"=T15."HOME") -> (reference out=w1982:refnum<vi>, error out=w1981:errorcluster)  [unwired: 1 in]
        n1240 = property on="Property Node" class="Bool (strict)"(reference=w1978, "Value"=FALSE) -> (reference out=w1976:refnum<vi>, error out=w1977:errorcluster)  [unwired: 1 in]
        n1241 = property on="Property Node" class="TabCtl (strict)"(reference=w1984, "Value"=T14."Setup") -> (reference out=w1986:refnum<vi>, error out=w1985:errorcluster)  [unwired: 1 in]
        n1242 = Close Reference(reference=w1982, error in (no error)=w1981) -> ()  [unwired: 1 out]
        n1243 = Close Reference(reference=w1976, error in (no error)=w1977) -> ()  [unwired: 1 out]
        n1244 = Close Reference(reference=w1986, error in (no error)=w1985) -> ()  [unwired: 1 out]
        n1245 = call "DATA ENCRYPT STRING FILE WRITE.vi"("error in (no error)"=w1987, "User Action"="User selected Back to Configure", "main ref"=w1975) -> ("error out"=w1988:errorcluster)  [unwired: 6 in, 1 out]
      }
      frame "MMBack" {
        # "Back to Configure"
        n1246 = Unbundle By Name(w1990) -> ("Motion Module.MMBack"=w1994:refnum<vi>)
        n1247 = Unbundle By Name(w1990) -> ("Main Home Screen.GUI"=w2000:refnum<vi>)
        n1248 = Unbundle By Name(w1990) -> ("Main Home Screen.MainPage"=w1996:refnum<vi>)
        n1249 = property on="Property Node" class="Bool (strict)"(reference=w1994, "Value"=FALSE) -> (reference out=w1992:refnum<vi>, error out=w1993:errorcluster)  [unwired: 1 in]
        n1250 = property on="Property Node" class="TabCtl (strict)"(reference=w1996, "Value"=T15."HOME") -> (reference out=w1998:refnum<vi>, error out=w1997:errorcluster)  [unwired: 1 in]
        n1251 = property on="Property Node" class="TabCtl (strict)"(reference=w2000, "Value"=T14."Load Head") -> (reference out=w2002:refnum<vi>, error out=w2001:errorcluster)  [unwired: 1 in]
        n1252 = Close Reference(reference=w1992, error in (no error)=w1993) -> ()  [unwired: 1 out]
        n1253 = Close Reference(reference=w1998, error in (no error)=w1997) -> ()  [unwired: 1 out]
        n1254 = Close Reference(reference=w2002, error in (no error)=w2001) -> ()  [unwired: 1 out]
        n1255 = call "DATA ENCRYPT STRING FILE WRITE.vi"("error in (no error)"=w2003, "User Action"="User selected Back to Load Selection", "main ref"=w1990) -> ("error out"=w2004:errorcluster)  [unwired: 6 in, 1 out]
      }
      frame "LHNext" {
        w2040 = FALSE ("Visible")
        n1256 = Unbundle By Name(w2006) -> ("Motion Module.HomeRot"=w2046:refnum<vi>)
        n1257 = Unbundle By Name(w2006) -> ("Motion Module.HomeScratch"=w2041:refnum<vi>)
        n1258 = Unbundle By Name(w2006) -> ("Motion Module.PlaceModule"=w2039:refnum<vi>)
        n1259 = Unbundle By Name(w2006) -> ("Motion Module.Motion Mode:"=w2032:refnum<vi>)
        n1260 = Unbundle By Name(w2006) -> ("Motion Module.Motion Direction:  3"=w2031:refnum<vi>)
        n1261 = Unbundle By Name(w2006) -> ("Motion Module.Wear Track Diameter (mm)"=w2025:refnum<vi>)
        n1262 = Unbundle By Name(w2006) -> ("Motion Module.Set WTD"=w2022:refnum<vi>)
        n1263 = Unbundle By Name(w2006) -> ("Motion Module.Rotary Module Selection"=w2016:refnum<vi>)
        n1264 = call "DATA ENCRYPT STRING FILE WRITE.vi"("error in (no error)"=w2055, "User Action"="User selected Select Module", "main ref"=w2006) -> ("error out"=w2019:errorcluster)  [unwired: 6 in, 1 out]
        n1265 = property on="Property Node" class="TabCtl (strict)"(reference=w2016, "Visible"=FALSE) -> (reference out=w2015:refnum<vi>, error out=w2017:errorcluster)  [unwired: 1 in]
        n1266 = property on="Property Node" class="Bool (strict)"(reference=w2046, error in=w2019, "Visible"=w2040) -> (reference out=w2044:refnum<vi>, error out=w2045:errorcluster)
        n1267 = property on="Property Node" class="Bool (strict)"(reference=w2041, error in=w2019, "Visible"=w2040) -> (reference out=w2043:refnum<vi>, error out=w2042:errorcluster)
        n1268 = property on="Property Node" class="Bool (strict)"(reference=w2039, error in=w2019, "Visible"=TRUE) -> (reference out=w2037:refnum<vi>, error out=w2038:errorcluster)
        n1269 = property on="Property Node" class="Ring (strict)"(reference=w2032, error in=w2019, "Visible"=FALSE) -> (reference out=w2034:refnum<vi>, error out=w2033:errorcluster)
        n1270 = property on="Property Node" class="Ring (strict)"(reference=w2031, error in=w2019, "Visible"=FALSE) -> (reference out=w2028:refnum<vi>, error out=w2030:errorcluster)
        n1271 = property on="Property Node" class="DigNum (strict)"(reference=w2025, "Visible"=FALSE) -> (reference out=w2024:refnum<vi>, error out=w2026:errorcluster)  [unwired: 1 in]
        n1272 = property on="Property Node" class="Bool (strict)"(reference=w2022, "Visible"=FALSE) -> (reference out=w2023:refnum<vi>, error out=w2021:errorcluster)  [unwired: 1 in]
        n1273 = Close Reference(reference=w2044, error in (no error)=w2045) -> ()  [unwired: 1 out]
        n1274 = Close Reference(reference=w2043, error in (no error)=w2042) -> ()  [unwired: 1 out]
        n1275 = Close Reference(reference=w2037, error in (no error)=w2038) -> ()  [unwired: 1 out]
        n1276 = Close Reference(reference=w2034, error in (no error)=w2033) -> ()  [unwired: 1 out]
        n1277 = Close Reference(reference=w2028, error in (no error)=w2030) -> ()  [unwired: 1 out]
        n1278 = Close Reference(reference=w2024, error in (no error)=w2026) -> ()  [unwired: 1 out]
        n1279 = Close Reference(reference=w2015, error in (no error)=w2017) -> ()  [unwired: 1 out]
        n1280 = Close Reference(reference=w2023, error in (no error)=w2021) -> ()  [unwired: 1 out]
        n1281 = Unbundle By Name(w2006) -> ("Motion Module.M3 Image"=w2014:refnum<vi>)
        n1282 = Unbundle By Name(w2006) -> ("Main Home Screen.GUI"=w2052:refnum<vi>)
        n1283 = Unbundle By Name(w2006) -> ("Main Home Screen.MainPage"=w2048:refnum<vi>)
        n1284 = Unbundle By Name(w2006) -> ("Loading.LHNext"=w2010:refnum<vi>)
        n1285 = property on="Property Node" class="TabCtl (strict)"(reference=w2014, "Value"=enum32{"Page 1", "Page 2"}."Page 2") -> (reference out=w2012:refnum<vi>, error out=w2013:errorcluster)  [unwired: 1 in]
        n1286 = property on="Property Node" class="TabCtl (strict)"(reference=w2048, "Value"=T15."HOME") -> (reference out=w2050:refnum<vi>, error out=w2049:errorcluster)  [unwired: 1 in]
        n1287 = property on="Property Node" class="TabCtl (strict)"(reference=w2052, "Value"=T14."Motion Module") -> (reference out=w2054:refnum<vi>, error out=w2053:errorcluster)  [unwired: 1 in]
        n1288 = property on="Property Node" class="Bool (strict)"(reference=w2010, "Value"=FALSE ("Visible")) -> (reference out=w2007:refnum<vi>, error out=w2009:errorcluster)  [unwired: 1 in]
        n1289 = Close Reference(reference=w2012, error in (no error)=w2013) -> ()  [unwired: 1 out]
        n1290 = Close Reference(reference=w2007, error in (no error)=w2009) -> ()  [unwired: 1 out]
        n1291 = Close Reference(reference=w2050, error in (no error)=w2049) -> ()  [unwired: 1 out]
        n1292 = Close Reference(reference=w2054, error in (no error)=w2053) -> ()  [unwired: 1 out]
      }
      frame "Rot Ver" {
        n1293 = call "Rotory Module Selection.vi"("error in (no error)"=w2059, "Data Cluster"=w2057) -> ("error out"=w2058:errorcluster)  [unwired: 9 in]
      }
      frame "Scratch" {
        n1294 = call "Scratch Module Selection.vi"("error in (no error)"=w2062, "Data Cluster"=w2060) -> ("error out"=w2061:errorcluster)  [unwired: 9 in]
      }
      frame "Traction" {
        n1295 = call "TractionModule Selection.vi"("error in (no error)"=w2065, "Data Cluster"=w2063) -> ("error out"=w2064:errorcluster)  [unwired: 9 in]
      }
      frame "Motion Mode:" {
        n1296 = Unbundle By Name(w2066) -> ("Motion Module.Motion Mode:"=w2068:refnum<vi>)
        n1297 = property on="Property Node" class="Ring (strict)"(reference=w2068) -> (reference out=w2070:refnum<vi>, error out=w2069:errorcluster, "Value"=w2067:u16)  [unwired: 1 in]
        n1298 = Close Reference(reference=w2070, error in (no error)=w2069) -> ()  [unwired: 1 out]
        n1299 = case shown="3" w2067 {
          tunnel: w2072 -> [w2089 w2106 w2123 w2140]
          tunnel: [w2088 w2105 w2122 w2139] -> w2071
          tunnel: w2066 -> [w2087 w2104 w2121 w2138]
          tunnel: w2066 -> [w2073 w2091 w2107 w2124]
          frame 0, Default {
            n1300 = Unbundle By Name(w2073) -> ("Motion Module.Rotary Module Selection"=w2083:refnum<vi>)
            n1301 = Unbundle By Name(w2073) -> ("Motion Module.Motion Direction:  3"=w2081:refnum<vi>)
            n1302 = Unbundle By Name(w2073) -> ("Main Screen.Angle (Deg)"=w2075:refnum<vi>)
            n1303 = property on="Property Node" class="TabCtl (strict)"(reference=w2083, "Value"=T17."Uniform Rotation") -> (reference out=w2085:refnum<vi>, error out=w2084:errorcluster)  [unwired: 1 in]
            n1304 = property on="Property Node" class="DigNum (strict)"(reference=w2075, "DisabledEnum"=T26."Disabled and Grayed Out" ("Disabled")) -> (reference out=w2077:refnum<vi>, error out=w2076:errorcluster)  [unwired: 1 in]
            n1305 = property on="Property Node" class="Ring (strict)"(reference=w2081, "Visible"=TRUE) -> (reference out=w2079:refnum<vi>, error out=w2080:errorcluster)  [unwired: 1 in]
            n1306 = Close Reference(reference=w2085, error in (no error)=w2084) -> ()  [unwired: 1 out]
            n1307 = Close Reference(reference=w2077, error in (no error)=w2076) -> ()  [unwired: 1 out]
            n1308 = Close Reference(reference=w2079, error in (no error)=w2080) -> ()  [unwired: 1 out]
            n1309 = call "DATA ENCRYPT STRING FILE WRITE.vi"("error in (no error)"=w2089, "User Action"="User Selected Uniform Rotation", "main ref"=w2087) -> ("error out"=w2088:errorcluster)  [unwired: 6 in, 1 out]
          }
          frame 1 {
            n1310 = Unbundle By Name(w2091) -> ("Motion Module.Rotary Module Selection"=w2100:refnum<vi>)
            n1311 = Unbundle By Name(w2091) -> ("Motion Module.Motion Direction:  3"=w2098:refnum<vi>)
            n1312 = Unbundle By Name(w2091) -> ("Main Screen.Angle (Deg)"=w2092:refnum<vi>)
            n1313 = property on="Property Node" class="TabCtl (strict)"(reference=w2100, "Value"=T17."Angular Oscillation") -> (reference out=w2102:refnum<vi>, error out=w2101:errorcluster)  [unwired: 1 in]
            n1314 = property on="Property Node" class="DigNum (strict)"(reference=w2092, "DisabledEnum"=T26."Enabled" ("Disabled")) -> (reference out=w2094:refnum<vi>, error out=w2093:errorcluster)  [unwired: 1 in]
            n1315 = property on="Property Node" class="Ring (strict)"(reference=w2098, "Visible"=FALSE) -> (reference out=w2096:refnum<vi>, error out=w2097:errorcluster)  [unwired: 1 in]
            n1316 = Close Reference(reference=w2102, error in (no error)=w2101) -> ()  [unwired: 1 out]
            n1317 = Close Reference(reference=w2096, error in (no error)=w2097) -> ()  [unwired: 1 out]
            n1318 = Close Reference(reference=w2094, error in (no error)=w2093) -> ()  [unwired: 1 out]
            n1319 = call "DATA ENCRYPT STRING FILE WRITE.vi"("error in (no error)"=w2106, "User Action"="User Selected Angular Oscillation", "main ref"=w2104) -> ("error out"=w2105:errorcluster)  [unwired: 6 in, 1 out]
          }
          frame 2 {
            n1320 = Unbundle By Name(w2107) -> ("Motion Module.Rotary Module Selection"=w2117:refnum<vi>)
            n1321 = Unbundle By Name(w2107) -> ("Motion Module.Motion Direction:  3"=w2115:refnum<vi>)
            n1322 = Unbundle By Name(w2107) -> ("Main Screen.Angle (Deg)"=w2109:refnum<vi>)
            n1323 = property on="Property Node" class="DigNum (strict)"(reference=w2109, "DisabledEnum"=T26."Disabled and Grayed Out" ("Disabled")) -> (reference out=w2111:refnum<vi>, error out=w2110:errorcluster)  [unwired: 1 in]
            n1324 = property on="Property Node" class="TabCtl (strict)"(reference=w2117, "Value"=T17."Speed Ramp") -> (reference out=w2119:refnum<vi>, error out=w2118:errorcluster)  [unwired: 1 in]
            n1325 = property on="Property Node" class="Ring (strict)"(reference=w2115, "Visible"=TRUE) -> (reference out=w2113:refnum<vi>, error out=w2114:errorcluster)  [unwired: 1 in]
            n1326 = Close Reference(reference=w2111, error in (no error)=w2110) -> ()  [unwired: 1 out]
            n1327 = Close Reference(reference=w2119, error in (no error)=w2118) -> ()  [unwired: 1 out]
            n1328 = Close Reference(reference=w2113, error in (no error)=w2114) -> ()  [unwired: 1 out]
            n1329 = call "DATA ENCRYPT STRING FILE WRITE.vi"("error in (no error)"=w2123, "User Action"="User Selected Ramp Mode", "main ref"=w2121) -> ("error out"=w2122:errorcluster)  [unwired: 6 in, 1 out]
          }
          frame 3 {
            n1330 = Unbundle By Name(w2124) -> ("Motion Module.Rotary Module Selection"=w2134:refnum<vi>)
            n1331 = Unbundle By Name(w2124) -> ("Motion Module.Motion Direction:  3"=w2132:refnum<vi>)
            n1332 = Unbundle By Name(w2124) -> ("Main Screen.Angle (Deg)"=w2126:refnum<vi>)
            n1333 = property on="Property Node" class="TabCtl (strict)"(reference=w2134, "Value"=T17."Speed Step") -> (reference out=w2136:refnum<vi>, error out=w2135:errorcluster)  [unwired: 1 in]
            n1334 = property on="Property Node" class="DigNum (strict)"(reference=w2126, "DisabledEnum"=T26."Disabled and Grayed Out" ("Disabled")) -> (reference out=w2128:refnum<vi>, error out=w2127:errorcluster)  [unwired: 1 in]
            n1335 = property on="Property Node" class="Ring (strict)"(reference=w2132, "Visible"=TRUE) -> (reference out=w2130:refnum<vi>, error out=w2131:errorcluster)  [unwired: 1 in]
            n1336 = Close Reference(reference=w2136, error in (no error)=w2135) -> ()  [unwired: 1 out]
            n1337 = Close Reference(reference=w2128, error in (no error)=w2127) -> ()  [unwired: 1 out]
            n1338 = Close Reference(reference=w2130, error in (no error)=w2131) -> ()  [unwired: 1 out]
            n1339 = call "DATA ENCRYPT STRING FILE WRITE.vi"("error in (no error)"=w2140, "User Action"="User Selected Step Mode", "main ref"=w2138) -> ("error out"=w2139:errorcluster)  [unwired: 6 in, 1 out]
          }
        }
      }
      frame "MMNext" {
        n1340 = Unbundle By Name(w2141) -> ("Motion Module.MMNext"=w2146:refnum<vi>)
        n1341 = Unbundle By Name(w2141) -> ("Motion Module.MMNext"=w2153:refnum<vi>)
        n1342 = Unbundle By Name(w2141) -> ("Main Home Screen.GUI"=w2155:refnum<vi>)
        n1343 = property on="Property Node" class="Bool (strict)"(reference=w2146, "Value"=FALSE ("Visible")) -> (reference out=w2143:refnum<vi>, error out=w2145:errorcluster)  [unwired: 1 in]
        n1344 = property on="Property Node" class="TabCtl (strict)"(reference=w2155, "Value"=T14."Environment") -> (reference out=w2157:refnum<vi>, error out=w2156:errorcluster)  [unwired: 1 in]
        n1345 = property on="Property Node" class="Bool (strict)"(reference=w2153, "Value"=FALSE) -> (reference out=w2151:refnum<vi>, error out=w2152:errorcluster)  [unwired: 1 in]
        n1346 = Close Reference(reference=w2143, error in (no error)=w2145) -> ()  [unwired: 1 out]
        n1347 = Close Reference(reference=w2151, error in (no error)=w2152) -> ()  [unwired: 1 out]
        n1348 = Close Reference(reference=w2157, error in (no error)=w2156) -> ()  [unwired: 1 out]
        n1349 = call "DATA ENCRYPT STRING FILE WRITE.vi"("error in (no error)"=w2148, "User Action"="User Selected SetUp Module", "main ref"=w2141) -> ("error out"=w2147:errorcluster)  [unwired: 6 in, 1 out]
        n1350 = call "Main Screen Tab Visible.vi"("error in (no error)"=w2147, "main ref"=w2141) -> ("error out"=w2142:errorcluster)  [unwired: 9 in]
      }
      frame "APBack" {
        n1351 = Unbundle By Name(w2158) -> ("Environmental control.APBack"=w2165:refnum<vi>)
        n1352 = Unbundle By Name(w2158) -> ("Main Home Screen.GUI"=w2167:refnum<vi>)
        n1353 = property on="Property Node" class="TabCtl (strict)"(reference=w2167, "Value"=T14."Motion Module") -> (reference out=w2169:refnum<vi>, error out=w2168:errorcluster)  [unwired: 1 in]
        n1354 = property on="Property Node" class="Bool (strict)"(reference=w2165, "Value"=FALSE) -> (reference out=w2163:refnum<vi>, error out=w2164:errorcluster)  [unwired: 1 in]
        n1355 = Close Reference(reference=w2163, error in (no error)=w2164) -> ()  [unwired: 1 out]
        n1356 = Close Reference(reference=w2169, error in (no error)=w2168) -> ()  [unwired: 1 out]
        n1357 = call "DATA ENCRYPT STRING FILE WRITE.vi"("error in (no error)"=w2160, "User Action"="User Selected Back to Module", "main ref"=w2158) -> ("error out"=w2159:errorcluster)  [unwired: 6 in, 1 out]
      }
      frame "SNext" {
        n1358 = Unbundle By Name(w2171) -> ("Environmental control.Enter the Stage \nTemperature (°C):"=w2172:refnum<vi>)
        n1359 = Unbundle By Name(w2171) -> ("Environmental control.Acoustic Emission 3"=w2179:refnum<vi>)
        n1360 = property on="Property Node" class="Bool (strict)"(reference=w2179) -> (reference out=w2177:refnum<vi>, error out=w2178:errorcluster, "Value"=w2175:bool)  [unwired: 1 in]
        n1361 = property on="Property Node" class="DigNum (strict)"(reference=w2172) -> (reference out=w2174:refnum<vi>, error out=w2173:errorcluster, "Value"=w2170:dbl)  [unwired: 1 in]
        n1362 = Close Reference(reference=w2177, error in (no error)=w2178) -> ()  [unwired: 1 out]
        n1363 = Close Reference(reference=w2174, error in (no error)=w2173) -> ()  [unwired: 1 out]
        n1364 = case shown="True" w2175 {
          tunnel: w2181 -> [w2184 w2188]
          tunnel: [w2184 w2185] -> w2176
          tunnel: w2171 -> [_ w2186]
          frame False {
          }
          frame True {
            n1365 = call "Acq Gain Selection.vi"("error in (no error)"=w2188, "Data Cluster"=w2186) -> ("error out"=w2187:errorcluster)  [unwired: 9 in]
            n1366 = call <vilib>:"Clear Errors.vi"("error in (no error)"=w2187) -> ("error out"=w2185:errorcluster)  [unwired: 5 in, 1 out]
          }
        }
        n1367 = local write "SetTmp"(w2170) -> ()
        n1368 = call "Init Before Main Screen.vi"("error in (no error)"=w2176, "Data Cluster"=w2171) -> ("error out"=w2180:errorcluster)  [unwired: 9 in]
        n1369 = call "DATA ENCRYPT STRING FILE WRITE.vi"("error in (no error)"=w2180, "User Action"="User Pressed Setup", "main ref"=w2171) -> ("error out"=w2182:errorcluster)  [unwired: 6 in, 1 out]
      }
      frame "Enable Platform" {
        n1370 = call "Reinitialise Load cell after Error.vi"("error in (no error)"=w2193, "main ref"=w2189) -> ("error out"=w2191:errorcluster)  [unwired: 9 in]
        n1371 = Unbundle By Name(w2189) -> ("Platform Settings.Enable Platform"=w2216:refnum<vi>)
        n1372 = Bundle By Name(cluster=T11 {"Sequence ID"=0, "Mode Command"=0, "Distance"=0.0, "SPEED"=0.0, "Reserved"=0.0, "SPARE 1"=0, "SPARE 2"=0, "SPARE 3"=0, "SPARE 4"=0, "SPARE 5"=0, "SPARE 6"=0, "SPARE 7"=0, "SPARE 8"=0, "SPARE 9"=0, "SPARE 10"=0, "SPARE 11"=0, "SPARE 12"=0, "SPARE 13"=0, "SPARE 14"=0, "SPARE 15"=0, "SPARE 16"=0, "SPARE 17"=0} ("Value"), "Mode Command"=u8 1, "Distance"=sgl 0.0, "SPEED"=sgl 0.0, "Sequence ID"=u16 0) -> (w2202:T11)
        n1373 = Unbundle By Name(w2189) -> ("Heave AND Surge.UPLINK HEAVE"=w2195:refnum<vi>)
        n1374 = property on="Property Node" class="Bool (strict)"(reference=w2216, "Value"=FALSE) -> (reference out=w2214:refnum<vi>, error out=w2215:errorcluster)  [unwired: 1 in]
        n1375 = property on="Property Node" class="Clust (strict)"(reference=w2195, error in=w2191, "Value"=w2202) -> (reference out=w2201:refnum<vi>, error out=w2200:errorcluster)
        n1376 = Close Reference(reference=w2214, error in (no error)=w2215) -> ()  [unwired: 1 out]
        n1377 = Close Reference(reference=w2201, error in (no error)=w2200) -> (error out=w2192:errorcluster)
        n1378 = call "DATA ENCRYPT STRING FILE WRITE.vi"("error in (no error)"=w2192, "User Action"="User Pressed Enable Platform", "main ref"=w2189) -> ("error out"=w2190:errorcluster)  [unwired: 6 in, 1 out]
        n1379 = call "HEAVE WRITE FGV.vi"("Enum - Menu"=Heave_Write_enum."WRITE", "error in (no error)"=w2190, "main ref"=w2189) -> ("error out"=w2206:errorcluster)  [unwired: 8 in]
        n1380 = call "SET LOAD PARAMETERS.vi"("error in (no error)"=w2190, "main ref"=w2189) -> ()  [unwired: 9 in, 1 out]
        n1381 = call "TRACTION HOME.vi"("error in (no error)"=w2190, "Data Cluster"=w2189) -> ("error out"=→"error out":errorcluster)  [unwired: 9 in]
        n1382 = Unbundle By Name(w2189) -> ("Heave AND Surge.Read Heave Temp"=w2210:refnum<vi>)
        n1383 = property on="Property Node" class="Bool (strict)"(reference=w2210, error in=w2206, "Value"=TRUE) -> (reference out=w2208:refnum<vi>, error out=w2209:errorcluster)
        n1384 = Close Reference(reference=w2208, error in (no error)=w2209) -> (error out=w2205:errorcluster)
        "HEAVE ENABLE" <- TRUE ("HEAVE ENABLE")
      }
      frame "Heave Up main" {
        n1385 = Unbundle By Name(w2217) -> ("Platform Settings.Heave Up main"=w2227:refnum<vi>)
        n1386 = call "Heave Up Main.vi"("error in (no error)"=w2219, "main ref"=w2217) -> ("error out"=w2218:errorcluster)  [unwired: 9 in]
        n1387 = property on="Property Node" class="Bool (strict)"(reference=w2227, "Value"=FALSE) -> (reference out=w2225:refnum<vi>, error out=w2226:errorcluster)  [unwired: 1 in]
        n1388 = Close Reference(reference=w2225, error in (no error)=w2226) -> ()  [unwired: 1 out]
        n1389 = call "DATA ENCRYPT STRING FILE WRITE.vi"("error in (no error)"=w2218, "User Action"="User Pressed Heave UP", "main ref"=w2217) -> ("error out"=w2222:errorcluster)  [unwired: 6 in, 1 out]
        n1390 = call "HEAVE WRITE FGV.vi"("Enum - Menu"=Heave_Write_enum."WRITE", "error in (no error)"=w2222, "main ref"=w2217) -> ("error out"=w2221:errorcluster)  [unwired: 8 in]
      }
      frame "Heave Up MM" {
        n1391 = Unbundle By Name(w2228) -> ("Motion Module.Heave Up MM"=w2238:refnum<vi>)
        n1392 = call "Heave Up Motion Module.vi"("error in (no error)"=w2230, "main ref"=w2228) -> ("error out"=w2229:errorcluster)  [unwired: 9 in]
        n1393 = property on="Property Node" class="Bool (strict)"(reference=w2238, "Value"=FALSE) -> (reference out=w2236:refnum<vi>, error out=w2237:errorcluster)  [unwired: 1 in]
        n1394 = Close Reference(reference=w2236, error in (no error)=w2237) -> ()  [unwired: 1 out]
        n1395 = call "DATA ENCRYPT STRING FILE WRITE.vi"("error in (no error)"=w2229, "User Action"="User Pressed Heave UP in Motion Module", "main ref"=w2228) -> ("error out"=w2233:errorcluster)  [unwired: 6 in, 1 out]
        n1396 = call "HEAVE WRITE FGV.vi"("Enum - Menu"=Heave_Write_enum."WRITE", "error in (no error)"=w2233, "main ref"=w2228) -> ("error out"=w2232:errorcluster)  [unwired: 8 in]
      }
      frame "Heave Down Main" {
        n1397 = call "Heave Down Main.vi"("error in (no error)"=w2241, "main ref"=w2239) -> ("error out"=w2240:errorcluster)  [unwired: 9 in]
        n1398 = Unbundle By Name(w2239) -> ("Platform Settings.Heave Down Main"=w2249:refnum<vi>)
        n1399 = property on="Property Node" class="Bool (strict)"(reference=w2249, "Value"=FALSE) -> (reference out=w2247:refnum<vi>, error out=w2248:errorcluster)  [unwired: 1 in]
        n1400 = Close Reference(reference=w2247, error in (no error)=w2248) -> ()  [unwired: 1 out]
        n1401 = call "DATA ENCRYPT STRING FILE WRITE.vi"("error in (no error)"=w2240, "User Action"="User Pressed Heave DOWN", "main ref"=w2239) -> ("error out"=w2244:errorcluster)  [unwired: 6 in, 1 out]
        n1402 = call "HEAVE WRITE FGV.vi"("Enum - Menu"=Heave_Write_enum."WRITE", "error in (no error)"=w2244, "main ref"=w2239) -> ("error out"=w2243:errorcluster)  [unwired: 8 in]
      }
      frame "Heave Down MM" {
        n1403 = call "Heave Down Motion Module.vi"("error in (no error)"=w2252, "main ref"=w2250) -> ("error out"=w2251:errorcluster)  [unwired: 9 in]
        n1404 = Unbundle By Name(w2250) -> ("Motion Module.Heave Down MM"=w2260:refnum<vi>)
        n1405 = property on="Property Node" class="Bool (strict)"(reference=w2260, "Value"=FALSE) -> (reference out=w2258:refnum<vi>, error out=w2259:errorcluster)  [unwired: 1 in]
        n1406 = Close Reference(reference=w2258, error in (no error)=w2259) -> ()  [unwired: 1 out]
        n1407 = call "DATA ENCRYPT STRING FILE WRITE.vi"("error in (no error)"=w2251, "User Action"="User Pressed Heave DOWN in Motion Module", "main ref"=w2250) -> ("error out"=w2255:errorcluster)  [unwired: 6 in, 1 out]
        n1408 = call "HEAVE WRITE FGV.vi"("Enum - Menu"=Heave_Write_enum."WRITE", "error in (no error)"=w2255, "main ref"=w2250) -> ("error out"=w2254:errorcluster)  [unwired: 8 in]
      }
      frame "Surge Backward Main" {
        n1409 = Unbundle By Name(w2261) -> ("Platform Settings.Surge Backward Main"=w2271:refnum<vi>)
        n1410 = call "Surge Backward Main.vi"("error in (no error)"=w2263, "main ref"=w2261) -> ("error out"=w2262:errorcluster)  [unwired: 9 in]
        n1411 = property on="Property Node" class="Bool (strict)"(reference=w2271, "Value"=FALSE) -> (reference out=w2269:refnum<vi>, error out=w2270:errorcluster)  [unwired: 1 in]
        n1412 = Close Reference(reference=w2269, error in (no error)=w2270) -> ()  [unwired: 1 out]
        n1413 = call "DATA ENCRYPT STRING FILE WRITE.vi"("error in (no error)"=w2262, "User Action"="User Pressed Surge Backward", "main ref"=w2261) -> ("error out"=w2266:errorcluster)  [unwired: 6 in, 1 out]
        n1414 = call "HEAVE WRITE FGV.vi"("Enum - Menu"=Heave_Write_enum."WRITE", "error in (no error)"=w2266, "main ref"=w2261) -> ("error out"=w2265:errorcluster)  [unwired: 8 in]
      }
      frame "Surge Backward MM" {
        n1415 = Unbundle By Name(w2272) -> ("Motion Module.Surge Backward MM"=w2282:refnum<vi>)
        n1416 = call "Surge Backward MM.vi"("error in (no error)"=w2274, "main ref"=w2272) -> ("error out"=w2273:errorcluster)  [unwired: 9 in]
        n1417 = property on="Property Node" class="Bool (strict)"(reference=w2282, "Value"=FALSE) -> (reference out=w2280:refnum<vi>, error out=w2281:errorcluster)  [unwired: 1 in]
        n1418 = Close Reference(reference=w2280, error in (no error)=w2281) -> ()  [unwired: 1 out]
        n1419 = call "DATA ENCRYPT STRING FILE WRITE.vi"("error in (no error)"=w2273, "User Action"="User Pressed Surge Backward in Motion Module", "main ref"=w2272) -> ("error out"=w2277:errorcluster)  [unwired: 6 in, 1 out]
        n1420 = call "HEAVE WRITE FGV.vi"("Enum - Menu"=Heave_Write_enum."WRITE", "error in (no error)"=w2277, "main ref"=w2272) -> ("error out"=w2276:errorcluster)  [unwired: 8 in]
      }
      frame "Surge Forward Main" {
        n1421 = Unbundle By Name(w2283) -> ("Platform Settings.Surge Forward Main"=w2293:refnum<vi>)
        n1422 = call "Surge Forward Main.vi"("error in (no error)"=w2285, "main ref"=w2283) -> ("error out"=w2284:errorcluster)  [unwired: 9 in]
        n1423 = property on="Property Node" class="Bool (strict)"(reference=w2293, "Value"=FALSE) -> (reference out=w2291:refnum<vi>, error out=w2292:errorcluster)  [unwired: 1 in]
        n1424 = Close Reference(reference=w2291, error in (no error)=w2292) -> ()  [unwired: 1 out]
        n1425 = call "DATA ENCRYPT STRING FILE WRITE.vi"("error in (no error)"=w2284, "User Action"="User Pressed Surge Forward", "main ref"=w2283) -> ("error out"=w2288:errorcluster)  [unwired: 6 in, 1 out]
        n1426 = call "HEAVE WRITE FGV.vi"("Enum - Menu"=Heave_Write_enum."WRITE", "error in (no error)"=w2288, "main ref"=w2283) -> ("error out"=w2287:errorcluster)  [unwired: 8 in]
      }
      frame "Surge Forward MM" {
        n1427 = Unbundle By Name(w2294) -> ("Motion Module.Surge Forward MM"=w2304:refnum<vi>)
        n1428 = call "Surge Forward MM.vi"("error in (no error)"=w2296, "main ref"=w2294) -> ("error out"=w2295:errorcluster)  [unwired: 9 in]
        n1429 = property on="Property Node" class="Bool (strict)"(reference=w2304, "Value"=FALSE) -> (reference out=w2302:refnum<vi>, error out=w2303:errorcluster)  [unwired: 1 in]
        n1430 = Close Reference(reference=w2302, error in (no error)=w2303) -> ()  [unwired: 1 out]
        n1431 = call "DATA ENCRYPT STRING FILE WRITE.vi"("error in (no error)"=w2295, "User Action"="User Pressed Surge Forward in Motion Module", "main ref"=w2294) -> ("error out"=w2299:errorcluster)  [unwired: 6 in, 1 out]
        n1432 = call "HEAVE WRITE FGV.vi"("Enum - Menu"=Heave_Write_enum."WRITE", "error in (no error)"=w2299, "main ref"=w2294) -> ("error out"=w2298:errorcluster)  [unwired: 8 in]
      }
      frame "Sway Left Main" {
        n1433 = call "Sway Left Main.vi"("error in (no error)"=w2308, "main ref"=w2306) -> ("error out"=w2307:errorcluster)  [unwired: 9 in]
        n1434 = Unbundle By Name(w2306) -> ("Platform Settings.Sway Left Main"=w2315:refnum<vi>)
        n1435 = property on="Property Node" class="Bool (strict)"(reference=w2315, "Value"=FALSE) -> (reference out=w2313:refnum<vi>, error out=w2314:errorcluster)  [unwired: 1 in]
        n1436 = Close Reference(reference=w2313, error in (no error)=w2314) -> ()  [unwired: 1 out]
        n1437 = call "DATA ENCRYPT STRING FILE WRITE.vi"("error in (no error)"=w2307, "User Action"="User Pressed Sway Left ", "main ref"=w2306) -> ("error out"=w2310:errorcluster)  [unwired: 6 in, 1 out]
        n1438 = call "SWAY WRITE FGV.vi"("Enum - Menu"=Sway_Write_enum."WRITE", "error in (no error)"=w2310, "main ref"=w2306) -> ("error out"=w2309:errorcluster)  [unwired: 8 in]
      }
      frame "Sway Left MM" {
        n1439 = call "Sway Left MM.vi"("error in (no error)"=w2319, "main ref"=w2317) -> ("error out"=w2318:errorcluster)  [unwired: 9 in]
        n1440 = Unbundle By Name(w2317) -> ("Motion Module.Sway Left MM"=w2326:refnum<vi>)
        n1441 = property on="Property Node" class="Bool (strict)"(reference=w2326, "Value"=FALSE) -> (reference out=w2324:refnum<vi>, error out=w2325:errorcluster)  [unwired: 1 in]
        n1442 = Close Reference(reference=w2324, error in (no error)=w2325) -> ()  [unwired: 1 out]
        n1443 = call "DATA ENCRYPT STRING FILE WRITE.vi"("error in (no error)"=w2318, "User Action"="User Pressed Sway Left in MM", "main ref"=w2317) -> ("error out"=w2321:errorcluster)  [unwired: 6 in, 1 out]
        n1444 = call "SWAY WRITE FGV.vi"("Enum - Menu"=Sway_Write_enum."WRITE", "error in (no error)"=w2321, "main ref"=w2317) -> ("error out"=w2320:errorcluster)  [unwired: 8 in]
      }
      frame "Sway Right MM" {
        n1445 = call "Sway Right MM.vi"("error in (no error)"=w2330, "main ref"=w2328) -> ("error out"=w2329:errorcluster)  [unwired: 9 in]
        n1446 = Unbundle By Name(w2328) -> ("Motion Module.Sway Right MM"=w2337:refnum<vi>)
        n1447 = property on="Property Node" class="Bool (strict)"(reference=w2337, "Value"=FALSE) -> (reference out=w2335:refnum<vi>, error out=w2336:errorcluster)  [unwired: 1 in]
        n1448 = Close Reference(reference=w2335, error in (no error)=w2336) -> ()  [unwired: 1 out]
        n1449 = call "DATA ENCRYPT STRING FILE WRITE.vi"("error in (no error)"=w2329, "User Action"="User Pressed Sway Right in MM", "main ref"=w2328) -> ("error out"=w2332:errorcluster)  [unwired: 6 in, 1 out]
        n1450 = call "SWAY WRITE FGV.vi"("Enum - Menu"=Sway_Write_enum."WRITE", "error in (no error)"=w2332, "main ref"=w2328) -> ("error out"=w2331:errorcluster)  [unwired: 8 in]
      }
      frame "Sway Right Main" {
        n1451 = call "Sway Right Main.vi"("error in (no error)"=w2341, "main ref"=w2339) -> ("error out"=w2340:errorcluster)  [unwired: 9 in]
        n1452 = Unbundle By Name(w2339) -> ("Platform Settings.Sway Right Main"=w2348:refnum<vi>)
        n1453 = property on="Property Node" class="Bool (strict)"(reference=w2348, "Value"=FALSE) -> (reference out=w2346:refnum<vi>, error out=w2347:errorcluster)  [unwired: 1 in]
        n1454 = Close Reference(reference=w2346, error in (no error)=w2347) -> ()  [unwired: 1 out]
        n1455 = call "DATA ENCRYPT STRING FILE WRITE.vi"("error in (no error)"=w2340, "User Action"="User Pressed Sway Right", "main ref"=w2339) -> ("error out"=w2343:errorcluster)  [unwired: 6 in, 1 out]
        n1456 = call "SWAY WRITE FGV.vi"("Enum - Menu"=Sway_Write_enum."WRITE", "error in (no error)"=w2343, "main ref"=w2339) -> ("error out"=w2342:errorcluster)  [unwired: 8 in]
      }
      frame "Manual Write Heave & Surge" {
        n1457 = Unbundle By Name(w2349) -> ("Heave AND Surge.Manual Write"=w2358:refnum<vi>)
        n1458 = property on="Property Node" class="Bool (strict)"(reference=w2358, "Value"=FALSE) -> (reference out=w2356:refnum<vi>, error out=w2357:errorcluster)  [unwired: 1 in]
        n1459 = Close Reference(reference=w2356, error in (no error)=w2357) -> ()  [unwired: 1 out]
        n1460 = call "DATA ENCRYPT STRING FILE WRITE.vi"("error in (no error)"=w2350, "User Action"="User Pressed Manual Write Heave and Surge", "main ref"=w2349) -> ("error out"=w2353:errorcluster)  [unwired: 6 in, 1 out]
        n1461 = call "HEAVE WRITE FGV.vi"("Enum - Menu"=Heave_Write_enum."WRITE", "error in (no error)"=w2353, "main ref"=w2349) -> ("error out"=w2352:errorcluster)  [unwired: 8 in]
      }
      frame "Manual Write SWAY" {
        n1462 = Unbundle By Name(w2360) -> ("SWAY.Manual Write SWAY"=w2368:refnum<vi>)
        n1463 = property on="Property Node" class="Bool (strict)"(reference=w2368, "Value"=FALSE) -> (reference out=w2366:refnum<vi>, error out=w2367:errorcluster)  [unwired: 1 in]
        n1464 = Close Reference(reference=w2366, error in (no error)=w2367) -> ()  [unwired: 1 out]
        n1465 = call "DATA ENCRYPT STRING FILE WRITE.vi"("error in (no error)"=w2361, "User Action"="User Pressed Manual Write Sway", "main ref"=w2360) -> ("error out"=w2363:errorcluster)  [unwired: 6 in, 1 out]
        n1466 = call "SWAY WRITE FGV.vi"("Enum - Menu"=Sway_Write_enum."WRITE", "error in (no error)"=w2363, "main ref"=w2360) -> ("error out"=w2362:errorcluster)  [unwired: 8 in]
      }
      frame "Manual Write TRACTION" {
        n1467 = Unbundle By Name(w2370) -> ("Traction.Manual Write TRACTION"=w2378:refnum<vi>)
        n1468 = property on="Property Node" class="Bool (strict)"(reference=w2378, "Value"=FALSE) -> (reference out=w2376:refnum<vi>, error out=w2377:errorcluster)  [unwired: 1 in]
        n1469 = Close Reference(reference=w2376, error in (no error)=w2377) -> ()  [unwired: 1 out]
        n1470 = call "DATA ENCRYPT STRING FILE WRITE.vi"("error in (no error)"=w2371, "User Action"="User Pressed Manual Write Traction", "main ref"=w2370) -> ("error out"=w2373:errorcluster)  [unwired: 6 in, 1 out]
        n1471 = call "TRACTION WRITE FGV.vi"("Enum - Menu"=Traction_Write_enum."WRITE", "error in (no error)"=w2373, "main ref"=w2370) -> ("error out"=w2372:errorcluster)  [unwired: 8 in]
      }
      frame "Manual Write ACQUOSTIC" {
        n1472 = local write "Manual Write Acquostic"(FALSE ("Manual Write Acquostic")) -> ()
        n1473 = call "DATA ENCRYPT STRING FILE WRITE.vi"("error in (no error)"=w2382, "User Action"="User Pressed Manual Write Acquostics", "main ref"=w2381) -> ("error out"=w2384:errorcluster)  [unwired: 6 in, 1 out]
        n1474 = call "Acq Write Loop.vi"("Enum - Menu"=Write_Main_Enum."WRITE", "error in (no error)"=w2384, "main ref"=w2381) -> ("error out"=w2383:errorcluster)  [unwired: 8 in]
      }
      frame "Load En" {
        # "zNL 2"
        n1475 = Unbundle By Name(w2387) -> ("Main Screen.Load En"=w2392:refnum<vi>)
        n1476 = property on="Property Node" class="Bool (strict)"(reference=w2392) -> (reference out=w2390:refnum<vi>, error out=w2391:errorcluster, "Value"=w2386:bool)  [unwired: 1 in]
        n1477 = Close Reference(reference=w2390, error in (no error)=w2391) -> ()  [unwired: 1 out]
        n1478 = case shown="False" w2386 {
          tunnel: [w2404 w2414] -> w2388
          tunnel: w2389 -> [w2406 w2413]
          tunnel: w2387 -> [w2394 w2408]
          tunnel: w2387 -> [w2402 _]
          tunnel: w2387 -> [w2401 _]
          frame False {
            n1479 = call "DATA ENCRYPT STRING FILE WRITE.vi"("error in (no error)"=w2406, "User Action"="User Pressed UnLoad on Main Screen", "main ref"=w2394) -> ("error out"=w2395:errorcluster)  [unwired: 6 in, 1 out]
            n1480 = call "Stall Data Flow.vim"("value in"=w2395, "milliseconds to wait"=u32 2000) -> ("value out"=w2400:errorcluster)  [unwired: 1 out]
            n1481 = Unbundle By Name(w2394) -> ("Main Screen.zNL 2"=w2398:refnum<vi>)
            n1482 = property on="Property Node" class="Bool (strict)"(reference=w2398, "DisabledEnum"=T26."Enabled" ("Disabled")) -> (reference out=w2396:refnum<vi>, error out=w2397:errorcluster)  [unwired: 1 in]
            n1483 = call "PID UNLOAD.vi"("error in (no error)"=w2400, "main ref"=w2401) -> ("error out"=w2403:errorcluster)  [unwired: 9 in]
            n1484 = Close Reference(reference=w2396, error in (no error)=w2397) -> ()  [unwired: 1 out]
            n1485 = call "HEAVE WRITE FGV.vi"("Enum - Menu"=Heave_Write_enum."WRITE", "error in (no error)"=w2403, "main ref"=w2402) -> ("error out"=w2404:errorcluster)  [unwired: 8 in]
          }
          frame True {
            n1486 = call "DATA ENCRYPT STRING FILE WRITE.vi"("error in (no error)"=w2413, "User Action"="User Pressed Load on Main Screen", "main ref"=w2408) -> ("error out"=w2414:errorcluster)  [unwired: 6 in, 1 out]
            n1487 = Unbundle By Name(w2408) -> ("Main Screen.zNL 2"=w2412:refnum<vi>)
            n1488 = property on="Property Node" class="Bool (strict)"(reference=w2412, "DisabledEnum"=T26."Disabled and Grayed Out" ("Disabled")) -> (reference out=w2410:refnum<vi>, error out=w2411:errorcluster)  [unwired: 1 in]
            n1489 = Close Reference(reference=w2410, error in (no error)=w2411) -> ()  [unwired: 1 out]
          }
        }
      }
      frame "apply load" {
        n1490 = Unbundle By Name(w2417) -> ("Main Screen.Load En"=w2422:refnum<vi>)
        n1491 = property on="Property Node" class="Bool (strict)"(reference=w2422) -> (reference out=w2420:refnum<vi>, error out=w2421:errorcluster, "Value"=w2416:bool)  [unwired: 1 in]
        n1492 = Close Reference(reference=w2420, error in (no error)=w2421) -> ()  [unwired: 1 out]
        n1493 = case shown="False" w2416 {
          tunnel: [w2429 w2436] -> w2418
          tunnel: w2419 -> [w2432 w2435]
          tunnel: w2417 -> [w2431 w2434]
          tunnel: w2417 -> [w2426 _]
          tunnel: w2417 -> [w2425 _]
          frame False {
            n1494 = call "DATA ENCRYPT STRING FILE WRITE.vi"("error in (no error)"=w2432, "User Action"="User Pressed UnLoad on Service Screen", "main ref"=w2431) -> ("error out"=w2428:errorcluster)  [unwired: 6 in, 1 out]
            n1495 = call "Stall Data Flow.vim"("value in"=w2428, "milliseconds to wait"=u32 2000) -> ("value out"=w2424:errorcluster)  [unwired: 1 out]
            n1496 = call "PID UNLOAD.vi"("error in (no error)"=w2424, "main ref"=w2425) -> ("error out"=w2427:errorcluster)  [unwired: 9 in]
            n1497 = call "HEAVE WRITE FGV.vi"("Enum - Menu"=Heave_Write_enum."WRITE", "error in (no error)"=w2427, "main ref"=w2426) -> ("error out"=w2429:errorcluster)  [unwired: 8 in]
          }
          frame True {
            n1498 = call "DATA ENCRYPT STRING FILE WRITE.vi"("error in (no error)"=w2435, "User Action"="User Pressed Load on Service Screen", "main ref"=w2434) -> ("error out"=w2436:errorcluster)  [unwired: 6 in, 1 out]
          }
        }
      }
      frame "BACK" {
        w2452 = FALSE ("Value")
        n1499 = Unbundle By Name(w2439) -> ("Environmental control.Acoustic Emission 3"=w2447:refnum<vi>)
        n1500 = Unbundle By Name(w2439) -> ("Main Screen.BACK"=w2471:refnum<vi>)
        n1501 = property on="Property Node" class="Bool (strict)"(reference=w2471, "Value"=FALSE) -> (reference out=w2469:refnum<vi>, error out=w2470:errorcluster)  [unwired: 1 in]
        n1502 = property on="Property Node" class="Bool (strict)"(reference=w2447) -> (reference out=w2445:refnum<vi>, error out=w2446:errorcluster, "Value"=w2444:bool)  [unwired: 1 in]
        n1503 = Close Reference(reference=w2469, error in (no error)=w2470) -> ()  [unwired: 1 out]
        n1504 = Close Reference(reference=w2445, error in (no error)=w2446) -> ()  [unwired: 1 out]
        n1505 = case shown="True" w2444 {
          tunnel: w2443 -> [w2472 w2476]
          tunnel: [w2472 w2473] -> w2442
          tunnel: w2439 -> [_ w2474]
          frame False {
          }
          frame True {
            n1506 = call "Acq stop.vi"("error in (no error)"=w2476, "Data Cluster"=w2474) -> ("error out"=w2475:errorcluster)  [unwired: 9 in]
            n1507 = call <vilib>:"Clear Errors.vi"("error in (no error)"=w2475) -> ("error out"=w2473:errorcluster)  [unwired: 5 in, 1 out]
          }
        }
        n1508 = Unbundle By Name(w2439) -> ("Main Home Screen.MainPage"=w2459:refnum<vi>)
        n1509 = Unbundle By Name(w2439) -> ("Main Screen.Start Test"=w2455:refnum<vi>)
        n1510 = Unbundle By Name(w2439) -> ("Main Screen.STOP"=w2454:refnum<vi>)
        n1511 = Unbundle By Name(w2439) -> ("Main Home Screen.GUI"=w2463:refnum<vi>)
        n1512 = property on="Property Node" class="TabCtl (strict)"(reference=w2459, "Value"=T15."HOME") -> (reference out=w2461:refnum<vi>, error out=w2460:errorcluster)  [unwired: 1 in]
        n1513 = property on="Property Node" class="TabCtl (strict)"(reference=w2463, "Value"=T14."Setup") -> (reference out=w2465:refnum<vi>, error out=w2464:errorcluster)  [unwired: 1 in]
        n1514 = property on="Property Node" class="Bool (strict)"(reference=w2455, "Visible"=TRUE ("Value"), "Value"=FALSE) -> (reference out=w2450:refnum<vi>, error out=w2456:errorcluster)  [unwired: 1 in]
        n1515 = property on="Property Node" class="Bool (strict)"(reference=w2454, "Value"=w2452, "Visible"=w2452) -> (reference out=w2449:refnum<vi>, error out=w2453:errorcluster)  [unwired: 1 in]
        n1516 = call "Temperature vi FGV.vi"("Enum"=Temperature_enum."write", "Set Temperature"=0.0, "main ref"=w2439) -> ("error out"=→"error out 5":errorcluster)  [unwired: 8 in]
        n1517 = Close Reference(reference=w2465, error in (no error)=w2464) -> ()  [unwired: 1 out]
        n1518 = Close Reference(reference=w2461, error in (no error)=w2460) -> ()  [unwired: 1 out]
        n1519 = Close Reference(reference=w2450, error in (no error)=w2456) -> ()  [unwired: 1 out]
        n1520 = Close Reference(reference=w2449, error in (no error)=w2453) -> ()  [unwired: 1 out]
        n1521 = call "DATA ENCRYPT STRING FILE WRITE.vi"("error in (no error)"=w2442, "User Action"="User Pressed Back on Main Screen", "main ref"=w2439) -> ("error out"=w2467:errorcluster)  [unwired: 6 in, 1 out]
        n1522 = call "Reinitial Parameter After Test.vi"("error in (no error)"=w2467, "main ref"=w2439) -> ("error out"=w2448:errorcluster)  [unwired: 9 in]
      }
      frame "Start Test" {
        n1523 = Unbundle By Name(w2477) -> ("Environmental control.Acoustic Emission 3"=w2483:refnum<vi>)
        n1524 = property on="Property Node" class="Bool (strict)"(reference=w2483) -> (reference out=w2481:refnum<vi>, error out=w2482:errorcluster, "Value"=w2480:bool)  [unwired: 1 in]
        n1525 = Close Reference(reference=w2481, error in (no error)=w2482) -> ()  [unwired: 1 out]
        n1526 = case shown="True" w2480 {
          tunnel: w2479 -> [w2485 w2489]
          tunnel: [w2485 w2486] -> w2478
          tunnel: w2477 -> [_ w2487]
          frame False {
          }
          frame True {
            n1527 = call "Acq start.vi"("error in (no error)"=w2489, "Data Cluster"=w2487) -> ("error out"=w2488:errorcluster)  [unwired: 9 in]
            n1528 = call <vilib>:"Clear Errors.vi"("error in (no error)"=w2488) -> ("error out"=w2486:errorcluster)  [unwired: 5 in, 1 out]
          }
        }
        n1529 = call "Test Start Sequence.vi"("error in (no error)"=w2478, "Data Cluster"=w2477) -> ("error out"=w2484:errorcluster)  [unwired: 9 in]
      }
      frame "STOP" {
        n1530 = call "Test Stop.vi"("error in (no error)"=w2515, "Data Cluster"=w2491) -> ("error out"=w2490:errorcluster)  [unwired: 9 in]
        n1531 = Unbundle By Name(w2491) -> ("Main Screen.Load En"=w2514:refnum<vi>)
        n1532 = Unbundle By Name(w2491) -> ("Main Screen.CZ FF"=w2509:refnum<vi>)
        n1533 = Unbundle By Name(w2491) -> ("Main Screen.zFF"=w2506:refnum<vi>)
        n1534 = property on="Property Node" class="Bool (strict)"(reference=w2514, "DisabledEnum"=T26."Disabled and Grayed Out" ("Disabled")) -> (reference out=w2502:refnum<vi>, error out=w2513:errorcluster)  [unwired: 1 in]
        n1535 = property on="Property Node" class="Bool (strict)"(reference=w2509, "DisabledEnum"=T26."Disabled and Grayed Out" ("Disabled"), "Value"=FALSE ("Visible")) -> (reference out=w2508:refnum<vi>, error out=w2510:errorcluster)  [unwired: 1 in]
        n1536 = property on="Property Node" class="Bool (strict)"(reference=w2506, "DisabledEnum"=T26."Disabled and Grayed Out" ("Disabled"), "Value"=FALSE ("Visible")) -> (reference out=w2507:refnum<vi>, error out=w2505:errorcluster)  [unwired: 1 in]
        n1537 = local read "tdms file out"() -> (w2495:refnum<k34>)
        n1538 = Close Reference(reference=w2502, error in (no error)=w2513) -> ()  [unwired: 1 out]
        n1539 = Close Reference(reference=w2508, error in (no error)=w2510) -> ()  [unwired: 1 out]
        n1540 = Close Reference(reference=w2507, error in (no error)=w2505) -> ()  [unwired: 1 out]
        n1541 = TDMS Close(11:w2495) -> ()  [unwired: 1 in, 2 out]
        n1542 = Unbundle By Name(w2491) -> ("Environmental control.Acoustic Emission 3"=w2500:refnum<vi>)
        n1543 = call "Temperature vi FGV.vi"("Enum"=Temperature_enum."write", "error in"=w2490, "Set Temperature"=0.0, "main ref"=w2491) -> ("error out"=→"error out 4":errorcluster)  [unwired: 7 in]
        n1544 = property on="Property Node" class="Bool (strict)"(reference=w2500) -> (reference out=w2498:refnum<vi>, error out=w2499:errorcluster, "Value"=w2497:bool)  [unwired: 1 in]
        n1545 = Close Reference(reference=w2498, error in (no error)=w2499) -> ()  [unwired: 1 out]
        n1546 = case shown="False" w2497 {
          tunnel: w2490 -> [w2516 w2520]
          tunnel: [w2516 w2517] -> w2496
          tunnel: w2491 -> [_ w2518]
          frame False {
          }
          frame True {
            n1547 = call "Acq stop.vi"("error in (no error)"=w2520, "Data Cluster"=w2518) -> ("error out"=w2519:errorcluster)  [unwired: 9 in]
            n1548 = call <vilib>:"Clear Errors.vi"("error in (no error)"=w2519) -> ("error out"=w2517:errorcluster)  [unwired: 5 in, 1 out]
          }
        }
      }
      frame "PlaceModule" {
        n1549 = call "Place Module.vi"("error in (no error)"=w2523, "main ref"=w2521) -> ("error out"=w2522:errorcluster)  [unwired: 9 in]
      }
      frame "Stage Homing" {
        n1550 = call "HOMINING.vi"("error in (no error)"=w2526, "main ref"=w2524) -> ("error out"=w2525:errorcluster)  [unwired: 9 in]
      }
      frame "Clear 3" {
        n1551 = Unbundle By Name(w2528) -> ("Loading.Stribeck Table  For loading"=w2538:refnum<vi>)
        n1552 = Unbundle By Name(w2528) -> ("Loading.Clear 3"=w2529:refnum<vi>)
        n1553 = property on="Property Node" class="Bool (strict)"(reference=w2529, "Value"=FALSE) -> (reference out=w2531:refnum<vi>, error out=w2530:errorcluster)  [unwired: 1 in]
        n1554 = call "DATA ENCRYPT STRING FILE WRITE.vi"("error in (no error)"=w2534, "User Action"="User Pressed Clear  on Step Load Sequence", "main ref"=w2528) -> ("error out"=w2533:errorcluster)  [unwired: 6 in, 1 out]
        n1555 = property on="Property Node" class="Tbl (strict)"(reference=w2538, "Value"=string[][] []) -> (reference out=w2536:refnum<vi>, error out=w2537:errorcluster)  [unwired: 1 in]
        n1556 = Close Reference(reference=w2531, error in (no error)=w2530) -> ()  [unwired: 1 out]
        n1557 = Close Reference(reference=w2536, error in (no error)=w2537) -> ()  [unwired: 1 out]
      }
      frame "Set WTD" {
        n1558 = Unbundle By Name(w2539) -> ("Motion Module.Set WTD"=w2542:refnum<vi>)
        n1559 = property on="Property Node" class="Bool (strict)"(reference=w2542, "Value"=FALSE) -> (reference out=w2544:refnum<vi>, error out=w2543:errorcluster)  [unwired: 1 in]
        n1560 = call "DATA ENCRYPT STRING FILE WRITE.vi"("error in (no error)"=w2546, "User Action"="User Pressed  on Set Wear Track", "main ref"=w2539) -> ("error out"=w2545:errorcluster)  [unwired: 6 in, 1 out]
        n1561 = call "Sway wear trac set.vi"("error in (no error)"=w2545, "main ref"=w2539) -> ("error out"=w2540:errorcluster)  [unwired: 9 in]
        n1562 = Close Reference(reference=w2544, error in (no error)=w2543) -> ()  [unwired: 1 out]
      }
      frame "Import 2" {
        n1563 = call "File Dialog"("start path"=path "C:/LAB-IQ 150/User Defined Protocol", "error in"=w2555) -> ("selected path"=w2549:path, "cancelled"=w2552:bool, "error out"=w2554:errorcluster)  [unwired: 10 in, 1 out]
        n1564 = call <vilib>:"Clear Errors.vi"("error in (no error)"=w2554) -> ("error out"=w2551:errorcluster)  [unwired: 5 in, 1 out]
        n1565 = case shown="False" w2552 {
          tunnel: w2551 -> [w2565 w2566]
          tunnel: [w2557 w2566] -> w2550
          tunnel: w2549 -> [w2564 _]
          tunnel: w2548 -> [w2559 _]
          frame False {
            n1566 = call-poly <vilib>:"Read Delimited Spreadsheet.vi"("file path (dialog if empty)"=w2564, "error in (no error)"=w2565, "delimiter (\\t)"=":" ("delimiter (\\t)")) -> ("all rows"=w2556:string[][], "error out"=w2558:errorcluster)  [unwired: 7 in, 4 out]
            n1567 = Unbundle By Name(w2559) -> ("Motion Module.StepTable For Speed"=w2562:refnum<vi>)
            n1568 = property on="Property Node" class="Tbl (strict)"(reference=w2562, error in=w2558, "Value"=w2556) -> (reference out=w2560:refnum<vi>, error out=w2561:errorcluster)
            n1569 = Close Reference(reference=w2560, error in (no error)=w2561) -> (error out=w2557:errorcluster)
          }
          frame True {
          }
        }
      }
      frame "Import 3" {
        n1570 = call "File Dialog7"("start path"=path "C:/LAB-IQ 150/User Defined Protocol", "error in"=w2575) -> ("selected path"=w2569:path, "cancelled"=w2572:bool, "error out"=w2574:errorcluster)  [unwired: 10 in, 1 out]
        n1571 = call <vilib>:"Clear Errors.vi"("error in (no error)"=w2574) -> ("error out"=w2571:errorcluster)  [unwired: 5 in, 1 out]
        n1572 = local write "Import 3"(FALSE ("Import 3")) -> ()
        n1573 = case shown="False" w2572 {
          tunnel: w2571 -> [w2585 w2586]
          tunnel: [w2577 w2586] -> w2570
          tunnel: w2569 -> [w2584 _]
          tunnel: w2568 -> [w2579 _]
          frame False {
            n1574 = call-poly <vilib>:"Read Delimited Spreadsheet.vi"("file path (dialog if empty)"=w2584, "error in (no error)"=w2585, "delimiter (\\t)"=":" ("delimiter (\\t)")) -> ("all rows"=w2576:string[][], "error out"=w2578:errorcluster)  [unwired: 7 in, 4 out]
            n1575 = Unbundle By Name(w2579) -> ("Loading.Stribeck Table  For loading"=w2582:refnum<vi>)
            n1576 = property on="Property Node" class="Tbl (strict)"(reference=w2582, error in=w2578, "Value"=w2576) -> (reference out=w2580:refnum<vi>, error out=w2581:errorcluster)
            n1577 = Close Reference(reference=w2580, error in (no error)=w2581) -> (error out=w2577:errorcluster)
          }
          frame True {
          }
        }
      }
      frame "Save 2" {
        n1578 = Unbundle By Name(w2590) -> ("Motion Module.StepTable For Speed"=w2605:refnum<vi>)
        n1579 = property on="Property Node" class="Tbl (strict)"(reference=w2605) -> (reference out=w2603:refnum<vi>, error out=w2604:errorcluster, "Value"=w2601:string[][])  [unwired: 1 in]
        n1580 = call "File Dialog2"("start path"=path "C:/LAB-IQ 150/User Defined Protocol", "error in"=w2595) -> ("selected path"=w2598:path, "error out"=w2597:errorcluster)  [unwired: 10 in, 2 out]
        n1581 = call <vilib>:"Clear Errors.vi"("error in (no error)"=w2597) -> ("error out"=w2596:errorcluster)  [unwired: 5 in, 1 out]
        n1582 = Close Reference(reference=w2603, error in (no error)=w2604) -> ()  [unwired: 1 out]
        n1583 = call-poly <vilib>:"Write Delimited Spreadsheet.vi"("file path (dialog if empty)"=w2598, "2D data"=w2601, "append to file? (new file:F)"=TRUE, "error in (no error)"=w2596, "delimiter (\\t)"=":" ("delimiter (\\t)")) -> ("error out"=w2594:errorcluster)  [unwired: 9 in, 1 out]
        n1584 = call <vilib>:"Clear Errors.vi"("error in (no error)"=w2594) -> ("error out"=w2589:errorcluster)  [unwired: 5 in, 1 out]
        n1585 = Unbundle By Name(w2590) -> ("Motion Module.Save 2"=w2591:refnum<vi>)
        n1586 = property on="Property Node" class="Bool (strict)"(reference=w2591, error in=w2589, "Value"=FALSE) -> (reference out=w2593:refnum<vi>, error out=w2592:errorcluster)
        n1587 = Close Reference(reference=w2593, error in (no error)=w2592) -> (error out=w2588:errorcluster)
      }
      frame "Save 3" {
        n1588 = Unbundle By Name(w2608) -> ("Loading.Stribeck Table  For loading"=w2620:refnum<vi>)
        n1589 = property on="Property Node" class="Tbl (strict)"(reference=w2620) -> (reference out=w2618:refnum<vi>, error out=w2619:errorcluster, "Value"=w2616:string[][])  [unwired: 1 in]
        n1590 = call "File Dialog8"("start path"=path "C:/LAB-IQ 150/User Defined Protocol", "error in"=w2610) -> ("selected path"=w2613:path, "error out"=w2612:errorcluster)  [unwired: 10 in, 2 out]
        n1591 = call <vilib>:"Clear Errors.vi"("error in (no error)"=w2612) -> ("error out"=w2611:errorcluster)  [unwired: 5 in, 1 out]
        n1592 = Close Reference(reference=w2618, error in (no error)=w2619) -> ()  [unwired: 1 out]
        n1593 = call-poly <vilib>:"Write Delimited Spreadsheet.vi"("file path (dialog if empty)"=w2613, "2D data"=w2616, "append to file? (new file:F)"=TRUE, "error in (no error)"=w2611, "delimiter (\\t)"=":" ("delimiter (\\t)")) -> ("error out"=w2609:errorcluster)  [unwired: 9 in, 1 out]
        n1594 = call <vilib>:"Clear Errors.vi"("error in (no error)"=w2609) -> ("error out"=w2607:errorcluster)  [unwired: 5 in, 1 out]
        n1595 = local write "Save 3"(FALSE ("Value")) -> ()
      }
      frame "Calculate Rotary" {
        n1596 = call "STEP LOAD MM_SEC AND RPM CONVERSION.vi"("error in (no error)"=w2624, "Data Cluster"=w2622) -> ("error out"=w2623:errorcluster)  [unwired: 9 in]
        n1597 = local write "calculate rotary"(FALSE) -> ()
      }
      frame "Clear List" {
        n1598 = Unbundle By Name(w2626) -> ("Environmental control.Sensors Picked"=w2633:refnum<vi>)
        n1599 = Unbundle By Name(w2626) -> ("Environmental control.Clear List"=w2627:refnum<vi>)
        n1600 = property on="Property Node" class="Bool (strict)"(reference=w2627, "Value"=FALSE) -> (reference out=w2629:refnum<vi>, error out=w2628:errorcluster)  [unwired: 1 in]
        n1601 = property on="Property Node" class="Str"(reference=w2633, "Value"="") -> (reference out=w2631:refnum<vi>, error out=w2632:errorcluster)  [unwired: 1 in]
        n1602 = Close Reference(reference=w2629, error in (no error)=w2628) -> ()  [unwired: 1 out]
        n1603 = Close Reference(reference=w2631, error in (no error)=w2632) -> ()  [unwired: 1 out]
      }
      frame "ClrLog" {
        n1604 = Unbundle By Name(w2636) -> ("Main Screen.ClrLog"=w2637:refnum<vi>)
        n1605 = Unbundle By Name(w2636) -> ("Main Screen.Trip Log"=w2643:refnum<vi>)
        n1606 = property on="Property Node" class="Bool (strict)"(reference=w2637, "Value"=FALSE) -> (reference out=w2639:refnum<vi>, error out=w2638:errorcluster)  [unwired: 1 in]
        n1607 = property on="Property Node" class="Str"(reference=w2643, "Value"="") -> (reference out=w2641:refnum<vi>, error out=w2642:errorcluster)  [unwired: 1 in]
        n1608 = Close Reference(reference=w2639, error in (no error)=w2638) -> ()  [unwired: 1 out]
        n1609 = Close Reference(reference=w2641, error in (no error)=w2642) -> ()  [unwired: 1 out]
      }
      frame "Add to list" {
        n1610 = Unbundle By Name(w2645) -> ("Environmental control.Sensors Picked"=w2651:refnum<vi>)
        n1611 = property on="Property Node" class="Str"(reference=w2651, error in=w2646, "Value"="") -> (reference out=w2649:refnum<vi>, error out=w2650:errorcluster)
        n1612 = Close Reference(reference=w2649, error in (no error)=w2650) -> (error out=w2647:errorcluster)
        n1613 = call "Add  to List Loop.vi"("error in (no error)"=w2647, "Data Cluster"=w2645) -> ("error out"=w2653:errorcluster)  [unwired: 9 in]
        n1614 = Unbundle By Name(w2645) -> ("Environmental control.Add to list"=w2655:refnum<vi>)
        n1615 = property on="Property Node" class="Bool (strict)"(reference=w2655, error in=w2653, "Value"=FALSE) -> (reference out=w2657:refnum<vi>, error out=w2656:errorcluster)
        n1616 = Close Reference(reference=w2657, error in (no error)=w2656) -> (error out=w2652:errorcluster)
      }
      frame "Disable Axis Jog Soft Limits" {
        n1617 = call "DATA ENCRYPT STRING FILE WRITE.vi"("error in (no error)"=w2661, "User Action"="User Pressed Disable Axis Jog Soft Limits in Main Screen", "main ref"=w2659) -> ("error out"=w2660:errorcluster)  [unwired: 6 in, 1 out]
      }
      frame "Home Service" {
        n1618 = Unbundle By Name(w2663) -> ("Main Home Screen.MainPage"=w2669:refnum<vi>)
        n1619 = Unbundle By Name(w2663) -> ("Main Home Screen.GUI"=w2667:refnum<vi>)
        n1620 = local write "Home Service"(FALSE ("Home Service")) -> ()
        n1621 = property on="Property Node" class="TabCtl (strict)"(reference=w2669, "Value"=T15."HOME") -> (reference out=w2671:refnum<vi>, error out=w2670:errorcluster)  [unwired: 1 in]
        n1622 = property on="Property Node" class="TabCtl (strict)"(reference=w2667, "Value"=T14."Setup") -> (reference out=w2665:refnum<vi>, error out=w2666:errorcluster)  [unwired: 1 in]
        n1623 = Close Reference(reference=w2671, error in (no error)=w2670) -> ()  [unwired: 1 out]
        n1624 = Close Reference(reference=w2665, error in (no error)=w2666) -> ()  [unwired: 1 out]
        n1625 = call "DATA ENCRYPT STRING FILE WRITE.vi"("error in (no error)"=w2674, "User Action"="User Pressed Home Service from Service Screen", "main ref"=w2663) -> ("error out"=w2673:errorcluster)  [unwired: 6 in, 1 out]
      }
      frame "Analysis Home" {
        n1626 = Unbundle By Name(w2676) -> ("Main Screen.Main Screen Tab"=w2679:refnum<vi>)
        n1627 = Unbundle By Name(w2676) -> ("Main Home Screen.MainPage"=w2686:refnum<vi>)
        n1628 = Unbundle By Name(w2676) -> ("Main Home Screen.GUI"=w2684:refnum<vi>)
        n1629 = local write "Analysis Home new"(FALSE ("Analysis Home new")) -> ()
        n1630 = property on="Property Node" class="TabCtl (strict)"(reference=w2679, "Value"=T18."  Acquire  ") -> (reference out=w2677:refnum<vi>, error out=w2678:errorcluster)  [unwired: 1 in]
        n1631 = property on="Property Node" class="TabCtl (strict)"(reference=w2686, "Value"=T15."HOME") -> (reference out=w2688:refnum<vi>, error out=w2687:errorcluster)  [unwired: 1 in]
        n1632 = property on="Property Node" class="TabCtl (strict)"(reference=w2684, "Value"=T14."Setup") -> (reference out=w2682:refnum<vi>, error out=w2683:errorcluster)  [unwired: 1 in]
        n1633 = Close Reference(reference=w2677, error in (no error)=w2678) -> ()  [unwired: 1 out]
        n1634 = Close Reference(reference=w2688, error in (no error)=w2687) -> ()  [unwired: 1 out]
        n1635 = Close Reference(reference=w2682, error in (no error)=w2683) -> ()  [unwired: 1 out]
        n1636 = call "DATA ENCRYPT STRING FILE WRITE.vi"("error in (no error)"=w2691, "User Action"="User Pressed Home from AnalysisScreen", "main ref"=w2676) -> ("error out"=w2690:errorcluster)  [unwired: 6 in, 1 out]
      }
      frame "Post Analysis" {
        n1637 = Unbundle By Name(w2694) -> ("Main Screen.Main Screen Tab"=w2697:refnum<vi>)
        n1638 = Unbundle By Name(w2694) -> ("Main Home Screen.MainPage"=w2703:refnum<vi>)
        n1639 = Unbundle By Name(w2694) -> ("Main Home Screen.GUI"=w2701:refnum<vi>)
        n1640 = property on="Property Node" class="TabCtl (strict)"(reference=w2697, "Value"=T18."Compare Files Rot") -> (reference out=w2695:refnum<vi>, error out=w2696:errorcluster)  [unwired: 1 in]
        n1641 = property on="Property Node" class="TabCtl (strict)"(reference=w2703, "Value"=T15."HOME") -> (reference out=w2705:refnum<vi>, error out=w2704:errorcluster)  [unwired: 1 in]
        n1642 = property on="Property Node" class="TabCtl (strict)"(reference=w2701, "Value"=T14."Begin") -> (reference out=w2699:refnum<vi>, error out=w2700:errorcluster)  [unwired: 1 in]
        n1643 = local write "Post Analysis"(FALSE ("Post Analysis")) -> ()
        n1644 = Close Reference(reference=w2695, error in (no error)=w2696) -> ()  [unwired: 1 out]
        n1645 = Close Reference(reference=w2705, error in (no error)=w2704) -> ()  [unwired: 1 out]
        n1646 = Close Reference(reference=w2699, error in (no error)=w2700) -> ()  [unwired: 1 out]
        n1647 = call "DATA ENCRYPT STRING FILE WRITE.vi"("error in (no error)"=w2708, "User Action"="User Pressed Post Analysis ", "main ref"=w2694) -> ("error out"=w2707:errorcluster)  [unwired: 6 in, 1 out]
      }
      frame "Edit Gain Constants" {
        n1648 = Unbundle By Name(w2710) -> ("About Screen.Edit Gain Constants"=w2716:refnum<vi>)
        n1649 = Unbundle By Name(w2710) -> ("About Screen.Temp Modbus:"=w2728:refnum<vi>)
        n1650 = Unbundle By Name(w2710) -> ("About Screen.Humidity Port:"=w2727:refnum<vi>)
        n1651 = Unbundle By Name(w2710) -> ("About Screen.Password"=w2722:refnum<vi>)
        n1652 = Unbundle By Name(w2710) -> ("About Screen.ECR Port:"=w2713:refnum<vi>)
        n1653 = property on="Property Node" class="Bool (strict)"(reference=w2716, "Value"=FALSE) -> (reference out=w2717:refnum<vi>, error out=w2715:errorcluster)  [unwired: 1 in]
        n1654 = property on="Property Node" class="VISAName"(reference=w2713, "DisabledEnum"=T26."Enabled" ("Disabled")) -> (reference out=w2709:refnum<vi>, error out=w2712:errorcluster)  [unwired: 1 in]
        n1655 = property on="Property Node" class="VISAName"(reference=w2728, "DisabledEnum"=T26."Enabled" ("Disabled")) -> (reference out=w2718:refnum<vi>, error out=w2729:errorcluster)  [unwired: 1 in]
        n1656 = property on="Property Node" class="VISAName"(reference=w2727, "DisabledEnum"=T26."Enabled" ("Disabled")) -> (reference out=w2725:refnum<vi>, error out=w2726:errorcluster)  [unwired: 1 in]
        n1657 = property on="Property Node" class="Str"(reference=w2722, "Visible"=FALSE) -> (reference out=w2724:refnum<vi>, error out=w2723:errorcluster)  [unwired: 1 in]
        n1658 = Close Reference(reference=w2717, error in (no error)=w2715) -> ()  [unwired: 1 out]
        n1659 = Close Reference(reference=w2724, error in (no error)=w2723) -> ()  [unwired: 1 out]
        n1660 = Close Reference(reference=w2709, error in (no error)=w2712) -> ()  [unwired: 1 out]
        n1661 = Close Reference(reference=w2718, error in (no error)=w2729) -> ()  [unwired: 1 out]
        n1662 = Close Reference(reference=w2725, error in (no error)=w2726) -> ()  [unwired: 1 out]
        n1663 = call "DATA ENCRYPT STRING FILE WRITE.vi"("error in (no error)"=w2732, "User Action"="User Pressed Home Service from Service Screen", "main ref"=w2710) -> ("error out"=w2731:errorcluster)  [unwired: 6 in, 1 out]
      }
      frame "Advanced Setting" {
        n1664 = Unbundle By Name(w2734) -> ("About Screen.Advanced Setting"=w2736:refnum<vi>)
        n1665 = property on="Property Node" class="Bool (strict)"(reference=w2736) -> (reference out=w2737:refnum<vi>, error out=w2735:errorcluster, "Value"=w2733:bool)  [unwired: 1 in]
        n1666 = Close Reference(reference=w2737, error in (no error)=w2735) -> ()  [unwired: 1 out]
        n1667 = case shown="True" w2733 {
          tunnel: w2734 -> [w2742 w2767]
          frame True {
            n1668 = Unbundle By Name(w2742) -> ("About Screen.Heave and Surge COM Port:"=w2764:refnum<vi>)
            n1669 = Unbundle By Name(w2742) -> ("About Screen.Edit Gain Constants"=w2744:refnum<vi>)
            n1670 = Unbundle By Name(w2742) -> ("About Screen.Sway COM Port:"=w2761:refnum<vi>)
            n1671 = Unbundle By Name(w2742) -> ("About Screen.Temp Modbus:"=w2758:refnum<vi>)
            n1672 = Unbundle By Name(w2742) -> ("About Screen.Humidity Port:"=w2757:refnum<vi>)
            n1673 = Unbundle By Name(w2742) -> ("About Screen.Password"=w2752:refnum<vi>)
            n1674 = property on="Property Node" class="Bool (strict)"(reference=w2744, "Value"=FALSE) -> (reference out=w2745:refnum<vi>, error out=w2743:errorcluster)  [unwired: 1 in]
            n1675 = property on="Property Node" class="VISAName"(reference=w2764, "DisabledEnum"=T26."Disabled and Grayed Out" ("Disabled")) -> (reference out=w2765:refnum<vi>, error out=w2763:errorcluster)  [unwired: 1 in]
            n1676 = property on="Property Node" class="VISAName"(reference=w2761, "DisabledEnum"=T26."Disabled and Grayed Out" ("Disabled")) -> (reference out=w2762:refnum<vi>, error out=w2760:errorcluster)  [unwired: 1 in]
            n1677 = property on="Property Node" class="VISAName"(reference=w2758, "DisabledEnum"=T26."Disabled and Grayed Out" ("Disabled")) -> (reference out=w2746:refnum<vi>, error out=w2759:errorcluster)  [unwired: 1 in]
            n1678 = property on="Property Node" class="VISAName"(reference=w2757, "DisabledEnum"=T26."Disabled and Grayed Out" ("Disabled")) -> (reference out=w2755:refnum<vi>, error out=w2756:errorcluster)  [unwired: 1 in]
            n1679 = property on="Property Node" class="Str"(reference=w2752, "Visible"=TRUE) -> (reference out=w2754:refnum<vi>, error out=w2753:errorcluster)  [unwired: 1 in]
            n1680 = Close Reference(reference=w2745, error in (no error)=w2743) -> ()  [unwired: 1 out]
            n1681 = Close Reference(reference=w2765, error in (no error)=w2763) -> ()  [unwired: 1 out]
            n1682 = Close Reference(reference=w2762, error in (no error)=w2760) -> ()  [unwired: 1 out]
            n1683 = Close Reference(reference=w2746, error in (no error)=w2759) -> ()  [unwired: 1 out]
            n1684 = Close Reference(reference=w2755, error in (no error)=w2756) -> ()  [unwired: 1 out]
            n1685 = Close Reference(reference=w2754, error in (no error)=w2753) -> ()  [unwired: 1 out]
          }
          frame False {
            n1686 = Unbundle By Name(w2767) -> ("About Screen.Heave and Surge COM Port:"=w2789:refnum<vi>)
            n1687 = Unbundle By Name(w2767) -> ("About Screen.Edit Gain Constants"=w2769:refnum<vi>)
            n1688 = Unbundle By Name(w2767) -> ("About Screen.Sway COM Port:"=w2786:refnum<vi>)
            n1689 = Unbundle By Name(w2767) -> ("About Screen.Temp Modbus:"=w2783:refnum<vi>)
            n1690 = Unbundle By Name(w2767) -> ("About Screen.Humidity Port:"=w2782:refnum<vi>)
            n1691 = Unbundle By Name(w2767) -> ("About Screen.Password"=w2777:refnum<vi>)
            n1692 = property on="Property Node" class="Bool (strict)"(reference=w2769, "Value"=FALSE) -> (reference out=w2770:refnum<vi>, error out=w2768:errorcluster)  [unwired: 1 in]
            n1693 = property on="Property Node" class="VISAName"(reference=w2789, "DisabledEnum"=T26."Disabled and Grayed Out" ("Disabled")) -> (reference out=w2790:refnum<vi>, error out=w2788:errorcluster)  [unwired: 1 in]
            n1694 = property on="Property Node" class="VISAName"(reference=w2786, "DisabledEnum"=T26."Disabled and Grayed Out" ("Disabled")) -> (reference out=w2787:refnum<vi>, error out=w2785:errorcluster)  [unwired: 1 in]
            n1695 = property on="Property Node" class="VISAName"(reference=w2783, "DisabledEnum"=T26."Disabled and Grayed Out" ("Disabled")) -> (reference out=w2771:refnum<vi>, error out=w2784:errorcluster)  [unwired: 1 in]
            n1696 = property on="Property Node" class="VISAName"(reference=w2782, "DisabledEnum"=T26."Disabled and Grayed Out" ("Disabled")) -> (reference out=w2780:refnum<vi>, error out=w2781:errorcluster)  [unwired: 1 in]
            n1697 = property on="Property Node" class="Str"(reference=w2777, "Visible"=FALSE) -> (reference out=w2779:refnum<vi>, error out=w2778:errorcluster)  [unwired: 1 in]
            n1698 = Close Reference(reference=w2770, error in (no error)=w2768) -> ()  [unwired: 1 out]
            n1699 = Close Reference(reference=w2790, error in (no error)=w2788) -> ()  [unwired: 1 out]
            n1700 = Close Reference(reference=w2787, error in (no error)=w2785) -> ()  [unwired: 1 out]
            n1701 = Close Reference(reference=w2771, error in (no error)=w2784) -> ()  [unwired: 1 out]
            n1702 = Close Reference(reference=w2780, error in (no error)=w2781) -> ()  [unwired: 1 out]
            n1703 = Close Reference(reference=w2779, error in (no error)=w2778) -> ()  [unwired: 1 out]
          }
        }
        n1704 = call "DATA ENCRYPT STRING FILE WRITE.vi"("error in (no error)"=w2740, "User Action"="User Pressed Advance Setting in Service Screen", "main ref"=w2734) -> ("error out"=w2739:errorcluster)  [unwired: 6 in, 1 out]
      }
      frame "Password" {
        n1705 = Unbundle By Name(w2791) -> ("About Screen.Password"=w2797:refnum<vi>)
        n1706 = property on="Property Node" class="Str"(reference=w2797) -> (reference out=w2798:refnum<vi>, error out=w2796:errorcluster, "Value"=w2795:string)  [unwired: 1 in]
        n1707 = call <vilib>:"Trim Whitespace.vi"("string"=w2795) -> ("trimmed string"=w2794:string)  [unwired: 1 in]
        n1708 = Close Reference(reference=w2798, error in (no error)=w2796) -> ()  [unwired: 1 out]
        n1709 = Equal?(x=w2794, y="UT150$") -> (x = y?=w2792:bool)
        n1710 = case shown="True" w2792 {
          tunnel: w2791 -> [_ w2801]
          frame False {
          }
          frame True {
            n1711 = Unbundle By Name(w2801) -> ("Main Screen.Main Screen Tab"=w2803:refnum<vi>)
            n1712 = Unbundle By Name(w2801) -> ("Main Home Screen.GUI"=w2807:refnum<vi>)
            n1713 = Unbundle By Name(w2801) -> ("About Screen.Password"=w2811:refnum<vi>)
            n1714 = property on="Property Node" class="TabCtl (strict)"(reference=w2807, "Value"=T14."Begin") -> (reference out=w2808:refnum<vi>, error out=w2806:errorcluster)  [unwired: 1 in]
            n1715 = property on="Property Node" class="TabCtl (strict)"(reference=w2803, "Value"=T18."Service") -> (reference out=w2802:refnum<vi>, error out=w2804:errorcluster)  [unwired: 1 in]
            n1716 = property on="Property Node" class="Str"(reference=w2811, "Value"="") -> (reference out=w2812:refnum<vi>, error out=w2810:errorcluster)  [unwired: 1 in]
            n1717 = Close Reference(reference=w2812, error in (no error)=w2810) -> ()  [unwired: 1 out]
            n1718 = Close Reference(reference=w2808, error in (no error)=w2806) -> ()  [unwired: 1 out]
            n1719 = Close Reference(reference=w2802, error in (no error)=w2804) -> ()  [unwired: 1 out]
          }
        }
      }
      frame "Service About" {
        n1720 = Unbundle By Name(w2814) -> ("Main Screen.Main Screen Tab"=w2817:refnum<vi>)
        n1721 = Unbundle By Name(w2814) -> ("Main Home Screen.GUI"=w2821:refnum<vi>)
        n1722 = local write "Service About"(FALSE ("Service About")) -> ()
        n1723 = property on="Property Node" class="TabCtl (strict)"(reference=w2821, "Value"=T14."Begin") -> (reference out=w2822:refnum<vi>, error out=w2820:errorcluster)  [unwired: 1 in]
        n1724 = property on="Property Node" class="TabCtl (strict)"(reference=w2817, "Value"=T18."About") -> (reference out=w2816:refnum<vi>, error out=w2818:errorcluster)  [unwired: 1 in]
        n1725 = Close Reference(reference=w2822, error in (no error)=w2820) -> ()  [unwired: 1 out]
        n1726 = Close Reference(reference=w2816, error in (no error)=w2818) -> ()  [unwired: 1 out]
      }
      frame "OPEN 1" {
        n1727 = Unbundle By Name(w2826) -> ("Analysis Screen.File 1 Discription"=w2835:refnum<vi>)
        n1728 = property on="Property Node" class="Str"(reference=w2835, error in=w2833, "Value"="") -> (reference out=w2836:refnum<vi>, error out=w2834:errorcluster)
        n1729 = Close Reference(reference=w2836, error in (no error)=w2834) -> (error out=w2832:errorcluster)
        n1730 = call <vilib>:"Application Directory.vi"() -> ("Application Directory"=w2840:path)
        n1731 = Unbundle By Name(w2826) -> ("Analysis Screen.OPEN 1"=w2828:refnum<vi>)
        n1732 = Build Path(base path=w2840, name or relative path="data") -> (appended path=w2838:path)
        n1733 = property on="Property Node" class="Bool (strict)"(reference=w2828, "Value"=FALSE) -> (reference out=w2829:refnum<vi>, error out=w2827:errorcluster)  [unwired: 1 in]
        n1734 = call "File Dialog3"("start path"=w2838, "error in"=w2832) -> ("selected path"=w2837:path, "cancelled"=w2824:bool, "error out"=w2841:errorcluster)  [unwired: 10 in, 1 out]
        n1735 = case shown="True" w2824 {
          tunnel: w2841 -> [w2855 _]
          tunnel: w2837 -> [w2851 _]
          tunnel: [w2843 _] -> w2830
          tunnel: w2826 -> [w2842 w2857]
          frame False {
            n1736 = Path To String(path=w2851) -> (string=w2850:string)
            n1737 = Unbundle By Name(w2842) -> ("Analysis Screen.File Name 1"=w2853:refnum<vi>)
            n1738 = call <vilib>:"Clear Errors.vi"("error in (no error)"=w2855) -> ("error out"=w2849:errorcluster)  [unwired: 5 in, 1 out]
            n1739 = property on="Property Node" class="Str"(reference=w2853, "Value"=w2850) -> (reference out=w2854:refnum<vi>, error out=w2852:errorcluster)  [unwired: 1 in]
            n1740 = call "INI FILE READ.vi"("error in (no error)"=w2849, "File Path"=w2850) -> ("error out"=w2845:errorcluster, "concatenated string"=w2844:string)  [unwired: 8 in]
            n1741 = Unbundle By Name(w2842) -> ("Analysis Screen.File 1 Discription"=w2847:refnum<vi>)
            n1742 = Close Reference(reference=w2854, error in (no error)=w2852) -> ()  [unwired: 1 out]
            n1743 = property on="Property Node" class="Str"(reference=w2847, error in=w2845, "Value"=w2844) -> (reference out=w2848:refnum<vi>, error out=w2846:errorcluster)
            n1744 = Close Reference(reference=w2848, error in (no error)=w2846) -> (error out=w2843:errorcluster)
          }
          frame True {
            n1745 = Unbundle By Name(w2857) -> ("Analysis Screen.File 1 Discription"=w2859:refnum<vi>)
            n1746 = Unbundle By Name(w2857) -> ("Analysis Screen.File Name 1"=w2863:refnum<vi>)
            n1747 = property on="Property Node" class="Str"(reference=w2859, "Value"="") -> (reference out=w2860:refnum<vi>, error out=w2858:errorcluster)  [unwired: 1 in]
            n1748 = property on="Property Node" class="Str"(reference=w2863, "Value"="") -> (reference out=w2864:refnum<vi>, error out=w2862:errorcluster)  [unwired: 1 in]
            n1749 = Close Reference(reference=w2860, error in (no error)=w2858) -> ()  [unwired: 1 out]
            n1750 = Close Reference(reference=w2864, error in (no error)=w2862) -> ()  [unwired: 1 out]
          }
        }
        n1751 = Close Reference(reference=w2829, error in (no error)=w2827) -> ()  [unwired: 1 out]
      }
      frame "OPEN 2" {
        n1752 = Unbundle By Name(w2867) -> ("Analysis Screen.File 2 Discription"=w2876:refnum<vi>)
        n1753 = property on="Property Node" class="Str"(reference=w2876, error in=w2874, "Value"="") -> (reference out=w2877:refnum<vi>, error out=w2875:errorcluster)
        n1754 = Close Reference(reference=w2877, error in (no error)=w2875) -> (error out=w2873:errorcluster)
        n1755 = call <vilib>:"Application Directory.vi"() -> ("Application Directory"=w2881:path)
        n1756 = Unbundle By Name(w2867) -> ("Analysis Screen.OPEN 2"=w2869:refnum<vi>)
        n1757 = Build Path(base path=w2881, name or relative path="data") -> (appended path=w2879:path)
        n1758 = property on="Property Node" class="Bool (strict)"(reference=w2869, "Value"=FALSE) -> (reference out=w2870:refnum<vi>, error out=w2868:errorcluster)  [unwired: 1 in]
        n1759 = call "File Dialog4"("start path"=w2879, "error in"=w2873) -> ("selected path"=w2878:path, "cancelled"=w2865:bool, "error out"=w2882:errorcluster)  [unwired: 10 in, 1 out]
        n1760 = case shown="True" w2865 {
          tunnel: w2882 -> [w2896 w2898]
          tunnel: w2878 -> [w2892 _]
          tunnel: [w2884 w2897] -> w2871
          tunnel: w2867 -> [w2883 w2900]
          frame False {
            n1761 = Path To String(path=w2892) -> (string=w2891:string)
            n1762 = Unbundle By Name(w2883) -> ("Analysis Screen.File Name 2"=w2894:refnum<vi>)
            n1763 = call <vilib>:"Clear Errors.vi"("error in (no error)"=w2896) -> ("error out"=w2890:errorcluster)  [unwired: 5 in, 1 out]
            n1764 = property on="Property Node" class="Str"(reference=w2894, "Value"=w2891) -> (reference out=w2895:refnum<vi>, error out=w2893:errorcluster)  [unwired: 1 in]
            n1765 = call "INI FILE READ.vi"("error in (no error)"=w2890, "File Path"=w2891) -> ("error out"=w2886:errorcluster, "concatenated string"=w2885:string)  [unwired: 8 in]
            n1766 = Unbundle By Name(w2883) -> ("Analysis Screen.File 2 Discription"=w2888:refnum<vi>)
            n1767 = Close Reference(reference=w2895, error in (no error)=w2893) -> ()  [unwired: 1 out]
            n1768 = property on="Property Node" class="Str"(reference=w2888, error in=w2886, "Value"=w2885) -> (reference out=w2889:refnum<vi>, error out=w2887:errorcluster)
            n1769 = Close Reference(reference=w2889, error in (no error)=w2887) -> (error out=w2884:errorcluster)
          }
          frame True {
            n1770 = Unbundle By Name(w2900) -> ("Analysis Screen.File Name 2"=w2906:refnum<vi>)
            n1771 = Unbundle By Name(w2900) -> ("Analysis Screen.File 2 Discription"=w2902:refnum<vi>)
            n1772 = property on="Property Node" class="Str"(reference=w2906, "Value"="") -> (reference out=w2907:refnum<vi>, error out=w2905:errorcluster)  [unwired: 1 in]
            n1773 = property on="Property Node" class="Str"(reference=w2902, "Value"="") -> (reference out=w2901:refnum<vi>, error out=w2903:errorcluster)  [unwired: 1 in]
            n1774 = call <vilib>:"Clear Errors.vi"("error in (no error)"=w2898) -> ("error out"=w2897:errorcluster)  [unwired: 5 in, 1 out]
            n1775 = Close Reference(reference=w2901, error in (no error)=w2903) -> ()  [unwired: 1 out]
            n1776 = Close Reference(reference=w2907, error in (no error)=w2905) -> ()  [unwired: 1 out]
          }
        }
        n1777 = Close Reference(reference=w2870, error in (no error)=w2868) -> ()  [unwired: 1 out]
      }
      frame "OPEN 3" {
        # "3416\n4017\n4554"
        n1778 = Unbundle By Name(w2910) -> ("Analysis Screen.File 3 Discription"=w2919:refnum<vi>)
        n1779 = property on="Property Node" class="Str"(reference=w2919, error in=w2917, "Value"="") -> (reference out=w2920:refnum<vi>, error out=w2918:errorcluster)
        n1780 = Close Reference(reference=w2920, error in (no error)=w2918) -> (error out=w2916:errorcluster)
        n1781 = call <vilib>:"Application Directory.vi"() -> ("Application Directory"=w2924:path)
        n1782 = Unbundle By Name(w2910) -> ("Analysis Screen.OPEN 3"=w2912:refnum<vi>)
        n1783 = Build Path(base path=w2924, name or relative path="data") -> (appended path=w2922:path)
        n1784 = property on="Property Node" class="Bool (strict)"(reference=w2912, "Value"=FALSE) -> (reference out=w2913:refnum<vi>, error out=w2911:errorcluster)  [unwired: 1 in]
        n1785 = call "File Dialog5"("start path"=w2922, "error in"=w2916) -> ("selected path"=w2921:path, "cancelled"=w2908:bool, "error out"=w2925:errorcluster)  [unwired: 10 in, 1 out]
        n1786 = case shown="True" w2908 {
          tunnel: w2925 -> [w2939 w2941]
          tunnel: w2921 -> [w2935 _]
          tunnel: [w2927 w2940] -> w2914
          tunnel: w2910 -> [w2926 w2943]
          frame False {
            n1787 = Path To String(path=w2935) -> (string=w2934:string)
            n1788 = Unbundle By Name(w2926) -> ("Analysis Screen.File Name 3"=w2937:refnum<vi>)
            n1789 = call <vilib>:"Clear Errors.vi"("error in (no error)"=w2939) -> ("error out"=w2933:errorcluster)  [unwired: 5 in, 1 out]
            n1790 = property on="Property Node" class="Str"(reference=w2937, "Value"=w2934) -> (reference out=w2938:refnum<vi>, error out=w2936:errorcluster)  [unwired: 1 in]
            n1791 = call "INI FILE READ.vi"("error in (no error)"=w2933, "File Path"=w2934) -> ("error out"=w2929:errorcluster, "concatenated string"=w2928:string)  [unwired: 8 in]
            n1792 = Unbundle By Name(w2926) -> ("Analysis Screen.File 3 Discription"=w2931:refnum<vi>)
            n1793 = Close Reference(reference=w2938, error in (no error)=w2936) -> ()  [unwired: 1 out]
            n1794 = property on="Property Node" class="Str"(reference=w2931, error in=w2929, "Value"=w2928) -> (reference out=w2932:refnum<vi>, error out=w2930:errorcluster)
            n1795 = Close Reference(reference=w2932, error in (no error)=w2930) -> (error out=w2927:errorcluster)
          }
          frame True {
            n1796 = Unbundle By Name(w2943) -> ("Analysis Screen.File Name 3"=w2949:refnum<vi>)
            n1797 = Unbundle By Name(w2943) -> ("Analysis Screen.File 3 Discription"=w2945:refnum<vi>)
            n1798 = property on="Property Node" class="Str"(reference=w2949, "Value"="") -> (reference out=w2950:refnum<vi>, error out=w2948:errorcluster)  [unwired: 1 in]
            n1799 = property on="Property Node" class="Str"(reference=w2945, "Value"="") -> (reference out=w2944:refnum<vi>, error out=w2946:errorcluster)  [unwired: 1 in]
            n1800 = Close Reference(reference=w2944, error in (no error)=w2946) -> ()  [unwired: 1 out]
            n1801 = Close Reference(reference=w2950, error in (no error)=w2948) -> ()  [unwired: 1 out]
            n1802 = call <vilib>:"Clear Errors.vi"("error in (no error)"=w2941) -> ("error out"=w2940:errorcluster)  [unwired: 5 in, 1 out]
          }
        }
        n1803 = Close Reference(reference=w2913, error in (no error)=w2911) -> ()  [unwired: 1 out]
      }
      frame "OPEN 4" {
        n1804 = Unbundle By Name(w2953) -> ("Analysis Screen.File 4 Discription"=w2962:refnum<vi>)
        n1805 = property on="Property Node" class="Str"(reference=w2962, error in=w2960, "Value"="") -> (reference out=w2963:refnum<vi>, error out=w2961:errorcluster)
        n1806 = Close Reference(reference=w2963, error in (no error)=w2961) -> (error out=w2959:errorcluster)
        n1807 = call <vilib>:"Application Directory.vi"() -> ("Application Directory"=w2967:path)
        n1808 = Unbundle By Name(w2953) -> ("Analysis Screen.OPEN 4"=w2955:refnum<vi>)
        n1809 = Build Path(base path=w2967, name or relative path="data") -> (appended path=w2965:path)
        n1810 = property on="Property Node" class="Bool (strict)"(reference=w2955, "Value"=FALSE) -> (reference out=w2956:refnum<vi>, error out=w2954:errorcluster)  [unwired: 1 in]
        n1811 = call "File Dialog6"("start path"=w2965, "error in"=w2959) -> ("selected path"=w2964:path, "cancelled"=w2951:bool, "error out"=w2968:errorcluster)  [unwired: 10 in, 1 out]
        n1812 = case shown="True" w2951 {
          tunnel: w2968 -> [w2982 w2984]
          tunnel: w2964 -> [w2978 _]
          tunnel: [w2970 w2983] -> w2957
          tunnel: w2953 -> [w2969 w2986]
          frame False {
            n1813 = Path To String(path=w2978) -> (string=w2977:string)
            n1814 = Unbundle By Name(w2969) -> ("Analysis Screen.File Name 4"=w2980:refnum<vi>)
            n1815 = call <vilib>:"Clear Errors.vi"("error in (no error)"=w2982) -> ("error out"=w2976:errorcluster)  [unwired: 5 in, 1 out]
            n1816 = property on="Property Node" class="Str"(reference=w2980, "Value"=w2977) -> (reference out=w2981:refnum<vi>, error out=w2979:errorcluster)  [unwired: 1 in]
            n1817 = call "INI FILE READ.vi"("error in (no error)"=w2976, "File Path"=w2977) -> ("error out"=w2972:errorcluster, "concatenated string"=w2971:string)  [unwired: 8 in]
            n1818 = Unbundle By Name(w2969) -> ("Analysis Screen.File 4 Discription"=w2974:refnum<vi>)
            n1819 = Close Reference(reference=w2981, error in (no error)=w2979) -> ()  [unwired: 1 out]
            n1820 = property on="Property Node" class="Str"(reference=w2974, error in=w2972, "Value"=w2971) -> (reference out=w2975:refnum<vi>, error out=w2973:errorcluster)
            n1821 = Close Reference(reference=w2975, error in (no error)=w2973) -> (error out=w2970:errorcluster)
          }
          frame True {
            n1822 = Unbundle By Name(w2986) -> ("Analysis Screen.File Name 4"=w2992:refnum<vi>)
            n1823 = Unbundle By Name(w2986) -> ("Analysis Screen.File 4 Discription"=w2988:refnum<vi>)
            n1824 = property on="Property Node" class="Str"(reference=w2992, "Value"="") -> (reference out=w2993:refnum<vi>, error out=w2991:errorcluster)  [unwired: 1 in]
            n1825 = property on="Property Node" class="Str"(reference=w2988, "Value"="") -> (reference out=w2987:refnum<vi>, error out=w2989:errorcluster)  [unwired: 1 in]
            n1826 = Close Reference(reference=w2987, error in (no error)=w2989) -> ()  [unwired: 1 out]
            n1827 = Close Reference(reference=w2993, error in (no error)=w2991) -> ()  [unwired: 1 out]
            n1828 = call <vilib>:"Clear Errors.vi"("error in (no error)"=w2984) -> ("error out"=w2983:errorcluster)  [unwired: 5 in, 1 out]
          }
        }
        n1829 = Close Reference(reference=w2956, error in (no error)=w2954) -> ()  [unwired: 1 out]
      }
      frame "Refresh 2" {
        n1830 = call "Data Log Refresh.vi"("error in (no error)"=w2996, "Data Cluster"=w2995) -> ("error out"=w2997:errorcluster)  [unwired: 9 in]
        n1831 = local write "Refresh 2"(FALSE ("Refresh 2")) -> ()
      }
      frame "Scratch Mode" {
        n1832 = Unbundle By Name(w2998) -> ("Motion Module.Scratch Mode"=w3001:refnum<vi>)
        n1833 = property on="Property Node" class="Ring (strict)"(reference=w3001) -> (reference out=w3002:refnum<vi>, error out=w3000:errorcluster, "Value"=w2999:u16)  [unwired: 1 in]
        n1834 = Close Reference(reference=w3002, error in (no error)=w3000) -> ()  [unwired: 1 out]
        n1835 = case shown="2" w2999 {
          tunnel: w2998 -> [w3005 w3009]
          frame 0, Default {
            n1836 = Unbundle By Name(w3005) -> ("Motion Module.No of Scratch"=w3007:refnum<vi>)
            n1837 = property on="Property Node" class="DigNum (strict)"(reference=w3007, "Visible"=FALSE) -> (reference out=w3008:refnum<vi>, error out=w3006:errorcluster)  [unwired: 1 in]
            n1838 = Close Reference(reference=w3008, error in (no error)=w3006) -> ()  [unwired: 1 out]
          }
          frame 2 {
            n1839 = Unbundle By Name(w3009) -> ("Motion Module.No of Scratch"=w3012:refnum<vi>)
            n1840 = property on="Property Node" class="DigNum (strict)"(reference=w3012, "Visible"=TRUE) -> (reference out=w3013:refnum<vi>, error out=w3011:errorcluster)  [unwired: 1 in]
            n1841 = Close Reference(reference=w3013, error in (no error)=w3011) -> ()  [unwired: 1 out]
          }
        }
      }
      frame "Export" {
        n1842 = call "Export file.vi"("error in (no error)"=w3022, "Data Cluster"=w3015) -> ("error out"=w3017:errorcluster)  [unwired: 9 in]
        n1843 = call "DATA ENCRYPT STRING FILE WRITE.vi"("error in (no error)"=w3017, "User Action"="User Pressed  Export ", "main ref"=w3015) -> ("error out"=w3016:errorcluster)  [unwired: 6 in, 1 out]
        n1844 = Unbundle By Name(w3015) -> ("Analysis Screen.Export"=w3020:refnum<vi>)
        n1845 = property on="Property Node" class="Bool (strict)"(reference=w3020, "Value"=FALSE) -> (reference out=w3021:refnum<vi>, error out=w3019:errorcluster)  [unwired: 1 in]
        n1846 = Close Reference(reference=w3021, error in (no error)=w3019) -> ()  [unwired: 1 out]
      }
      frame "Traction Receipe Update Details" {
        n1847 = call "Traction Receipe Main.vi"("error in (no error)"=w3028, "main ref"=w3025) -> ("error out"=w3027:errorcluster)  [unwired: 9 in]
        n1848 = local write "Traction Receipe Update Details"(FALSE ("Traction Step Update Details")) -> ()
        n1849 = call "DATA ENCRYPT STRING FILE WRITE.vi"("error in (no error)"=w3027, "User Action"="User Pressed  Traction Update Details ", "main ref"=w3025) -> ("error out"=w3026:errorcluster)  [unwired: 6 in, 1 out]
      }
      frame "Acoustic Emission 3" {
        n1850 = Unbundle By Name(w3030) -> ("Environmental control.Acoustic Emission 3"=w3033:refnum<vi>)
        n1851 = property on="Property Node" class="Bool (strict)"(reference=w3033) -> (reference out=w3031:refnum<vi>, error out=w3032:errorcluster, "Value"=w3029:bool)  [unwired: 1 in]
        n1852 = Close Reference(reference=w3031, error in (no error)=w3032) -> ()  [unwired: 1 out]
        n1853 = case shown="True" w3029 {
          tunnel: w3030 -> [w3037 w3042]
          frame True {
            n1854 = Unbundle By Name(w3037) -> ("Acquostic.Gains"=w3039:refnum<vi>)
            n1855 = property class="RadioBtnsControl (strict)"(reference=w3039, "Visible"=TRUE) -> (reference out=w3041:refnum<vi>, error out=w3040:errorcluster)  [unwired: 1 in]
            n1856 = Close Reference(reference=w3041, error in (no error)=w3040) -> ()  [unwired: 1 out]
          }
          frame False {
            n1857 = Unbundle By Name(w3042) -> ("Acquostic.Gains"=w3044:refnum<vi>)
            n1858 = property class="RadioBtnsControl (strict)"(reference=w3044, "Visible"=FALSE) -> (reference out=w3046:refnum<vi>, error out=w3045:errorcluster)  [unwired: 1 in]
            n1859 = Close Reference(reference=w3046, error in (no error)=w3045) -> ()  [unwired: 1 out]
          }
        }
        n1860 = call "DATA ENCRYPT STRING FILE WRITE.vi"("error in (no error)"=w3036, "User Action"="User Pressed  on  Acuostic in Environmental Screen", "main ref"=w3030) -> ("error out"=w3035:errorcluster)  [unwired: 6 in, 1 out]
      }
      frame "Info" {
        n1861 = call "ABOUT SCREEN Unitest.vi"("error in (no error)"=w3048) -> ("error out"=w3047:errorcluster)  [unwired: 10 in]
        n1862 = Unbundle By Name(w3053) -> ("ABOUT.Info"=w3050:refnum<vi>)
        n1863 = property class="Bool (strict)"(reference=w3050, "Value"=FALSE ("Visible")) -> (reference out=w3052:refnum<vi>, error out=w3051:errorcluster)  [unwired: 1 in]
        n1864 = Close Reference(reference=w3052, error in (no error)=w3051) -> ()  [unwired: 1 out]
        n1865 = call "DATA ENCRYPT STRING FILE WRITE.vi"("error in (no error)"=w3047, "User Action"="User Pressed  on  About Button", "main ref"=w3053) -> ("error out"=w3055:errorcluster)  [unwired: 6 in, 1 out]
      }
      frame "Clear rot" {
        n1866 = property on="StepTable For Speed 3" class="Tbl (strict)"("Value"=string[][] [["", "", ""], ["", "", ""], ["", "", ""], ["", "", ""]] ("StepTable For Speed 3")) -> ()  [unwired: 2 in, 2 out]
        n1867 = property on="StepTable For Speed" class="Tbl (strict)"("Value"=string[][] [] ("StepTable For Speed")) -> ()  [unwired: 2 in, 2 out]
        n1868 = local write "Clear rot"(FALSE ("Clear rot")) -> ()
        n1869 = call "DATA ENCRYPT STRING FILE WRITE.vi"("error in (no error)"=w3059, "User Action"="User Pressed  on  Clear  Button", "main ref"=w3060) -> ("error out"=w3062:errorcluster)  [unwired: 6 in, 1 out]
      }
      frame "Report" {
        n1870 = call "REPORT GENERATION FOR PYTHON.vi"("error in (no error)"=w3068, "main ref"=w3065) -> ("error out"=w3067:errorcluster)  [unwired: 9 in]
        n1871 = local write "Report"(FALSE ("Report")) -> ()
        n1872 = call "DATA ENCRYPT STRING FILE WRITE.vi"("error in (no error)"=w3067, "User Action"="User Pressed Report ", "main ref"=w3065) -> ("error out"=w3066:errorcluster)  [unwired: 6 in, 1 out]
      }
      frame "Load Disable Trip" {
        n1873 = call "DATA ENCRYPT STRING FILE WRITE.vi"("error in (no error)"=w3072, "User Action"="User Pressed On Load Disable Trip", "main ref"=w3070) -> ("error out"=w3071:errorcluster)  [unwired: 6 in, 1 out]
      }
      frame "COF Disable Trip" {
        n1874 = call "DATA ENCRYPT STRING FILE WRITE.vi"("error in (no error)"=w3076, "User Action"="User Pressed On COF Disable Trip", "main ref"=w3074) -> ("error out"=w3075:errorcluster)  [unwired: 6 in, 1 out]
      }
      frame "Depth Trip 2" {
        n1875 = call "DATA ENCRYPT STRING FILE WRITE.vi"("error in (no error)"=w3080, "User Action"="User Pressed On Depth Trip", "main ref"=w3078) -> ("error out"=w3079:errorcluster)  [unwired: 6 in, 1 out]
      }
      frame "zNL 2" {
        n1876 = call "DATA ENCRYPT STRING FILE WRITE.vi"("error in (no error)"=w3084, "User Action"="User Pressed On Tare Load cell value on Main Screen", "main ref"=w3082) -> ("error out"=w3083:errorcluster)  [unwired: 6 in, 1 out]
      }
      frame "High Temp" {
        n1877 = Unbundle By Name(w3089) -> ("Environmental control.High Temp"=w3095:refnum<vi>)
        n1878 = property on="Property Node" class="Bool (strict)"(reference=w3095) -> (reference out=w3093:refnum<vi>, error out=w3094:errorcluster, "Value"=w3088:bool)  [unwired: 1 in]
        n1879 = Close Reference(reference=w3093, error in (no error)=w3094) -> ()  [unwired: 1 out]
        n1880 = Unbundle By Name(w3089) -> ("Environmental control.Enter the Stage \nTemperature (°C):"=w3090:refnum<vi>)
        n1881 = Select(t=TRUE, s=w3088, f=FALSE) -> (s? t:f=w3085:bool)
        n1882 = property on="Property Node" class="DigNum (strict)"(reference=w3090, "Visible"=w3085) -> (reference out=w3092:refnum<vi>, error out=w3091:errorcluster)  [unwired: 1 in]
        n1883 = Close Reference(reference=w3092, error in (no error)=w3091) -> ()  [unwired: 1 out]
        n1884 = call "DATA ENCRYPT STRING FILE WRITE.vi"("error in (no error)"=w3098, "User Action"="User Pressed On High Temperature Module", "main ref"=w3089) -> ("error out"=w3097:errorcluster)  [unwired: 6 in, 1 out]
      }
      frame "Heater" {
        n1885 = Unbundle By Name(w3101) -> ("Main Screen.Heater"=w3104:refnum<vi>)
        n1886 = property on="Property Node" class="Bool (strict)"(reference=w3104) -> (reference out=w3102:refnum<vi>, error out=w3103:errorcluster, "Value"=w3100:bool)  [unwired: 1 in]
        n1887 = local read "SetTmp"() -> (w3099:dbl)
        n1888 = Close Reference(reference=w3102, error in (no error)=w3103) -> ()  [unwired: 1 out]
        n1889 = case shown="False" w3100 {
          tunnel: w3101 -> [w3110 w3113]
          tunnel: w3099 -> [_ w3112]
          frame False {
            n1890 = call "Temperature vi FGV.vi"("Enum"=Temperature_enum."write", "Set Temperature"=0.0, "main ref"=w3110) -> ("error out"=→"error out 6":errorcluster)  [unwired: 8 in]
          }
          frame True {
            n1891 = call "Temperature vi FGV.vi"("Enum"=Temperature_enum."write", "Set Temperature"=w3112, "main ref"=w3113) -> ()  [unwired: 8 in, 1 out]
          }
        }
        n1892 = call "DATA ENCRYPT STRING FILE WRITE.vi"("error in (no error)"=w3107, "User Action"="User Pressed On High Temperature Module", "main ref"=w3101) -> ("error out"=w3106:errorcluster)  [unwired: 6 in, 1 out]
      }
      frame "Error" {
        # "#CodeRecommended - If you ever change the name of this \"Error\" message, you'll need to update the name in the Check Loop Error.vi as well."
        # "#CodeRecommended - Consider creating a system for logging errors in some way. These errors are for notification purposes only. Handling of specific errors should be performed in the message frames that generated the error."
        # "Error - Display an error dialog. This message is sent by the \"Error Handler\" VIs at the end of other loops in this application."
        n1893 = Merge Errors(w3115) -> (w3116:errorcluster)
      }
      frame "Confirm Quit" {
        # "#CodeNeeded - If you want to provide an \"Are you sure\" dialog (or some other notification) before the application exits, place that code here. This message is typically sent from a Panel Close? event."
        # "Confirm Quit - Message that can confirm whether or not the user wants to exit the application."
        n1894 = call-poly "Enqueue Message.vi"("Priority Message? (F)"=TRUE, "error in (no error)"=w3124, "Message"="Exit", "Message Queue"=w3121) -> ("error out"=w3122:errorcluster)  [unwired: 6 in, 1 out]
        n1895 = Merge Errors(w3122) -> (w3123:errorcluster)
      }
      frame "Exit" {
        # "Stop the VI"
        # "Release the message queue reference"
        # "#CodeNeeded - Add any required cleanup code here. Note that if 'Exit' was called as a result of an error, an error dialog will be displayed. Add any custom error handling for an 'Exit' condition here as well."
        # "Exit - Exit the application."
        n1896 = call "Fire User Event - Stop.vi"("User Event - Stop"=w3127) -> ("error out"=w3126:errorcluster)  [unwired: 10 in]
        n1897 = Release Queue(queue=w3132, error in (no error)=w3125) -> (error out=w3129:errorcluster)  [unwired: 1 in, 2 out]
        n1898 = Merge Errors(w3126, w3129) -> (w3128:errorcluster)
      }
      frame Default {
        # "'Default' case only runs if there is a message that isn't defined in any of the other cases.  Output a programming error."
        n1899 = xnode ("Error Ring")("parameter 0"=w3133) -> ("error out"=w3134:errorcluster)
      }
    }
    n1900 = call "LAB-IQ Error Handler - Message Handling Loop.vi"("error in (no error)"=w1618, "Message Queue"=w1620) -> ("dup error in"=w1619:errorcluster)  [unwired: 8 in, 1 out]
  }
  n1901 = while "Timed Loop" {
    shift-right: [w3154] -> _
    shift-left: w47 -> [w3155]
    tunnel: [w3148] -> w70
    tunnel: w15 -> [w3143]
    tunnel: w18 -> [w3146]
    tunnel: w48 -> [w3145]
    stop <- w3153 stop-if-true
    # "Load  Handling Loop"
    n1902 = call "Dequeue Message.vi"("error in (no error)"=w3146, "Message Queue"=w3143) -> ("error out"=w3152:errorcluster, "output data"=w3150:dbl[][], "Message"=w3151:string, "dup Message Queue"=w3149:refnum<queue>)  [unwired: 6 in]
    n1903 = case "Message Cases" shown="\"Load Main\"" w3151 {
      selector: w3151 -> [_ _ _ _ _ w3202]
      tunnel: w3149 -> [w3159 w3170 _ w3191 w3201 _]
      tunnel: w3152 -> [w3158 w3168 w3180 w3193 w3195 _]
      tunnel: [w3161 w3171 w3181 w3186 w3197 w3203] -> w3147
      tunnel: w3155 -> [w3157 w3163 w3182 w3183 w3200 w3204]
      tunnel: [w3157 w3163 w3182 w3183 w3200 w3204] -> w3154
      tunnel: [_ _ _ _ TRUE _] -> w3153
      tunnel: w3150 -> [_ _ _ _ _ _]
      tunnel: w3145 -> [_ _ _ _ w3194 _]
      frame "init" {
        # "Bundle control references and a sample string value."
        # "Initialize - All initialization work should take place in this message, since other loops can potentially enqueue messages that execute immediately after this one."
        n1904 = call "SET LOAD PARAMETERS.vi"("error in (no error)"=w3158, "main ref"=w3157) -> ("error out"=w3156:errorcluster)  [unwired: 9 in]
        n1905 = call-poly "Enqueue Message.vi"("error in (no error)"=w3156, "Message"="Load Main", "Message Queue"=w3159) -> ("error out"=w3161:errorcluster)  [unwired: 7 in, 1 out]
      }
      frame "Load Main" {
        n1906 = call "LOAD CELL READ.vi"("error in (no error)"=w3168, "main ref"=w3163) -> ("error out"=w3164:errorcluster)  [unwired: 9 in]
        n1907 = call <vilib>:"Clear Errors.vi"("error in (no error)"=w3164) -> ("error out"=w3162:errorcluster)  [unwired: 5 in, 1 out]
        n1908 = Unbundle By Name(w3163) -> ("Main Home Screen.EXIT"=w3169:refnum<vi>)
        n1909 = property on="Property Node" class="Bool (strict)"(reference=w3169) -> (reference out=w3166:refnum<vi>, error out=w3167:errorcluster, "Value"=w3165:bool)  [unwired: 1 in]
        n1910 = Close Reference(reference=w3166, error in (no error)=w3167) -> ()  [unwired: 1 out]
        n1911 = case shown="False" w3165 {
          tunnel: [w3174 w3178] -> w3171
          tunnel: w3170 -> [w3173 w3177]
          tunnel: w3162 -> [w3172 w3176]
          frame True {
            n1912 = call-poly "Enqueue Message.vi"("error in (no error)"=w3172, "Message"="Confirm Quit", "Message Queue"=w3173) -> ("error out"=w3174:errorcluster)  [unwired: 7 in, 1 out]
          }
          frame False {
            n1913 = call-poly "Enqueue Message.vi"("error in (no error)"=w3176, "Message"="Load Main", "Message Queue"=w3177) -> ("error out"=w3178:errorcluster)  [unwired: 7 in, 1 out]
          }
        }
      }
      frame "Error" {
        # "#CodeRecommended - If you ever change the name of this \"Error\" message, you'll need to update the name in the Check Loop Error.vi as well."
        # "#CodeRecommended - Consider creating a system for logging errors in some way. These errors are for notification purposes only. Handling of specific errors should be performed in the message frames that generated the error."
        # "Error - Display an error dialog. This message is sent by the \"Error Handler\" VIs at the end of other loops in this application."
        n1914 = Merge Errors(w3180) -> (w3181:errorcluster)
      }
      frame "Confirm Quit" {
        # "#CodeNeeded - If you want to provide an \"Are you sure\" dialog (or some other notification) before the application exits, place that code here. This message is typically sent from a Panel Close? event."
        # "Confirm Quit - Message that can confirm whether or not the user wants to exit the application."
        n1915 = call-poly "Enqueue Message.vi"("Priority Message? (F)"=TRUE, "error in (no error)"=w3193, "Message"="Exit", "Message Queue"=w3191) -> ("error out"=w3192:errorcluster)  [unwired: 6 in, 1 out]
        n1916 = Merge Errors(w3192) -> (w3188:errorcluster)
        n1917 = call <vilib>:"Clear Errors.vi"("error in (no error)"=w3188) -> ("error out"=w3187:errorcluster)  [unwired: 5 in, 1 out]
        n1918 = call "NEW Load Cell FGV.vi"("Enum - Menu"=Load_cell_Enum."close", "error in (no error)"=w3187, "main ref"=w3183) -> ("error out"=w3185:errorcluster)  [unwired: 6 in, 2 out]
        n1919 = call <vilib>:"Clear Errors.vi"("error in (no error)"=w3185) -> ("error out"=w3186:errorcluster)  [unwired: 5 in, 1 out]
      }
      frame "Exit" {
        # "Stop the VI"
        # "Release the message queue reference"
        # "#CodeNeeded - Add any required cleanup code here. Note that if 'Exit' was called as a result of an error, an error dialog will be displayed. Add any custom error handling for an 'Exit' condition here as well."
        # "Exit - Exit the application."
        n1920 = call "Fire User Event - Stop.vi"("User Event - Stop"=w3194) -> ("error out"=w3196:errorcluster)  [unwired: 10 in]
        n1921 = Release Queue(queue=w3201, error in (no error)=w3195) -> (error out=w3198:errorcluster)  [unwired: 1 in, 2 out]
        n1922 = Merge Errors(w3196, w3198) -> (w3197:errorcluster)
      }
      frame Default {
        # "'Default' case only runs if there is a message that isn't defined in any of the other cases.  Output a programming error."
        n1923 = xnode ("Error Ring")("parameter 0"=w3202) -> ("error out"=w3203:errorcluster)
      }
    }
    n1924 = call "LAB-IQ Error Handler - Message Handling Loop.vi"("error in (no error)"=w3147, "Message Queue"=w3149) -> ("dup error in"=w3148:errorcluster)  [unwired: 8 in, 1 out]
    n1925 = Wait (ms)(milliseconds to wait=u32 20) -> ()  [unwired: 1 out]
  }
  n1926 = while "Timed Loop" {
    shift-right: [w3213] -> _
    shift-left: w47 -> [w3223]
    tunnel: [w3217] -> w69
    tunnel: w13 -> [w3212]
    tunnel: w18 -> [w3215]
    tunnel: w48 -> [w3214]
    stop <- w3222 stop-if-true
    # "Sway Motor  Handling Loop"
    n1927 = call "Dequeue Message.vi"("error in (no error)"=w3215, "Message Queue"=w3212) -> ("error out"=w3221:errorcluster, "output data"=w3219:dbl[][], "Message"=w3220:string, "dup Message Queue"=w3218:refnum<queue>)  [unwired: 6 in]
    n1928 = case "Message Cases" shown="\"Sway Main\"" w3220 {
      selector: w3220 -> [_ _ _ _ _ w3303]
      tunnel: w3218 -> [w3235 w3264 _ w3290 w3302 _]
      tunnel: w3221 -> [w3237 w3247 w3285 w3294 w3296 _]
      tunnel: [w3238 w3265 w3286 w3292 w3298 w3304] -> w3216
      tunnel: w3223 -> [w3225 w3242 w3287 w3293 w3301 w3305]
      tunnel: [w3225 w3242 w3287 w3293 w3301 w3305] -> w3213
      tunnel: [_ _ _ _ TRUE _] -> w3222
      tunnel: w3219 -> [_ _ _ _ _ _]
      tunnel: w3214 -> [_ _ _ _ w3295 _]
      frame "init" {
        # "Initialize - All initialization work should take place in this message, since other loops can potentially enqueue messages that execute immediately after this one."
        n1929 = call "SWAY WRITE FGV.vi"("Enum - Menu"=Sway_Write_enum."INIT", "error in (no error)"=w3237, "main ref"=w3225) -> ("error out"=w3234:errorcluster)  [unwired: 8 in]
        n1930 = call <vilib>:"Clear Errors.vi"("error in (no error)"=w3234) -> ("error out"=w3228:errorcluster)  [unwired: 5 in, 1 out]
        n1931 = call "Stall Data Flow.vim"("value in"=w3228, "milliseconds to wait"=u32 1000) -> ("value out"=w3232:errorcluster)  [unwired: 1 out]
        n1932 = call "Sway Init.vi"("error in (no error)"=w3232, "main ref"=w3225) -> ("error out"=w3229:errorcluster)  [unwired: 9 in]
        n1933 = call <vilib>:"Clear Errors.vi"("error in (no error)"=w3229) -> ("error out"=w3227:errorcluster)  [unwired: 5 in, 1 out]
        n1934 = call "SWAY READ FGV.vi"("Enum - Menu"=Sway_Right_enum."INIT", "error in (no error)"=w3227, "main ref"=w3225) -> ("error out"=w3226:errorcluster)  [unwired: 7 in, 1 out]
        n1935 = call <vilib>:"Clear Errors.vi"("error in (no error)"=w3226) -> ("error out"=w3230:errorcluster)  [unwired: 5 in, 1 out]
        n1936 = call-poly "Enqueue Message.vi"("error in (no error)"=w3230, "Message"="Sway Main", "Message Queue"=w3235) -> ("error out"=w3238:errorcluster)  [unwired: 7 in, 1 out]
      }
      frame "Sway Main" {
        n1937 = Unbundle By Name(w3242) -> ("Heave AND Surge.Homed"=w3250:refnum<vi>)
        n1938 = Unbundle By Name(w3242) -> ("SWAY.Read SWAY Temp"=w3259:refnum<vi>)
        n1939 = local read "HEAVE ENABLE"() -> (w3254:bool)
        n1940 = property on="Property Node" class="DigNum (strict)"(reference=w3250) -> (reference out=w3252:refnum<vi>, error out=w3251:errorcluster, "Value"=w3241:u8)  [unwired: 1 in]
        n1941 = property on="Property Node" class="Bool (strict)"(reference=w3259) -> (reference out=w3257:refnum<vi>, error out=w3258:errorcluster, "Value"=w3256:bool)  [unwired: 1 in]
        n1942 = Equal?(x=w3254, y=TRUE) -> (x = y?=w3249:bool)
        n1943 = Close Reference(reference=w3252, error in (no error)=w3251) -> ()  [unwired: 1 out]
        n1944 = Equal?(x=w3241, y=u8 1 ("Value")) -> (x = y?=w3239:bool)
        n1945 = Close Reference(reference=w3257, error in (no error)=w3258) -> ()  [unwired: 1 out]
        n1946 = And(x=w3249, y=w3239) -> (x .and. y?=w3248:bool)
        n1947 = case shown="True" w3256 {
          tunnel: w3247 -> [w3272 w3276]
          tunnel: [w3272 w3275] -> w3244
          tunnel: w3242 -> [_ w3274]
          frame False {
          }
          frame True {
            n1948 = call "SWAY READ FGV.vi"("Enum - Menu"=Sway_Right_enum."READ", "error in (no error)"=w3276, "main ref"=w3274) -> ("error out"=w3275:errorcluster)  [unwired: 7 in, 1 out]
          }
        }
        n1949 = case shown="True" w3248 {
          tunnel: w3242 -> [_ w3271]
          tunnel: w3247 -> [w3266 w3270]
          tunnel: [w3266 w3267] -> w3245
          frame False {
          }
          frame True {
            n1950 = call "SWAY HOME.vi"("error in (no error)"=w3270, "Data Cluster"=w3271) -> ("error out"=w3268:errorcluster)  [unwired: 9 in]
            n1951 = local write "HEAVE ENABLE"(FALSE ("HEAVE ENABLE")) -> ()
            n1952 = call <vilib>:"Clear Errors.vi"("error in (no error)"=w3268) -> ("error out"=w3267:errorcluster)  [unwired: 5 in, 1 out]
          }
        }
        n1953 = call "Sway Reinitize.vi"("error in (no error)"=w3244, "Data Cluster"=w3242) -> ("error out"=w3243:errorcluster)  [unwired: 9 in]
        n1954 = Unbundle By Name(w3242) -> ("Main Home Screen.EXIT"=w3263:refnum<vi>)
        n1955 = property on="Property Node" class="Bool (strict)"(reference=w3263) -> (reference out=w3261:refnum<vi>, error out=w3262:errorcluster, "Value"=w3260:bool)  [unwired: 1 in]
        n1956 = call <vilib>:"Clear Errors.vi"("error in (no error)"=w3243) -> ("error out"=w3255:errorcluster)  [unwired: 5 in, 1 out]
        n1957 = Merge Errors(w3255, w3245) -> (w3246:errorcluster)
        n1958 = Close Reference(reference=w3261, error in (no error)=w3262) -> ()  [unwired: 1 out]
        n1959 = case shown="False" w3260 {
          tunnel: [w3279 w3283] -> w3265
          tunnel: w3264 -> [w3278 w3282]
          tunnel: w3246 -> [w3277 w3281]
          frame True {
            n1960 = call-poly "Enqueue Message.vi"("error in (no error)"=w3277, "Message"="Confirm Quit", "Message Queue"=w3278) -> ("error out"=w3279:errorcluster)  [unwired: 7 in, 1 out]
          }
          frame False {
            n1961 = call-poly "Enqueue Message.vi"("error in (no error)"=w3281, "Message"="Sway Main", "Message Queue"=w3282) -> ("error out"=w3283:errorcluster)  [unwired: 7 in, 1 out]
          }
        }
      }
      frame "Error" {
        # "#CodeRecommended - If you ever change the name of this \"Error\" message, you'll need to update the name in the Check Loop Error.vi as well."
        # "#CodeRecommended - Consider creating a system for logging errors in some way. These errors are for notification purposes only. Handling of specific errors should be performed in the message frames that generated the error."
        # "Error - Display an error dialog. This message is sent by the \"Error Handler\" VIs at the end of other loops in this application."
        n1962 = Merge Errors(w3285) -> (w3286:errorcluster)
      }
      frame "Confirm Quit" {
        # "#CodeNeeded - If you want to provide an \"Are you sure\" dialog (or some other notification) before the application exits, place that code here. This message is typically sent from a Panel Close? event."
        # "Confirm Quit - Message that can confirm whether or not the user wants to exit the application."
        n1963 = call-poly "Enqueue Message.vi"("Priority Message? (F)"=TRUE, "error in (no error)"=w3294, "Message"="Exit", "Message Queue"=w3290) -> ("error out"=w3291:errorcluster)  [unwired: 6 in, 1 out]
        n1964 = Merge Errors(w3291) -> (w3292:errorcluster)
      }
      frame "Exit" {
        # "Stop the VI"
        # "Release the message queue reference"
        # "#CodeNeeded - Add any required cleanup code here. Note that if 'Exit' was called as a result of an error, an error dialog will be displayed. Add any custom error handling for an 'Exit' condition here as well."
        # "Exit - Exit the application."
        n1965 = call "Fire User Event - Stop.vi"("User Event - Stop"=w3295) -> ("error out"=w3297:errorcluster)  [unwired: 10 in]
        n1966 = Release Queue(queue=w3302, error in (no error)=w3296) -> (error out=w3299:errorcluster)  [unwired: 1 in, 2 out]
        n1967 = Merge Errors(w3297, w3299) -> (w3298:errorcluster)
      }
      frame Default {
        # "'Default' case only runs if there is a message that isn't defined in any of the other cases.  Output a programming error."
        n1968 = xnode ("Error Ring")("parameter 0"=w3303) -> ("error out"=w3304:errorcluster)
      }
    }
    n1969 = call "LAB-IQ Error Handler - Message Handling Loop.vi"("error in (no error)"=w3216, "Message Queue"=w3218) -> ("dup error in"=w3217:errorcluster)  [unwired: 8 in, 1 out]
  }
  n1970 = while {
    shift-right: [w3324] -> _
    shift-left: w47 -> [w3325]
    tunnel: [w3318] -> w61
    tunnel: w11 -> [w3316]
    tunnel: w18 -> [w3315]
    tunnel: w48 -> [w3314]
    stop <- w3323 stop-if-true
    # "Temperature  Handling Loop"
    n1971 = call "Dequeue Message.vi"("error in (no error)"=w3315, "Message Queue"=w3316) -> ("error out"=w3322:errorcluster, "output data"=w3320:dbl[][], "Message"=w3321:string, "dup Message Queue"=w3319:refnum<queue>)  [unwired: 6 in]
    n1972 = case "Message Cases" shown="\"Confirm Quit\"" w3321 {
      selector: w3321 -> [_ _ _ _ _ w3384]
      tunnel: w3319 -> [w3330 w3343 _ w3373 w3383 _]
      tunnel: w3322 -> [w3332 w3341 w3363 w3370 w3377 _]
      tunnel: [w3333 w3344 w3364 w3375 w3379 w3385] -> w3317
      tunnel: w3325 -> [w3328 w3334 w3365 w3368 w3382 w3386]
      tunnel: [w3328 w3334 w3365 w3368 w3382 w3386] -> w3324
      tunnel: [_ _ _ _ TRUE _] -> w3323
      tunnel: w3320 -> [_ _ _ _ _ _]
      tunnel: w3314 -> [_ _ _ _ w3376 _]
      frame "init" {
        # "Initialize - All initialization work should take place in this message, since other loops can potentially enqueue messages that execute immediately after this one."
        n1973 = call "Temperature vi FGV.vi"("Enum"=Temperature_enum."Init", "error in"=w3332, "main ref"=w3328) -> ("error out"=w3329:errorcluster)  [unwired: 8 in]
        n1974 = call <vilib>:"Clear Errors.vi"("error in (no error)"=w3329) -> ("error out"=w3326:errorcluster)  [unwired: 5 in, 1 out]
        n1975 = call-poly "Enqueue Message.vi"("error in (no error)"=w3326, "Message"="Temperature Main", "Message Queue"=w3330) -> ("error out"=w3333:errorcluster)  [unwired: 7 in, 1 out]
      }
      frame "Temperature Main" {
        n1976 = call "Temperature vi FGV.vi"("Enum"=Temperature_enum."read", "error in"=w3341, "main ref"=w3334) -> ("error out"=w3336:errorcluster)  [unwired: 8 in]
        n1977 = case shown="Error .." w3336 {
          selector: w3336 -> [w3345 w3353]
          tunnel: [w3345 w3346] -> w3335
          tunnel: w3334 -> [_ w3348]
          frame No Error {
          }
          frame Error {
            n1978 = call <vilib>:"Clear Errors.vi"("error in (no error)"=w3353) -> ("error out"=w3352:errorcluster)  [unwired: 5 in, 1 out]
            n1979 = call "Temperature vi FGV.vi"("Enum"=Temperature_enum."close", "error in"=w3352, "main ref"=w3348) -> ("error out"=w3351:errorcluster)  [unwired: 8 in]
            n1980 = call <vilib>:"Clear Errors.vi"("error in (no error)"=w3351) -> ("error out"=w3347:errorcluster)  [unwired: 5 in, 1 out]
            n1981 = call "Temperature vi FGV.vi"("Enum"=Temperature_enum."error_init", "error in"=w3347, "main ref"=w3348) -> ("error out"=w3350:errorcluster)  [unwired: 8 in]
            n1982 = call <vilib>:"Clear Errors.vi"("error in (no error)"=w3350) -> ("error out"=w3346:errorcluster)  [unwired: 5 in, 1 out]
          }
        }
        n1983 = Unbundle By Name(w3334) -> ("Main Home Screen.EXIT"=w3342:refnum<vi>)
        n1984 = property on="Property Node" class="Bool (strict)"(reference=w3342) -> (reference out=w3339:refnum<vi>, error out=w3340:errorcluster, "Value"=w3338:bool)  [unwired: 1 in]
        n1985 = case shown="False" w3338 {
          tunnel: [w3357 w3361] -> w3344
          tunnel: w3343 -> [w3356 w3360]
          tunnel: w3335 -> [w3355 w3359]
          frame True {
            n1986 = call-poly "Enqueue Message.vi"("error in (no error)"=w3355, "Message"="Confirm Quit", "Message Queue"=w3356) -> ("error out"=w3357:errorcluster)  [unwired: 7 in, 1 out]
          }
          frame False {
            n1987 = call-poly "Enqueue Message.vi"("error in (no error)"=w3359, "Message"="Temperature Main", "Message Queue"=w3360) -> ("error out"=w3361:errorcluster)  [unwired: 7 in, 1 out]
          }
        }
        n1988 = Close Reference(reference=w3339, error in (no error)=w3340) -> ()  [unwired: 1 out]
      }
      frame "Error" {
        # "#CodeRecommended - If you ever change the name of this \"Error\" message, you'll need to update the name in the Check Loop Error.vi as well."
        # "#CodeRecommended - Consider creating a system for logging errors in some way. These errors are for notification purposes only. Handling of specific errors should be performed in the message frames that generated the error."
        # "Error - Display an error dialog. This message is sent by the \"Error Handler\" VIs at the end of other loops in this application."
        n1989 = Merge Errors(w3363) -> (w3364:errorcluster)
      }
      frame "Confirm Quit" {
        # "#CodeNeeded - If you want to provide an \"Are you sure\" dialog (or some other notification) before the application exits, place that code here. This message is typically sent from a Panel Close? event."
        # "Confirm Quit - Message that can confirm whether or not the user wants to exit the application."
        n1990 = call "Temperature vi FGV.vi"("Enum"=Temperature_enum."close", "error in"=w3370, "main ref"=w3368) -> ("error out"=w3369:errorcluster)  [unwired: 8 in]
        n1991 = call <vilib>:"Clear Errors.vi"("error in (no error)"=w3369) -> ("error out"=w3366:errorcluster)  [unwired: 5 in, 1 out]
        n1992 = call-poly "Enqueue Message.vi"("Priority Message? (F)"=TRUE, "error in (no error)"=w3366, "Message"="Exit", "Message Queue"=w3373) -> ("error out"=w3374:errorcluster)  [unwired: 6 in, 1 out]
        n1993 = Merge Errors(w3374) -> (w3375:errorcluster)
      }
      frame "Exit" {
        # "Stop the VI"
        # "Release the message queue reference"
        # "#CodeNeeded - Add any required cleanup code here. Note that if 'Exit' was called as a result of an error, an error dialog will be displayed. Add any custom error handling for an 'Exit' condition here as well."
        # "Exit - Exit the application."
        n1994 = call "Fire User Event - Stop.vi"("User Event - Stop"=w3376) -> ("error out"=w3378:errorcluster)  [unwired: 10 in]
        n1995 = Release Queue(queue=w3383, error in (no error)=w3377) -> (error out=w3380:errorcluster)  [unwired: 1 in, 2 out]
        n1996 = Merge Errors(w3378, w3380) -> (w3379:errorcluster)
      }
      frame Default {
        # "'Default' case only runs if there is a message that isn't defined in any of the other cases.  Output a programming error."
        n1997 = xnode ("Error Ring")("parameter 0"=w3384) -> ("error out"=w3385:errorcluster)
      }
    }
    n1998 = call "LAB-IQ Error Handler - Message Handling Loop.vi"("error in (no error)"=w3317, "Message Queue"=w3319) -> ("dup error in"=w3318:errorcluster)  [unwired: 8 in, 1 out]
    n1999 = Wait (ms)(milliseconds to wait=u32 50) -> ()  [unwired: 1 out]
  }
  n2000 = while {
    shift-right: [w3396] -> _
    shift-left: w47 -> [w3406]
    tunnel: [w3400] -> w52
    tunnel: w7 -> [w3394]
    tunnel: w18 -> [w3398]
    tunnel: w48 -> [w3397]
    stop <- w3405 stop-if-true
    # "Program  Handling Loop"
    n2001 = call "Dequeue Message.vi"("error in (no error)"=w3398, "Message Queue"=w3394) -> ("error out"=w3404:errorcluster, "output data"=w3402:dbl[][], "Message"=w3403:string, "dup Message Queue"=w3401:refnum<queue>)  [unwired: 6 in]
    n2002 = case "Message Cases" shown="\"Program Main\"" w3403 {
      selector: w3403 -> [_ _ _ _ _ w3447]
      tunnel: w3401 -> [w3407 w3419 _ w3434 w3446 _]
      tunnel: w3404 -> [w3410 w3413 w3429 w3438 w3440 _]
      tunnel: [w3411 w3420 w3430 w3436 w3442 w3448] -> w3399
      tunnel: w3406 -> [w3409 w3412 w3431 w3437 w3445 w3449]
      tunnel: [w3409 w3412 w3431 w3437 w3445 w3449] -> w3396
      tunnel: [_ _ _ _ TRUE _] -> w3405
      tunnel: w3402 -> [_ _ _ _ _ _]
      tunnel: w3397 -> [_ _ _ _ w3439 _]
      frame "init" {
        # "Initialize - All initialization work should take place in this message, since other loops can potentially enqueue messages that execute immediately after this one."
        n2003 = call-poly "Enqueue Message.vi"("error in (no error)"=w3410, "Message"="Program Main", "Message Queue"=w3407) -> ("error out"=w3411:errorcluster)  [unwired: 7 in, 1 out]
      }
      frame "Program Main" {
        n2004 = call "Main Program Loop Vi.vi"("error in (no error)"=w3413, "Data Cluster"=w3412) -> ("error out"=w3414:errorcluster)  [unwired: 9 in]
        n2005 = Unbundle By Name(w3412) -> ("Main Home Screen.EXIT"=w3418:refnum<vi>)
        n2006 = property on="Property Node" class="Bool (strict)"(reference=w3418) -> (reference out=w3416:refnum<vi>, error out=w3417:errorcluster, "Value"=w3415:bool)  [unwired: 1 in]
        n2007 = case shown="False" w3415 {
          tunnel: [w3423 w3427] -> w3420
          tunnel: w3419 -> [w3422 w3426]
          tunnel: w3414 -> [w3421 w3425]
          frame True {
            n2008 = call-poly "Enqueue Message.vi"("error in (no error)"=w3421, "Message"="Confirm Quit", "Message Queue"=w3422) -> ("error out"=w3423:errorcluster)  [unwired: 7 in, 1 out]
          }
          frame False {
            n2009 = call-poly "Enqueue Message.vi"("error in (no error)"=w3425, "Message"="Program Main", "Message Queue"=w3426) -> ("error out"=w3427:errorcluster)  [unwired: 7 in, 1 out]
          }
        }
        n2010 = Close Reference(reference=w3416, error in (no error)=w3417) -> ()  [unwired: 1 out]
      }
      frame "Error" {
        # "#CodeRecommended - If you ever change the name of this \"Error\" message, you'll need to update the name in the Check Loop Error.vi as well."
        # "#CodeRecommended - Consider creating a system for logging errors in some way. These errors are for notification purposes only. Handling of specific errors should be performed in the message frames that generated the error."
        # "Error - Display an error dialog. This message is sent by the \"Error Handler\" VIs at the end of other loops in this application."
        n2011 = Merge Errors(w3429) -> (w3430:errorcluster)
      }
      frame "Confirm Quit" {
        # "#CodeNeeded - If you want to provide an \"Are you sure\" dialog (or some other notification) before the application exits, place that code here. This message is typically sent from a Panel Close? event."
        # "Confirm Quit - Message that can confirm whether or not the user wants to exit the application."
        n2012 = call-poly "Enqueue Message.vi"("Priority Message? (F)"=TRUE, "error in (no error)"=w3438, "Message"="Exit", "Message Queue"=w3434) -> ("error out"=w3435:errorcluster)  [unwired: 6 in, 1 out]
        n2013 = Merge Errors(w3435) -> (w3436:errorcluster)
      }
      frame "Exit" {
        # "Stop the VI"
        # "Release the message queue reference"
        # "#CodeNeeded - Add any required cleanup code here. Note that if 'Exit' was called as a result of an error, an error dialog will be displayed. Add any custom error handling for an 'Exit' condition here as well."
        # "Exit - Exit the application."
        n2014 = call "Fire User Event - Stop.vi"("User Event - Stop"=w3439) -> ("error out"=w3441:errorcluster)  [unwired: 10 in]
        n2015 = Release Queue(queue=w3446, error in (no error)=w3440) -> (error out=w3443:errorcluster)  [unwired: 1 in, 2 out]
        n2016 = Merge Errors(w3441, w3443) -> (w3442:errorcluster)
      }
      frame Default {
        # "'Default' case only runs if there is a message that isn't defined in any of the other cases.  Output a programming error."
        n2017 = xnode ("Error Ring")("parameter 0"=w3447) -> ("error out"=w3448:errorcluster)
      }
    }
    n2018 = call "LAB-IQ Error Handler - Message Handling Loop.vi"("error in (no error)"=w3399, "Message Queue"=w3401) -> ("dup error in"=w3400:errorcluster)  [unwired: 8 in, 1 out]
    n2019 = Wait Until Next ms Multiple(millisecond multiple=i64 100 ("Period")) -> ()  [unwired: 1 out]
  }
  n2020 = while "Timed Loop" {
    shift-right: [w3461] -> _
    shift-left: w47 -> [w3471]
    tunnel: [w3465] -> w51
    tunnel: w8 -> [w3459]
    tunnel: w18 -> [w3463]
    tunnel: w48 -> [w3462]
    tunnel: w5 -> [w3460]
    shift-right: [w3457] -> _
    shift-left: dbl[][] [] -> [w3458]
    stop <- w3470 stop-if-true
    # "Monitor  Handling Loop"
    n2021 = call "Dequeue Message.vi"("error in (no error)"=w3463, "Message Queue"=w3459) -> ("error out"=w3469:errorcluster, "output data"=w3467:dbl[][], "Message"=w3468:string, "dup Message Queue"=w3466:refnum<queue>)  [unwired: 6 in]
    n2022 = case "Message Cases" shown="\"Monitor Main\"" w3468 {
      selector: w3468 -> [_ _ _ _ _ w3523]
      tunnel: w3466 -> [w3473 w3491 _ w3508 w3521 _]
      tunnel: w3469 -> [w3476 w3485 w3502 w3512 w3515 _]
      tunnel: [w3477 w3492 w3503 w3510 w3517 w3524] -> w3464
      tunnel: w3471 -> [w3475 w3484 w3504 w3511 w3520 w3525]
      tunnel: [w3475 w3484 w3504 w3511 w3520 w3525] -> w3461
      tunnel: [_ _ _ _ TRUE _] -> w3470
      tunnel: w3467 -> [_ _ _ _ _ _]
      tunnel: w3462 -> [_ _ _ _ w3514 _]
      tunnel: w3460 -> [_ w3481 _ _ _ _]
      tunnel: w3458 -> [_ w3480 _ _ _ _]
      tunnel: [dbl[][] [] ("DATA ARRAY OUT") w3479 dbl[][] [] ("DATA ARRAY OUT") dbl[][] [] ("DATA ARRAY OUT") dbl[][] [] ("DATA ARRAY OUT") dbl[][] [] ("DATA ARRAY OUT")] -> w3457
      frame "init" {
        (unwired) dbl[] [] ("DATA ARRAY 2 OUT")
        # "Initialize - All initialization work should take place in this message, since other loops can potentially enqueue messages that execute immediately after this one."
        n2023 = call-poly "Enqueue Message.vi"("error in (no error)"=w3476, "Message"="Monitor Main", "Message Queue"=w3473) -> ("error out"=w3477:errorcluster)  [unwired: 7 in, 1 out]
      }
      frame "Monitor Main" {
        n2024 = local read "tdms file out"() -> (w3478:refnum<k34>)
        n2025 = call "LOAD SELECTION MAIN CODE.vi"("error in (no error)"=w3485, "main ref"=w3484) -> ("error out"=w3482:errorcluster)  [unwired: 9 in]
        n2026 = call "Main Monitor Loop.vi"("tdms file out"=w3478, "Message Queue"=w3481, "error in (no error)"=w3485, "DATA ARRAY"=w3480, "main ref"=w3484) -> ("error out"=w3486:errorcluster, "DATA ARRAY OUT"=w3479:dbl[][])  [unwired: 5 in]
        n2027 = Merge Errors(w3486, w3482) -> (w3483:errorcluster)
        n2028 = Unbundle By Name(w3484) -> ("Main Home Screen.EXIT"=w3490:refnum<vi>)
        n2029 = property on="Property Node" class="Bool (strict)"(reference=w3490) -> (reference out=w3488:refnum<vi>, error out=w3489:errorcluster, "Value"=w3487:bool)  [unwired: 1 in]
        n2030 = case shown="False" w3487 {
          tunnel: [w3495 w3497] -> w3492
          tunnel: w3491 -> [w3494 w3499]
          tunnel: w3483 -> [w3493 w3498]
          frame True {
            n2031 = call-poly "Enqueue Message.vi"("error in (no error)"=w3493, "Message"="Confirm Quit", "Message Queue"=w3494) -> ("error out"=w3495:errorcluster)  [unwired: 7 in, 1 out]
          }
          frame False {
            n2032 = call-poly "Enqueue Message.vi"("error in (no error)"=w3498, "Message"="Monitor Main", "Message Queue"=w3499) -> ("error out"=w3497:errorcluster)  [unwired: 7 in, 1 out]
          }
        }
        n2033 = Close Reference(reference=w3488, error in (no error)=w3489) -> ()  [unwired: 1 out]
      }
      frame "Error" {
        (unwired) dbl[] [] ("DATA ARRAY 2 OUT")
        # "#CodeRecommended - If you ever change the name of this \"Error\" message, you'll need to update the name in the Check Loop Error.vi as well."
        # "#CodeRecommended - Consider creating a system for logging errors in some way. These errors are for notification purposes only. Handling of specific errors should be performed in the message frames that generated the error."
        # "Error - Display an error dialog. This message is sent by the \"Error Handler\" VIs at the end of other loops in this application."
        n2034 = Merge Errors(w3502) -> (w3503:errorcluster)
      }
      frame "Confirm Quit" {
        (unwired) dbl[] [] ("DATA ARRAY 2 OUT")
        # "#CodeNeeded - If you want to provide an \"Are you sure\" dialog (or some other notification) before the application exits, place that code here. This message is typically sent from a Panel Close? event."
        # "Confirm Quit - Message that can confirm whether or not the user wants to exit the application."
        n2035 = call-poly "Enqueue Message.vi"("Priority Message? (F)"=TRUE, "error in (no error)"=w3512, "Message"="Exit", "Message Queue"=w3508) -> ("error out"=w3509:errorcluster)  [unwired: 6 in, 1 out]
        n2036 = Merge Errors(w3509) -> (w3510:errorcluster)
      }
      frame "Exit" {
        (unwired) dbl[] [] ("DATA ARRAY 2 OUT")
        # "Stop the VI"
        # "Release the message queue reference"
        # "#CodeNeeded - Add any required cleanup code here. Note that if 'Exit' was called as a result of an error, an error dialog will be displayed. Add any custom error handling for an 'Exit' condition here as well."
        # "Exit - Exit the application."
        n2037 = call "Fire User Event - Stop.vi"("User Event - Stop"=w3514) -> ("error out"=w3516:errorcluster)  [unwired: 10 in]
        n2038 = Release Queue(queue=w3521, error in (no error)=w3515) -> (error out=w3518:errorcluster)  [unwired: 1 in, 2 out]
        n2039 = Merge Errors(w3516, w3518) -> (w3517:errorcluster)
      }
      frame Default {
        (unwired) dbl[] [] ("DATA ARRAY 2 OUT")
        # "'Default' case only runs if there is a message that isn't defined in any of the other cases.  Output a programming error."
        n2040 = xnode ("Error Ring")("parameter 0"=w3523) -> ("error out"=w3524:errorcluster)
      }
    }
    n2041 = call "LAB-IQ Error Handler - Message Handling Loop.vi"("error in (no error)"=w3464, "Message Queue"=w3466) -> ("dup error in"=w3465:errorcluster)  [unwired: 8 in, 1 out]
  }
  n2042 = while "Timed Loop" {
    shift-right: [w3551] -> _
    shift-left: w47 -> [w3552]
    tunnel: [w3545] -> w50
    tunnel: w6 -> [w3533]
    tunnel: w18 -> [w3543]
    tunnel: w48 -> [w3542]
    shift-right: [w3540] -> _
    shift-left: w59 -> [w3541]
    shift-right: [w3538] -> _
    shift-left: w59 -> [w3539]
    shift-right: [w3536] -> _
    shift-left: w59 -> [w3537]
    shift-right: [w3535] -> _
    shift-left: w59 -> [w3534]
    stop <- w3550 stop-if-true
    # "Load Pid  Handling Loop"
    n2043 = call "Dequeue Message.vi"("error in (no error)"=w3543, "Message Queue"=w3533) -> ("error out"=w3549:errorcluster, "output data"=w3547:dbl[][], "Message"=w3548:string, "dup Message Queue"=w3546:refnum<queue>)  [unwired: 6 in]
    n2044 = case "Message Cases" shown="\"Load Pid Main\"" w3548 {
      selector: w3548 -> [_ _ _ _ _ w3656]
      tunnel: w3546 -> [w3557 w3588 _ w3635 w3651 _]
      tunnel: w3549 -> [w3560 w3586 w3622 w3639 w3645 _]
      tunnel: [w3561 w3589 w3627 w3637 w3647 w3657] -> w3544
      tunnel: w3552 -> [w3559 w3564 w3628 w3638 w3650 w3658]
      tunnel: [w3559 w3564 w3628 w3638 w3650 w3658] -> w3551
      tunnel: [_ _ _ _ TRUE _] -> w3550
      tunnel: w3547 -> [_ _ _ _ _ _]
      tunnel: w3542 -> [_ _ _ _ w3644 _]
      tunnel: w3541 -> [w3555 w3576 w3626 w3632 w3643 w3654]
      tunnel: [w3555 w3575 w3626 w3632 w3643 w3654] -> w3540
      tunnel: w3539 -> [w3556 w3574 w3625 w3631 w3642 w3655]
      tunnel: [w3556 w3573 w3625 w3631 w3642 w3655] -> w3538
      tunnel: w3537 -> [w3554 w3572 w3624 w3630 w3641 w3653]
      tunnel: [w3554 w3571 w3624 w3630 w3641 w3653] -> w3536
      tunnel: w3534 -> [_ w3570 _ _ _ _]
      tunnel: [w3553 w3569 w3623 w3629 w3640 w3652] -> w3535
      tunnel: w3534 -> [w3553 _ w3623 w3629 w3640 w3652]
      frame "init" {
        # "Initialize - All initialization work should take place in this message, since other loops can potentially enqueue messages that execute immediately after this one."
        n2045 = call-poly "Enqueue Message.vi"("error in (no error)"=w3560, "Message"="Load Pid Main", "Message Queue"=w3557) -> ("error out"=w3561:errorcluster)  [unwired: 7 in, 1 out]
      }
      frame "Load Pid Main" {
        n2046 = Unbundle By Name(w3564) -> ("New PID LOGIC.PID"=w3565:refnum<vi>)
        n2047 = Unbundle By Name(w3564) -> ("Main Screen.Load En"=w3581:refnum<vi>)
        n2048 = property on="Property Node" class="Clust (strict)"(reference=w3565) -> (reference out=w3567:refnum<vi>, error out=w3566:errorcluster, "Value"=w3563:T4)  [unwired: 1 in]
        n2049 = property on="Property Node" class="Bool (strict)"(reference=w3581) -> (reference out=w3579:refnum<vi>, error out=w3580:errorcluster, "Value"=w3578:bool)  [unwired: 1 in]
        n2050 = Unbundle By Name(w3563) -> ("apply load"=w3562:bool)
        n2051 = Close Reference(reference=w3567, error in (no error)=w3566) -> ()  [unwired: 1 out]
        n2052 = Close Reference(reference=w3579, error in (no error)=w3580) -> ()  [unwired: 1 out]
        n2053 = Or(x=w3578, y=w3562) -> (x .or. y?=w3577:bool)
        n2054 = case shown="True" w3577 {
          tunnel: w3586 -> [w3596 w3609]
          tunnel: [w3596 w3608] -> w3582
          tunnel: w3564 -> [_ w3607]
          tunnel: w3576 -> [w3595 w3606]
          tunnel: [w3595 w3605] -> w3575
          tunnel: w3574 -> [w3594 w3604]
          tunnel: [w3594 w3603] -> w3573
          tunnel: w3572 -> [w3591 w3600]
          tunnel: [w3591 w3599] -> w3571
          tunnel: w3570 -> [w3590 w3598]
          tunnel: [w3590 w3597] -> w3569
          frame False {
            n2055 = local write "Checkbox 2"(TRUE ("Checkbox 2")) -> ()
            n2056 = local write "Checkbox"(TRUE ("Checkbox")) -> ()
          }
          frame True {
            n2057 = case shown="True" "Checkbox 2" {
              selector: "Checkbox 2" -> [_ w3612]
              tunnel: [FALSE ("Checkbox") "Checkbox"] -> w3602
              frame False {
              }
              frame True {
                n2058 = Not(x=w3612) -> (.not. x?=w3611:bool)
                n2059 = local write "Checkbox 2"(w3611) -> ()
              }
            }
            n2060 = call "NEW LOAD CELL PID.vi"("filtered_load_in"=w3600, "filtered_deriv_in"=w3598, "integral_out"=w3604, "error in (no error)"=w3609, "prev_error_out"=w3606, "Checkbox"=w3602, "main ref"=w3607) -> ("error out"=w3608:errorcluster, "prev_error_out"=w3605:dbl, "integral_out"=w3603:dbl, "filtered_load_out"=w3599:dbl, "filtered_deriv_out"=w3597:dbl)
          }
        }
        n2061 = Unbundle By Name(w3564) -> ("Main Home Screen.EXIT"=w3587:refnum<vi>)
        n2062 = property on="Property Node" class="Bool (strict)"(reference=w3587) -> (reference out=w3584:refnum<vi>, error out=w3585:errorcluster, "Value"=w3583:bool)  [unwired: 1 in]
        n2063 = case shown="False" w3583 {
          tunnel: [w3616 w3620] -> w3589
          tunnel: w3588 -> [w3615 w3619]
          tunnel: w3582 -> [w3614 w3618]
          frame True {
            n2064 = call-poly "Enqueue Message.vi"("error in (no error)"=w3614, "Message"="Confirm Quit", "Message Queue"=w3615) -> ("error out"=w3616:errorcluster)  [unwired: 7 in, 1 out]
          }
          frame False {
            n2065 = call-poly "Enqueue Message.vi"("error in (no error)"=w3618, "Message"="Load Pid Main", "Message Queue"=w3619) -> ("error out"=w3620:errorcluster)  [unwired: 7 in, 1 out]
          }
        }
        n2066 = Close Reference(reference=w3584, error in (no error)=w3585) -> ()  [unwired: 1 out]
        n2067 = Wait (ms)(milliseconds to wait=u32 30) -> ()  [unwired: 1 out]
      }
      frame "Error" {
        # "#CodeRecommended - If you ever change the name of this \"Error\" message, you'll need to update the name in the Check Loop Error.vi as well."
        # "#CodeRecommended - Consider creating a system for logging errors in some way. These errors are for notification purposes only. Handling of specific errors should be performed in the message frames that generated the error."
        # "Error - Display an error dialog. This message is sent by the \"Error Handler\" VIs at the end of other loops in this application."
        n2068 = Merge Errors(w3622) -> (w3627:errorcluster)
      }
      frame "Confirm Quit" {
        # "#CodeNeeded - If you want to provide an \"Are you sure\" dialog (or some other notification) before the application exits, place that code here. This message is typically sent from a Panel Close? event."
        # "Confirm Quit - Message that can confirm whether or not the user wants to exit the application."
        n2069 = call-poly "Enqueue Message.vi"("Priority Message? (F)"=TRUE, "error in (no error)"=w3639, "Message"="Exit", "Message Queue"=w3635) -> ("error out"=w3636:errorcluster)  [unwired: 6 in, 1 out]
        n2070 = Merge Errors(w3636) -> (w3637:errorcluster)
      }
      frame "Exit" {
        # "Stop the VI"
        # "Release the message queue reference"
        # "#CodeNeeded - Add any required cleanup code here. Note that if 'Exit' was called as a result of an error, an error dialog will be displayed. Add any custom error handling for an 'Exit' condition here as well."
        # "Exit - Exit the application."
        n2071 = call "Fire User Event - Stop.vi"("User Event - Stop"=w3644) -> ("error out"=w3646:errorcluster)  [unwired: 10 in]
        n2072 = Release Queue(queue=w3651, error in (no error)=w3645) -> (error out=w3648:errorcluster)  [unwired: 1 in, 2 out]
        n2073 = Merge Errors(w3646, w3648) -> (w3647:errorcluster)
      }
      frame Default {
        # "'Default' case only runs if there is a message that isn't defined in any of the other cases.  Output a programming error."
        n2074 = xnode ("Error Ring")("parameter 0"=w3656) -> ("error out"=w3657:errorcluster)
      }
    }
    n2075 = call "LAB-IQ Error Handler - Message Handling Loop.vi"("error in (no error)"=w3544, "Message Queue"=w3546) -> ("dup error in"=w3545:errorcluster)  [unwired: 8 in, 1 out]
  }
  n2076 = while {
    shift-right: [w3676] -> _
    shift-left: w47 -> [w3677]
    tunnel: [w3671] -> _
    tunnel: w5 -> [w3666]
    tunnel: w18 -> [w3669]
    tunnel: w48 -> [w3668]
    stop <- w3675 stop-if-true
    # "Report  Handling Loop"
    n2077 = call "Dequeue Message.vi"("error in (no error)"=w3669, "Message Queue"=w3666) -> ("error out"=w3674:errorcluster, "output data"=w3667:dbl[][], "Message"=w3673:string, "dup Message Queue"=w3672:refnum<queue>)  [unwired: 6 in]
    n2078 = case "Message Cases" shown="\"Report\"" w3673 {
      selector: w3673 -> [_ _ _ _ _ w3717]
      tunnel: w3672 -> [w3678 w3694 _ w3704 w3716 _]
      tunnel: w3674 -> [w3680 _ w3699 w3708 w3710 _]
      tunnel: [w3681 w3695 w3700 w3706 w3712 w3718] -> w3670
      tunnel: w3677 -> [w3679 w3689 w3701 w3707 w3715 w3719]
      tunnel: [w3679 w3689 w3701 w3707 w3715 w3719] -> w3676
      tunnel: [_ _ _ _ TRUE _] -> w3675
      tunnel: w3668 -> [_ _ _ _ w3709 _]
      tunnel: w3667 -> [_ w3688 _ _ _ _]
      frame "init" {
        # "Initialize - All initialization work should take place in this message, since other loops can potentially enqueue messages that execute immediately after this one."
        n2079 = disable-structure shown="Disabled" {
          disable-tunnel: [w3685 w3686] -> w3681
          disable-tunnel: w3680 -> [w3684 w3686]
          disable-tunnel: w3678 -> [w3682 _]
          frame Disabled {
            n2080 = call-poly "Enqueue Message.vi"("error in (no error)"=w3684, "Message"="Report", "Message Queue"=w3682) -> ("error out"=w3685:errorcluster)  [unwired: 7 in, 1 out]
          }
          frame Enabled {
          }
        }
      }
      frame "Report" {
        n2081 = local read "tdms file out"() -> (w3687:refnum<k34>)
        n2082 = call "Main Data Log.vi"("tdms file out"=w3687, "output data"=w3688, "main ref"=w3689) -> ()  [unwired: 8 in, 1 out]
        n2083 = Unbundle By Name(w3689) -> ("Main Home Screen.EXIT"=w3693:refnum<vi>)
        n2084 = property on="Property Node" class="Bool (strict)"(reference=w3693) -> (reference out=w3691:refnum<vi>, error out=w3692:errorcluster, "Value"=w3690:bool)  [unwired: 1 in]
        n2085 = case shown="False" w3690 {
          tunnel: [w3697 _] -> w3695
          tunnel: w3694 -> [w3696 _]
          frame True {
            n2086 = call-poly "Enqueue Message.vi"("Message"="Confirm Quit", "Message Queue"=w3696) -> ("error out"=w3697:errorcluster)  [unwired: 8 in, 1 out]
          }
          frame False {
          }
        }
        n2087 = Close Reference(reference=w3691, error in (no error)=w3692) -> ()  [unwired: 1 out]
      }
      frame "Error" {
        # "#CodeRecommended - If you ever change the name of this \"Error\" message, you'll need to update the name in the Check Loop Error.vi as well."
        # "#CodeRecommended - Consider creating a system for logging errors in some way. These errors are for notification purposes only. Handling of specific errors should be performed in the message frames that generated the error."
        # "Error - Display an error dialog. This message is sent by the \"Error Handler\" VIs at the end of other loops in this application."
        n2088 = Merge Errors(w3699) -> (w3700:errorcluster)
      }
      frame "Confirm Quit" {
        # "#CodeNeeded - If you want to provide an \"Are you sure\" dialog (or some other notification) before the application exits, place that code here. This message is typically sent from a Panel Close? event."
        # "Confirm Quit - Message that can confirm whether or not the user wants to exit the application."
        n2089 = call-poly "Enqueue Message.vi"("Priority Message? (F)"=TRUE, "error in (no error)"=w3708, "Message"="Exit", "Message Queue"=w3704) -> ("error out"=w3705:errorcluster)  [unwired: 6 in, 1 out]
        n2090 = Merge Errors(w3705) -> (w3706:errorcluster)
      }
      frame "Exit" {
        # "Stop the VI"
        # "Release the message queue reference"
        # "#CodeNeeded - Add any required cleanup code here. Note that if 'Exit' was called as a result of an error, an error dialog will be displayed. Add any custom error handling for an 'Exit' condition here as well."
        # "Exit - Exit the application."
        n2091 = call "Fire User Event - Stop.vi"("User Event - Stop"=w3709) -> ("error out"=w3711:errorcluster)  [unwired: 10 in]
        n2092 = Release Queue(queue=w3716, error in (no error)=w3710) -> (error out=w3713:errorcluster)  [unwired: 1 in, 2 out]
        n2093 = Merge Errors(w3711, w3713) -> (w3712:errorcluster)
      }
      frame Default {
        # "'Default' case only runs if there is a message that isn't defined in any of the other cases.  Output a programming error."
        n2094 = xnode ("Error Ring")("parameter 0"=w3717) -> ("error out"=w3718:errorcluster)
      }
    }
    n2095 = call "LAB-IQ Error Handler - Message Handling Loop.vi"("error in (no error)"=w3670, "Message Queue"=w3672) -> ("dup error in"=w3671:errorcluster)  [unwired: 8 in, 1 out]
  }
  n2096 = while {
    shift-right: [w3729] -> _
    shift-left: w47 -> [w3739]
    tunnel: [w3733] -> w46
    tunnel: w4 -> [w3727]
    tunnel: w18 -> [w3731]
    tunnel: w48 -> [w3730]
    stop <- w3738 stop-if-true
    # "Acqoustic  Handling Loop"
    n2097 = call "Dequeue Message.vi"("error in (no error)"=w3731, "Message Queue"=w3727) -> ("error out"=w3737:errorcluster, "output data"=w3735:dbl[][], "Message"=w3736:string, "dup Message Queue"=w3734:refnum<queue>)  [unwired: 6 in]
    n2098 = case "Message Cases" shown="\"Acoustic Main\"" w3736 {
      selector: w3736 -> [_ _ _ _ _ w3820]
      tunnel: w3734 -> [w3751 w3772 _ w3805 w3818 _]
      tunnel: w3737 -> [w3745 w3763 w3798 w3809 w3812 _]
      tunnel: [w3753 w3773 w3800 w3807 w3814 w3821] -> w3732
      tunnel: w3739 -> [w3742 w3758 w3801 w3808 w3817 w3822]
      tunnel: [w3742 w3758 w3801 w3808 w3817 w3822] -> w3729
      tunnel: [_ _ _ _ TRUE _] -> w3738
      tunnel: w3735 -> [_ _ _ _ _ _]
      tunnel: w3730 -> [_ _ _ _ w3811 _]
      tunnel: [i64 1000 ("Period") w3754 i64 1000 ("Period") i64 1000 ("Period") i64 1000 ("Period") i64 1000 ("Period")] -> w3728
      frame "init" {
        # "Initialize - All initialization work should take place in this message, since other loops can potentially enqueue messages that execute immediately after this one."
        n2099 = call "Acq Write Loop.vi"("Enum - Menu"=Write_Main_Enum."INIT", "error in (no error)"=w3745, "main ref"=w3742) -> ("error out"=w3750:errorcluster)  [unwired: 8 in]
        n2100 = call <vilib>:"Clear Errors.vi"("error in (no error)"=w3750) -> ("error out"=w3749:errorcluster)  [unwired: 5 in, 1 out]
        n2101 = call "Stall Data Flow.vim"("value in"=w3749, "milliseconds to wait"=u32 1000) -> ("value out"=w3748:errorcluster)  [unwired: 1 out]
        n2102 = call "Acq Read Loop.vi"("Enum - Menu"=Read_Main_Enum."INIT", "error in (no error)"=w3748, "main ref"=w3742) -> ("error out"=w3746:errorcluster)  [unwired: 7 in, 1 out]
        n2103 = call <vilib>:"Clear Errors.vi"("error in (no error)"=w3746) -> ("error out"=w3744:errorcluster)  [unwired: 5 in, 1 out]
        n2104 = call-poly "Enqueue Message.vi"("error in (no error)"=w3744, "Message"="Acoustic Main", "Message Queue"=w3751) -> ("error out"=w3753:errorcluster)  [unwired: 7 in, 1 out]
      }
      frame "Acoustic Main" {
        (unwired) TRUE
        n2105 = Unbundle By Name(w3758) -> ("Environmental control.Acoustic Emission 3"=w3767:refnum<vi>)
        n2106 = Unbundle By Name(w3758) -> ("Main Screen.Start Test Temp"=w3759:refnum<vi>)
        n2107 = property class="Bool (strict)"(reference=w3759) -> (reference out=w3757:refnum<vi>, error out=w3760:errorcluster, "Value"=w3755:bool)  [unwired: 1 in]
        n2108 = property on="Property Node" class="Bool (strict)"(reference=w3767) -> (reference out=w3765:refnum<vi>, error out=w3766:errorcluster, "Value"=w3764:bool)  [unwired: 1 in]
        n2109 = Close Reference(reference=w3757, error in (no error)=w3760) -> ()  [unwired: 1 out]
        n2110 = Close Reference(reference=w3765, error in (no error)=w3766) -> ()  [unwired: 1 out]
        n2111 = And(x=w3764, y=w3755) -> (x .and. y?=w3756:bool)
        n2112 = case shown="True" w3756 {
          tunnel: w3763 -> [w3775 w3784]
          tunnel: w3758 -> [_ w3779]
          tunnel: [w3775 w3777] -> w3762
          tunnel: [i64 1000 ("Period") i64 1 ("Period")] -> w3754
          frame False {
          }
          frame True {
            n2113 = call "Acq Read Loop.vi"("Enum - Menu"=Read_Main_Enum."READ", "error in (no error)"=w3784, "main ref"=w3779) -> ("error out"=w3782:errorcluster, "ERROR TEMP"=w3781:bool)  [unwired: 7 in]
            n2114 = call <vilib>:"Clear Errors.vi"("error in (no error)"=w3782) -> ("error out"=w3778:errorcluster)  [unwired: 5 in, 1 out]
            n2115 = disable-structure shown="Disabled" {
              disable-tunnel: w3781 -> [w3788 _]
              disable-tunnel: [w3787 w3789] -> w3780
              disable-tunnel: w3779 -> [w3786 _]
              disable-tunnel: w3778 -> [w3785 w3789]
              frame Disabled {
                n2116 = call "Acoustic Reinitize.vi"("error in (no error)"=w3785, "Checkbox"=w3788, "Data Cluster"=w3786) -> ("error out"=w3787:errorcluster)  [unwired: 8 in]
              }
              frame Enabled {
              }
            }
            n2117 = call <vilib>:"Clear Errors.vi"("error in (no error)"=w3780) -> ("error out"=w3777:errorcluster)  [unwired: 5 in, 1 out]
          }
        }
        n2118 = Unbundle By Name(w3758) -> ("Main Home Screen.EXIT"=w3771:refnum<vi>)
        n2119 = property on="Property Node" class="Bool (strict)"(reference=w3771) -> (reference out=w3769:refnum<vi>, error out=w3770:errorcluster, "Value"=w3768:bool)  [unwired: 1 in]
        n2120 = call <vilib>:"Clear Errors.vi"("error in (no error)"=w3762) -> ("error out"=w3761:errorcluster)  [unwired: 5 in, 1 out]
        n2121 = Close Reference(reference=w3769, error in (no error)=w3770) -> ()  [unwired: 1 out]
        n2122 = case shown="True" w3768 {
          tunnel: [w3792 w3796] -> w3773
          tunnel: w3772 -> [w3791 w3795]
          tunnel: w3761 -> [w3790 w3794]
          frame True {
            n2123 = call-poly "Enqueue Message.vi"("error in (no error)"=w3790, "Message"="Confirm Quit", "Message Queue"=w3791) -> ("error out"=w3792:errorcluster)  [unwired: 7 in, 1 out]
          }
          frame False {
            n2124 = call-poly "Enqueue Message.vi"("error in (no error)"=w3794, "Message"="Acoustic Main", "Message Queue"=w3795) -> ("error out"=w3796:errorcluster)  [unwired: 7 in, 1 out]
          }
        }
      }
      frame "Error" {
        # "#CodeRecommended - If you ever change the name of this \"Error\" message, you'll need to update the name in the Check Loop Error.vi as well."
        # "#CodeRecommended - Consider creating a system for logging errors in some way. These errors are for notification purposes only. Handling of specific errors should be performed in the message frames that generated the error."
        # "Error - Display an error dialog. This message is sent by the \"Error Handler\" VIs at the end of other loops in this application."
        n2125 = Merge Errors(w3798) -> (w3800:errorcluster)
      }
      frame "Confirm Quit" {
        # "#CodeNeeded - If you want to provide an \"Are you sure\" dialog (or some other notification) before the application exits, place that code here. This message is typically sent from a Panel Close? event."
        # "Confirm Quit - Message that can confirm whether or not the user wants to exit the application."
        n2126 = call-poly "Enqueue Message.vi"("Priority Message? (F)"=TRUE, "error in (no error)"=w3809, "Message"="Exit", "Message Queue"=w3805) -> ("error out"=w3806:errorcluster)  [unwired: 6 in, 1 out]
        n2127 = Merge Errors(w3806) -> (w3807:errorcluster)
      }
      frame "Exit" {
        # "Stop the VI"
        # "Release the message queue reference"
        # "#CodeNeeded - Add any required cleanup code here. Note that if 'Exit' was called as a result of an error, an error dialog will be displayed. Add any custom error handling for an 'Exit' condition here as well."
        # "Exit - Exit the application."
        n2128 = call "Fire User Event - Stop.vi"("User Event - Stop"=w3811) -> ("error out"=w3813:errorcluster)  [unwired: 10 in]
        n2129 = Release Queue(queue=w3818, error in (no error)=w3812) -> (error out=w3815:errorcluster)  [unwired: 1 in, 2 out]
        n2130 = Merge Errors(w3813, w3815) -> (w3814:errorcluster)
      }
      frame Default {
        # "'Default' case only runs if there is a message that isn't defined in any of the other cases.  Output a programming error."
        n2131 = xnode ("Error Ring")("parameter 0"=w3820) -> ("error out"=w3821:errorcluster)
      }
    }
    n2132 = Wait (ms)(milliseconds to wait=w3728) -> ()  [unwired: 1 out]
    n2133 = call "LAB-IQ Error Handler - Message Handling Loop.vi"("error in (no error)"=w3732, "Message Queue"=w3734) -> ("dup error in"=w3733:errorcluster)  [unwired: 8 in, 1 out]
  }
  n2134 = Unregister For Events(event registration refnum=w93, error in=w91) -> (error out=w94:errorcluster)
  n2135 = Merge Errors(w94, w96, w70, w69, w68, w61, w58, w54, w53, w52, w51, w50, w46, w46) -> (w95:errorcluster)
  n2136 = call "Destroy User Event - Stop.vi"("error in (no error)"=w95, "User Event - Stop"=w48) -> ("error out"=w92:errorcluster)  [unwired: 9 in]
  n2137 = disable-structure "Conditional Disable Structure" shown="RUN_TIME_ENGINE==True" {
    disable-tunnel: w92 -> [_ _]
    frame condition #0 (active) {
    }
    frame condition #1 {
      # "Call Quit LabVIEW if running as a built application."
      n2138 = Quit LabVIEW() -> ()  [unwired: 1 in]
    }
  }
